vi "SSL Detection Frame Simple Estimator Cameras VelCmd.vi"(0 "NewCameras":T1[](array[typedef]) {"robots_blue"."height" format="%+4.3f"; "robots_blue"."pixel_y" format="%+4.3f"; "robots_blue"."pixel_x" format="%+4.3f"; "robots_blue"."orientation" format="%+4.3f"; "robots_blue"."y" format="%+4.3f"; "robots_blue"."confidence" format="%4.3f"; "robots_blue"."x" format="%+4.3f"; "robots_yellow"."height" format="%+4.3f"; "robots_yellow"."pixel_y" format="%+4.3f"; "robots_yellow"."pixel_x" format="%+4.3f"; "robots_yellow"."orientation" format="%+4.3f"; "robots_yellow"."y" format="%+4.3f"; "robots_yellow"."confidence" format="%4.3f"; "robots_yellow"."x" format="%+4.3f"}, 1 "Life Time":dbl=4.0, 2 "timeToValidateBall":dbl=0.5, 3 "Estimador":T5=enum."Nenhum", 5 "Field Size":T6, 9 "grSim?":bool, 10 "cameras array":dbl[](array[numeric]), 12 "Team":enum16{"Azul", "Amarelo"}(ring) caption="Enum", 14 "max ball vel":dbl, 15 "Side":enum16{"Esquerdo", "Direito"}(ring)=enum."Direito" caption="Enum") -> (4 "Detection Frame Out":T1 {"robots_blue"."height" format="%+4.3f"; "robots_blue"."pixel_y" format="%+4.3f"; "robots_blue"."pixel_x" format="%+4.3f"; "robots_blue"."orientation" format="%+4.3f"; "robots_blue"."y" format="%+4.3f"; "robots_blue"."confidence" format="%4.3f"; "robots_blue"."x" format="%+4.3f"; "robots_yellow"."height" format="%+4.3f"; "robots_yellow"."pixel_y" format="%+4.3f"; "robots_yellow"."pixel_x" format="%+4.3f"; "robots_yellow"."orientation" format="%+4.3f"; "robots_yellow"."y" format="%+4.3f"; "robots_yellow"."confidence" format="%4.3f"; "robots_yellow"."x" format="%+4.3f"}, 6 "Field Size Out":T6)   [LabVIEW 2022 SP3]
uses:
  Controls/SSL Detection Frame.ctl
  Controls/SSL Detection Robot.ctl
  <vilib>/Analysis/Matrix/Datatypes/RealMatrix.ctl
  Controls/SSL Detection Ball.ctl
  Controls/Estimadores.ctl
  <vilib>/Analysis/Matrix/Numeric/Conversions/Array To Matrix - RA.vi
  <vilib>/Analysis/Matrix/NI_Matrix.lvlib
  <vilib>/ptbypt/NI_PtbyPt.lvlib
  Utilities_class/Utilities.lvclass
  <vilib>/Analysis/NI_AALBase.lvlib
  Vision.lvclass
panel:
  in  "Enable":bool=TRUE
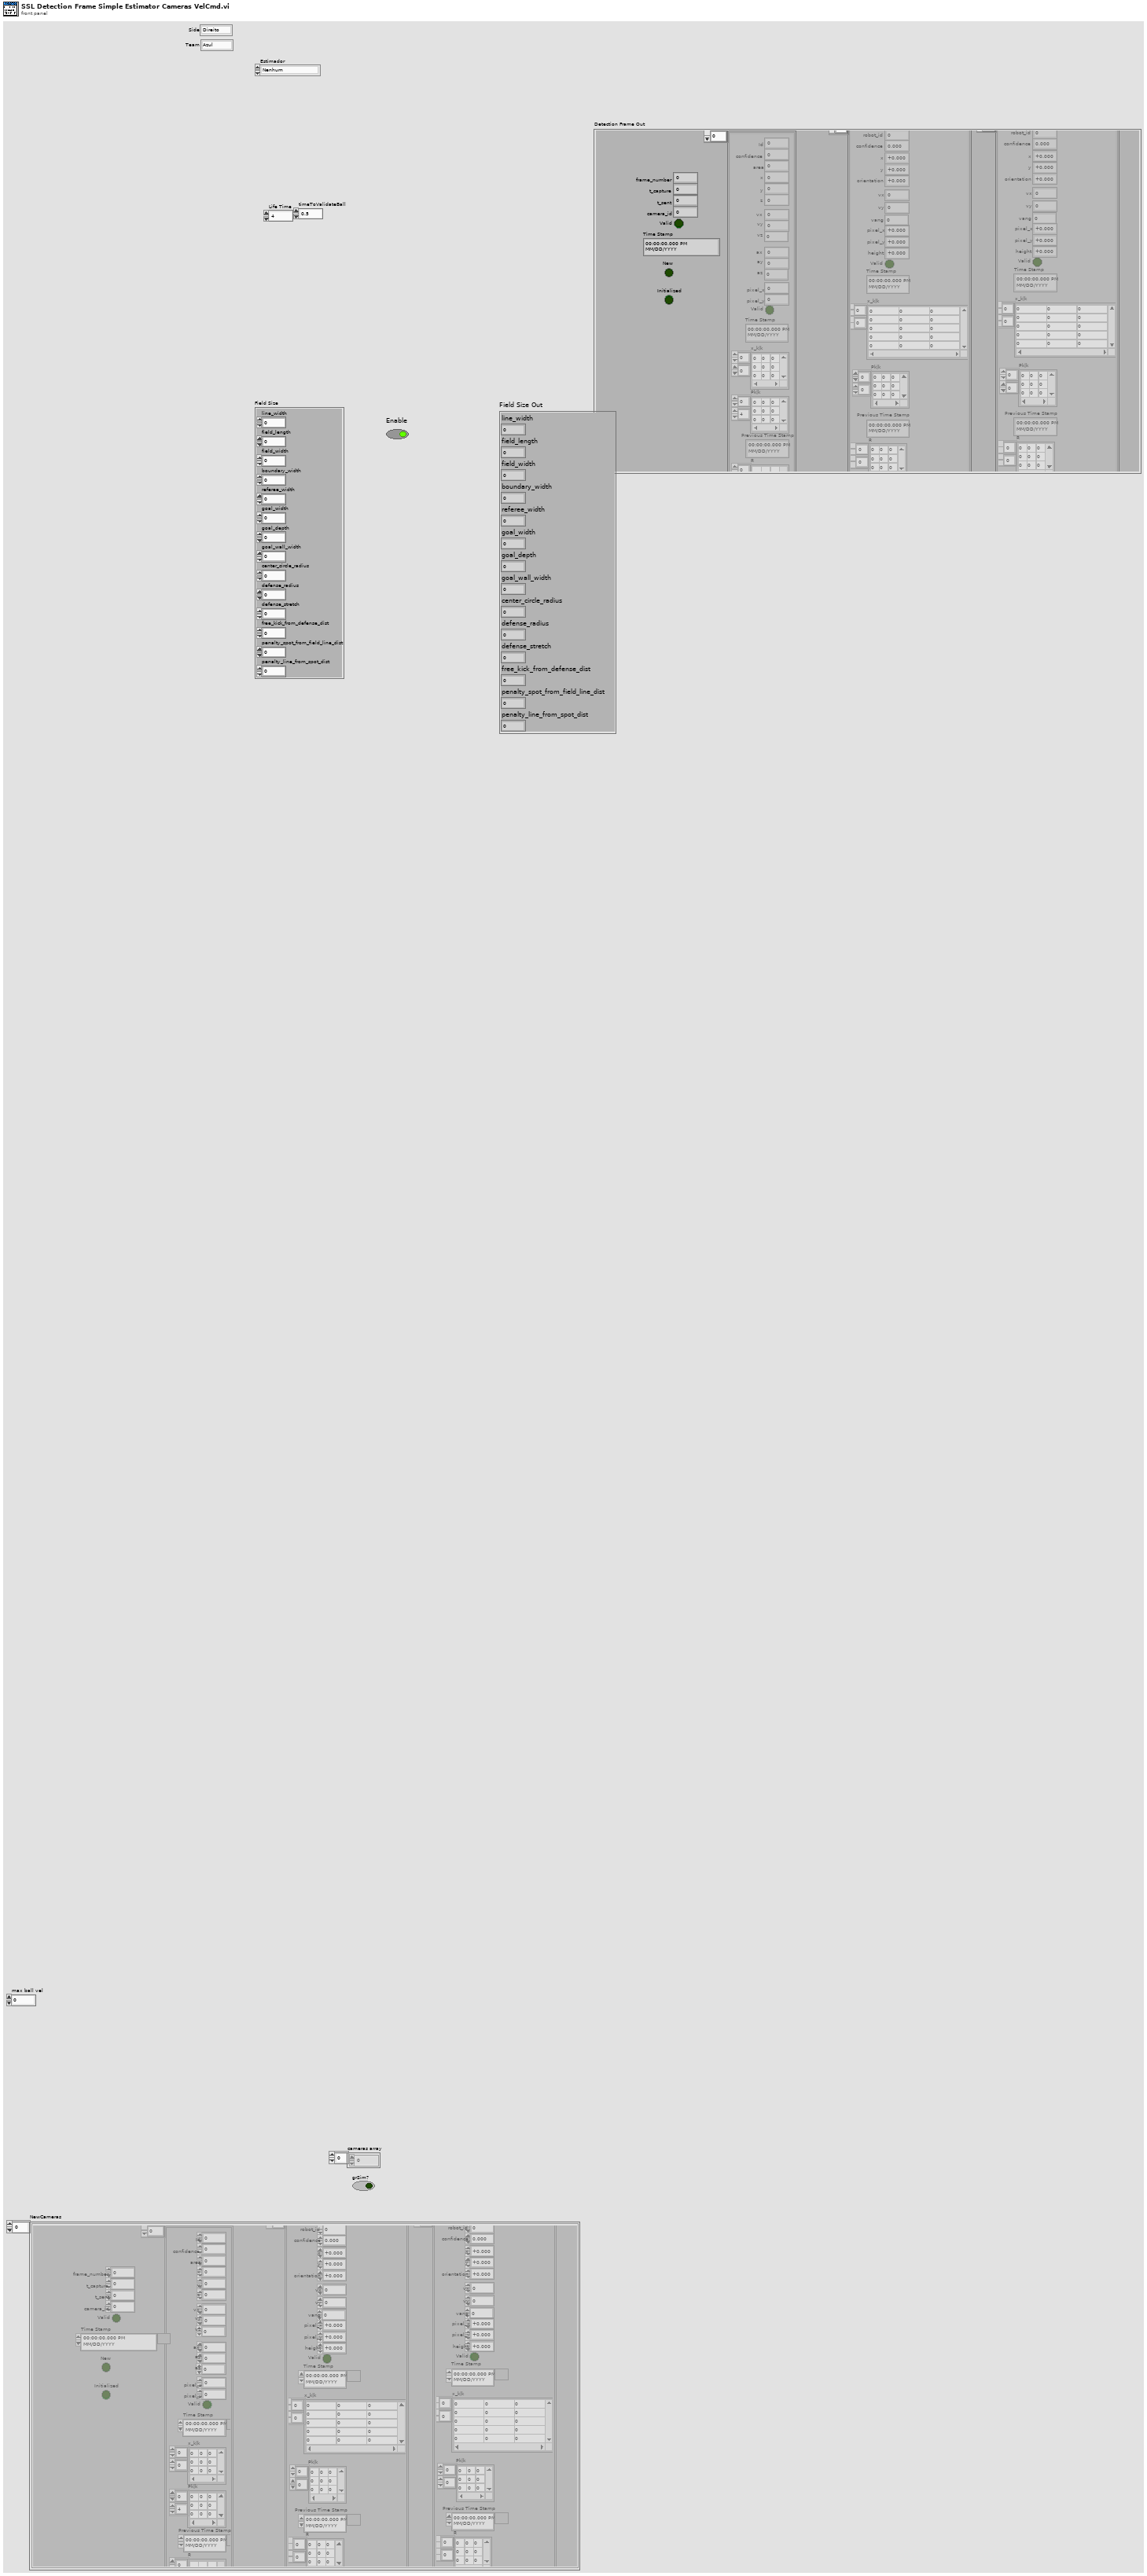
[diagram p1: front panel]
types:
  T1 = typedef "SSL Detection Frame.ctl" = cluster{"frame_number":u32, "t_capture":dbl, "t_sent":dbl, "camera_id":u32, "robots_yellow":T2[], "robots_blue":T2[], "balls":T4[], "Valid":bool, "Time Stamp":timestamp, "New":bool, "Initialized":bool}
  T2 = typedef "SSL Detection Robot.ctl" = cluster{"x":sgl, "robot_id":u32, "confidence":sgl, "y":sgl, "orientation":sgl, "pixel_x":sgl, "pixel_y":sgl, "height":sgl, "Valid":bool, "Time Stamp":timestamp, "x_k|k":T3, "Pk|k":T3, "Previous Time Stamp":timestamp, "R":T3, "vx":dbl, "vy":dbl, "vang":dbl}
  T3 = typedef "NI_Matrix.lvlib/RealMatrix.ctl" = dbl[][]
  T4 = typedef "SSL Detection Ball.ctl" = cluster{"x":sgl, "area":u32, "confidence":sgl, "y":sgl, "z":sgl, "pixel_x":sgl, "pixel_y":sgl, "Valid":bool, "Time Stamp":timestamp, "x_k|k":T3, "Pk|k":T3, "Id":u32, "Previous Time Stamp":timestamp, "R":T3, " vx":sgl, "vy":dbl, "vz":dbl, " ax":sgl, "ay":dbl, "az":dbl}
  T5 = typedef "Estimadores.ctl" = enum16{"Variable2ndDerivate", "4thDerivate", "2ndDerivate", "Nenhum", "Simples", "Kalman"}
  T6 = cluster{"line_width":u32, "field_length":u32, "field_width":u32, "boundary_width":u32, "referee_width":u32, "goal_width":u32, "goal_depth":u32, "goal_wall_width":u32, "center_circle_radius":u32, "defense_radius":u32, "defense_stretch":u32, "free_kick_from_defense_dist":u32, "penalty_spot_from_field_line_dist":u32, "penalty_line_from_spot_dist":u32}
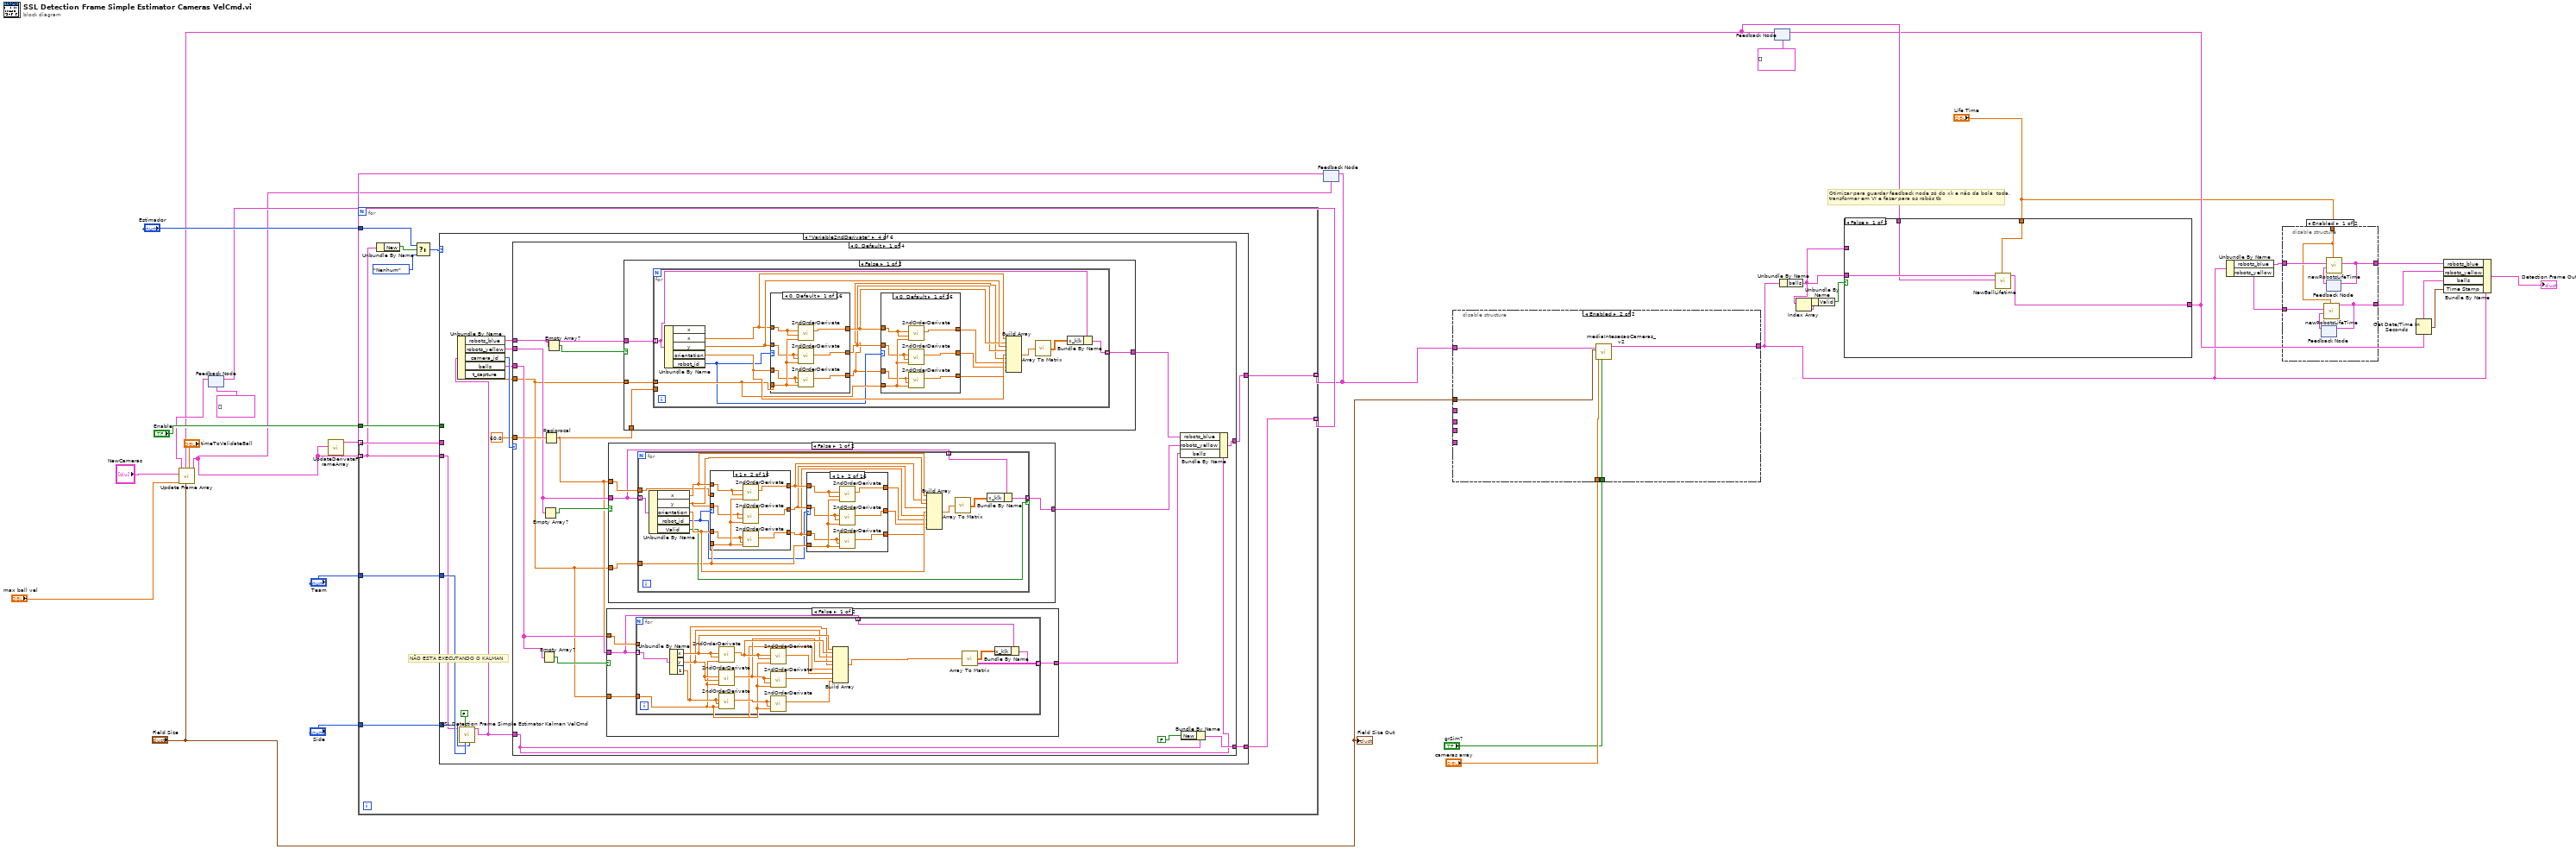
[diagram p0: block diagram]
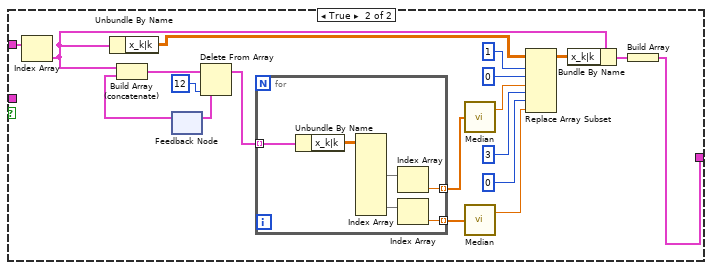
[diagram p3: hidden frame]
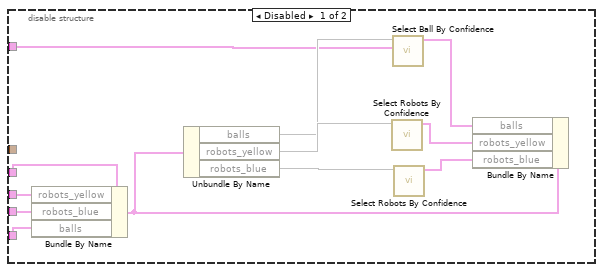
[diagram p4: hidden frame]
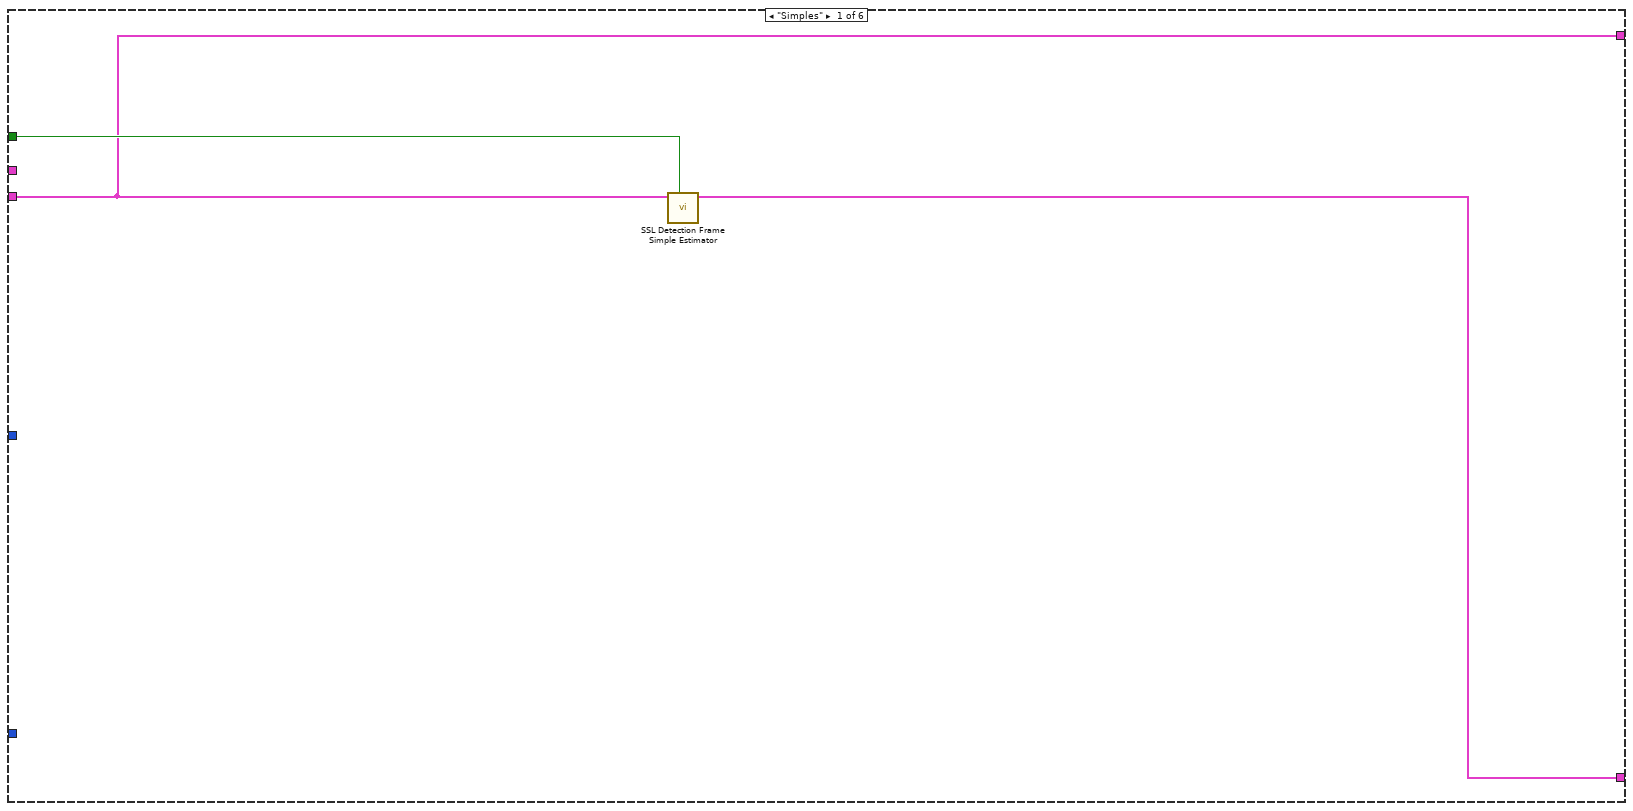
[diagram p5: hidden frame]
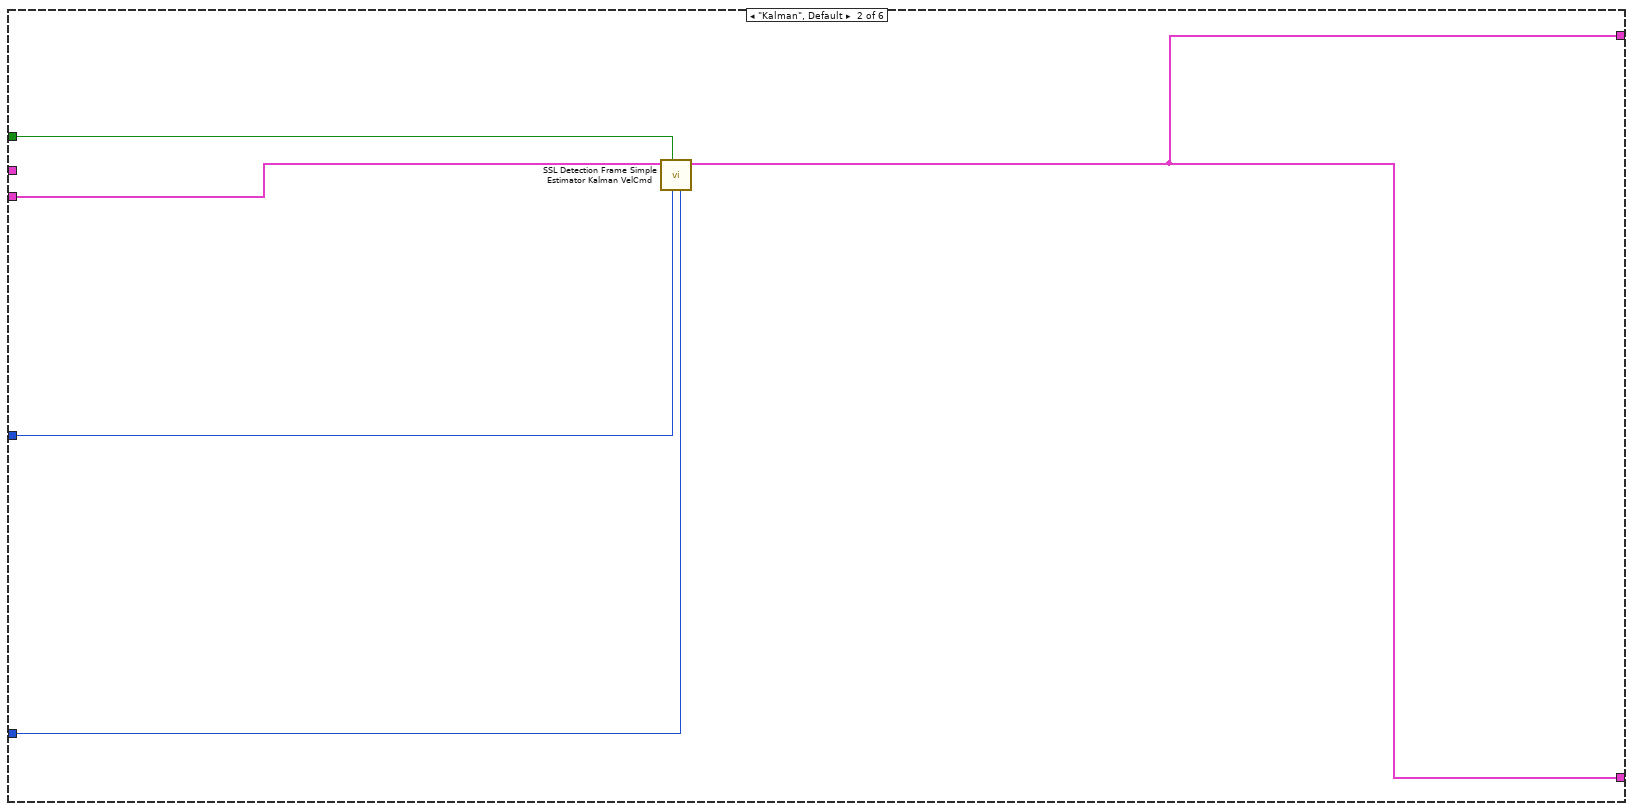
[diagram p6: hidden frame]
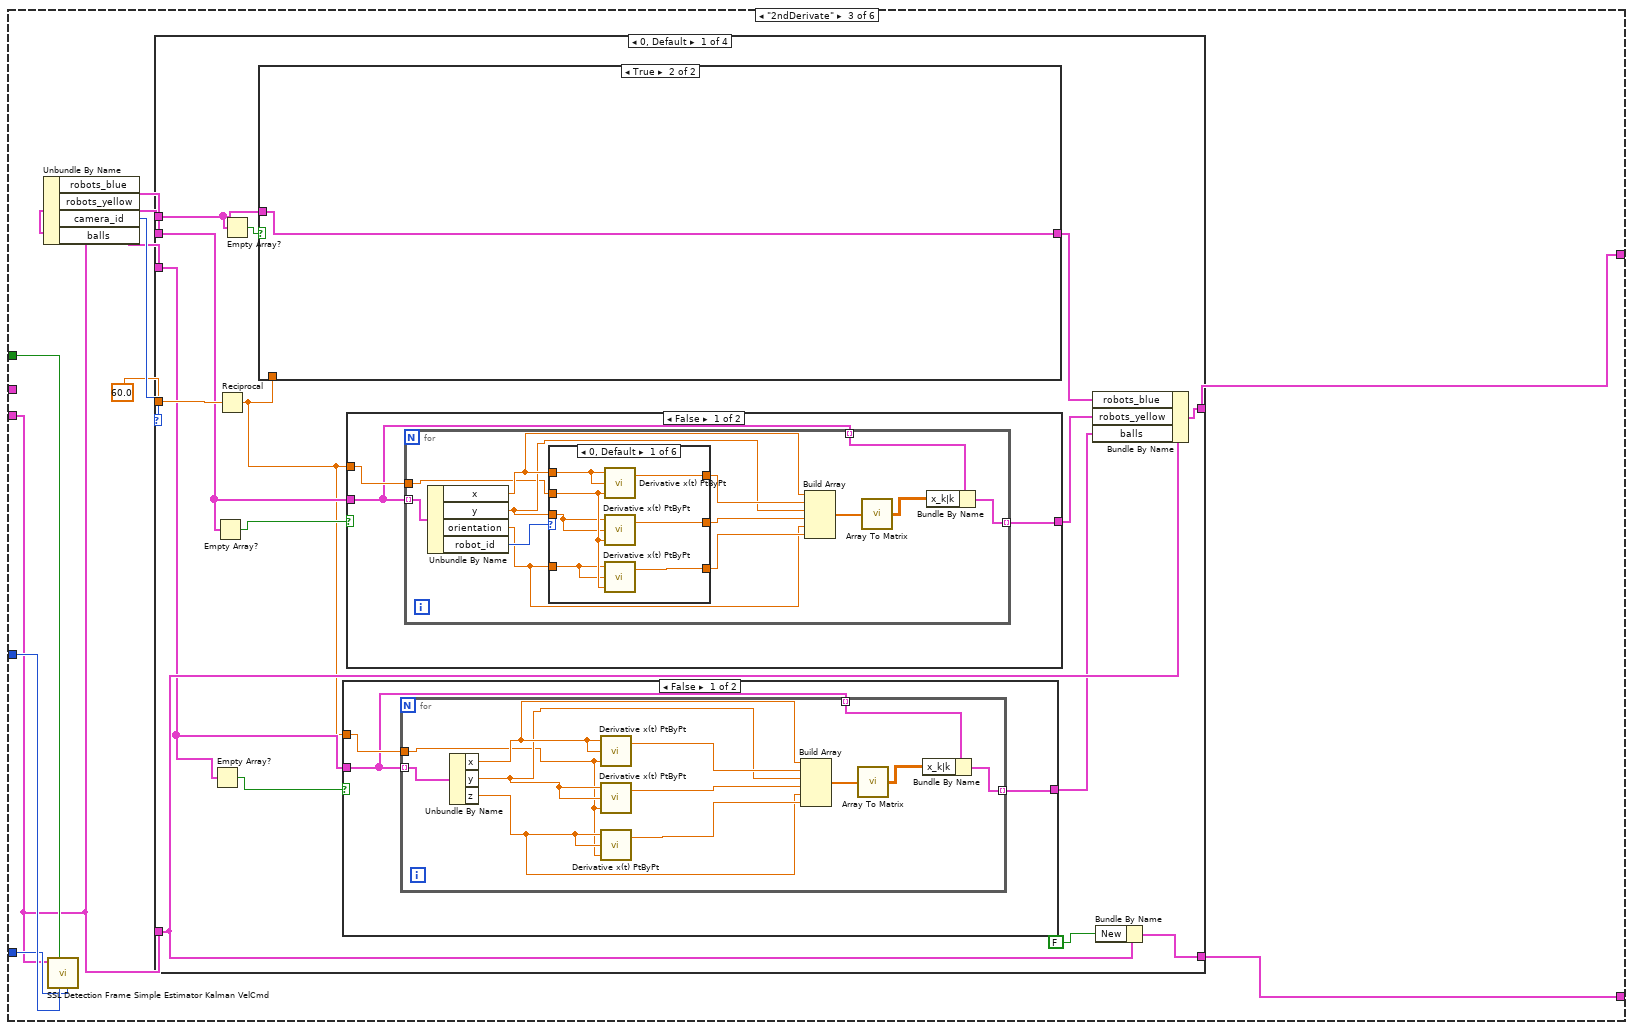
[diagram p7: hidden frame]
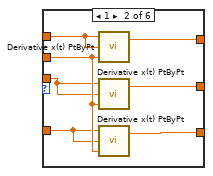
[diagram p9: hidden frame]
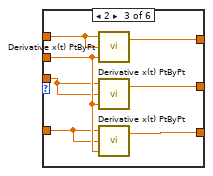
[diagram p10: hidden frame]
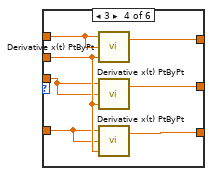
[diagram p11: hidden frame]
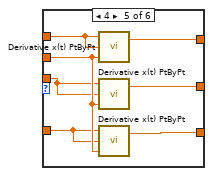
[diagram p12: hidden frame]
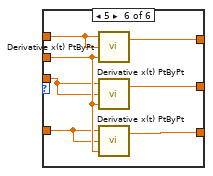
[diagram p13: hidden frame]
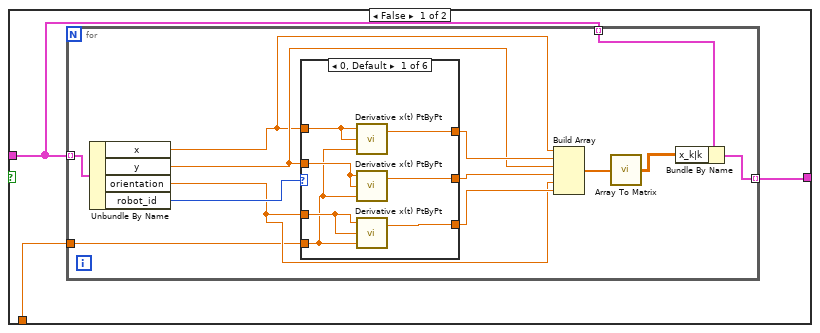
[diagram p15: hidden frame]
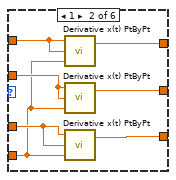
[diagram p16: hidden frame]
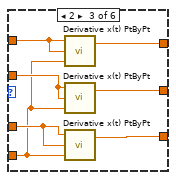
[diagram p17: hidden frame]
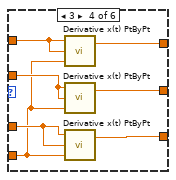
[diagram p18: hidden frame]
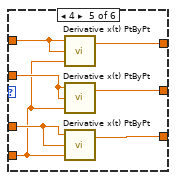
[diagram p19: hidden frame]
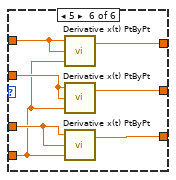
[diagram p20: hidden frame]
diagram:
  # "Otimizar para guardar feedback node só do xk e não da bola  toda.\ntransformar em VI e fazer para os robôs tb"
  n1 = feedback #1(T1[] []) -> (w28:T1[])
  n2 = feedback #2(T4[] [] ("balls")) -> (w13:T4[])
  n3 = call "Update Frame Array.vi"("timeToValidateBall"="timeToValidateBall", "Field Size"="Field Size", "balls"=w13, "max ball vel"="max ball vel", "Detection Frame In"="NewCameras", "Array Detection Frame In"=w28) -> ("Detection Frame out"=w18:T1[])  [unwired: 4 in, 1 out]
  n4 = feedback #3(w18) -> (w19:T1[])
  n5 = call "UpdateDerivateFrameArray.vi"("Current Detection Frame In"=w18, "Last Array Detection Frame In"=w19) -> ("Sorted Cameras Array"=w17:T1[])  [unwired: 9 in]
  n6 = for {
    tunnel: [w41] -> w26 mode=indexing
    tunnel: "Estimador" -> [w38]
    tunnel: "Enable" -> [w42]
    tunnel: w18 -> [w33] mode=indexing
    tunnel: "Team" -> [w40]
    tunnel: "Side" -> [w39]
    tunnel: [w36] -> w16 mode=indexing
    tunnel: w17 -> [w35] mode=indexing
    # "NÃO ESTA EXECUTANDO O KALMAN"
    n7 = Unbundle By Name(w33) -> ("New"=w34:bool)
    n8 = Select(t=w38, s=w34, f=Estimadores."Nenhum" ("Estimador")) -> (s? t:f=w37:T5)
    n9 = case shown="\"Variable2ndDerivate\"" w37 {
      tunnel: [w44 w46 w55 w665 w2786 w4880] -> w41
      tunnel: w33 -> [w43 w47 w51 w660 w2781 w4880]
      tunnel: w42 -> [w45 w50 w61 _ _ _]
      tunnel: w40 -> [_ w49 w60 w670 w2791 _]
      tunnel: w39 -> [_ w48 w59 w669 w2790 _]
      tunnel: [w43 w46 w56 w666 w2787 w4879] -> w36
      tunnel: w35 -> [_ _ _ _ _ w4879]
      frame "Simples" {
        n10 = call "SSL Detection Frame Simple Estimator.vi"("Enable"=w45, "Detection Frame In"=w43) -> ("Detection Frame Out"=w44:T1)  [unwired: 8 in, 1 out]
      }
      frame "Kalman", Default {
        n11 = call "SSL Detection Frame Simple Estimator Kalman VelCmd.vi"("Lado"=w48, "Time"=w49, "Enable"=w50, "Detection Frame In"=w47) -> ("Detection Frame Out"=w46:T1)  [unwired: 6 in, 1 out]
      }
      frame "2ndDerivate" {
        n12 = Unbundle By Name(w51) -> ("robots_blue"=w58:T2[], "robots_yellow"=w57:T2[], "camera_id"=w54:u32, "balls"=w53:T4[])
        n13 = call "SSL Detection Frame Simple Estimator Kalman VelCmd.vi"("Lado"=w59, "Time"=w60, "Enable"=w61, "Detection Frame In"=w51) -> ()  [unwired: 6 in, 2 out]
        n14 = case shown="0, Default" w54 {
          tunnel: w58 -> [w75 w224 w373 w522]
          tunnel: 60.0 -> [w74 w223 w372 w521]
          tunnel: w57 -> [w72 w221 w370 w519]
          tunnel: [w69 w218 w367 w516] -> w56
          tunnel: [w67 w216 w365 w514] -> w55
          tunnel: w51 -> [w66 w215 w364 w513]
          tunnel: w53 -> [w64 w213 w362 w511]
          frame 0, Default {
            n15 = Empty Array?(array=w64) -> (empty?=w65:bool)
            n16 = Empty Array?(array=w72) -> (empty?=w73:bool)
            n17 = Reciprocal(x=w74) -> (1/x=w63:dbl)
            n18 = Empty Array?(array=w75) -> (empty?=w76:bool)
            n19 = case shown="True" w76 {
              tunnel: w75 -> [w153 w210]
              tunnel: w63 -> [w154 _]
              tunnel: [w152 w210] -> w71
              frame False {
                n20 = for {
                  tunnel: w153 -> [w167] mode=indexing
                  tunnel: w154 -> [w157]
                  tunnel: w153 -> [w165] mode=indexing
                  tunnel: [w156] -> w152 mode=indexing
                  n21 = Unbundle By Name(w167) -> ("x"=w155:sgl, "y"=w159:sgl, "orientation"=w158:sgl, "robot_id"=w166:u32)
                  n22 = case shown="0, Default" w166 {
                    tunnel: w155 -> [w168 w178 w185 w192 w199 w206]
                    tunnel: [w174 w181 w188 w195 w202 w209] -> w164
                    tunnel: [w173 w180 w187 w194 w201 w208] -> w163
                    tunnel: [w172 w179 w186 w193 w200 w207] -> w162
                    tunnel: w159 -> [w171 w177 w184 w191 w198 w205]
                    tunnel: w158 -> [w170 w176 w183 w190 w197 w204]
                    tunnel: w157 -> [w169 w175 w182 w189 w196 w203]
                    frame 0, Default {
                      n23 = call <vilib>:"Derivative x(t) PtByPt.vi"("dt"=w169, "initial condition"=w168, "x"=w168) -> ("dx/dt"=w174:dbl)  [unwired: 1 in, 1 out]
                      n24 = call <vilib>:"Derivative x(t) PtByPt.vi"("dt"=w169, "initial condition"=w171, "x"=w171) -> ("dx/dt"=w173:dbl)  [unwired: 1 in, 1 out]
                      n25 = call <vilib>:"Derivative x(t) PtByPt.vi"("dt"=w169, "initial condition"=w170, "x"=w170) -> ("dx/dt"=w172:dbl)  [unwired: 1 in, 1 out]
                    }
                    frame 1 {
                      n26 = call <vilib>:"Derivative x(t) PtByPt.vi"("dt"=w175, "initial condition"=w178, "x"=w178) -> ("dx/dt"=w181:dbl)  [unwired: 1 in, 1 out]
                      n27 = call <vilib>:"Derivative x(t) PtByPt.vi"("dt"=w175, "initial condition"=w177, "x"=w177) -> ("dx/dt"=w180:dbl)  [unwired: 1 in, 1 out]
                      n28 = call <vilib>:"Derivative x(t) PtByPt.vi"("dt"=w175, "initial condition"=w176, "x"=w176) -> ("dx/dt"=w179:dbl)  [unwired: 1 in, 1 out]
                    }
                    frame 2 {
                      n29 = call <vilib>:"Derivative x(t) PtByPt.vi"("dt"=w182, "initial condition"=w185, "x"=w185) -> ("dx/dt"=w188:dbl)  [unwired: 1 in, 1 out]
                      n30 = call <vilib>:"Derivative x(t) PtByPt.vi"("dt"=w182, "initial condition"=w184, "x"=w184) -> ("dx/dt"=w187:dbl)  [unwired: 1 in, 1 out]
                      n31 = call <vilib>:"Derivative x(t) PtByPt.vi"("dt"=w182, "initial condition"=w183, "x"=w183) -> ("dx/dt"=w186:dbl)  [unwired: 1 in, 1 out]
                    }
                    frame 3 {
                      n32 = call <vilib>:"Derivative x(t) PtByPt.vi"("dt"=w189, "initial condition"=w192, "x"=w192) -> ("dx/dt"=w195:dbl)  [unwired: 1 in, 1 out]
                      n33 = call <vilib>:"Derivative x(t) PtByPt.vi"("dt"=w189, "initial condition"=w191, "x"=w191) -> ("dx/dt"=w194:dbl)  [unwired: 1 in, 1 out]
                      n34 = call <vilib>:"Derivative x(t) PtByPt.vi"("dt"=w189, "initial condition"=w190, "x"=w190) -> ("dx/dt"=w193:dbl)  [unwired: 1 in, 1 out]
                    }
                    frame 4 {
                      n35 = call <vilib>:"Derivative x(t) PtByPt.vi"("dt"=w196, "initial condition"=w199, "x"=w199) -> ("dx/dt"=w202:dbl)  [unwired: 1 in, 1 out]
                      n36 = call <vilib>:"Derivative x(t) PtByPt.vi"("dt"=w196, "initial condition"=w198, "x"=w198) -> ("dx/dt"=w201:dbl)  [unwired: 1 in, 1 out]
                      n37 = call <vilib>:"Derivative x(t) PtByPt.vi"("dt"=w196, "initial condition"=w197, "x"=w197) -> ("dx/dt"=w200:dbl)  [unwired: 1 in, 1 out]
                    }
                    frame 5 {
                      n38 = call <vilib>:"Derivative x(t) PtByPt.vi"("dt"=w203, "initial condition"=w206, "x"=w206) -> ("dx/dt"=w209:dbl)  [unwired: 1 in, 1 out]
                      n39 = call <vilib>:"Derivative x(t) PtByPt.vi"("dt"=w203, "initial condition"=w205, "x"=w205) -> ("dx/dt"=w208:dbl)  [unwired: 1 in, 1 out]
                      n40 = call <vilib>:"Derivative x(t) PtByPt.vi"("dt"=w203, "initial condition"=w204, "x"=w204) -> ("dx/dt"=w207:dbl)  [unwired: 1 in, 1 out]
                    }
                  }
                  n41 = Build Array(w155, w164, w159, w163, w158, w162) -> (w161:dbl[])
                  n42 = call-poly <vilib>:"Array To Matrix.vi"("Real 1D Array"=w161) -> ("Real Matrix (Column Vector)"=w160:T3)
                  n43 = Bundle By Name(cluster=w165, "x_k|k"=w160) -> (w156:T2)
                }
              }
              frame True {
              }
            }
            n44 = case shown="False" w65 {
              tunnel: w64 -> [w78 w92]
              tunnel: w63 -> [w79 _]
              tunnel: [w77 w92] -> w62
              frame False {
                n45 = for {
                  tunnel: w78 -> [w91] mode=indexing
                  tunnel: w79 -> [w80]
                  tunnel: w78 -> [w90] mode=indexing
                  tunnel: [w81] -> w77 mode=indexing
                  n46 = Unbundle By Name(w91) -> ("x"=w85:sgl, "y"=w84:sgl, "z"=w86:sgl)
                  n47 = call <vilib>:"Derivative x(t) PtByPt.vi"("dt"=w80, "initial condition"=w85, "x"=w85) -> ("dx/dt"=w89:dbl)  [unwired: 1 in, 1 out]
                  n48 = call <vilib>:"Derivative x(t) PtByPt.vi"("dt"=w80, "initial condition"=w84, "x"=w84) -> ("dx/dt"=w88:dbl)  [unwired: 1 in, 1 out]
                  n49 = call <vilib>:"Derivative x(t) PtByPt.vi"("dt"=w80, "initial condition"=w86, "x"=w86) -> ("dx/dt"=w87:dbl)  [unwired: 1 in, 1 out]
                  n50 = Build Array(w85, w89, w84, w88, w86, w87) -> (w83:dbl[])
                  n51 = call-poly <vilib>:"Array To Matrix.vi"("Real 1D Array"=w83) -> ("Real Matrix (Column Vector)"=w82:T3)
                  n52 = Bundle By Name(cluster=w90, "x_k|k"=w82) -> (w81:T4)
                }
              }
              frame True {
              }
            }
            n53 = case shown="False" w73 {
              tunnel: w72 -> [w94 w151]
              tunnel: w63 -> [w95 _]
              tunnel: [w93 w151] -> w70
              frame False {
                n54 = for {
                  tunnel: w94 -> [w108] mode=indexing
                  tunnel: w95 -> [w96]
                  tunnel: w94 -> [w106] mode=indexing
                  tunnel: [w97] -> w93 mode=indexing
                  n55 = Unbundle By Name(w108) -> ("x"=w101:sgl, "y"=w100:sgl, "orientation"=w102:sgl, "robot_id"=w107:u32)
                  n56 = case shown="0, Default" w107 {
                    tunnel: w101 -> [w112 w119 w126 w133 w140 w147]
                    tunnel: w100 -> [w110 w117 w124 w131 w138 w145]
                    tunnel: w102 -> [w109 w116 w123 w130 w137 w144]
                    tunnel: [w115 w122 w129 w136 w143 w150] -> w105
                    tunnel: [w114 w121 w128 w135 w142 w149] -> w104
                    tunnel: [w113 w120 w127 w134 w141 w148] -> w103
                    tunnel: w96 -> [w111 w118 w125 w132 w139 w146]
                    frame 0, Default {
                      n57 = call <vilib>:"Derivative x(t) PtByPt.vi"("dt"=w111, "initial condition"=w112, "x"=w112) -> ("dx/dt"=w115:dbl)  [unwired: 1 in, 1 out]
                      n58 = call <vilib>:"Derivative x(t) PtByPt.vi"("dt"=w111, "initial condition"=w110, "x"=w110) -> ("dx/dt"=w114:dbl)  [unwired: 1 in, 1 out]
                      n59 = call <vilib>:"Derivative x(t) PtByPt.vi"("dt"=w111, "initial condition"=w109, "x"=w109) -> ("dx/dt"=w113:dbl)  [unwired: 1 in, 1 out]
                    }
                    frame 1 {
                      n60 = call <vilib>:"Derivative x(t) PtByPt.vi"("dt"=w118, "initial condition"=w119, "x"=w119) -> ("dx/dt"=w122:dbl)  [unwired: 1 in, 1 out]
                      n61 = call <vilib>:"Derivative x(t) PtByPt.vi"("dt"=w118, "initial condition"=w117, "x"=w117) -> ("dx/dt"=w121:dbl)  [unwired: 1 in, 1 out]
                      n62 = call <vilib>:"Derivative x(t) PtByPt.vi"("dt"=w118, "initial condition"=w116, "x"=w116) -> ("dx/dt"=w120:dbl)  [unwired: 1 in, 1 out]
                    }
                    frame 2 {
                      n63 = call <vilib>:"Derivative x(t) PtByPt.vi"("dt"=w125, "initial condition"=w126, "x"=w126) -> ("dx/dt"=w129:dbl)  [unwired: 1 in, 1 out]
                      n64 = call <vilib>:"Derivative x(t) PtByPt.vi"("dt"=w125, "initial condition"=w124, "x"=w124) -> ("dx/dt"=w128:dbl)  [unwired: 1 in, 1 out]
                      n65 = call <vilib>:"Derivative x(t) PtByPt.vi"("dt"=w125, "initial condition"=w123, "x"=w123) -> ("dx/dt"=w127:dbl)  [unwired: 1 in, 1 out]
                    }
                    frame 3 {
                      n66 = call <vilib>:"Derivative x(t) PtByPt.vi"("dt"=w132, "initial condition"=w133, "x"=w133) -> ("dx/dt"=w136:dbl)  [unwired: 1 in, 1 out]
                      n67 = call <vilib>:"Derivative x(t) PtByPt.vi"("dt"=w132, "initial condition"=w131, "x"=w131) -> ("dx/dt"=w135:dbl)  [unwired: 1 in, 1 out]
                      n68 = call <vilib>:"Derivative x(t) PtByPt.vi"("dt"=w132, "initial condition"=w130, "x"=w130) -> ("dx/dt"=w134:dbl)  [unwired: 1 in, 1 out]
                    }
                    frame 4 {
                      n69 = call <vilib>:"Derivative x(t) PtByPt.vi"("dt"=w139, "initial condition"=w140, "x"=w140) -> ("dx/dt"=w143:dbl)  [unwired: 1 in, 1 out]
                      n70 = call <vilib>:"Derivative x(t) PtByPt.vi"("dt"=w139, "initial condition"=w138, "x"=w138) -> ("dx/dt"=w142:dbl)  [unwired: 1 in, 1 out]
                      n71 = call <vilib>:"Derivative x(t) PtByPt.vi"("dt"=w139, "initial condition"=w137, "x"=w137) -> ("dx/dt"=w141:dbl)  [unwired: 1 in, 1 out]
                    }
                    frame 5 {
                      n72 = call <vilib>:"Derivative x(t) PtByPt.vi"("dt"=w146, "initial condition"=w147, "x"=w147) -> ("dx/dt"=w150:dbl)  [unwired: 1 in, 1 out]
                      n73 = call <vilib>:"Derivative x(t) PtByPt.vi"("dt"=w146, "initial condition"=w145, "x"=w145) -> ("dx/dt"=w149:dbl)  [unwired: 1 in, 1 out]
                      n74 = call <vilib>:"Derivative x(t) PtByPt.vi"("dt"=w146, "initial condition"=w144, "x"=w144) -> ("dx/dt"=w148:dbl)  [unwired: 1 in, 1 out]
                    }
                  }
                  n75 = Build Array(w101, w105, w100, w104, w102, w103) -> (w99:dbl[])
                  n76 = call-poly <vilib>:"Array To Matrix.vi"("Real 1D Array"=w99) -> ("Real Matrix (Column Vector)"=w98:T3)
                  n77 = Bundle By Name(cluster=w106, "x_k|k"=w98) -> (w97:T2)
                }
              }
              frame True {
              }
            }
            n78 = Bundle By Name(cluster=w66, "robots_blue"=w71, "robots_yellow"=w70, "balls"=w62) -> (w69:T1)
            n79 = Bundle By Name(cluster=w66, "New"=FALSE) -> (w67:T1)
          }
          frame 1 {
            n80 = Empty Array?(array=w213) -> (empty?=w214:bool)
            n81 = Empty Array?(array=w221) -> (empty?=w222:bool)
            n82 = Reciprocal(x=w223) -> (1/x=w212:dbl)
            n83 = Empty Array?(array=w224) -> (empty?=w225:bool)
            n84 = case shown="False" w225 {
              tunnel: w224 -> [w302 w359]
              tunnel: w212 -> [w303 _]
              tunnel: [w301 w359] -> w220
              frame False {
                n85 = for {
                  tunnel: w302 -> [w316] mode=indexing
                  tunnel: w303 -> [w306]
                  tunnel: w302 -> [w314] mode=indexing
                  tunnel: [w305] -> w301 mode=indexing
                  n86 = Unbundle By Name(w316) -> ("x"=w304:sgl, "y"=w308:sgl, "orientation"=w307:sgl, "robot_id"=w315:u32)
                  n87 = case shown="0, Default" w315 {
                    tunnel: w304 -> [w317 w327 w334 w341 w348 w355]
                    tunnel: [w323 w330 w337 w344 w351 w358] -> w313
                    tunnel: [w322 w329 w336 w343 w350 w357] -> w312
                    tunnel: [w321 w328 w335 w342 w349 w356] -> w311
                    tunnel: w308 -> [w320 w326 w333 w340 w347 w354]
                    tunnel: w307 -> [w319 w325 w332 w339 w346 w353]
                    tunnel: w306 -> [w318 w324 w331 w338 w345 w352]
                    frame 0, Default {
                      n88 = call <vilib>:"Derivative x(t) PtByPt.vi"("dt"=w318, "initial condition"=w317, "x"=w317) -> ("dx/dt"=w323:dbl)  [unwired: 1 in, 1 out]
                      n89 = call <vilib>:"Derivative x(t) PtByPt.vi"("dt"=w318, "initial condition"=w320, "x"=w320) -> ("dx/dt"=w322:dbl)  [unwired: 1 in, 1 out]
                      n90 = call <vilib>:"Derivative x(t) PtByPt.vi"("dt"=w318, "initial condition"=w319, "x"=w319) -> ("dx/dt"=w321:dbl)  [unwired: 1 in, 1 out]
                    }
                    frame 1 {
                      n91 = call <vilib>:"Derivative x(t) PtByPt.vi"("dt"=w324, "initial condition"=w327, "x"=w327) -> ("dx/dt"=w330:dbl)  [unwired: 1 in, 1 out]
                      n92 = call <vilib>:"Derivative x(t) PtByPt.vi"("dt"=w324, "initial condition"=w326, "x"=w326) -> ("dx/dt"=w329:dbl)  [unwired: 1 in, 1 out]
                      n93 = call <vilib>:"Derivative x(t) PtByPt.vi"("dt"=w324, "initial condition"=w325, "x"=w325) -> ("dx/dt"=w328:dbl)  [unwired: 1 in, 1 out]
                    }
                    frame 2 {
                      n94 = call <vilib>:"Derivative x(t) PtByPt.vi"("dt"=w331, "initial condition"=w334, "x"=w334) -> ("dx/dt"=w337:dbl)  [unwired: 1 in, 1 out]
                      n95 = call <vilib>:"Derivative x(t) PtByPt.vi"("dt"=w331, "initial condition"=w333, "x"=w333) -> ("dx/dt"=w336:dbl)  [unwired: 1 in, 1 out]
                      n96 = call <vilib>:"Derivative x(t) PtByPt.vi"("dt"=w331, "initial condition"=w332, "x"=w332) -> ("dx/dt"=w335:dbl)  [unwired: 1 in, 1 out]
                    }
                    frame 3 {
                      n97 = call <vilib>:"Derivative x(t) PtByPt.vi"("dt"=w338, "initial condition"=w341, "x"=w341) -> ("dx/dt"=w344:dbl)  [unwired: 1 in, 1 out]
                      n98 = call <vilib>:"Derivative x(t) PtByPt.vi"("dt"=w338, "initial condition"=w340, "x"=w340) -> ("dx/dt"=w343:dbl)  [unwired: 1 in, 1 out]
                      n99 = call <vilib>:"Derivative x(t) PtByPt.vi"("dt"=w338, "initial condition"=w339, "x"=w339) -> ("dx/dt"=w342:dbl)  [unwired: 1 in, 1 out]
                    }
                    frame 4 {
                      n100 = call <vilib>:"Derivative x(t) PtByPt.vi"("dt"=w345, "initial condition"=w348, "x"=w348) -> ("dx/dt"=w351:dbl)  [unwired: 1 in, 1 out]
                      n101 = call <vilib>:"Derivative x(t) PtByPt.vi"("dt"=w345, "initial condition"=w347, "x"=w347) -> ("dx/dt"=w350:dbl)  [unwired: 1 in, 1 out]
                      n102 = call <vilib>:"Derivative x(t) PtByPt.vi"("dt"=w345, "initial condition"=w346, "x"=w346) -> ("dx/dt"=w349:dbl)  [unwired: 1 in, 1 out]
                    }
                    frame 5 {
                      n103 = call <vilib>:"Derivative x(t) PtByPt.vi"("dt"=w352, "initial condition"=w355, "x"=w355) -> ("dx/dt"=w358:dbl)  [unwired: 1 in, 1 out]
                      n104 = call <vilib>:"Derivative x(t) PtByPt.vi"("dt"=w352, "initial condition"=w354, "x"=w354) -> ("dx/dt"=w357:dbl)  [unwired: 1 in, 1 out]
                      n105 = call <vilib>:"Derivative x(t) PtByPt.vi"("dt"=w352, "initial condition"=w353, "x"=w353) -> ("dx/dt"=w356:dbl)  [unwired: 1 in, 1 out]
                    }
                  }
                  n106 = Build Array(w304, w313, w308, w312, w307, w311) -> (w310:dbl[])
                  n107 = call-poly <vilib>:"Array To Matrix.vi"("Real 1D Array"=w310) -> ("Real Matrix (Column Vector)"=w309:T3)
                  n108 = Bundle By Name(cluster=w314, "x_k|k"=w309) -> (w305:T2)
                }
              }
              frame True {
              }
            }
            n109 = case shown="False" w214 {
              tunnel: w213 -> [w227 w241]
              tunnel: w212 -> [w228 _]
              tunnel: [w226 w241] -> w211
              frame False {
                n110 = for {
                  tunnel: w227 -> [w240] mode=indexing
                  tunnel: w228 -> [w229]
                  tunnel: w227 -> [w239] mode=indexing
                  tunnel: [w230] -> w226 mode=indexing
                  n111 = Unbundle By Name(w240) -> ("x"=w234:sgl, "y"=w233:sgl, "z"=w235:sgl)
                  n112 = call <vilib>:"Derivative x(t) PtByPt.vi"("dt"=w229, "initial condition"=w234, "x"=w234) -> ("dx/dt"=w238:dbl)  [unwired: 1 in, 1 out]
                  n113 = call <vilib>:"Derivative x(t) PtByPt.vi"("dt"=w229, "initial condition"=w233, "x"=w233) -> ("dx/dt"=w237:dbl)  [unwired: 1 in, 1 out]
                  n114 = call <vilib>:"Derivative x(t) PtByPt.vi"("dt"=w229, "initial condition"=w235, "x"=w235) -> ("dx/dt"=w236:dbl)  [unwired: 1 in, 1 out]
                  n115 = Build Array(w234, w238, w233, w237, w235, w236) -> (w232:dbl[])
                  n116 = call-poly <vilib>:"Array To Matrix.vi"("Real 1D Array"=w232) -> ("Real Matrix (Column Vector)"=w231:T3)
                  n117 = Bundle By Name(cluster=w239, "x_k|k"=w231) -> (w230:T4)
                }
              }
              frame True {
              }
            }
            n118 = case shown="False" w222 {
              tunnel: w221 -> [w243 w300]
              tunnel: w212 -> [w244 _]
              tunnel: [w242 w300] -> w219
              frame False {
                n119 = for {
                  tunnel: w243 -> [w257] mode=indexing
                  tunnel: w244 -> [w245]
                  tunnel: w243 -> [w255] mode=indexing
                  tunnel: [w246] -> w242 mode=indexing
                  n120 = Unbundle By Name(w257) -> ("x"=w250:sgl, "y"=w249:sgl, "orientation"=w251:sgl, "robot_id"=w256:u32)
                  n121 = case shown="0, Default" w256 {
                    tunnel: w250 -> [w261 w268 w275 w282 w289 w296]
                    tunnel: w249 -> [w259 w266 w273 w280 w287 w294]
                    tunnel: w251 -> [w258 w265 w272 w279 w286 w293]
                    tunnel: [w264 w271 w278 w285 w292 w299] -> w254
                    tunnel: [w263 w270 w277 w284 w291 w298] -> w253
                    tunnel: [w262 w269 w276 w283 w290 w297] -> w252
                    tunnel: w245 -> [w260 w267 w274 w281 w288 w295]
                    frame 0, Default {
                      n122 = call <vilib>:"Derivative x(t) PtByPt.vi"("dt"=w260, "initial condition"=w261, "x"=w261) -> ("dx/dt"=w264:dbl)  [unwired: 1 in, 1 out]
                      n123 = call <vilib>:"Derivative x(t) PtByPt.vi"("dt"=w260, "initial condition"=w259, "x"=w259) -> ("dx/dt"=w263:dbl)  [unwired: 1 in, 1 out]
                      n124 = call <vilib>:"Derivative x(t) PtByPt.vi"("dt"=w260, "initial condition"=w258, "x"=w258) -> ("dx/dt"=w262:dbl)  [unwired: 1 in, 1 out]
                    }
                    frame 1 {
                      n125 = call <vilib>:"Derivative x(t) PtByPt.vi"("dt"=w267, "initial condition"=w268, "x"=w268) -> ("dx/dt"=w271:dbl)  [unwired: 1 in, 1 out]
                      n126 = call <vilib>:"Derivative x(t) PtByPt.vi"("dt"=w267, "initial condition"=w266, "x"=w266) -> ("dx/dt"=w270:dbl)  [unwired: 1 in, 1 out]
                      n127 = call <vilib>:"Derivative x(t) PtByPt.vi"("dt"=w267, "initial condition"=w265, "x"=w265) -> ("dx/dt"=w269:dbl)  [unwired: 1 in, 1 out]
                    }
                    frame 2 {
                      n128 = call <vilib>:"Derivative x(t) PtByPt.vi"("dt"=w274, "initial condition"=w275, "x"=w275) -> ("dx/dt"=w278:dbl)  [unwired: 1 in, 1 out]
                      n129 = call <vilib>:"Derivative x(t) PtByPt.vi"("dt"=w274, "initial condition"=w273, "x"=w273) -> ("dx/dt"=w277:dbl)  [unwired: 1 in, 1 out]
                      n130 = call <vilib>:"Derivative x(t) PtByPt.vi"("dt"=w274, "initial condition"=w272, "x"=w272) -> ("dx/dt"=w276:dbl)  [unwired: 1 in, 1 out]
                    }
                    frame 3 {
                      n131 = call <vilib>:"Derivative x(t) PtByPt.vi"("dt"=w281, "initial condition"=w282, "x"=w282) -> ("dx/dt"=w285:dbl)  [unwired: 1 in, 1 out]
                      n132 = call <vilib>:"Derivative x(t) PtByPt.vi"("dt"=w281, "initial condition"=w280, "x"=w280) -> ("dx/dt"=w284:dbl)  [unwired: 1 in, 1 out]
                      n133 = call <vilib>:"Derivative x(t) PtByPt.vi"("dt"=w281, "initial condition"=w279, "x"=w279) -> ("dx/dt"=w283:dbl)  [unwired: 1 in, 1 out]
                    }
                    frame 4 {
                      n134 = call <vilib>:"Derivative x(t) PtByPt.vi"("dt"=w288, "initial condition"=w289, "x"=w289) -> ("dx/dt"=w292:dbl)  [unwired: 1 in, 1 out]
                      n135 = call <vilib>:"Derivative x(t) PtByPt.vi"("dt"=w288, "initial condition"=w287, "x"=w287) -> ("dx/dt"=w291:dbl)  [unwired: 1 in, 1 out]
                      n136 = call <vilib>:"Derivative x(t) PtByPt.vi"("dt"=w288, "initial condition"=w286, "x"=w286) -> ("dx/dt"=w290:dbl)  [unwired: 1 in, 1 out]
                    }
                    frame 5 {
                      n137 = call <vilib>:"Derivative x(t) PtByPt.vi"("dt"=w295, "initial condition"=w296, "x"=w296) -> ("dx/dt"=w299:dbl)  [unwired: 1 in, 1 out]
                      n138 = call <vilib>:"Derivative x(t) PtByPt.vi"("dt"=w295, "initial condition"=w294, "x"=w294) -> ("dx/dt"=w298:dbl)  [unwired: 1 in, 1 out]
                      n139 = call <vilib>:"Derivative x(t) PtByPt.vi"("dt"=w295, "initial condition"=w293, "x"=w293) -> ("dx/dt"=w297:dbl)  [unwired: 1 in, 1 out]
                    }
                  }
                  n140 = Build Array(w250, w254, w249, w253, w251, w252) -> (w248:dbl[])
                  n141 = call-poly <vilib>:"Array To Matrix.vi"("Real 1D Array"=w248) -> ("Real Matrix (Column Vector)"=w247:T3)
                  n142 = Bundle By Name(cluster=w255, "x_k|k"=w247) -> (w246:T2)
                }
              }
              frame True {
              }
            }
            n143 = Bundle By Name(cluster=w215, "robots_blue"=w220, "robots_yellow"=w219, "balls"=w211) -> (w218:T1)
            n144 = Bundle By Name(cluster=w215, "New"=FALSE) -> (w216:T1)
          }
          frame 2 {
            n145 = Empty Array?(array=w362) -> (empty?=w363:bool)
            n146 = Empty Array?(array=w370) -> (empty?=w371:bool)
            n147 = Reciprocal(x=w372) -> (1/x=w361:dbl)
            n148 = Empty Array?(array=w373) -> (empty?=w374:bool)
            n149 = case shown="False" w374 {
              tunnel: w373 -> [w451 w508]
              tunnel: w361 -> [w452 _]
              tunnel: [w450 w508] -> w369
              frame False {
                n150 = for {
                  tunnel: w451 -> [w465] mode=indexing
                  tunnel: w452 -> [w455]
                  tunnel: w451 -> [w463] mode=indexing
                  tunnel: [w454] -> w450 mode=indexing
                  n151 = Unbundle By Name(w465) -> ("x"=w453:sgl, "y"=w457:sgl, "orientation"=w456:sgl, "robot_id"=w464:u32)
                  n152 = case shown="0, Default" w464 {
                    tunnel: w453 -> [w466 w476 w483 w490 w497 w504]
                    tunnel: [w472 w479 w486 w493 w500 w507] -> w462
                    tunnel: [w471 w478 w485 w492 w499 w506] -> w461
                    tunnel: [w470 w477 w484 w491 w498 w505] -> w460
                    tunnel: w457 -> [w469 w475 w482 w489 w496 w503]
                    tunnel: w456 -> [w468 w474 w481 w488 w495 w502]
                    tunnel: w455 -> [w467 w473 w480 w487 w494 w501]
                    frame 0, Default {
                      n153 = call <vilib>:"Derivative x(t) PtByPt.vi"("dt"=w467, "initial condition"=w466, "x"=w466) -> ("dx/dt"=w472:dbl)  [unwired: 1 in, 1 out]
                      n154 = call <vilib>:"Derivative x(t) PtByPt.vi"("dt"=w467, "initial condition"=w469, "x"=w469) -> ("dx/dt"=w471:dbl)  [unwired: 1 in, 1 out]
                      n155 = call <vilib>:"Derivative x(t) PtByPt.vi"("dt"=w467, "initial condition"=w468, "x"=w468) -> ("dx/dt"=w470:dbl)  [unwired: 1 in, 1 out]
                    }
                    frame 1 {
                      n156 = call <vilib>:"Derivative x(t) PtByPt.vi"("dt"=w473, "initial condition"=w476, "x"=w476) -> ("dx/dt"=w479:dbl)  [unwired: 1 in, 1 out]
                      n157 = call <vilib>:"Derivative x(t) PtByPt.vi"("dt"=w473, "initial condition"=w475, "x"=w475) -> ("dx/dt"=w478:dbl)  [unwired: 1 in, 1 out]
                      n158 = call <vilib>:"Derivative x(t) PtByPt.vi"("dt"=w473, "initial condition"=w474, "x"=w474) -> ("dx/dt"=w477:dbl)  [unwired: 1 in, 1 out]
                    }
                    frame 2 {
                      n159 = call <vilib>:"Derivative x(t) PtByPt.vi"("dt"=w480, "initial condition"=w483, "x"=w483) -> ("dx/dt"=w486:dbl)  [unwired: 1 in, 1 out]
                      n160 = call <vilib>:"Derivative x(t) PtByPt.vi"("dt"=w480, "initial condition"=w482, "x"=w482) -> ("dx/dt"=w485:dbl)  [unwired: 1 in, 1 out]
                      n161 = call <vilib>:"Derivative x(t) PtByPt.vi"("dt"=w480, "initial condition"=w481, "x"=w481) -> ("dx/dt"=w484:dbl)  [unwired: 1 in, 1 out]
                    }
                    frame 3 {
                      n162 = call <vilib>:"Derivative x(t) PtByPt.vi"("dt"=w487, "initial condition"=w490, "x"=w490) -> ("dx/dt"=w493:dbl)  [unwired: 1 in, 1 out]
                      n163 = call <vilib>:"Derivative x(t) PtByPt.vi"("dt"=w487, "initial condition"=w489, "x"=w489) -> ("dx/dt"=w492:dbl)  [unwired: 1 in, 1 out]
                      n164 = call <vilib>:"Derivative x(t) PtByPt.vi"("dt"=w487, "initial condition"=w488, "x"=w488) -> ("dx/dt"=w491:dbl)  [unwired: 1 in, 1 out]
                    }
                    frame 4 {
                      n165 = call <vilib>:"Derivative x(t) PtByPt.vi"("dt"=w494, "initial condition"=w497, "x"=w497) -> ("dx/dt"=w500:dbl)  [unwired: 1 in, 1 out]
                      n166 = call <vilib>:"Derivative x(t) PtByPt.vi"("dt"=w494, "initial condition"=w496, "x"=w496) -> ("dx/dt"=w499:dbl)  [unwired: 1 in, 1 out]
                      n167 = call <vilib>:"Derivative x(t) PtByPt.vi"("dt"=w494, "initial condition"=w495, "x"=w495) -> ("dx/dt"=w498:dbl)  [unwired: 1 in, 1 out]
                    }
                    frame 5 {
                      n168 = call <vilib>:"Derivative x(t) PtByPt.vi"("dt"=w501, "initial condition"=w504, "x"=w504) -> ("dx/dt"=w507:dbl)  [unwired: 1 in, 1 out]
                      n169 = call <vilib>:"Derivative x(t) PtByPt.vi"("dt"=w501, "initial condition"=w503, "x"=w503) -> ("dx/dt"=w506:dbl)  [unwired: 1 in, 1 out]
                      n170 = call <vilib>:"Derivative x(t) PtByPt.vi"("dt"=w501, "initial condition"=w502, "x"=w502) -> ("dx/dt"=w505:dbl)  [unwired: 1 in, 1 out]
                    }
                  }
                  n171 = Build Array(w453, w462, w457, w461, w456, w460) -> (w459:dbl[])
                  n172 = call-poly <vilib>:"Array To Matrix.vi"("Real 1D Array"=w459) -> ("Real Matrix (Column Vector)"=w458:T3)
                  n173 = Bundle By Name(cluster=w463, "x_k|k"=w458) -> (w454:T2)
                }
              }
              frame True {
              }
            }
            n174 = case shown="False" w363 {
              tunnel: w362 -> [w376 w390]
              tunnel: w361 -> [w377 _]
              tunnel: [w375 w390] -> w360
              frame False {
                n175 = for {
                  tunnel: w376 -> [w389] mode=indexing
                  tunnel: w377 -> [w378]
                  tunnel: w376 -> [w388] mode=indexing
                  tunnel: [w379] -> w375 mode=indexing
                  n176 = Unbundle By Name(w389) -> ("x"=w383:sgl, "y"=w382:sgl, "z"=w384:sgl)
                  n177 = call <vilib>:"Derivative x(t) PtByPt.vi"("dt"=w378, "initial condition"=w383, "x"=w383) -> ("dx/dt"=w387:dbl)  [unwired: 1 in, 1 out]
                  n178 = call <vilib>:"Derivative x(t) PtByPt.vi"("dt"=w378, "initial condition"=w382, "x"=w382) -> ("dx/dt"=w386:dbl)  [unwired: 1 in, 1 out]
                  n179 = call <vilib>:"Derivative x(t) PtByPt.vi"("dt"=w378, "initial condition"=w384, "x"=w384) -> ("dx/dt"=w385:dbl)  [unwired: 1 in, 1 out]
                  n180 = Build Array(w383, w387, w382, w386, w384, w385) -> (w381:dbl[])
                  n181 = call-poly <vilib>:"Array To Matrix.vi"("Real 1D Array"=w381) -> ("Real Matrix (Column Vector)"=w380:T3)
                  n182 = Bundle By Name(cluster=w388, "x_k|k"=w380) -> (w379:T4)
                }
              }
              frame True {
              }
            }
            n183 = case shown="False" w371 {
              tunnel: w370 -> [w392 w449]
              tunnel: w361 -> [w393 _]
              tunnel: [w391 w449] -> w368
              frame False {
                n184 = for {
                  tunnel: w392 -> [w406] mode=indexing
                  tunnel: w393 -> [w394]
                  tunnel: w392 -> [w404] mode=indexing
                  tunnel: [w395] -> w391 mode=indexing
                  n185 = Unbundle By Name(w406) -> ("x"=w399:sgl, "y"=w398:sgl, "orientation"=w400:sgl, "robot_id"=w405:u32)
                  n186 = case shown="0, Default" w405 {
                    tunnel: w399 -> [w410 w417 w424 w431 w438 w445]
                    tunnel: w398 -> [w408 w415 w422 w429 w436 w443]
                    tunnel: w400 -> [w407 w414 w421 w428 w435 w442]
                    tunnel: [w413 w420 w427 w434 w441 w448] -> w403
                    tunnel: [w412 w419 w426 w433 w440 w447] -> w402
                    tunnel: [w411 w418 w425 w432 w439 w446] -> w401
                    tunnel: w394 -> [w409 w416 w423 w430 w437 w444]
                    frame 0, Default {
                      n187 = call <vilib>:"Derivative x(t) PtByPt.vi"("dt"=w409, "initial condition"=w410, "x"=w410) -> ("dx/dt"=w413:dbl)  [unwired: 1 in, 1 out]
                      n188 = call <vilib>:"Derivative x(t) PtByPt.vi"("dt"=w409, "initial condition"=w408, "x"=w408) -> ("dx/dt"=w412:dbl)  [unwired: 1 in, 1 out]
                      n189 = call <vilib>:"Derivative x(t) PtByPt.vi"("dt"=w409, "initial condition"=w407, "x"=w407) -> ("dx/dt"=w411:dbl)  [unwired: 1 in, 1 out]
                    }
                    frame 1 {
                      n190 = call <vilib>:"Derivative x(t) PtByPt.vi"("dt"=w416, "initial condition"=w417, "x"=w417) -> ("dx/dt"=w420:dbl)  [unwired: 1 in, 1 out]
                      n191 = call <vilib>:"Derivative x(t) PtByPt.vi"("dt"=w416, "initial condition"=w415, "x"=w415) -> ("dx/dt"=w419:dbl)  [unwired: 1 in, 1 out]
                      n192 = call <vilib>:"Derivative x(t) PtByPt.vi"("dt"=w416, "initial condition"=w414, "x"=w414) -> ("dx/dt"=w418:dbl)  [unwired: 1 in, 1 out]
                    }
                    frame 2 {
                      n193 = call <vilib>:"Derivative x(t) PtByPt.vi"("dt"=w423, "initial condition"=w424, "x"=w424) -> ("dx/dt"=w427:dbl)  [unwired: 1 in, 1 out]
                      n194 = call <vilib>:"Derivative x(t) PtByPt.vi"("dt"=w423, "initial condition"=w422, "x"=w422) -> ("dx/dt"=w426:dbl)  [unwired: 1 in, 1 out]
                      n195 = call <vilib>:"Derivative x(t) PtByPt.vi"("dt"=w423, "initial condition"=w421, "x"=w421) -> ("dx/dt"=w425:dbl)  [unwired: 1 in, 1 out]
                    }
                    frame 3 {
                      n196 = call <vilib>:"Derivative x(t) PtByPt.vi"("dt"=w430, "initial condition"=w431, "x"=w431) -> ("dx/dt"=w434:dbl)  [unwired: 1 in, 1 out]
                      n197 = call <vilib>:"Derivative x(t) PtByPt.vi"("dt"=w430, "initial condition"=w429, "x"=w429) -> ("dx/dt"=w433:dbl)  [unwired: 1 in, 1 out]
                      n198 = call <vilib>:"Derivative x(t) PtByPt.vi"("dt"=w430, "initial condition"=w428, "x"=w428) -> ("dx/dt"=w432:dbl)  [unwired: 1 in, 1 out]
                    }
                    frame 4 {
                      n199 = call <vilib>:"Derivative x(t) PtByPt.vi"("dt"=w437, "initial condition"=w438, "x"=w438) -> ("dx/dt"=w441:dbl)  [unwired: 1 in, 1 out]
                      n200 = call <vilib>:"Derivative x(t) PtByPt.vi"("dt"=w437, "initial condition"=w436, "x"=w436) -> ("dx/dt"=w440:dbl)  [unwired: 1 in, 1 out]
                      n201 = call <vilib>:"Derivative x(t) PtByPt.vi"("dt"=w437, "initial condition"=w435, "x"=w435) -> ("dx/dt"=w439:dbl)  [unwired: 1 in, 1 out]
                    }
                    frame 5 {
                      n202 = call <vilib>:"Derivative x(t) PtByPt.vi"("dt"=w444, "initial condition"=w445, "x"=w445) -> ("dx/dt"=w448:dbl)  [unwired: 1 in, 1 out]
                      n203 = call <vilib>:"Derivative x(t) PtByPt.vi"("dt"=w444, "initial condition"=w443, "x"=w443) -> ("dx/dt"=w447:dbl)  [unwired: 1 in, 1 out]
                      n204 = call <vilib>:"Derivative x(t) PtByPt.vi"("dt"=w444, "initial condition"=w442, "x"=w442) -> ("dx/dt"=w446:dbl)  [unwired: 1 in, 1 out]
                    }
                  }
                  n205 = Build Array(w399, w403, w398, w402, w400, w401) -> (w397:dbl[])
                  n206 = call-poly <vilib>:"Array To Matrix.vi"("Real 1D Array"=w397) -> ("Real Matrix (Column Vector)"=w396:T3)
                  n207 = Bundle By Name(cluster=w404, "x_k|k"=w396) -> (w395:T2)
                }
              }
              frame True {
              }
            }
            n208 = Bundle By Name(cluster=w364, "robots_blue"=w369, "robots_yellow"=w368, "balls"=w360) -> (w367:T1)
            n209 = Bundle By Name(cluster=w364, "New"=FALSE) -> (w365:T1)
          }
          frame 3 {
            n210 = Empty Array?(array=w511) -> (empty?=w512:bool)
            n211 = Empty Array?(array=w519) -> (empty?=w520:bool)
            n212 = Reciprocal(x=w521) -> (1/x=w510:dbl)
            n213 = Empty Array?(array=w522) -> (empty?=w523:bool)
            n214 = case shown="False" w523 {
              tunnel: w522 -> [w600 w657]
              tunnel: w510 -> [w601 _]
              tunnel: [w599 w657] -> w518
              frame False {
                n215 = for {
                  tunnel: w600 -> [w614] mode=indexing
                  tunnel: w601 -> [w604]
                  tunnel: w600 -> [w612] mode=indexing
                  tunnel: [w603] -> w599 mode=indexing
                  n216 = Unbundle By Name(w614) -> ("x"=w602:sgl, "y"=w606:sgl, "orientation"=w605:sgl, "robot_id"=w613:u32)
                  n217 = case shown="3" w613 {
                    tunnel: w602 -> [w615 w625 w632 w639 w646 w653]
                    tunnel: [w621 w628 w635 w642 w649 w656] -> w611
                    tunnel: [w620 w627 w634 w641 w648 w655] -> w610
                    tunnel: [w619 w626 w633 w640 w647 w654] -> w609
                    tunnel: w606 -> [w618 w624 w631 w638 w645 w652]
                    tunnel: w605 -> [w617 w623 w630 w637 w644 w651]
                    tunnel: w604 -> [w616 w622 w629 w636 w643 w650]
                    frame 0, Default {
                      n218 = call <vilib>:"Derivative x(t) PtByPt.vi"("dt"=w616, "initial condition"=w615, "x"=w615) -> ("dx/dt"=w621:dbl)  [unwired: 1 in, 1 out]
                      n219 = call <vilib>:"Derivative x(t) PtByPt.vi"("dt"=w616, "initial condition"=w618, "x"=w618) -> ("dx/dt"=w620:dbl)  [unwired: 1 in, 1 out]
                      n220 = call <vilib>:"Derivative x(t) PtByPt.vi"("dt"=w616, "initial condition"=w617, "x"=w617) -> ("dx/dt"=w619:dbl)  [unwired: 1 in, 1 out]
                    }
                    frame 1 {
                      n221 = call <vilib>:"Derivative x(t) PtByPt.vi"("dt"=w622, "initial condition"=w625, "x"=w625) -> ("dx/dt"=w628:dbl)  [unwired: 1 in, 1 out]
                      n222 = call <vilib>:"Derivative x(t) PtByPt.vi"("dt"=w622, "initial condition"=w624, "x"=w624) -> ("dx/dt"=w627:dbl)  [unwired: 1 in, 1 out]
                      n223 = call <vilib>:"Derivative x(t) PtByPt.vi"("dt"=w622, "initial condition"=w623, "x"=w623) -> ("dx/dt"=w626:dbl)  [unwired: 1 in, 1 out]
                    }
                    frame 2 {
                      n224 = call <vilib>:"Derivative x(t) PtByPt.vi"("dt"=w629, "initial condition"=w632, "x"=w632) -> ("dx/dt"=w635:dbl)  [unwired: 1 in, 1 out]
                      n225 = call <vilib>:"Derivative x(t) PtByPt.vi"("dt"=w629, "initial condition"=w631, "x"=w631) -> ("dx/dt"=w634:dbl)  [unwired: 1 in, 1 out]
                      n226 = call <vilib>:"Derivative x(t) PtByPt.vi"("dt"=w629, "initial condition"=w630, "x"=w630) -> ("dx/dt"=w633:dbl)  [unwired: 1 in, 1 out]
                    }
                    frame 3 {
                      n227 = call <vilib>:"Derivative x(t) PtByPt.vi"("dt"=w636, "initial condition"=w639, "x"=w639) -> ("dx/dt"=w642:dbl)  [unwired: 1 in, 1 out]
                      n228 = call <vilib>:"Derivative x(t) PtByPt.vi"("dt"=w636, "initial condition"=w638, "x"=w638) -> ("dx/dt"=w641:dbl)  [unwired: 1 in, 1 out]
                      n229 = call <vilib>:"Derivative x(t) PtByPt.vi"("dt"=w636, "initial condition"=w637, "x"=w637) -> ("dx/dt"=w640:dbl)  [unwired: 1 in, 1 out]
                    }
                    frame 4 {
                      n230 = call <vilib>:"Derivative x(t) PtByPt.vi"("dt"=w643, "initial condition"=w646, "x"=w646) -> ("dx/dt"=w649:dbl)  [unwired: 1 in, 1 out]
                      n231 = call <vilib>:"Derivative x(t) PtByPt.vi"("dt"=w643, "initial condition"=w645, "x"=w645) -> ("dx/dt"=w648:dbl)  [unwired: 1 in, 1 out]
                      n232 = call <vilib>:"Derivative x(t) PtByPt.vi"("dt"=w643, "initial condition"=w644, "x"=w644) -> ("dx/dt"=w647:dbl)  [unwired: 1 in, 1 out]
                    }
                    frame 5 {
                      n233 = call <vilib>:"Derivative x(t) PtByPt.vi"("dt"=w650, "initial condition"=w653, "x"=w653) -> ("dx/dt"=w656:dbl)  [unwired: 1 in, 1 out]
                      n234 = call <vilib>:"Derivative x(t) PtByPt.vi"("dt"=w650, "initial condition"=w652, "x"=w652) -> ("dx/dt"=w655:dbl)  [unwired: 1 in, 1 out]
                      n235 = call <vilib>:"Derivative x(t) PtByPt.vi"("dt"=w650, "initial condition"=w651, "x"=w651) -> ("dx/dt"=w654:dbl)  [unwired: 1 in, 1 out]
                    }
                  }
                  n236 = Build Array(w602, w611, w606, w610, w605, w609) -> (w608:dbl[])
                  n237 = call-poly <vilib>:"Array To Matrix.vi"("Real 1D Array"=w608) -> ("Real Matrix (Column Vector)"=w607:T3)
                  n238 = Bundle By Name(cluster=w612, "x_k|k"=w607) -> (w603:T2)
                }
              }
              frame True {
              }
            }
            n239 = case shown="False" w512 {
              tunnel: w511 -> [w525 w539]
              tunnel: w510 -> [w526 _]
              tunnel: [w524 w539] -> w509
              frame False {
                n240 = for {
                  tunnel: w525 -> [w538] mode=indexing
                  tunnel: w526 -> [w527]
                  tunnel: w525 -> [w537] mode=indexing
                  tunnel: [w528] -> w524 mode=indexing
                  n241 = Unbundle By Name(w538) -> ("x"=w532:sgl, "y"=w531:sgl, "z"=w533:sgl)
                  n242 = call <vilib>:"Derivative x(t) PtByPt.vi"("dt"=w527, "initial condition"=w532, "x"=w532) -> ("dx/dt"=w536:dbl)  [unwired: 1 in, 1 out]
                  n243 = call <vilib>:"Derivative x(t) PtByPt.vi"("dt"=w527, "initial condition"=w531, "x"=w531) -> ("dx/dt"=w535:dbl)  [unwired: 1 in, 1 out]
                  n244 = call <vilib>:"Derivative x(t) PtByPt.vi"("dt"=w527, "initial condition"=w533, "x"=w533) -> ("dx/dt"=w534:dbl)  [unwired: 1 in, 1 out]
                  n245 = Build Array(w532, w536, w531, w535, w533, w534) -> (w530:dbl[])
                  n246 = call-poly <vilib>:"Array To Matrix.vi"("Real 1D Array"=w530) -> ("Real Matrix (Column Vector)"=w529:T3)
                  n247 = Bundle By Name(cluster=w537, "x_k|k"=w529) -> (w528:T4)
                }
              }
              frame True {
              }
            }
            n248 = case shown="False" w520 {
              tunnel: w519 -> [w541 w598]
              tunnel: w510 -> [w542 _]
              tunnel: [w540 w598] -> w517
              frame False {
                n249 = for {
                  tunnel: w541 -> [w555] mode=indexing
                  tunnel: w542 -> [w543]
                  tunnel: w541 -> [w553] mode=indexing
                  tunnel: [w544] -> w540 mode=indexing
                  n250 = Unbundle By Name(w555) -> ("x"=w548:sgl, "y"=w547:sgl, "orientation"=w549:sgl, "robot_id"=w554:u32)
                  n251 = case shown="0, Default" w554 {
                    tunnel: w548 -> [w559 w566 w573 w580 w587 w594]
                    tunnel: w547 -> [w557 w564 w571 w578 w585 w592]
                    tunnel: w549 -> [w556 w563 w570 w577 w584 w591]
                    tunnel: [w562 w569 w576 w583 w590 w597] -> w552
                    tunnel: [w561 w568 w575 w582 w589 w596] -> w551
                    tunnel: [w560 w567 w574 w581 w588 w595] -> w550
                    tunnel: w543 -> [w558 w565 w572 w579 w586 w593]
                    frame 0, Default {
                      n252 = call <vilib>:"Derivative x(t) PtByPt.vi"("dt"=w558, "initial condition"=w559, "x"=w559) -> ("dx/dt"=w562:dbl)  [unwired: 1 in, 1 out]
                      n253 = call <vilib>:"Derivative x(t) PtByPt.vi"("dt"=w558, "initial condition"=w557, "x"=w557) -> ("dx/dt"=w561:dbl)  [unwired: 1 in, 1 out]
                      n254 = call <vilib>:"Derivative x(t) PtByPt.vi"("dt"=w558, "initial condition"=w556, "x"=w556) -> ("dx/dt"=w560:dbl)  [unwired: 1 in, 1 out]
                    }
                    frame 1 {
                      n255 = call <vilib>:"Derivative x(t) PtByPt.vi"("dt"=w565, "initial condition"=w566, "x"=w566) -> ("dx/dt"=w569:dbl)  [unwired: 1 in, 1 out]
                      n256 = call <vilib>:"Derivative x(t) PtByPt.vi"("dt"=w565, "initial condition"=w564, "x"=w564) -> ("dx/dt"=w568:dbl)  [unwired: 1 in, 1 out]
                      n257 = call <vilib>:"Derivative x(t) PtByPt.vi"("dt"=w565, "initial condition"=w563, "x"=w563) -> ("dx/dt"=w567:dbl)  [unwired: 1 in, 1 out]
                    }
                    frame 2 {
                      n258 = call <vilib>:"Derivative x(t) PtByPt.vi"("dt"=w572, "initial condition"=w573, "x"=w573) -> ("dx/dt"=w576:dbl)  [unwired: 1 in, 1 out]
                      n259 = call <vilib>:"Derivative x(t) PtByPt.vi"("dt"=w572, "initial condition"=w571, "x"=w571) -> ("dx/dt"=w575:dbl)  [unwired: 1 in, 1 out]
                      n260 = call <vilib>:"Derivative x(t) PtByPt.vi"("dt"=w572, "initial condition"=w570, "x"=w570) -> ("dx/dt"=w574:dbl)  [unwired: 1 in, 1 out]
                    }
                    frame 3 {
                      n261 = call <vilib>:"Derivative x(t) PtByPt.vi"("dt"=w579, "initial condition"=w580, "x"=w580) -> ("dx/dt"=w583:dbl)  [unwired: 1 in, 1 out]
                      n262 = call <vilib>:"Derivative x(t) PtByPt.vi"("dt"=w579, "initial condition"=w578, "x"=w578) -> ("dx/dt"=w582:dbl)  [unwired: 1 in, 1 out]
                      n263 = call <vilib>:"Derivative x(t) PtByPt.vi"("dt"=w579, "initial condition"=w577, "x"=w577) -> ("dx/dt"=w581:dbl)  [unwired: 1 in, 1 out]
                    }
                    frame 4 {
                      n264 = call <vilib>:"Derivative x(t) PtByPt.vi"("dt"=w586, "initial condition"=w587, "x"=w587) -> ("dx/dt"=w590:dbl)  [unwired: 1 in, 1 out]
                      n265 = call <vilib>:"Derivative x(t) PtByPt.vi"("dt"=w586, "initial condition"=w585, "x"=w585) -> ("dx/dt"=w589:dbl)  [unwired: 1 in, 1 out]
                      n266 = call <vilib>:"Derivative x(t) PtByPt.vi"("dt"=w586, "initial condition"=w584, "x"=w584) -> ("dx/dt"=w588:dbl)  [unwired: 1 in, 1 out]
                    }
                    frame 5 {
                      n267 = call <vilib>:"Derivative x(t) PtByPt.vi"("dt"=w593, "initial condition"=w594, "x"=w594) -> ("dx/dt"=w597:dbl)  [unwired: 1 in, 1 out]
                      n268 = call <vilib>:"Derivative x(t) PtByPt.vi"("dt"=w593, "initial condition"=w592, "x"=w592) -> ("dx/dt"=w596:dbl)  [unwired: 1 in, 1 out]
                      n269 = call <vilib>:"Derivative x(t) PtByPt.vi"("dt"=w593, "initial condition"=w591, "x"=w591) -> ("dx/dt"=w595:dbl)  [unwired: 1 in, 1 out]
                    }
                  }
                  n270 = Build Array(w548, w552, w547, w551, w549, w550) -> (w546:dbl[])
                  n271 = call-poly <vilib>:"Array To Matrix.vi"("Real 1D Array"=w546) -> ("Real Matrix (Column Vector)"=w545:T3)
                  n272 = Bundle By Name(cluster=w553, "x_k|k"=w545) -> (w544:T2)
                }
              }
              frame True {
              }
            }
            n273 = Bundle By Name(cluster=w513, "robots_blue"=w518, "robots_yellow"=w517, "balls"=w509) -> (w516:T1)
            n274 = Bundle By Name(cluster=w513, "New"=FALSE) -> (w514:T1)
          }
        }
      }
      frame "Variable2ndDerivate" {
        n275 = call "SSL Detection Frame Simple Estimator Kalman VelCmd.vi"("Lado"=w669, "Time"=w670, "Enable"=FALSE, "Detection Frame In"=w660) -> ("Detection Frame Out"=w659:T1)  [unwired: 6 in, 1 out]
        n276 = Unbundle By Name(w659) -> ("robots_blue"=w668:T2[], "robots_yellow"=w667:T2[], "camera_id"=w664:u32, "balls"=w663:T4[], "t_capture"=w661:dbl)
        n277 = case shown="0, Default" w664 {
          tunnel: w668 -> [w685 w1212 w1739 w2266]
          tunnel: 60.0 -> [w684 w1211 w1738 w2265]
          tunnel: w667 -> [w682 w1209 w1736 w2263]
          tunnel: [w679 w1206 w1733 w2260] -> w666
          tunnel: [w677 w1204 w1731 w2258] -> w665
          tunnel: w659 -> [w676 w1203 w1730 w2257]
          tunnel: w663 -> [w674 w1201 w1728 w2255]
          tunnel: w661 -> [w671 w1198 w1725 w2252]
          frame 0, Default {
            n278 = Empty Array?(array=w674) -> (empty?=w675:bool)
            n279 = Empty Array?(array=w682) -> (empty?=w683:bool)
            n280 = Reciprocal(x=w684) -> (1/x=w673:dbl)
            n281 = Empty Array?(array=w685) -> (empty?=w686:bool)
            n282 = case shown="False" w675 {
              tunnel: w674 -> [w689 w706]
              tunnel: w673 -> [w690 _]
              tunnel: [w688 w706] -> w672
              tunnel: w671 -> [w687 _]
              frame False {
                n283 = for {
                  tunnel: w689 -> [w694] mode=indexing
                  tunnel: w690 -> [_]
                  tunnel: w689 -> [w705] mode=indexing
                  tunnel: [w703] -> w688 mode=indexing
                  tunnel: w687 -> [w693]
                  n284 = Unbundle By Name(w694) -> ("x"=w701:sgl, "y"=w699:sgl, "z"=w697:sgl)
                  n285 = call "2ndOrderDerivate.vi"("t_capture"=w693, "initial condition"=w701, "x"=w701) -> ("dx/dt"=w700:dbl)  [unwired: 5 in, 3 out]
                  n286 = call "2ndOrderDerivate.vi"("t_capture"=w693, "initial condition"=w699, "x"=w699) -> ("dx/dt"=w698:dbl)  [unwired: 5 in, 3 out]
                  n287 = call "2ndOrderDerivate.vi"("t_capture"=w693, "initial condition"=w697, "x"=w697) -> ("dx/dt"=w702:dbl)  [unwired: 5 in, 3 out]
                  n288 = call "2ndOrderDerivate.vi"("t_capture"=w693, "initial condition"=w700, "x"=w700) -> ("dx/dt"=w696:dbl)  [unwired: 5 in, 3 out]
                  n289 = call "2ndOrderDerivate.vi"("t_capture"=w693, "initial condition"=w698, "x"=w698) -> ("dx/dt"=w691:dbl)  [unwired: 5 in, 3 out]
                  n290 = call "2ndOrderDerivate.vi"("t_capture"=w693, "initial condition"=w702, "x"=w702) -> ("dx/dt"=w695:dbl)  [unwired: 5 in, 3 out]
                  n291 = Build Array(w701, w700, w699, w698, w697, w693, w696, w691, w695) -> (w692:dbl[])
                  n292 = call-poly <vilib>:"Array To Matrix.vi"("Real 1D Array"=w692) -> ("Real Matrix (Column Vector)"=w704:T3)
                  n293 = Bundle By Name(cluster=w705, "x_k|k"=w704) -> (w703:T4)
                }
              }
              frame True {
              }
            }
            n294 = case shown="False" w683 {
              tunnel: w682 -> [w709 w953]
              tunnel: w673 -> [w710 _]
              tunnel: [w708 w953] -> w680
              tunnel: w671 -> [w707 _]
              frame False {
                n295 = for {
                  tunnel: w709 -> [w728] mode=indexing
                  tunnel: w710 -> [w720]
                  tunnel: w709 -> [w727] mode=indexing
                  tunnel: [w721] -> w708 mode=indexing if=w719
                  tunnel: w707 -> [w718]
                  n296 = Unbundle By Name(w728) -> ("x"=w725:sgl, "y"=w724:sgl, "orientation"=w726:sgl, "robot_id"=w711:u32, "Valid"=w719:bool)
                  n297 = case shown="1" w711 {
                    tunnel: w725 -> [w847 w854 w861 w868 w875 w882 w889 w896 w903 w910 w917 w924 w931 w938 w945 w952]
                    tunnel: w724 -> [w845 w852 w859 w866 w873 w880 w887 w894 w901 w908 w915 w922 w929 w936 w943 w950]
                    tunnel: w726 -> [w844 w851 w858 w865 w872 w879 w886 w893 w900 w907 w914 w921 w928 w935 w942 w949]
                    tunnel: [w843 w850 w857 w864 w871 w878 w885 w892 w899 w906 w913 w920 w927 w934 w941 w948] -> w717
                    tunnel: [w842 w849 w856 w863 w870 w877 w884 w891 w898 w905 w912 w919 w926 w933 w940 w947] -> w716
                    tunnel: [w841 w848 w855 w862 w869 w876 w883 w890 w897 w904 w911 w918 w925 w932 w939 w946] -> w715
                    tunnel: w720 -> [_ _ _ _ _ _ _ _ _ _ _ _ _ _ _ _]
                    tunnel: w718 -> [w846 w853 w860 w867 w874 w881 w888 w895 w902 w909 w916 w923 w930 w937 w944 w951]
                    frame 0, Default {
                      n298 = call "2ndOrderDerivate.vi"("t_capture"=w846, "initial condition"=w847, "x"=w847) -> ("dx/dt"=w843:dbl)  [unwired: 5 in, 3 out]
                      n299 = call "2ndOrderDerivate.vi"("t_capture"=w846, "initial condition"=w845, "x"=w845) -> ("dx/dt"=w842:dbl)  [unwired: 5 in, 3 out]
                      n300 = call "2ndOrderDerivate.vi"("t_capture"=w846, "initial condition"=w844, "x"=w844) -> ("dx/dt"=w841:dbl)  [unwired: 5 in, 3 out]
                    }
                    frame 1 {
                      n301 = call "2ndOrderDerivate.vi"("t_capture"=w853, "initial condition"=w854, "x"=w854) -> ("dx/dt"=w850:dbl)  [unwired: 5 in, 3 out]
                      n302 = call "2ndOrderDerivate.vi"("t_capture"=w853, "initial condition"=w852, "x"=w852) -> ("dx/dt"=w849:dbl)  [unwired: 5 in, 3 out]
                      n303 = call "2ndOrderDerivate.vi"("t_capture"=w853, "initial condition"=w851, "x"=w851) -> ("dx/dt"=w848:dbl)  [unwired: 5 in, 3 out]
                    }
                    frame 2 {
                      n304 = call "2ndOrderDerivate.vi"("t_capture"=w860, "initial condition"=w861, "x"=w861) -> ("dx/dt"=w857:dbl)  [unwired: 5 in, 3 out]
                      n305 = call "2ndOrderDerivate.vi"("t_capture"=w860, "initial condition"=w859, "x"=w859) -> ("dx/dt"=w856:dbl)  [unwired: 5 in, 3 out]
                      n306 = call "2ndOrderDerivate.vi"("t_capture"=w860, "initial condition"=w858, "x"=w858) -> ("dx/dt"=w855:dbl)  [unwired: 5 in, 3 out]
                    }
                    frame 3 {
                      n307 = call "2ndOrderDerivate.vi"("t_capture"=w867, "initial condition"=w868, "x"=w868) -> ("dx/dt"=w864:dbl)  [unwired: 5 in, 3 out]
                      n308 = call "2ndOrderDerivate.vi"("t_capture"=w867, "initial condition"=w866, "x"=w866) -> ("dx/dt"=w863:dbl)  [unwired: 5 in, 3 out]
                      n309 = call "2ndOrderDerivate.vi"("t_capture"=w867, "initial condition"=w865, "x"=w865) -> ("dx/dt"=w862:dbl)  [unwired: 5 in, 3 out]
                    }
                    frame 4 {
                      n310 = call "2ndOrderDerivate.vi"("t_capture"=w874, "initial condition"=w875, "x"=w875) -> ("dx/dt"=w871:dbl)  [unwired: 5 in, 3 out]
                      n311 = call "2ndOrderDerivate.vi"("t_capture"=w874, "initial condition"=w873, "x"=w873) -> ("dx/dt"=w870:dbl)  [unwired: 5 in, 3 out]
                      n312 = call "2ndOrderDerivate.vi"("t_capture"=w874, "initial condition"=w872, "x"=w872) -> ("dx/dt"=w869:dbl)  [unwired: 5 in, 3 out]
                    }
                    frame 5 {
                      n313 = call "2ndOrderDerivate.vi"("t_capture"=w881, "initial condition"=w882, "x"=w882) -> ("dx/dt"=w878:dbl)  [unwired: 5 in, 3 out]
                      n314 = call "2ndOrderDerivate.vi"("t_capture"=w881, "initial condition"=w880, "x"=w880) -> ("dx/dt"=w877:dbl)  [unwired: 5 in, 3 out]
                      n315 = call "2ndOrderDerivate.vi"("t_capture"=w881, "initial condition"=w879, "x"=w879) -> ("dx/dt"=w876:dbl)  [unwired: 5 in, 3 out]
                    }
                    frame 6 {
                      n316 = call "2ndOrderDerivate.vi"("t_capture"=w888, "initial condition"=w889, "x"=w889) -> ("dx/dt"=w885:dbl)  [unwired: 5 in, 3 out]
                      n317 = call "2ndOrderDerivate.vi"("t_capture"=w888, "initial condition"=w887, "x"=w887) -> ("dx/dt"=w884:dbl)  [unwired: 5 in, 3 out]
                      n318 = call "2ndOrderDerivate.vi"("t_capture"=w888, "initial condition"=w886, "x"=w886) -> ("dx/dt"=w883:dbl)  [unwired: 5 in, 3 out]
                    }
                    frame 7 {
                      n319 = call "2ndOrderDerivate.vi"("t_capture"=w895, "initial condition"=w896, "x"=w896) -> ("dx/dt"=w892:dbl)  [unwired: 5 in, 3 out]
                      n320 = call "2ndOrderDerivate.vi"("t_capture"=w895, "initial condition"=w894, "x"=w894) -> ("dx/dt"=w891:dbl)  [unwired: 5 in, 3 out]
                      n321 = call "2ndOrderDerivate.vi"("t_capture"=w895, "initial condition"=w893, "x"=w893) -> ("dx/dt"=w890:dbl)  [unwired: 5 in, 3 out]
                    }
                    frame 8 {
                      n322 = call "2ndOrderDerivate.vi"("t_capture"=w902, "initial condition"=w903, "x"=w903) -> ("dx/dt"=w899:dbl)  [unwired: 5 in, 3 out]
                      n323 = call "2ndOrderDerivate.vi"("t_capture"=w902, "initial condition"=w901, "x"=w901) -> ("dx/dt"=w898:dbl)  [unwired: 5 in, 3 out]
                      n324 = call "2ndOrderDerivate.vi"("t_capture"=w902, "initial condition"=w900, "x"=w900) -> ("dx/dt"=w897:dbl)  [unwired: 5 in, 3 out]
                    }
                    frame 9 {
                      n325 = call "2ndOrderDerivate.vi"("t_capture"=w909, "initial condition"=w910, "x"=w910) -> ("dx/dt"=w906:dbl)  [unwired: 5 in, 3 out]
                      n326 = call "2ndOrderDerivate.vi"("t_capture"=w909, "initial condition"=w908, "x"=w908) -> ("dx/dt"=w905:dbl)  [unwired: 5 in, 3 out]
                      n327 = call "2ndOrderDerivate.vi"("t_capture"=w909, "initial condition"=w907, "x"=w907) -> ("dx/dt"=w904:dbl)  [unwired: 5 in, 3 out]
                    }
                    frame 10 {
                      n328 = call "2ndOrderDerivate.vi"("t_capture"=w916, "initial condition"=w917, "x"=w917) -> ("dx/dt"=w913:dbl)  [unwired: 5 in, 3 out]
                      n329 = call "2ndOrderDerivate.vi"("t_capture"=w916, "initial condition"=w915, "x"=w915) -> ("dx/dt"=w912:dbl)  [unwired: 5 in, 3 out]
                      n330 = call "2ndOrderDerivate.vi"("t_capture"=w916, "initial condition"=w914, "x"=w914) -> ("dx/dt"=w911:dbl)  [unwired: 5 in, 3 out]
                    }
                    frame 11 {
                      n331 = call "2ndOrderDerivate.vi"("t_capture"=w923, "initial condition"=w924, "x"=w924) -> ("dx/dt"=w920:dbl)  [unwired: 5 in, 3 out]
                      n332 = call "2ndOrderDerivate.vi"("t_capture"=w923, "initial condition"=w922, "x"=w922) -> ("dx/dt"=w919:dbl)  [unwired: 5 in, 3 out]
                      n333 = call "2ndOrderDerivate.vi"("t_capture"=w923, "initial condition"=w921, "x"=w921) -> ("dx/dt"=w918:dbl)  [unwired: 5 in, 3 out]
                    }
                    frame 12 {
                      n334 = call "2ndOrderDerivate.vi"("t_capture"=w930, "initial condition"=w931, "x"=w931) -> ("dx/dt"=w927:dbl)  [unwired: 5 in, 3 out]
                      n335 = call "2ndOrderDerivate.vi"("t_capture"=w930, "initial condition"=w929, "x"=w929) -> ("dx/dt"=w926:dbl)  [unwired: 5 in, 3 out]
                      n336 = call "2ndOrderDerivate.vi"("t_capture"=w930, "initial condition"=w928, "x"=w928) -> ("dx/dt"=w925:dbl)  [unwired: 5 in, 3 out]
                    }
                    frame 13 {
                      n337 = call "2ndOrderDerivate.vi"("t_capture"=w937, "initial condition"=w938, "x"=w938) -> ("dx/dt"=w934:dbl)  [unwired: 5 in, 3 out]
                      n338 = call "2ndOrderDerivate.vi"("t_capture"=w937, "initial condition"=w936, "x"=w936) -> ("dx/dt"=w933:dbl)  [unwired: 5 in, 3 out]
                      n339 = call "2ndOrderDerivate.vi"("t_capture"=w937, "initial condition"=w935, "x"=w935) -> ("dx/dt"=w932:dbl)  [unwired: 5 in, 3 out]
                    }
                    frame 14 {
                      n340 = call "2ndOrderDerivate.vi"("t_capture"=w944, "initial condition"=w945, "x"=w945) -> ("dx/dt"=w941:dbl)  [unwired: 5 in, 3 out]
                      n341 = call "2ndOrderDerivate.vi"("t_capture"=w944, "initial condition"=w943, "x"=w943) -> ("dx/dt"=w940:dbl)  [unwired: 5 in, 3 out]
                      n342 = call "2ndOrderDerivate.vi"("t_capture"=w944, "initial condition"=w942, "x"=w942) -> ("dx/dt"=w939:dbl)  [unwired: 5 in, 3 out]
                    }
                    frame 15 {
                      n343 = call "2ndOrderDerivate.vi"("t_capture"=w951, "initial condition"=w952, "x"=w952) -> ("dx/dt"=w948:dbl)  [unwired: 5 in, 3 out]
                      n344 = call "2ndOrderDerivate.vi"("t_capture"=w951, "initial condition"=w950, "x"=w950) -> ("dx/dt"=w947:dbl)  [unwired: 5 in, 3 out]
                      n345 = call "2ndOrderDerivate.vi"("t_capture"=w951, "initial condition"=w949, "x"=w949) -> ("dx/dt"=w946:dbl)  [unwired: 5 in, 3 out]
                    }
                  }
                  n346 = case shown="1" w711 {
                    tunnel: w717 -> [w735 w742 w749 w756 w763 w770 w777 w784 w791 w798 w805 w812 w819 w826 w833 w840]
                    tunnel: w716 -> [w733 w740 w747 w754 w761 w768 w775 w782 w789 w796 w803 w810 w817 w824 w831 w838]
                    tunnel: w715 -> [w732 w739 w746 w753 w760 w767 w774 w781 w788 w795 w802 w809 w816 w823 w830 w837]
                    tunnel: [w731 w738 w745 w752 w759 w766 w773 w780 w787 w794 w801 w808 w815 w822 w829 w836] -> w714
                    tunnel: [w730 w737 w744 w751 w758 w765 w772 w779 w786 w793 w800 w807 w814 w821 w828 w835] -> w713
                    tunnel: [w729 w736 w743 w750 w757 w764 w771 w778 w785 w792 w799 w806 w813 w820 w827 w834] -> w712
                    tunnel: w718 -> [w734 w741 w748 w755 w762 w769 w776 w783 w790 w797 w804 w811 w818 w825 w832 w839]
                    frame 0, Default {
                      n347 = call "2ndOrderDerivate.vi"("t_capture"=w734, "initial condition"=w735, "x"=w735) -> ("dx/dt"=w731:dbl)  [unwired: 5 in, 3 out]
                      n348 = call "2ndOrderDerivate.vi"("t_capture"=w734, "initial condition"=w733, "x"=w733) -> ("dx/dt"=w730:dbl)  [unwired: 5 in, 3 out]
                      n349 = call "2ndOrderDerivate.vi"("t_capture"=w734, "initial condition"=w732, "x"=w732) -> ("dx/dt"=w729:dbl)  [unwired: 5 in, 3 out]
                    }
                    frame 1 {
                      n350 = call "2ndOrderDerivate.vi"("t_capture"=w741, "initial condition"=w742, "x"=w742) -> ("dx/dt"=w738:dbl)  [unwired: 5 in, 3 out]
                      n351 = call "2ndOrderDerivate.vi"("t_capture"=w741, "initial condition"=w740, "x"=w740) -> ("dx/dt"=w737:dbl)  [unwired: 5 in, 3 out]
                      n352 = call "2ndOrderDerivate.vi"("t_capture"=w741, "initial condition"=w739, "x"=w739) -> ("dx/dt"=w736:dbl)  [unwired: 5 in, 3 out]
                    }
                    frame 2 {
                      n353 = call "2ndOrderDerivate.vi"("t_capture"=w748, "initial condition"=w749, "x"=w749) -> ("dx/dt"=w745:dbl)  [unwired: 5 in, 3 out]
                      n354 = call "2ndOrderDerivate.vi"("t_capture"=w748, "initial condition"=w747, "x"=w747) -> ("dx/dt"=w744:dbl)  [unwired: 5 in, 3 out]
                      n355 = call "2ndOrderDerivate.vi"("t_capture"=w748, "initial condition"=w746, "x"=w746) -> ("dx/dt"=w743:dbl)  [unwired: 5 in, 3 out]
                    }
                    frame 3 {
                      n356 = call "2ndOrderDerivate.vi"("t_capture"=w755, "initial condition"=w756, "x"=w756) -> ("dx/dt"=w752:dbl)  [unwired: 5 in, 3 out]
                      n357 = call "2ndOrderDerivate.vi"("t_capture"=w755, "initial condition"=w754, "x"=w754) -> ("dx/dt"=w751:dbl)  [unwired: 5 in, 3 out]
                      n358 = call "2ndOrderDerivate.vi"("t_capture"=w755, "initial condition"=w753, "x"=w753) -> ("dx/dt"=w750:dbl)  [unwired: 5 in, 3 out]
                    }
                    frame 4 {
                      n359 = call "2ndOrderDerivate.vi"("t_capture"=w762, "initial condition"=w763, "x"=w763) -> ("dx/dt"=w759:dbl)  [unwired: 5 in, 3 out]
                      n360 = call "2ndOrderDerivate.vi"("t_capture"=w762, "initial condition"=w761, "x"=w761) -> ("dx/dt"=w758:dbl)  [unwired: 5 in, 3 out]
                      n361 = call "2ndOrderDerivate.vi"("t_capture"=w762, "initial condition"=w760, "x"=w760) -> ("dx/dt"=w757:dbl)  [unwired: 5 in, 3 out]
                    }
                    frame 5 {
                      n362 = call "2ndOrderDerivate.vi"("t_capture"=w769, "initial condition"=w770, "x"=w770) -> ("dx/dt"=w766:dbl)  [unwired: 5 in, 3 out]
                      n363 = call "2ndOrderDerivate.vi"("t_capture"=w769, "initial condition"=w768, "x"=w768) -> ("dx/dt"=w765:dbl)  [unwired: 5 in, 3 out]
                      n364 = call "2ndOrderDerivate.vi"("t_capture"=w769, "initial condition"=w767, "x"=w767) -> ("dx/dt"=w764:dbl)  [unwired: 5 in, 3 out]
                    }
                    frame 6 {
                      n365 = call "2ndOrderDerivate.vi"("t_capture"=w776, "initial condition"=w777, "x"=w777) -> ("dx/dt"=w773:dbl)  [unwired: 5 in, 3 out]
                      n366 = call "2ndOrderDerivate.vi"("t_capture"=w776, "initial condition"=w775, "x"=w775) -> ("dx/dt"=w772:dbl)  [unwired: 5 in, 3 out]
                      n367 = call "2ndOrderDerivate.vi"("t_capture"=w776, "initial condition"=w774, "x"=w774) -> ("dx/dt"=w771:dbl)  [unwired: 5 in, 3 out]
                    }
                    frame 7 {
                      n368 = call "2ndOrderDerivate.vi"("t_capture"=w783, "initial condition"=w784, "x"=w784) -> ("dx/dt"=w780:dbl)  [unwired: 5 in, 3 out]
                      n369 = call "2ndOrderDerivate.vi"("t_capture"=w783, "initial condition"=w782, "x"=w782) -> ("dx/dt"=w779:dbl)  [unwired: 5 in, 3 out]
                      n370 = call "2ndOrderDerivate.vi"("t_capture"=w783, "initial condition"=w781, "x"=w781) -> ("dx/dt"=w778:dbl)  [unwired: 5 in, 3 out]
                    }
                    frame 8 {
                      n371 = call "2ndOrderDerivate.vi"("t_capture"=w790, "initial condition"=w791, "x"=w791) -> ("dx/dt"=w787:dbl)  [unwired: 5 in, 3 out]
                      n372 = call "2ndOrderDerivate.vi"("t_capture"=w790, "initial condition"=w789, "x"=w789) -> ("dx/dt"=w786:dbl)  [unwired: 5 in, 3 out]
                      n373 = call "2ndOrderDerivate.vi"("t_capture"=w790, "initial condition"=w788, "x"=w788) -> ("dx/dt"=w785:dbl)  [unwired: 5 in, 3 out]
                    }
                    frame 9 {
                      n374 = call "2ndOrderDerivate.vi"("t_capture"=w797, "initial condition"=w798, "x"=w798) -> ("dx/dt"=w794:dbl)  [unwired: 5 in, 3 out]
                      n375 = call "2ndOrderDerivate.vi"("t_capture"=w797, "initial condition"=w796, "x"=w796) -> ("dx/dt"=w793:dbl)  [unwired: 5 in, 3 out]
                      n376 = call "2ndOrderDerivate.vi"("t_capture"=w797, "initial condition"=w795, "x"=w795) -> ("dx/dt"=w792:dbl)  [unwired: 5 in, 3 out]
                    }
                    frame 10 {
                      n377 = call "2ndOrderDerivate.vi"("t_capture"=w804, "initial condition"=w805, "x"=w805) -> ("dx/dt"=w801:dbl)  [unwired: 5 in, 3 out]
                      n378 = call "2ndOrderDerivate.vi"("t_capture"=w804, "initial condition"=w803, "x"=w803) -> ("dx/dt"=w800:dbl)  [unwired: 5 in, 3 out]
                      n379 = call "2ndOrderDerivate.vi"("t_capture"=w804, "initial condition"=w802, "x"=w802) -> ("dx/dt"=w799:dbl)  [unwired: 5 in, 3 out]
                    }
                    frame 11 {
                      n380 = call "2ndOrderDerivate.vi"("t_capture"=w811, "initial condition"=w812, "x"=w812) -> ("dx/dt"=w808:dbl)  [unwired: 5 in, 3 out]
                      n381 = call "2ndOrderDerivate.vi"("t_capture"=w811, "initial condition"=w810, "x"=w810) -> ("dx/dt"=w807:dbl)  [unwired: 5 in, 3 out]
                      n382 = call "2ndOrderDerivate.vi"("t_capture"=w811, "initial condition"=w809, "x"=w809) -> ("dx/dt"=w806:dbl)  [unwired: 5 in, 3 out]
                    }
                    frame 12 {
                      n383 = call "2ndOrderDerivate.vi"("t_capture"=w818, "initial condition"=w819, "x"=w819) -> ("dx/dt"=w815:dbl)  [unwired: 5 in, 3 out]
                      n384 = call "2ndOrderDerivate.vi"("t_capture"=w818, "initial condition"=w817, "x"=w817) -> ("dx/dt"=w814:dbl)  [unwired: 5 in, 3 out]
                      n385 = call "2ndOrderDerivate.vi"("t_capture"=w818, "initial condition"=w816, "x"=w816) -> ("dx/dt"=w813:dbl)  [unwired: 5 in, 3 out]
                    }
                    frame 13 {
                      n386 = call "2ndOrderDerivate.vi"("t_capture"=w825, "initial condition"=w826, "x"=w826) -> ("dx/dt"=w822:dbl)  [unwired: 5 in, 3 out]
                      n387 = call "2ndOrderDerivate.vi"("t_capture"=w825, "initial condition"=w824, "x"=w824) -> ("dx/dt"=w821:dbl)  [unwired: 5 in, 3 out]
                      n388 = call "2ndOrderDerivate.vi"("t_capture"=w825, "initial condition"=w823, "x"=w823) -> ("dx/dt"=w820:dbl)  [unwired: 5 in, 3 out]
                    }
                    frame 14 {
                      n389 = call "2ndOrderDerivate.vi"("t_capture"=w832, "initial condition"=w833, "x"=w833) -> ("dx/dt"=w829:dbl)  [unwired: 5 in, 3 out]
                      n390 = call "2ndOrderDerivate.vi"("t_capture"=w832, "initial condition"=w831, "x"=w831) -> ("dx/dt"=w828:dbl)  [unwired: 5 in, 3 out]
                      n391 = call "2ndOrderDerivate.vi"("t_capture"=w832, "initial condition"=w830, "x"=w830) -> ("dx/dt"=w827:dbl)  [unwired: 5 in, 3 out]
                    }
                    frame 15 {
                      n392 = call "2ndOrderDerivate.vi"("t_capture"=w839, "initial condition"=w840, "x"=w840) -> ("dx/dt"=w836:dbl)  [unwired: 5 in, 3 out]
                      n393 = call "2ndOrderDerivate.vi"("t_capture"=w839, "initial condition"=w838, "x"=w838) -> ("dx/dt"=w835:dbl)  [unwired: 5 in, 3 out]
                      n394 = call "2ndOrderDerivate.vi"("t_capture"=w839, "initial condition"=w837, "x"=w837) -> ("dx/dt"=w834:dbl)  [unwired: 5 in, 3 out]
                    }
                  }
                  n395 = Build Array(w725, w717, w724, w716, w726, w715, w714, w713, w712) -> (w723:dbl[])
                  n396 = call-poly <vilib>:"Array To Matrix.vi"("Real 1D Array"=w723) -> ("Real Matrix (Column Vector)"=w722:T3)
                  n397 = Bundle By Name(cluster=w727, "x_k|k"=w722) -> (w721:T2)
                }
              }
              frame True {
              }
            }
            n398 = case shown="False" w686 {
              tunnel: w685 -> [w956 w1197]
              tunnel: w673 -> [w957 _]
              tunnel: [w955 w1197] -> w681
              tunnel: w671 -> [w954 _]
              frame False {
                n399 = for {
                  tunnel: w956 -> [w966] mode=indexing
                  tunnel: w957 -> [_]
                  tunnel: [w968] -> w955 mode=indexing
                  tunnel: w954 -> [w965]
                  n400 = Unbundle By Name(w966) -> ("x"=w967:sgl, "y"=w970:sgl, "orientation"=w969:sgl, "robot_id"=w964:u32)  [unwired: 1 out]
                  n401 = case shown="0, Default" w964 {
                    tunnel: w967 -> [w1087 w1094 w1101 w1108 w1115 w1122 w1129 w1136 w1143 w1150 w1157 w1164 w1171 w1178 w1185 w1192]
                    tunnel: [w1089 w1096 w1103 w1110 w1117 w1124 w1131 w1138 w1145 w1152 w1159 w1166 w1173 w1180 w1187 w1194] -> w963
                    tunnel: [w1091 w1098 w1105 w1112 w1119 w1126 w1133 w1140 w1147 w1154 w1161 w1168 w1175 w1182 w1189 w1196] -> w962
                    tunnel: [w1090 w1097 w1104 w1111 w1118 w1125 w1132 w1139 w1146 w1153 w1160 w1167 w1174 w1181 w1188 w1195] -> w961
                    tunnel: w970 -> [w1086 w1093 w1100 w1107 w1114 w1121 w1128 w1135 w1142 w1149 w1156 w1163 w1170 w1177 w1184 w1191]
                    tunnel: w969 -> [w1085 w1092 w1099 w1106 w1113 w1120 w1127 w1134 w1141 w1148 w1155 w1162 w1169 w1176 w1183 w1190]
                    tunnel: w965 -> [w1088 w1095 w1102 w1109 w1116 w1123 w1130 w1137 w1144 w1151 w1158 w1165 w1172 w1179 w1186 w1193]
                    frame 0, Default {
                      n402 = call "2ndOrderDerivate.vi"("t_capture"=w1088, "initial condition"=w1087, "x"=w1087) -> ("dx/dt"=w1089:dbl)  [unwired: 5 in, 3 out]
                      n403 = call "2ndOrderDerivate.vi"("t_capture"=w1088, "initial condition"=w1086, "x"=w1086) -> ("dx/dt"=w1091:dbl)  [unwired: 5 in, 3 out]
                      n404 = call "2ndOrderDerivate.vi"("t_capture"=w1088, "initial condition"=w1085, "x"=w1085) -> ("dx/dt"=w1090:dbl)  [unwired: 5 in, 3 out]
                    }
                    frame 1 {
                      n405 = call "2ndOrderDerivate.vi"("t_capture"=w1095, "initial condition"=w1094, "x"=w1094) -> ("dx/dt"=w1096:dbl)  [unwired: 5 in, 3 out]
                      n406 = call "2ndOrderDerivate.vi"("t_capture"=w1095, "initial condition"=w1093, "x"=w1093) -> ("dx/dt"=w1098:dbl)  [unwired: 5 in, 3 out]
                      n407 = call "2ndOrderDerivate.vi"("t_capture"=w1095, "initial condition"=w1092, "x"=w1092) -> ("dx/dt"=w1097:dbl)  [unwired: 5 in, 3 out]
                    }
                    frame 2 {
                      n408 = call "2ndOrderDerivate.vi"("t_capture"=w1102, "initial condition"=w1101, "x"=w1101) -> ("dx/dt"=w1103:dbl)  [unwired: 5 in, 3 out]
                      n409 = call "2ndOrderDerivate.vi"("t_capture"=w1102, "initial condition"=w1100, "x"=w1100) -> ("dx/dt"=w1105:dbl)  [unwired: 5 in, 3 out]
                      n410 = call "2ndOrderDerivate.vi"("t_capture"=w1102, "initial condition"=w1099, "x"=w1099) -> ("dx/dt"=w1104:dbl)  [unwired: 5 in, 3 out]
                    }
                    frame 3 {
                      n411 = call "2ndOrderDerivate.vi"("t_capture"=w1109, "initial condition"=w1108, "x"=w1108) -> ("dx/dt"=w1110:dbl)  [unwired: 5 in, 3 out]
                      n412 = call "2ndOrderDerivate.vi"("t_capture"=w1109, "initial condition"=w1107, "x"=w1107) -> ("dx/dt"=w1112:dbl)  [unwired: 5 in, 3 out]
                      n413 = call "2ndOrderDerivate.vi"("t_capture"=w1109, "initial condition"=w1106, "x"=w1106) -> ("dx/dt"=w1111:dbl)  [unwired: 5 in, 3 out]
                    }
                    frame 4 {
                      n414 = call "2ndOrderDerivate.vi"("t_capture"=w1116, "initial condition"=w1115, "x"=w1115) -> ("dx/dt"=w1117:dbl)  [unwired: 5 in, 3 out]
                      n415 = call "2ndOrderDerivate.vi"("t_capture"=w1116, "initial condition"=w1114, "x"=w1114) -> ("dx/dt"=w1119:dbl)  [unwired: 5 in, 3 out]
                      n416 = call "2ndOrderDerivate.vi"("t_capture"=w1116, "initial condition"=w1113, "x"=w1113) -> ("dx/dt"=w1118:dbl)  [unwired: 5 in, 3 out]
                    }
                    frame 5 {
                      n417 = call "2ndOrderDerivate.vi"("t_capture"=w1123, "initial condition"=w1122, "x"=w1122) -> ("dx/dt"=w1124:dbl)  [unwired: 5 in, 3 out]
                      n418 = call "2ndOrderDerivate.vi"("t_capture"=w1123, "initial condition"=w1121, "x"=w1121) -> ("dx/dt"=w1126:dbl)  [unwired: 5 in, 3 out]
                      n419 = call "2ndOrderDerivate.vi"("t_capture"=w1123, "initial condition"=w1120, "x"=w1120) -> ("dx/dt"=w1125:dbl)  [unwired: 5 in, 3 out]
                    }
                    frame 6 {
                      n420 = call "2ndOrderDerivate.vi"("t_capture"=w1130, "initial condition"=w1129, "x"=w1129) -> ("dx/dt"=w1131:dbl)  [unwired: 5 in, 3 out]
                      n421 = call "2ndOrderDerivate.vi"("t_capture"=w1130, "initial condition"=w1128, "x"=w1128) -> ("dx/dt"=w1133:dbl)  [unwired: 5 in, 3 out]
                      n422 = call "2ndOrderDerivate.vi"("t_capture"=w1130, "initial condition"=w1127, "x"=w1127) -> ("dx/dt"=w1132:dbl)  [unwired: 5 in, 3 out]
                    }
                    frame 7 {
                      n423 = call "2ndOrderDerivate.vi"("t_capture"=w1137, "initial condition"=w1136, "x"=w1136) -> ("dx/dt"=w1138:dbl)  [unwired: 5 in, 3 out]
                      n424 = call "2ndOrderDerivate.vi"("t_capture"=w1137, "initial condition"=w1135, "x"=w1135) -> ("dx/dt"=w1140:dbl)  [unwired: 5 in, 3 out]
                      n425 = call "2ndOrderDerivate.vi"("t_capture"=w1137, "initial condition"=w1134, "x"=w1134) -> ("dx/dt"=w1139:dbl)  [unwired: 5 in, 3 out]
                    }
                    frame 8 {
                      n426 = call "2ndOrderDerivate.vi"("t_capture"=w1144, "initial condition"=w1143, "x"=w1143) -> ("dx/dt"=w1145:dbl)  [unwired: 5 in, 3 out]
                      n427 = call "2ndOrderDerivate.vi"("t_capture"=w1144, "initial condition"=w1142, "x"=w1142) -> ("dx/dt"=w1147:dbl)  [unwired: 5 in, 3 out]
                      n428 = call "2ndOrderDerivate.vi"("t_capture"=w1144, "initial condition"=w1141, "x"=w1141) -> ("dx/dt"=w1146:dbl)  [unwired: 5 in, 3 out]
                    }
                    frame 9 {
                      n429 = call "2ndOrderDerivate.vi"("t_capture"=w1151, "initial condition"=w1150, "x"=w1150) -> ("dx/dt"=w1152:dbl)  [unwired: 5 in, 3 out]
                      n430 = call "2ndOrderDerivate.vi"("t_capture"=w1151, "initial condition"=w1149, "x"=w1149) -> ("dx/dt"=w1154:dbl)  [unwired: 5 in, 3 out]
                      n431 = call "2ndOrderDerivate.vi"("t_capture"=w1151, "initial condition"=w1148, "x"=w1148) -> ("dx/dt"=w1153:dbl)  [unwired: 5 in, 3 out]
                    }
                    frame 10 {
                      n432 = call "2ndOrderDerivate.vi"("t_capture"=w1158, "initial condition"=w1157, "x"=w1157) -> ("dx/dt"=w1159:dbl)  [unwired: 5 in, 3 out]
                      n433 = call "2ndOrderDerivate.vi"("t_capture"=w1158, "initial condition"=w1156, "x"=w1156) -> ("dx/dt"=w1161:dbl)  [unwired: 5 in, 3 out]
                      n434 = call "2ndOrderDerivate.vi"("t_capture"=w1158, "initial condition"=w1155, "x"=w1155) -> ("dx/dt"=w1160:dbl)  [unwired: 5 in, 3 out]
                    }
                    frame 11 {
                      n435 = call "2ndOrderDerivate.vi"("t_capture"=w1165, "initial condition"=w1164, "x"=w1164) -> ("dx/dt"=w1166:dbl)  [unwired: 5 in, 3 out]
                      n436 = call "2ndOrderDerivate.vi"("t_capture"=w1165, "initial condition"=w1163, "x"=w1163) -> ("dx/dt"=w1168:dbl)  [unwired: 5 in, 3 out]
                      n437 = call "2ndOrderDerivate.vi"("t_capture"=w1165, "initial condition"=w1162, "x"=w1162) -> ("dx/dt"=w1167:dbl)  [unwired: 5 in, 3 out]
                    }
                    frame 12 {
                      n438 = call "2ndOrderDerivate.vi"("t_capture"=w1172, "initial condition"=w1171, "x"=w1171) -> ("dx/dt"=w1173:dbl)  [unwired: 5 in, 3 out]
                      n439 = call "2ndOrderDerivate.vi"("t_capture"=w1172, "initial condition"=w1170, "x"=w1170) -> ("dx/dt"=w1175:dbl)  [unwired: 5 in, 3 out]
                      n440 = call "2ndOrderDerivate.vi"("t_capture"=w1172, "initial condition"=w1169, "x"=w1169) -> ("dx/dt"=w1174:dbl)  [unwired: 5 in, 3 out]
                    }
                    frame 13 {
                      n441 = call "2ndOrderDerivate.vi"("t_capture"=w1179, "initial condition"=w1178, "x"=w1178) -> ("dx/dt"=w1180:dbl)  [unwired: 5 in, 3 out]
                      n442 = call "2ndOrderDerivate.vi"("t_capture"=w1179, "initial condition"=w1177, "x"=w1177) -> ("dx/dt"=w1182:dbl)  [unwired: 5 in, 3 out]
                      n443 = call "2ndOrderDerivate.vi"("t_capture"=w1179, "initial condition"=w1176, "x"=w1176) -> ("dx/dt"=w1181:dbl)  [unwired: 5 in, 3 out]
                    }
                    frame 14 {
                      n444 = call "2ndOrderDerivate.vi"("t_capture"=w1186, "initial condition"=w1185, "x"=w1185) -> ("dx/dt"=w1187:dbl)  [unwired: 5 in, 3 out]
                      n445 = call "2ndOrderDerivate.vi"("t_capture"=w1186, "initial condition"=w1184, "x"=w1184) -> ("dx/dt"=w1189:dbl)  [unwired: 5 in, 3 out]
                      n446 = call "2ndOrderDerivate.vi"("t_capture"=w1186, "initial condition"=w1183, "x"=w1183) -> ("dx/dt"=w1188:dbl)  [unwired: 5 in, 3 out]
                    }
                    frame 15 {
                      n447 = call "2ndOrderDerivate.vi"("t_capture"=w1193, "initial condition"=w1192, "x"=w1192) -> ("dx/dt"=w1194:dbl)  [unwired: 5 in, 3 out]
                      n448 = call "2ndOrderDerivate.vi"("t_capture"=w1193, "initial condition"=w1191, "x"=w1191) -> ("dx/dt"=w1196:dbl)  [unwired: 5 in, 3 out]
                      n449 = call "2ndOrderDerivate.vi"("t_capture"=w1193, "initial condition"=w1190, "x"=w1190) -> ("dx/dt"=w1195:dbl)  [unwired: 5 in, 3 out]
                    }
                  }
                  n450 = case shown="0, Default" w964 {
                    tunnel: w963 -> [w975 w982 w989 w996 w1003 w1010 w1017 w1024 w1031 w1038 w1045 w1052 w1059 w1066 w1073 w1080]
                    tunnel: [w977 w984 w991 w998 w1005 w1012 w1019 w1026 w1033 w1040 w1047 w1054 w1061 w1068 w1075 w1082] -> w960
                    tunnel: [w979 w986 w993 w1000 w1007 w1014 w1021 w1028 w1035 w1042 w1049 w1056 w1063 w1070 w1077 w1084] -> w959
                    tunnel: [w978 w985 w992 w999 w1006 w1013 w1020 w1027 w1034 w1041 w1048 w1055 w1062 w1069 w1076 w1083] -> w958
                    tunnel: w962 -> [w974 w981 w988 w995 w1002 w1009 w1016 w1023 w1030 w1037 w1044 w1051 w1058 w1065 w1072 w1079]
                    tunnel: w961 -> [w973 w980 w987 w994 w1001 w1008 w1015 w1022 w1029 w1036 w1043 w1050 w1057 w1064 w1071 w1078]
                    tunnel: w965 -> [w976 w983 w990 w997 w1004 w1011 w1018 w1025 w1032 w1039 w1046 w1053 w1060 w1067 w1074 w1081]
                    frame 0, Default {
                      n451 = call "2ndOrderDerivate.vi"("t_capture"=w976, "initial condition"=w975, "x"=w975) -> ("dx/dt"=w977:dbl)  [unwired: 5 in, 3 out]
                      n452 = call "2ndOrderDerivate.vi"("t_capture"=w976, "initial condition"=w974, "x"=w974) -> ("dx/dt"=w979:dbl)  [unwired: 5 in, 3 out]
                      n453 = call "2ndOrderDerivate.vi"("t_capture"=w976, "initial condition"=w973, "x"=w973) -> ("dx/dt"=w978:dbl)  [unwired: 5 in, 3 out]
                    }
                    frame 1 {
                      n454 = call "2ndOrderDerivate.vi"("t_capture"=w983, "initial condition"=w982, "x"=w982) -> ("dx/dt"=w984:dbl)  [unwired: 5 in, 3 out]
                      n455 = call "2ndOrderDerivate.vi"("t_capture"=w983, "initial condition"=w981, "x"=w981) -> ("dx/dt"=w986:dbl)  [unwired: 5 in, 3 out]
                      n456 = call "2ndOrderDerivate.vi"("t_capture"=w983, "initial condition"=w980, "x"=w980) -> ("dx/dt"=w985:dbl)  [unwired: 5 in, 3 out]
                    }
                    frame 2 {
                      n457 = call "2ndOrderDerivate.vi"("t_capture"=w990, "initial condition"=w989, "x"=w989) -> ("dx/dt"=w991:dbl)  [unwired: 5 in, 3 out]
                      n458 = call "2ndOrderDerivate.vi"("t_capture"=w990, "initial condition"=w988, "x"=w988) -> ("dx/dt"=w993:dbl)  [unwired: 5 in, 3 out]
                      n459 = call "2ndOrderDerivate.vi"("t_capture"=w990, "initial condition"=w987, "x"=w987) -> ("dx/dt"=w992:dbl)  [unwired: 5 in, 3 out]
                    }
                    frame 3 {
                      n460 = call "2ndOrderDerivate.vi"("t_capture"=w997, "initial condition"=w996, "x"=w996) -> ("dx/dt"=w998:dbl)  [unwired: 5 in, 3 out]
                      n461 = call "2ndOrderDerivate.vi"("t_capture"=w997, "initial condition"=w995, "x"=w995) -> ("dx/dt"=w1000:dbl)  [unwired: 5 in, 3 out]
                      n462 = call "2ndOrderDerivate.vi"("t_capture"=w997, "initial condition"=w994, "x"=w994) -> ("dx/dt"=w999:dbl)  [unwired: 5 in, 3 out]
                    }
                    frame 4 {
                      n463 = call "2ndOrderDerivate.vi"("t_capture"=w1004, "initial condition"=w1003, "x"=w1003) -> ("dx/dt"=w1005:dbl)  [unwired: 5 in, 3 out]
                      n464 = call "2ndOrderDerivate.vi"("t_capture"=w1004, "initial condition"=w1002, "x"=w1002) -> ("dx/dt"=w1007:dbl)  [unwired: 5 in, 3 out]
                      n465 = call "2ndOrderDerivate.vi"("t_capture"=w1004, "initial condition"=w1001, "x"=w1001) -> ("dx/dt"=w1006:dbl)  [unwired: 5 in, 3 out]
                    }
                    frame 5 {
                      n466 = call "2ndOrderDerivate.vi"("t_capture"=w1011, "initial condition"=w1010, "x"=w1010) -> ("dx/dt"=w1012:dbl)  [unwired: 5 in, 3 out]
                      n467 = call "2ndOrderDerivate.vi"("t_capture"=w1011, "initial condition"=w1009, "x"=w1009) -> ("dx/dt"=w1014:dbl)  [unwired: 5 in, 3 out]
                      n468 = call "2ndOrderDerivate.vi"("t_capture"=w1011, "initial condition"=w1008, "x"=w1008) -> ("dx/dt"=w1013:dbl)  [unwired: 5 in, 3 out]
                    }
                    frame 6 {
                      n469 = call "2ndOrderDerivate.vi"("t_capture"=w1018, "initial condition"=w1017, "x"=w1017) -> ("dx/dt"=w1019:dbl)  [unwired: 5 in, 3 out]
                      n470 = call "2ndOrderDerivate.vi"("t_capture"=w1018, "initial condition"=w1016, "x"=w1016) -> ("dx/dt"=w1021:dbl)  [unwired: 5 in, 3 out]
                      n471 = call "2ndOrderDerivate.vi"("t_capture"=w1018, "initial condition"=w1015, "x"=w1015) -> ("dx/dt"=w1020:dbl)  [unwired: 5 in, 3 out]
                    }
                    frame 7 {
                      n472 = call "2ndOrderDerivate.vi"("t_capture"=w1025, "initial condition"=w1024, "x"=w1024) -> ("dx/dt"=w1026:dbl)  [unwired: 5 in, 3 out]
                      n473 = call "2ndOrderDerivate.vi"("t_capture"=w1025, "initial condition"=w1023, "x"=w1023) -> ("dx/dt"=w1028:dbl)  [unwired: 5 in, 3 out]
                      n474 = call "2ndOrderDerivate.vi"("t_capture"=w1025, "initial condition"=w1022, "x"=w1022) -> ("dx/dt"=w1027:dbl)  [unwired: 5 in, 3 out]
                    }
                    frame 8 {
                      n475 = call "2ndOrderDerivate.vi"("t_capture"=w1032, "initial condition"=w1031, "x"=w1031) -> ("dx/dt"=w1033:dbl)  [unwired: 5 in, 3 out]
                      n476 = call "2ndOrderDerivate.vi"("t_capture"=w1032, "initial condition"=w1030, "x"=w1030) -> ("dx/dt"=w1035:dbl)  [unwired: 5 in, 3 out]
                      n477 = call "2ndOrderDerivate.vi"("t_capture"=w1032, "initial condition"=w1029, "x"=w1029) -> ("dx/dt"=w1034:dbl)  [unwired: 5 in, 3 out]
                    }
                    frame 9 {
                      n478 = call "2ndOrderDerivate.vi"("t_capture"=w1039, "initial condition"=w1038, "x"=w1038) -> ("dx/dt"=w1040:dbl)  [unwired: 5 in, 3 out]
                      n479 = call "2ndOrderDerivate.vi"("t_capture"=w1039, "initial condition"=w1037, "x"=w1037) -> ("dx/dt"=w1042:dbl)  [unwired: 5 in, 3 out]
                      n480 = call "2ndOrderDerivate.vi"("t_capture"=w1039, "initial condition"=w1036, "x"=w1036) -> ("dx/dt"=w1041:dbl)  [unwired: 5 in, 3 out]
                    }
                    frame 10 {
                      n481 = call "2ndOrderDerivate.vi"("t_capture"=w1046, "initial condition"=w1045, "x"=w1045) -> ("dx/dt"=w1047:dbl)  [unwired: 5 in, 3 out]
                      n482 = call "2ndOrderDerivate.vi"("t_capture"=w1046, "initial condition"=w1044, "x"=w1044) -> ("dx/dt"=w1049:dbl)  [unwired: 5 in, 3 out]
                      n483 = call "2ndOrderDerivate.vi"("t_capture"=w1046, "initial condition"=w1043, "x"=w1043) -> ("dx/dt"=w1048:dbl)  [unwired: 5 in, 3 out]
                    }
                    frame 11 {
                      n484 = call "2ndOrderDerivate.vi"("t_capture"=w1053, "initial condition"=w1052, "x"=w1052) -> ("dx/dt"=w1054:dbl)  [unwired: 5 in, 3 out]
                      n485 = call "2ndOrderDerivate.vi"("t_capture"=w1053, "initial condition"=w1051, "x"=w1051) -> ("dx/dt"=w1056:dbl)  [unwired: 5 in, 3 out]
                      n486 = call "2ndOrderDerivate.vi"("t_capture"=w1053, "initial condition"=w1050, "x"=w1050) -> ("dx/dt"=w1055:dbl)  [unwired: 5 in, 3 out]
                    }
                    frame 12 {
                      n487 = call "2ndOrderDerivate.vi"("t_capture"=w1060, "initial condition"=w1059, "x"=w1059) -> ("dx/dt"=w1061:dbl)  [unwired: 5 in, 3 out]
                      n488 = call "2ndOrderDerivate.vi"("t_capture"=w1060, "initial condition"=w1058, "x"=w1058) -> ("dx/dt"=w1063:dbl)  [unwired: 5 in, 3 out]
                      n489 = call "2ndOrderDerivate.vi"("t_capture"=w1060, "initial condition"=w1057, "x"=w1057) -> ("dx/dt"=w1062:dbl)  [unwired: 5 in, 3 out]
                    }
                    frame 13 {
                      n490 = call "2ndOrderDerivate.vi"("t_capture"=w1067, "initial condition"=w1066, "x"=w1066) -> ("dx/dt"=w1068:dbl)  [unwired: 5 in, 3 out]
                      n491 = call "2ndOrderDerivate.vi"("t_capture"=w1067, "initial condition"=w1065, "x"=w1065) -> ("dx/dt"=w1070:dbl)  [unwired: 5 in, 3 out]
                      n492 = call "2ndOrderDerivate.vi"("t_capture"=w1067, "initial condition"=w1064, "x"=w1064) -> ("dx/dt"=w1069:dbl)  [unwired: 5 in, 3 out]
                    }
                    frame 14 {
                      n493 = call "2ndOrderDerivate.vi"("t_capture"=w1074, "initial condition"=w1073, "x"=w1073) -> ("dx/dt"=w1075:dbl)  [unwired: 5 in, 3 out]
                      n494 = call "2ndOrderDerivate.vi"("t_capture"=w1074, "initial condition"=w1072, "x"=w1072) -> ("dx/dt"=w1077:dbl)  [unwired: 5 in, 3 out]
                      n495 = call "2ndOrderDerivate.vi"("t_capture"=w1074, "initial condition"=w1071, "x"=w1071) -> ("dx/dt"=w1076:dbl)  [unwired: 5 in, 3 out]
                    }
                    frame 15 {
                      n496 = call "2ndOrderDerivate.vi"("t_capture"=w1081, "initial condition"=w1080, "x"=w1080) -> ("dx/dt"=w1082:dbl)  [unwired: 5 in, 3 out]
                      n497 = call "2ndOrderDerivate.vi"("t_capture"=w1081, "initial condition"=w1079, "x"=w1079) -> ("dx/dt"=w1084:dbl)  [unwired: 5 in, 3 out]
                      n498 = call "2ndOrderDerivate.vi"("t_capture"=w1081, "initial condition"=w1078, "x"=w1078) -> ("dx/dt"=w1083:dbl)  [unwired: 5 in, 3 out]
                    }
                  }
                  n499 = Build Array(w967, w963, w970, w962, w969, w961, w960, w959, w958) -> (w972:dbl[])
                  n500 = call-poly <vilib>:"Array To Matrix.vi"("Real 1D Array"=w972) -> ("Real Matrix (Column Vector)"=w971:T3)
                  n501 = Bundle By Name(cluster=w966, "x_k|k"=w971) -> (w968:T2)
                }
              }
              frame True {
              }
            }
            n502 = Bundle By Name(cluster=w676, "robots_blue"=w681, "robots_yellow"=w680, "balls"=w672) -> (w679:T1)
            n503 = Bundle By Name(cluster=w676, "New"=FALSE) -> (w677:T1)
          }
          frame 1 {
            n504 = Empty Array?(array=w1201) -> (empty?=w1202:bool)
            n505 = Empty Array?(array=w1209) -> (empty?=w1210:bool)
            n506 = Reciprocal(x=w1211) -> (1/x=w1200:dbl)
            n507 = Empty Array?(array=w1212) -> (empty?=w1213:bool)
            n508 = case shown="False" w1202 {
              tunnel: w1201 -> [w1216 w1233]
              tunnel: w1200 -> [w1217 _]
              tunnel: [w1215 w1233] -> w1199
              tunnel: w1198 -> [w1214 _]
              frame False {
                n509 = for {
                  tunnel: w1216 -> [w1220] mode=indexing
                  tunnel: w1217 -> [_]
                  tunnel: w1216 -> [w1232] mode=indexing
                  tunnel: [w1230] -> w1215 mode=indexing
                  tunnel: w1214 -> [w1219]
                  n510 = Unbundle By Name(w1220) -> ("x"=w1228:sgl, "y"=w1226:sgl, "z"=w1224:sgl)
                  n511 = call "2ndOrderDerivate.vi"("t_capture"=w1219, "initial condition"=w1228, "x"=w1228) -> ("dx/dt"=w1227:dbl)  [unwired: 5 in, 3 out]
                  n512 = call "2ndOrderDerivate.vi"("t_capture"=w1219, "initial condition"=w1226, "x"=w1226) -> ("dx/dt"=w1225:dbl)  [unwired: 5 in, 3 out]
                  n513 = call "2ndOrderDerivate.vi"("t_capture"=w1219, "initial condition"=w1224, "x"=w1224) -> ("dx/dt"=w1229:dbl)  [unwired: 5 in, 3 out]
                  n514 = call "2ndOrderDerivate.vi"("t_capture"=w1219, "initial condition"=w1227, "x"=w1227) -> ("dx/dt"=w1223:dbl)  [unwired: 5 in, 3 out]
                  n515 = call "2ndOrderDerivate.vi"("t_capture"=w1219, "initial condition"=w1225, "x"=w1225) -> ()  [unwired: 5 in, 4 out]
                  n516 = call "2ndOrderDerivate.vi"("t_capture"=w1219, "initial condition"=w1229, "x"=w1229) -> ("dx/dt"=w1222:dbl)  [unwired: 5 in, 3 out]
                  n517 = Build Array(w1228, w1227, w1226, w1225, w1224, w1219, w1223, 2.0 ("element"), w1222) -> (w1218:dbl[])
                  n518 = call-poly <vilib>:"Array To Matrix.vi"("Real 1D Array"=w1218) -> ("Real Matrix (Column Vector)"=w1231:T3)
                  n519 = Bundle By Name(cluster=w1232, "x_k|k"=w1231) -> (w1230:T4)
                }
              }
              frame True {
              }
            }
            n520 = case shown="False" w1210 {
              tunnel: w1209 -> [w1236 w1480]
              tunnel: w1200 -> [w1237 _]
              tunnel: [w1235 w1480] -> w1207
              tunnel: w1198 -> [w1234 _]
              frame False {
                n521 = for {
                  tunnel: w1236 -> [w1255] mode=indexing
                  tunnel: w1237 -> [w1247]
                  tunnel: w1236 -> [w1254] mode=indexing
                  tunnel: [w1248] -> w1235 mode=indexing if=w1246
                  tunnel: w1234 -> [w1245]
                  n522 = Unbundle By Name(w1255) -> ("x"=w1252:sgl, "y"=w1251:sgl, "orientation"=w1253:sgl, "robot_id"=w1238:u32, "Valid"=w1246:bool)
                  n523 = case shown="1" w1238 {
                    tunnel: w1252 -> [w1374 w1381 w1388 w1395 w1402 w1409 w1416 w1423 w1430 w1437 w1444 w1451 w1458 w1465 w1472 w1479]
                    tunnel: w1251 -> [w1372 w1379 w1386 w1393 w1400 w1407 w1414 w1421 w1428 w1435 w1442 w1449 w1456 w1463 w1470 w1477]
                    tunnel: w1253 -> [w1371 w1378 w1385 w1392 w1399 w1406 w1413 w1420 w1427 w1434 w1441 w1448 w1455 w1462 w1469 w1476]
                    tunnel: [w1370 w1377 w1384 w1391 w1398 w1405 w1412 w1419 w1426 w1433 w1440 w1447 w1454 w1461 w1468 w1475] -> w1244
                    tunnel: [w1369 w1376 w1383 w1390 w1397 w1404 w1411 w1418 w1425 w1432 w1439 w1446 w1453 w1460 w1467 w1474] -> w1243
                    tunnel: [w1368 w1375 w1382 w1389 w1396 w1403 w1410 w1417 w1424 w1431 w1438 w1445 w1452 w1459 w1466 w1473] -> w1242
                    tunnel: w1247 -> [_ _ _ _ _ _ _ _ _ _ _ _ _ _ _ _]
                    tunnel: w1245 -> [w1373 w1380 w1387 w1394 w1401 w1408 w1415 w1422 w1429 w1436 w1443 w1450 w1457 w1464 w1471 w1478]
                    frame 0, Default {
                      n524 = call "2ndOrderDerivate.vi"("t_capture"=w1373, "initial condition"=w1374, "x"=w1374) -> ("dx/dt"=w1370:dbl)  [unwired: 5 in, 3 out]
                      n525 = call "2ndOrderDerivate.vi"("t_capture"=w1373, "initial condition"=w1372, "x"=w1372) -> ("dx/dt"=w1369:dbl)  [unwired: 5 in, 3 out]
                      n526 = call "2ndOrderDerivate.vi"("t_capture"=w1373, "initial condition"=w1371, "x"=w1371) -> ("dx/dt"=w1368:dbl)  [unwired: 5 in, 3 out]
                    }
                    frame 1 {
                      n527 = call "2ndOrderDerivate.vi"("t_capture"=w1380, "initial condition"=w1381, "x"=w1381) -> ("dx/dt"=w1377:dbl)  [unwired: 5 in, 3 out]
                      n528 = call "2ndOrderDerivate.vi"("t_capture"=w1380, "initial condition"=w1379, "x"=w1379) -> ("dx/dt"=w1376:dbl)  [unwired: 5 in, 3 out]
                      n529 = call "2ndOrderDerivate.vi"("t_capture"=w1380, "initial condition"=w1378, "x"=w1378) -> ("dx/dt"=w1375:dbl)  [unwired: 5 in, 3 out]
                    }
                    frame 2 {
                      n530 = call "2ndOrderDerivate.vi"("t_capture"=w1387, "initial condition"=w1388, "x"=w1388) -> ("dx/dt"=w1384:dbl)  [unwired: 5 in, 3 out]
                      n531 = call "2ndOrderDerivate.vi"("t_capture"=w1387, "initial condition"=w1386, "x"=w1386) -> ("dx/dt"=w1383:dbl)  [unwired: 5 in, 3 out]
                      n532 = call "2ndOrderDerivate.vi"("t_capture"=w1387, "initial condition"=w1385, "x"=w1385) -> ("dx/dt"=w1382:dbl)  [unwired: 5 in, 3 out]
                    }
                    frame 3 {
                      n533 = call "2ndOrderDerivate.vi"("t_capture"=w1394, "initial condition"=w1395, "x"=w1395) -> ("dx/dt"=w1391:dbl)  [unwired: 5 in, 3 out]
                      n534 = call "2ndOrderDerivate.vi"("t_capture"=w1394, "initial condition"=w1393, "x"=w1393) -> ("dx/dt"=w1390:dbl)  [unwired: 5 in, 3 out]
                      n535 = call "2ndOrderDerivate.vi"("t_capture"=w1394, "initial condition"=w1392, "x"=w1392) -> ("dx/dt"=w1389:dbl)  [unwired: 5 in, 3 out]
                    }
                    frame 4 {
                      n536 = call "2ndOrderDerivate.vi"("t_capture"=w1401, "initial condition"=w1402, "x"=w1402) -> ("dx/dt"=w1398:dbl)  [unwired: 5 in, 3 out]
                      n537 = call "2ndOrderDerivate.vi"("t_capture"=w1401, "initial condition"=w1400, "x"=w1400) -> ("dx/dt"=w1397:dbl)  [unwired: 5 in, 3 out]
                      n538 = call "2ndOrderDerivate.vi"("t_capture"=w1401, "initial condition"=w1399, "x"=w1399) -> ("dx/dt"=w1396:dbl)  [unwired: 5 in, 3 out]
                    }
                    frame 5 {
                      n539 = call "2ndOrderDerivate.vi"("t_capture"=w1408, "initial condition"=w1409, "x"=w1409) -> ("dx/dt"=w1405:dbl)  [unwired: 5 in, 3 out]
                      n540 = call "2ndOrderDerivate.vi"("t_capture"=w1408, "initial condition"=w1407, "x"=w1407) -> ("dx/dt"=w1404:dbl)  [unwired: 5 in, 3 out]
                      n541 = call "2ndOrderDerivate.vi"("t_capture"=w1408, "initial condition"=w1406, "x"=w1406) -> ("dx/dt"=w1403:dbl)  [unwired: 5 in, 3 out]
                    }
                    frame 6 {
                      n542 = call "2ndOrderDerivate.vi"("t_capture"=w1415, "initial condition"=w1416, "x"=w1416) -> ("dx/dt"=w1412:dbl)  [unwired: 5 in, 3 out]
                      n543 = call "2ndOrderDerivate.vi"("t_capture"=w1415, "initial condition"=w1414, "x"=w1414) -> ("dx/dt"=w1411:dbl)  [unwired: 5 in, 3 out]
                      n544 = call "2ndOrderDerivate.vi"("t_capture"=w1415, "initial condition"=w1413, "x"=w1413) -> ("dx/dt"=w1410:dbl)  [unwired: 5 in, 3 out]
                    }
                    frame 7 {
                      n545 = call "2ndOrderDerivate.vi"("t_capture"=w1422, "initial condition"=w1423, "x"=w1423) -> ("dx/dt"=w1419:dbl)  [unwired: 5 in, 3 out]
                      n546 = call "2ndOrderDerivate.vi"("t_capture"=w1422, "initial condition"=w1421, "x"=w1421) -> ("dx/dt"=w1418:dbl)  [unwired: 5 in, 3 out]
                      n547 = call "2ndOrderDerivate.vi"("t_capture"=w1422, "initial condition"=w1420, "x"=w1420) -> ("dx/dt"=w1417:dbl)  [unwired: 5 in, 3 out]
                    }
                    frame 8 {
                      n548 = call "2ndOrderDerivate.vi"("t_capture"=w1429, "initial condition"=w1430, "x"=w1430) -> ("dx/dt"=w1426:dbl)  [unwired: 5 in, 3 out]
                      n549 = call "2ndOrderDerivate.vi"("t_capture"=w1429, "initial condition"=w1428, "x"=w1428) -> ("dx/dt"=w1425:dbl)  [unwired: 5 in, 3 out]
                      n550 = call "2ndOrderDerivate.vi"("t_capture"=w1429, "initial condition"=w1427, "x"=w1427) -> ("dx/dt"=w1424:dbl)  [unwired: 5 in, 3 out]
                    }
                    frame 9 {
                      n551 = call "2ndOrderDerivate.vi"("t_capture"=w1436, "initial condition"=w1437, "x"=w1437) -> ("dx/dt"=w1433:dbl)  [unwired: 5 in, 3 out]
                      n552 = call "2ndOrderDerivate.vi"("t_capture"=w1436, "initial condition"=w1435, "x"=w1435) -> ("dx/dt"=w1432:dbl)  [unwired: 5 in, 3 out]
                      n553 = call "2ndOrderDerivate.vi"("t_capture"=w1436, "initial condition"=w1434, "x"=w1434) -> ("dx/dt"=w1431:dbl)  [unwired: 5 in, 3 out]
                    }
                    frame 10 {
                      n554 = call "2ndOrderDerivate.vi"("t_capture"=w1443, "initial condition"=w1444, "x"=w1444) -> ("dx/dt"=w1440:dbl)  [unwired: 5 in, 3 out]
                      n555 = call "2ndOrderDerivate.vi"("t_capture"=w1443, "initial condition"=w1442, "x"=w1442) -> ("dx/dt"=w1439:dbl)  [unwired: 5 in, 3 out]
                      n556 = call "2ndOrderDerivate.vi"("t_capture"=w1443, "initial condition"=w1441, "x"=w1441) -> ("dx/dt"=w1438:dbl)  [unwired: 5 in, 3 out]
                    }
                    frame 11 {
                      n557 = call "2ndOrderDerivate.vi"("t_capture"=w1450, "initial condition"=w1451, "x"=w1451) -> ("dx/dt"=w1447:dbl)  [unwired: 5 in, 3 out]
                      n558 = call "2ndOrderDerivate.vi"("t_capture"=w1450, "initial condition"=w1449, "x"=w1449) -> ("dx/dt"=w1446:dbl)  [unwired: 5 in, 3 out]
                      n559 = call "2ndOrderDerivate.vi"("t_capture"=w1450, "initial condition"=w1448, "x"=w1448) -> ("dx/dt"=w1445:dbl)  [unwired: 5 in, 3 out]
                    }
                    frame 12 {
                      n560 = call "2ndOrderDerivate.vi"("t_capture"=w1457, "initial condition"=w1458, "x"=w1458) -> ("dx/dt"=w1454:dbl)  [unwired: 5 in, 3 out]
                      n561 = call "2ndOrderDerivate.vi"("t_capture"=w1457, "initial condition"=w1456, "x"=w1456) -> ("dx/dt"=w1453:dbl)  [unwired: 5 in, 3 out]
                      n562 = call "2ndOrderDerivate.vi"("t_capture"=w1457, "initial condition"=w1455, "x"=w1455) -> ("dx/dt"=w1452:dbl)  [unwired: 5 in, 3 out]
                    }
                    frame 13 {
                      n563 = call "2ndOrderDerivate.vi"("t_capture"=w1464, "initial condition"=w1465, "x"=w1465) -> ("dx/dt"=w1461:dbl)  [unwired: 5 in, 3 out]
                      n564 = call "2ndOrderDerivate.vi"("t_capture"=w1464, "initial condition"=w1463, "x"=w1463) -> ("dx/dt"=w1460:dbl)  [unwired: 5 in, 3 out]
                      n565 = call "2ndOrderDerivate.vi"("t_capture"=w1464, "initial condition"=w1462, "x"=w1462) -> ("dx/dt"=w1459:dbl)  [unwired: 5 in, 3 out]
                    }
                    frame 14 {
                      n566 = call "2ndOrderDerivate.vi"("t_capture"=w1471, "initial condition"=w1472, "x"=w1472) -> ("dx/dt"=w1468:dbl)  [unwired: 5 in, 3 out]
                      n567 = call "2ndOrderDerivate.vi"("t_capture"=w1471, "initial condition"=w1470, "x"=w1470) -> ("dx/dt"=w1467:dbl)  [unwired: 5 in, 3 out]
                      n568 = call "2ndOrderDerivate.vi"("t_capture"=w1471, "initial condition"=w1469, "x"=w1469) -> ("dx/dt"=w1466:dbl)  [unwired: 5 in, 3 out]
                    }
                    frame 15 {
                      n569 = call "2ndOrderDerivate.vi"("t_capture"=w1478, "initial condition"=w1479, "x"=w1479) -> ("dx/dt"=w1475:dbl)  [unwired: 5 in, 3 out]
                      n570 = call "2ndOrderDerivate.vi"("t_capture"=w1478, "initial condition"=w1477, "x"=w1477) -> ("dx/dt"=w1474:dbl)  [unwired: 5 in, 3 out]
                      n571 = call "2ndOrderDerivate.vi"("t_capture"=w1478, "initial condition"=w1476, "x"=w1476) -> ("dx/dt"=w1473:dbl)  [unwired: 5 in, 3 out]
                    }
                  }
                  n572 = case shown="1" w1238 {
                    tunnel: w1244 -> [w1262 w1269 w1276 w1283 w1290 w1297 w1304 w1311 w1318 w1325 w1332 w1339 w1346 w1353 w1360 w1367]
                    tunnel: w1243 -> [w1260 w1267 w1274 w1281 w1288 w1295 w1302 w1309 w1316 w1323 w1330 w1337 w1344 w1351 w1358 w1365]
                    tunnel: w1242 -> [w1259 w1266 w1273 w1280 w1287 w1294 w1301 w1308 w1315 w1322 w1329 w1336 w1343 w1350 w1357 w1364]
                    tunnel: [w1258 w1265 w1272 w1279 w1286 w1293 w1300 w1307 w1314 w1321 w1328 w1335 w1342 w1349 w1356 w1363] -> w1241
                    tunnel: [w1257 w1264 w1271 w1278 w1285 w1292 w1299 w1306 w1313 w1320 w1327 w1334 w1341 w1348 w1355 w1362] -> w1240
                    tunnel: [w1256 w1263 w1270 w1277 w1284 w1291 w1298 w1305 w1312 w1319 w1326 w1333 w1340 w1347 w1354 w1361] -> w1239
                    tunnel: w1245 -> [w1261 w1268 w1275 w1282 w1289 w1296 w1303 w1310 w1317 w1324 w1331 w1338 w1345 w1352 w1359 w1366]
                    frame 0, Default {
                      n573 = call "2ndOrderDerivate.vi"("t_capture"=w1261, "initial condition"=w1262, "x"=w1262) -> ("dx/dt"=w1258:dbl)  [unwired: 5 in, 3 out]
                      n574 = call "2ndOrderDerivate.vi"("t_capture"=w1261, "initial condition"=w1260, "x"=w1260) -> ("dx/dt"=w1257:dbl)  [unwired: 5 in, 3 out]
                      n575 = call "2ndOrderDerivate.vi"("t_capture"=w1261, "initial condition"=w1259, "x"=w1259) -> ("dx/dt"=w1256:dbl)  [unwired: 5 in, 3 out]
                    }
                    frame 1 {
                      n576 = call "2ndOrderDerivate.vi"("t_capture"=w1268, "initial condition"=w1269, "x"=w1269) -> ("dx/dt"=w1265:dbl)  [unwired: 5 in, 3 out]
                      n577 = call "2ndOrderDerivate.vi"("t_capture"=w1268, "initial condition"=w1267, "x"=w1267) -> ("dx/dt"=w1264:dbl)  [unwired: 5 in, 3 out]
                      n578 = call "2ndOrderDerivate.vi"("t_capture"=w1268, "initial condition"=w1266, "x"=w1266) -> ("dx/dt"=w1263:dbl)  [unwired: 5 in, 3 out]
                    }
                    frame 2 {
                      n579 = call "2ndOrderDerivate.vi"("t_capture"=w1275, "initial condition"=w1276, "x"=w1276) -> ("dx/dt"=w1272:dbl)  [unwired: 5 in, 3 out]
                      n580 = call "2ndOrderDerivate.vi"("t_capture"=w1275, "initial condition"=w1274, "x"=w1274) -> ("dx/dt"=w1271:dbl)  [unwired: 5 in, 3 out]
                      n581 = call "2ndOrderDerivate.vi"("t_capture"=w1275, "initial condition"=w1273, "x"=w1273) -> ("dx/dt"=w1270:dbl)  [unwired: 5 in, 3 out]
                    }
                    frame 3 {
                      n582 = call "2ndOrderDerivate.vi"("t_capture"=w1282, "initial condition"=w1283, "x"=w1283) -> ("dx/dt"=w1279:dbl)  [unwired: 5 in, 3 out]
                      n583 = call "2ndOrderDerivate.vi"("t_capture"=w1282, "initial condition"=w1281, "x"=w1281) -> ("dx/dt"=w1278:dbl)  [unwired: 5 in, 3 out]
                      n584 = call "2ndOrderDerivate.vi"("t_capture"=w1282, "initial condition"=w1280, "x"=w1280) -> ("dx/dt"=w1277:dbl)  [unwired: 5 in, 3 out]
                    }
                    frame 4 {
                      n585 = call "2ndOrderDerivate.vi"("t_capture"=w1289, "initial condition"=w1290, "x"=w1290) -> ("dx/dt"=w1286:dbl)  [unwired: 5 in, 3 out]
                      n586 = call "2ndOrderDerivate.vi"("t_capture"=w1289, "initial condition"=w1288, "x"=w1288) -> ("dx/dt"=w1285:dbl)  [unwired: 5 in, 3 out]
                      n587 = call "2ndOrderDerivate.vi"("t_capture"=w1289, "initial condition"=w1287, "x"=w1287) -> ("dx/dt"=w1284:dbl)  [unwired: 5 in, 3 out]
                    }
                    frame 5 {
                      n588 = call "2ndOrderDerivate.vi"("t_capture"=w1296, "initial condition"=w1297, "x"=w1297) -> ("dx/dt"=w1293:dbl)  [unwired: 5 in, 3 out]
                      n589 = call "2ndOrderDerivate.vi"("t_capture"=w1296, "initial condition"=w1295, "x"=w1295) -> ("dx/dt"=w1292:dbl)  [unwired: 5 in, 3 out]
                      n590 = call "2ndOrderDerivate.vi"("t_capture"=w1296, "initial condition"=w1294, "x"=w1294) -> ("dx/dt"=w1291:dbl)  [unwired: 5 in, 3 out]
                    }
                    frame 6 {
                      n591 = call "2ndOrderDerivate.vi"("t_capture"=w1303, "initial condition"=w1304, "x"=w1304) -> ("dx/dt"=w1300:dbl)  [unwired: 5 in, 3 out]
                      n592 = call "2ndOrderDerivate.vi"("t_capture"=w1303, "initial condition"=w1302, "x"=w1302) -> ("dx/dt"=w1299:dbl)  [unwired: 5 in, 3 out]
                      n593 = call "2ndOrderDerivate.vi"("t_capture"=w1303, "initial condition"=w1301, "x"=w1301) -> ("dx/dt"=w1298:dbl)  [unwired: 5 in, 3 out]
                    }
                    frame 7 {
                      n594 = call "2ndOrderDerivate.vi"("t_capture"=w1310, "initial condition"=w1311, "x"=w1311) -> ("dx/dt"=w1307:dbl)  [unwired: 5 in, 3 out]
                      n595 = call "2ndOrderDerivate.vi"("t_capture"=w1310, "initial condition"=w1309, "x"=w1309) -> ("dx/dt"=w1306:dbl)  [unwired: 5 in, 3 out]
                      n596 = call "2ndOrderDerivate.vi"("t_capture"=w1310, "initial condition"=w1308, "x"=w1308) -> ("dx/dt"=w1305:dbl)  [unwired: 5 in, 3 out]
                    }
                    frame 8 {
                      n597 = call "2ndOrderDerivate.vi"("t_capture"=w1317, "initial condition"=w1318, "x"=w1318) -> ("dx/dt"=w1314:dbl)  [unwired: 5 in, 3 out]
                      n598 = call "2ndOrderDerivate.vi"("t_capture"=w1317, "initial condition"=w1316, "x"=w1316) -> ("dx/dt"=w1313:dbl)  [unwired: 5 in, 3 out]
                      n599 = call "2ndOrderDerivate.vi"("t_capture"=w1317, "initial condition"=w1315, "x"=w1315) -> ("dx/dt"=w1312:dbl)  [unwired: 5 in, 3 out]
                    }
                    frame 9 {
                      n600 = call "2ndOrderDerivate.vi"("t_capture"=w1324, "initial condition"=w1325, "x"=w1325) -> ("dx/dt"=w1321:dbl)  [unwired: 5 in, 3 out]
                      n601 = call "2ndOrderDerivate.vi"("t_capture"=w1324, "initial condition"=w1323, "x"=w1323) -> ("dx/dt"=w1320:dbl)  [unwired: 5 in, 3 out]
                      n602 = call "2ndOrderDerivate.vi"("t_capture"=w1324, "initial condition"=w1322, "x"=w1322) -> ("dx/dt"=w1319:dbl)  [unwired: 5 in, 3 out]
                    }
                    frame 10 {
                      n603 = call "2ndOrderDerivate.vi"("t_capture"=w1331, "initial condition"=w1332, "x"=w1332) -> ("dx/dt"=w1328:dbl)  [unwired: 5 in, 3 out]
                      n604 = call "2ndOrderDerivate.vi"("t_capture"=w1331, "initial condition"=w1330, "x"=w1330) -> ("dx/dt"=w1327:dbl)  [unwired: 5 in, 3 out]
                      n605 = call "2ndOrderDerivate.vi"("t_capture"=w1331, "initial condition"=w1329, "x"=w1329) -> ("dx/dt"=w1326:dbl)  [unwired: 5 in, 3 out]
                    }
                    frame 11 {
                      n606 = call "2ndOrderDerivate.vi"("t_capture"=w1338, "initial condition"=w1339, "x"=w1339) -> ("dx/dt"=w1335:dbl)  [unwired: 5 in, 3 out]
                      n607 = call "2ndOrderDerivate.vi"("t_capture"=w1338, "initial condition"=w1337, "x"=w1337) -> ("dx/dt"=w1334:dbl)  [unwired: 5 in, 3 out]
                      n608 = call "2ndOrderDerivate.vi"("t_capture"=w1338, "initial condition"=w1336, "x"=w1336) -> ("dx/dt"=w1333:dbl)  [unwired: 5 in, 3 out]
                    }
                    frame 12 {
                      n609 = call "2ndOrderDerivate.vi"("t_capture"=w1345, "initial condition"=w1346, "x"=w1346) -> ("dx/dt"=w1342:dbl)  [unwired: 5 in, 3 out]
                      n610 = call "2ndOrderDerivate.vi"("t_capture"=w1345, "initial condition"=w1344, "x"=w1344) -> ("dx/dt"=w1341:dbl)  [unwired: 5 in, 3 out]
                      n611 = call "2ndOrderDerivate.vi"("t_capture"=w1345, "initial condition"=w1343, "x"=w1343) -> ("dx/dt"=w1340:dbl)  [unwired: 5 in, 3 out]
                    }
                    frame 13 {
                      n612 = call "2ndOrderDerivate.vi"("t_capture"=w1352, "initial condition"=w1353, "x"=w1353) -> ("dx/dt"=w1349:dbl)  [unwired: 5 in, 3 out]
                      n613 = call "2ndOrderDerivate.vi"("t_capture"=w1352, "initial condition"=w1351, "x"=w1351) -> ("dx/dt"=w1348:dbl)  [unwired: 5 in, 3 out]
                      n614 = call "2ndOrderDerivate.vi"("t_capture"=w1352, "initial condition"=w1350, "x"=w1350) -> ("dx/dt"=w1347:dbl)  [unwired: 5 in, 3 out]
                    }
                    frame 14 {
                      n615 = call "2ndOrderDerivate.vi"("t_capture"=w1359, "initial condition"=w1360, "x"=w1360) -> ("dx/dt"=w1356:dbl)  [unwired: 5 in, 3 out]
                      n616 = call "2ndOrderDerivate.vi"("t_capture"=w1359, "initial condition"=w1358, "x"=w1358) -> ("dx/dt"=w1355:dbl)  [unwired: 5 in, 3 out]
                      n617 = call "2ndOrderDerivate.vi"("t_capture"=w1359, "initial condition"=w1357, "x"=w1357) -> ("dx/dt"=w1354:dbl)  [unwired: 5 in, 3 out]
                    }
                    frame 15 {
                      n618 = call "2ndOrderDerivate.vi"("t_capture"=w1366, "initial condition"=w1367, "x"=w1367) -> ("dx/dt"=w1363:dbl)  [unwired: 5 in, 3 out]
                      n619 = call "2ndOrderDerivate.vi"("t_capture"=w1366, "initial condition"=w1365, "x"=w1365) -> ("dx/dt"=w1362:dbl)  [unwired: 5 in, 3 out]
                      n620 = call "2ndOrderDerivate.vi"("t_capture"=w1366, "initial condition"=w1364, "x"=w1364) -> ("dx/dt"=w1361:dbl)  [unwired: 5 in, 3 out]
                    }
                  }
                  n621 = Build Array(w1252, w1244, w1251, w1243, w1253, w1242, w1241, w1240, w1239) -> (w1250:dbl[])
                  n622 = call-poly <vilib>:"Array To Matrix.vi"("Real 1D Array"=w1250) -> ("Real Matrix (Column Vector)"=w1249:T3)
                  n623 = Bundle By Name(cluster=w1254, "x_k|k"=w1249) -> (w1248:T2)
                }
              }
              frame True {
              }
            }
            n624 = case shown="False" w1213 {
              tunnel: w1212 -> [w1483 w1724]
              tunnel: w1200 -> [w1484 _]
              tunnel: [w1482 w1724] -> w1208
              tunnel: w1198 -> [w1481 _]
              frame False {
                n625 = for {
                  tunnel: w1483 -> [w1493] mode=indexing
                  tunnel: w1484 -> [_]
                  tunnel: [w1495] -> w1482 mode=indexing
                  tunnel: w1481 -> [w1492]
                  n626 = Unbundle By Name(w1493) -> ("x"=w1494:sgl, "y"=w1497:sgl, "orientation"=w1496:sgl, "robot_id"=w1491:u32)  [unwired: 1 out]
                  n627 = case shown="0, Default" w1491 {
                    tunnel: w1494 -> [w1614 w1621 w1628 w1635 w1642 w1649 w1656 w1663 w1670 w1677 w1684 w1691 w1698 w1705 w1712 w1719]
                    tunnel: [w1616 w1623 w1630 w1637 w1644 w1651 w1658 w1665 w1672 w1679 w1686 w1693 w1700 w1707 w1714 w1721] -> w1490
                    tunnel: [w1618 w1625 w1632 w1639 w1646 w1653 w1660 w1667 w1674 w1681 w1688 w1695 w1702 w1709 w1716 w1723] -> w1489
                    tunnel: [w1617 w1624 w1631 w1638 w1645 w1652 w1659 w1666 w1673 w1680 w1687 w1694 w1701 w1708 w1715 w1722] -> w1488
                    tunnel: w1497 -> [w1613 w1620 w1627 w1634 w1641 w1648 w1655 w1662 w1669 w1676 w1683 w1690 w1697 w1704 w1711 w1718]
                    tunnel: w1496 -> [w1612 w1619 w1626 w1633 w1640 w1647 w1654 w1661 w1668 w1675 w1682 w1689 w1696 w1703 w1710 w1717]
                    tunnel: w1492 -> [w1615 w1622 w1629 w1636 w1643 w1650 w1657 w1664 w1671 w1678 w1685 w1692 w1699 w1706 w1713 w1720]
                    frame 0, Default {
                      n628 = call "2ndOrderDerivate.vi"("t_capture"=w1615, "initial condition"=w1614, "x"=w1614) -> ("dx/dt"=w1616:dbl)  [unwired: 5 in, 3 out]
                      n629 = call "2ndOrderDerivate.vi"("t_capture"=w1615, "initial condition"=w1613, "x"=w1613) -> ("dx/dt"=w1618:dbl)  [unwired: 5 in, 3 out]
                      n630 = call "2ndOrderDerivate.vi"("t_capture"=w1615, "initial condition"=w1612, "x"=w1612) -> ("dx/dt"=w1617:dbl)  [unwired: 5 in, 3 out]
                    }
                    frame 1 {
                      n631 = call "2ndOrderDerivate.vi"("t_capture"=w1622, "initial condition"=w1621, "x"=w1621) -> ("dx/dt"=w1623:dbl)  [unwired: 5 in, 3 out]
                      n632 = call "2ndOrderDerivate.vi"("t_capture"=w1622, "initial condition"=w1620, "x"=w1620) -> ("dx/dt"=w1625:dbl)  [unwired: 5 in, 3 out]
                      n633 = call "2ndOrderDerivate.vi"("t_capture"=w1622, "initial condition"=w1619, "x"=w1619) -> ("dx/dt"=w1624:dbl)  [unwired: 5 in, 3 out]
                    }
                    frame 2 {
                      n634 = call "2ndOrderDerivate.vi"("t_capture"=w1629, "initial condition"=w1628, "x"=w1628) -> ("dx/dt"=w1630:dbl)  [unwired: 5 in, 3 out]
                      n635 = call "2ndOrderDerivate.vi"("t_capture"=w1629, "initial condition"=w1627, "x"=w1627) -> ("dx/dt"=w1632:dbl)  [unwired: 5 in, 3 out]
                      n636 = call "2ndOrderDerivate.vi"("t_capture"=w1629, "initial condition"=w1626, "x"=w1626) -> ("dx/dt"=w1631:dbl)  [unwired: 5 in, 3 out]
                    }
                    frame 3 {
                      n637 = call "2ndOrderDerivate.vi"("t_capture"=w1636, "initial condition"=w1635, "x"=w1635) -> ("dx/dt"=w1637:dbl)  [unwired: 5 in, 3 out]
                      n638 = call "2ndOrderDerivate.vi"("t_capture"=w1636, "initial condition"=w1634, "x"=w1634) -> ("dx/dt"=w1639:dbl)  [unwired: 5 in, 3 out]
                      n639 = call "2ndOrderDerivate.vi"("t_capture"=w1636, "initial condition"=w1633, "x"=w1633) -> ("dx/dt"=w1638:dbl)  [unwired: 5 in, 3 out]
                    }
                    frame 4 {
                      n640 = call "2ndOrderDerivate.vi"("t_capture"=w1643, "initial condition"=w1642, "x"=w1642) -> ("dx/dt"=w1644:dbl)  [unwired: 5 in, 3 out]
                      n641 = call "2ndOrderDerivate.vi"("t_capture"=w1643, "initial condition"=w1641, "x"=w1641) -> ("dx/dt"=w1646:dbl)  [unwired: 5 in, 3 out]
                      n642 = call "2ndOrderDerivate.vi"("t_capture"=w1643, "initial condition"=w1640, "x"=w1640) -> ("dx/dt"=w1645:dbl)  [unwired: 5 in, 3 out]
                    }
                    frame 5 {
                      n643 = call "2ndOrderDerivate.vi"("t_capture"=w1650, "initial condition"=w1649, "x"=w1649) -> ("dx/dt"=w1651:dbl)  [unwired: 5 in, 3 out]
                      n644 = call "2ndOrderDerivate.vi"("t_capture"=w1650, "initial condition"=w1648, "x"=w1648) -> ("dx/dt"=w1653:dbl)  [unwired: 5 in, 3 out]
                      n645 = call "2ndOrderDerivate.vi"("t_capture"=w1650, "initial condition"=w1647, "x"=w1647) -> ("dx/dt"=w1652:dbl)  [unwired: 5 in, 3 out]
                    }
                    frame 6 {
                      n646 = call "2ndOrderDerivate.vi"("t_capture"=w1657, "initial condition"=w1656, "x"=w1656) -> ("dx/dt"=w1658:dbl)  [unwired: 5 in, 3 out]
                      n647 = call "2ndOrderDerivate.vi"("t_capture"=w1657, "initial condition"=w1655, "x"=w1655) -> ("dx/dt"=w1660:dbl)  [unwired: 5 in, 3 out]
                      n648 = call "2ndOrderDerivate.vi"("t_capture"=w1657, "initial condition"=w1654, "x"=w1654) -> ("dx/dt"=w1659:dbl)  [unwired: 5 in, 3 out]
                    }
                    frame 7 {
                      n649 = call "2ndOrderDerivate.vi"("t_capture"=w1664, "initial condition"=w1663, "x"=w1663) -> ("dx/dt"=w1665:dbl)  [unwired: 5 in, 3 out]
                      n650 = call "2ndOrderDerivate.vi"("t_capture"=w1664, "initial condition"=w1662, "x"=w1662) -> ("dx/dt"=w1667:dbl)  [unwired: 5 in, 3 out]
                      n651 = call "2ndOrderDerivate.vi"("t_capture"=w1664, "initial condition"=w1661, "x"=w1661) -> ("dx/dt"=w1666:dbl)  [unwired: 5 in, 3 out]
                    }
                    frame 8 {
                      n652 = call "2ndOrderDerivate.vi"("t_capture"=w1671, "initial condition"=w1670, "x"=w1670) -> ("dx/dt"=w1672:dbl)  [unwired: 5 in, 3 out]
                      n653 = call "2ndOrderDerivate.vi"("t_capture"=w1671, "initial condition"=w1669, "x"=w1669) -> ("dx/dt"=w1674:dbl)  [unwired: 5 in, 3 out]
                      n654 = call "2ndOrderDerivate.vi"("t_capture"=w1671, "initial condition"=w1668, "x"=w1668) -> ("dx/dt"=w1673:dbl)  [unwired: 5 in, 3 out]
                    }
                    frame 9 {
                      n655 = call "2ndOrderDerivate.vi"("t_capture"=w1678, "initial condition"=w1677, "x"=w1677) -> ("dx/dt"=w1679:dbl)  [unwired: 5 in, 3 out]
                      n656 = call "2ndOrderDerivate.vi"("t_capture"=w1678, "initial condition"=w1676, "x"=w1676) -> ("dx/dt"=w1681:dbl)  [unwired: 5 in, 3 out]
                      n657 = call "2ndOrderDerivate.vi"("t_capture"=w1678, "initial condition"=w1675, "x"=w1675) -> ("dx/dt"=w1680:dbl)  [unwired: 5 in, 3 out]
                    }
                    frame 10 {
                      n658 = call "2ndOrderDerivate.vi"("t_capture"=w1685, "initial condition"=w1684, "x"=w1684) -> ("dx/dt"=w1686:dbl)  [unwired: 5 in, 3 out]
                      n659 = call "2ndOrderDerivate.vi"("t_capture"=w1685, "initial condition"=w1683, "x"=w1683) -> ("dx/dt"=w1688:dbl)  [unwired: 5 in, 3 out]
                      n660 = call "2ndOrderDerivate.vi"("t_capture"=w1685, "initial condition"=w1682, "x"=w1682) -> ("dx/dt"=w1687:dbl)  [unwired: 5 in, 3 out]
                    }
                    frame 11 {
                      n661 = call "2ndOrderDerivate.vi"("t_capture"=w1692, "initial condition"=w1691, "x"=w1691) -> ("dx/dt"=w1693:dbl)  [unwired: 5 in, 3 out]
                      n662 = call "2ndOrderDerivate.vi"("t_capture"=w1692, "initial condition"=w1690, "x"=w1690) -> ("dx/dt"=w1695:dbl)  [unwired: 5 in, 3 out]
                      n663 = call "2ndOrderDerivate.vi"("t_capture"=w1692, "initial condition"=w1689, "x"=w1689) -> ("dx/dt"=w1694:dbl)  [unwired: 5 in, 3 out]
                    }
                    frame 12 {
                      n664 = call "2ndOrderDerivate.vi"("t_capture"=w1699, "initial condition"=w1698, "x"=w1698) -> ("dx/dt"=w1700:dbl)  [unwired: 5 in, 3 out]
                      n665 = call "2ndOrderDerivate.vi"("t_capture"=w1699, "initial condition"=w1697, "x"=w1697) -> ("dx/dt"=w1702:dbl)  [unwired: 5 in, 3 out]
                      n666 = call "2ndOrderDerivate.vi"("t_capture"=w1699, "initial condition"=w1696, "x"=w1696) -> ("dx/dt"=w1701:dbl)  [unwired: 5 in, 3 out]
                    }
                    frame 13 {
                      n667 = call "2ndOrderDerivate.vi"("t_capture"=w1706, "initial condition"=w1705, "x"=w1705) -> ("dx/dt"=w1707:dbl)  [unwired: 5 in, 3 out]
                      n668 = call "2ndOrderDerivate.vi"("t_capture"=w1706, "initial condition"=w1704, "x"=w1704) -> ("dx/dt"=w1709:dbl)  [unwired: 5 in, 3 out]
                      n669 = call "2ndOrderDerivate.vi"("t_capture"=w1706, "initial condition"=w1703, "x"=w1703) -> ("dx/dt"=w1708:dbl)  [unwired: 5 in, 3 out]
                    }
                    frame 14 {
                      n670 = call "2ndOrderDerivate.vi"("t_capture"=w1713, "initial condition"=w1712, "x"=w1712) -> ("dx/dt"=w1714:dbl)  [unwired: 5 in, 3 out]
                      n671 = call "2ndOrderDerivate.vi"("t_capture"=w1713, "initial condition"=w1711, "x"=w1711) -> ("dx/dt"=w1716:dbl)  [unwired: 5 in, 3 out]
                      n672 = call "2ndOrderDerivate.vi"("t_capture"=w1713, "initial condition"=w1710, "x"=w1710) -> ("dx/dt"=w1715:dbl)  [unwired: 5 in, 3 out]
                    }
                    frame 15 {
                      n673 = call "2ndOrderDerivate.vi"("t_capture"=w1720, "initial condition"=w1719, "x"=w1719) -> ("dx/dt"=w1721:dbl)  [unwired: 5 in, 3 out]
                      n674 = call "2ndOrderDerivate.vi"("t_capture"=w1720, "initial condition"=w1718, "x"=w1718) -> ("dx/dt"=w1723:dbl)  [unwired: 5 in, 3 out]
                      n675 = call "2ndOrderDerivate.vi"("t_capture"=w1720, "initial condition"=w1717, "x"=w1717) -> ("dx/dt"=w1722:dbl)  [unwired: 5 in, 3 out]
                    }
                  }
                  n676 = case shown="0, Default" w1491 {
                    tunnel: w1490 -> [w1502 w1509 w1516 w1523 w1530 w1537 w1544 w1551 w1558 w1565 w1572 w1579 w1586 w1593 w1600 w1607]
                    tunnel: [w1504 w1511 w1518 w1525 w1532 w1539 w1546 w1553 w1560 w1567 w1574 w1581 w1588 w1595 w1602 w1609] -> w1487
                    tunnel: [w1506 w1513 w1520 w1527 w1534 w1541 w1548 w1555 w1562 w1569 w1576 w1583 w1590 w1597 w1604 w1611] -> w1486
                    tunnel: [w1505 w1512 w1519 w1526 w1533 w1540 w1547 w1554 w1561 w1568 w1575 w1582 w1589 w1596 w1603 w1610] -> w1485
                    tunnel: w1489 -> [w1501 w1508 w1515 w1522 w1529 w1536 w1543 w1550 w1557 w1564 w1571 w1578 w1585 w1592 w1599 w1606]
                    tunnel: w1488 -> [w1500 w1507 w1514 w1521 w1528 w1535 w1542 w1549 w1556 w1563 w1570 w1577 w1584 w1591 w1598 w1605]
                    tunnel: w1492 -> [w1503 w1510 w1517 w1524 w1531 w1538 w1545 w1552 w1559 w1566 w1573 w1580 w1587 w1594 w1601 w1608]
                    frame 0, Default {
                      n677 = call "2ndOrderDerivate.vi"("t_capture"=w1503, "initial condition"=w1502, "x"=w1502) -> ("dx/dt"=w1504:dbl)  [unwired: 5 in, 3 out]
                      n678 = call "2ndOrderDerivate.vi"("t_capture"=w1503, "initial condition"=w1501, "x"=w1501) -> ("dx/dt"=w1506:dbl)  [unwired: 5 in, 3 out]
                      n679 = call "2ndOrderDerivate.vi"("t_capture"=w1503, "initial condition"=w1500, "x"=w1500) -> ("dx/dt"=w1505:dbl)  [unwired: 5 in, 3 out]
                    }
                    frame 1 {
                      n680 = call "2ndOrderDerivate.vi"("t_capture"=w1510, "initial condition"=w1509, "x"=w1509) -> ("dx/dt"=w1511:dbl)  [unwired: 5 in, 3 out]
                      n681 = call "2ndOrderDerivate.vi"("t_capture"=w1510, "initial condition"=w1508, "x"=w1508) -> ("dx/dt"=w1513:dbl)  [unwired: 5 in, 3 out]
                      n682 = call "2ndOrderDerivate.vi"("t_capture"=w1510, "initial condition"=w1507, "x"=w1507) -> ("dx/dt"=w1512:dbl)  [unwired: 5 in, 3 out]
                    }
                    frame 2 {
                      n683 = call "2ndOrderDerivate.vi"("t_capture"=w1517, "initial condition"=w1516, "x"=w1516) -> ("dx/dt"=w1518:dbl)  [unwired: 5 in, 3 out]
                      n684 = call "2ndOrderDerivate.vi"("t_capture"=w1517, "initial condition"=w1515, "x"=w1515) -> ("dx/dt"=w1520:dbl)  [unwired: 5 in, 3 out]
                      n685 = call "2ndOrderDerivate.vi"("t_capture"=w1517, "initial condition"=w1514, "x"=w1514) -> ("dx/dt"=w1519:dbl)  [unwired: 5 in, 3 out]
                    }
                    frame 3 {
                      n686 = call "2ndOrderDerivate.vi"("t_capture"=w1524, "initial condition"=w1523, "x"=w1523) -> ("dx/dt"=w1525:dbl)  [unwired: 5 in, 3 out]
                      n687 = call "2ndOrderDerivate.vi"("t_capture"=w1524, "initial condition"=w1522, "x"=w1522) -> ("dx/dt"=w1527:dbl)  [unwired: 5 in, 3 out]
                      n688 = call "2ndOrderDerivate.vi"("t_capture"=w1524, "initial condition"=w1521, "x"=w1521) -> ("dx/dt"=w1526:dbl)  [unwired: 5 in, 3 out]
                    }
                    frame 4 {
                      n689 = call "2ndOrderDerivate.vi"("t_capture"=w1531, "initial condition"=w1530, "x"=w1530) -> ("dx/dt"=w1532:dbl)  [unwired: 5 in, 3 out]
                      n690 = call "2ndOrderDerivate.vi"("t_capture"=w1531, "initial condition"=w1529, "x"=w1529) -> ("dx/dt"=w1534:dbl)  [unwired: 5 in, 3 out]
                      n691 = call "2ndOrderDerivate.vi"("t_capture"=w1531, "initial condition"=w1528, "x"=w1528) -> ("dx/dt"=w1533:dbl)  [unwired: 5 in, 3 out]
                    }
                    frame 5 {
                      n692 = call "2ndOrderDerivate.vi"("t_capture"=w1538, "initial condition"=w1537, "x"=w1537) -> ("dx/dt"=w1539:dbl)  [unwired: 5 in, 3 out]
                      n693 = call "2ndOrderDerivate.vi"("t_capture"=w1538, "initial condition"=w1536, "x"=w1536) -> ("dx/dt"=w1541:dbl)  [unwired: 5 in, 3 out]
                      n694 = call "2ndOrderDerivate.vi"("t_capture"=w1538, "initial condition"=w1535, "x"=w1535) -> ("dx/dt"=w1540:dbl)  [unwired: 5 in, 3 out]
                    }
                    frame 6 {
                      n695 = call "2ndOrderDerivate.vi"("t_capture"=w1545, "initial condition"=w1544, "x"=w1544) -> ("dx/dt"=w1546:dbl)  [unwired: 5 in, 3 out]
                      n696 = call "2ndOrderDerivate.vi"("t_capture"=w1545, "initial condition"=w1543, "x"=w1543) -> ("dx/dt"=w1548:dbl)  [unwired: 5 in, 3 out]
                      n697 = call "2ndOrderDerivate.vi"("t_capture"=w1545, "initial condition"=w1542, "x"=w1542) -> ("dx/dt"=w1547:dbl)  [unwired: 5 in, 3 out]
                    }
                    frame 7 {
                      n698 = call "2ndOrderDerivate.vi"("t_capture"=w1552, "initial condition"=w1551, "x"=w1551) -> ("dx/dt"=w1553:dbl)  [unwired: 5 in, 3 out]
                      n699 = call "2ndOrderDerivate.vi"("t_capture"=w1552, "initial condition"=w1550, "x"=w1550) -> ("dx/dt"=w1555:dbl)  [unwired: 5 in, 3 out]
                      n700 = call "2ndOrderDerivate.vi"("t_capture"=w1552, "initial condition"=w1549, "x"=w1549) -> ("dx/dt"=w1554:dbl)  [unwired: 5 in, 3 out]
                    }
                    frame 8 {
                      n701 = call "2ndOrderDerivate.vi"("t_capture"=w1559, "initial condition"=w1558, "x"=w1558) -> ("dx/dt"=w1560:dbl)  [unwired: 5 in, 3 out]
                      n702 = call "2ndOrderDerivate.vi"("t_capture"=w1559, "initial condition"=w1557, "x"=w1557) -> ("dx/dt"=w1562:dbl)  [unwired: 5 in, 3 out]
                      n703 = call "2ndOrderDerivate.vi"("t_capture"=w1559, "initial condition"=w1556, "x"=w1556) -> ("dx/dt"=w1561:dbl)  [unwired: 5 in, 3 out]
                    }
                    frame 9 {
                      n704 = call "2ndOrderDerivate.vi"("t_capture"=w1566, "initial condition"=w1565, "x"=w1565) -> ("dx/dt"=w1567:dbl)  [unwired: 5 in, 3 out]
                      n705 = call "2ndOrderDerivate.vi"("t_capture"=w1566, "initial condition"=w1564, "x"=w1564) -> ("dx/dt"=w1569:dbl)  [unwired: 5 in, 3 out]
                      n706 = call "2ndOrderDerivate.vi"("t_capture"=w1566, "initial condition"=w1563, "x"=w1563) -> ("dx/dt"=w1568:dbl)  [unwired: 5 in, 3 out]
                    }
                    frame 10 {
                      n707 = call "2ndOrderDerivate.vi"("t_capture"=w1573, "initial condition"=w1572, "x"=w1572) -> ("dx/dt"=w1574:dbl)  [unwired: 5 in, 3 out]
                      n708 = call "2ndOrderDerivate.vi"("t_capture"=w1573, "initial condition"=w1571, "x"=w1571) -> ("dx/dt"=w1576:dbl)  [unwired: 5 in, 3 out]
                      n709 = call "2ndOrderDerivate.vi"("t_capture"=w1573, "initial condition"=w1570, "x"=w1570) -> ("dx/dt"=w1575:dbl)  [unwired: 5 in, 3 out]
                    }
                    frame 11 {
                      n710 = call "2ndOrderDerivate.vi"("t_capture"=w1580, "initial condition"=w1579, "x"=w1579) -> ("dx/dt"=w1581:dbl)  [unwired: 5 in, 3 out]
                      n711 = call "2ndOrderDerivate.vi"("t_capture"=w1580, "initial condition"=w1578, "x"=w1578) -> ("dx/dt"=w1583:dbl)  [unwired: 5 in, 3 out]
                      n712 = call "2ndOrderDerivate.vi"("t_capture"=w1580, "initial condition"=w1577, "x"=w1577) -> ("dx/dt"=w1582:dbl)  [unwired: 5 in, 3 out]
                    }
                    frame 12 {
                      n713 = call "2ndOrderDerivate.vi"("t_capture"=w1587, "initial condition"=w1586, "x"=w1586) -> ("dx/dt"=w1588:dbl)  [unwired: 5 in, 3 out]
                      n714 = call "2ndOrderDerivate.vi"("t_capture"=w1587, "initial condition"=w1585, "x"=w1585) -> ("dx/dt"=w1590:dbl)  [unwired: 5 in, 3 out]
                      n715 = call "2ndOrderDerivate.vi"("t_capture"=w1587, "initial condition"=w1584, "x"=w1584) -> ("dx/dt"=w1589:dbl)  [unwired: 5 in, 3 out]
                    }
                    frame 13 {
                      n716 = call "2ndOrderDerivate.vi"("t_capture"=w1594, "initial condition"=w1593, "x"=w1593) -> ("dx/dt"=w1595:dbl)  [unwired: 5 in, 3 out]
                      n717 = call "2ndOrderDerivate.vi"("t_capture"=w1594, "initial condition"=w1592, "x"=w1592) -> ("dx/dt"=w1597:dbl)  [unwired: 5 in, 3 out]
                      n718 = call "2ndOrderDerivate.vi"("t_capture"=w1594, "initial condition"=w1591, "x"=w1591) -> ("dx/dt"=w1596:dbl)  [unwired: 5 in, 3 out]
                    }
                    frame 14 {
                      n719 = call "2ndOrderDerivate.vi"("t_capture"=w1601, "initial condition"=w1600, "x"=w1600) -> ("dx/dt"=w1602:dbl)  [unwired: 5 in, 3 out]
                      n720 = call "2ndOrderDerivate.vi"("t_capture"=w1601, "initial condition"=w1599, "x"=w1599) -> ("dx/dt"=w1604:dbl)  [unwired: 5 in, 3 out]
                      n721 = call "2ndOrderDerivate.vi"("t_capture"=w1601, "initial condition"=w1598, "x"=w1598) -> ("dx/dt"=w1603:dbl)  [unwired: 5 in, 3 out]
                    }
                    frame 15 {
                      n722 = call "2ndOrderDerivate.vi"("t_capture"=w1608, "initial condition"=w1607, "x"=w1607) -> ("dx/dt"=w1609:dbl)  [unwired: 5 in, 3 out]
                      n723 = call "2ndOrderDerivate.vi"("t_capture"=w1608, "initial condition"=w1606, "x"=w1606) -> ("dx/dt"=w1611:dbl)  [unwired: 5 in, 3 out]
                      n724 = call "2ndOrderDerivate.vi"("t_capture"=w1608, "initial condition"=w1605, "x"=w1605) -> ("dx/dt"=w1610:dbl)  [unwired: 5 in, 3 out]
                    }
                  }
                  n725 = Build Array(w1494, w1490, w1497, w1489, w1496, w1488, w1487, w1486, w1485) -> (w1499:dbl[])
                  n726 = call-poly <vilib>:"Array To Matrix.vi"("Real 1D Array"=w1499) -> ("Real Matrix (Column Vector)"=w1498:T3)
                  n727 = Bundle By Name(cluster=w1493, "x_k|k"=w1498) -> (w1495:T2)
                }
              }
              frame True {
              }
            }
            n728 = Bundle By Name(cluster=w1203, "robots_blue"=w1208, "robots_yellow"=w1207, "balls"=w1199) -> (w1206:T1)
            n729 = Bundle By Name(cluster=w1203, "New"=FALSE) -> (w1204:T1)
          }
          frame 2 {
            n730 = Empty Array?(array=w1728) -> (empty?=w1729:bool)
            n731 = Empty Array?(array=w1736) -> (empty?=w1737:bool)
            n732 = Reciprocal(x=w1738) -> (1/x=w1727:dbl)
            n733 = Empty Array?(array=w1739) -> (empty?=w1740:bool)
            n734 = case shown="False" w1729 {
              tunnel: w1728 -> [w1743 w1760]
              tunnel: w1727 -> [w1744 _]
              tunnel: [w1742 w1760] -> w1726
              tunnel: w1725 -> [w1741 _]
              frame False {
                n735 = for {
                  tunnel: w1743 -> [w1748] mode=indexing
                  tunnel: w1744 -> [_]
                  tunnel: w1743 -> [w1759] mode=indexing
                  tunnel: [w1757] -> w1742 mode=indexing
                  tunnel: w1741 -> [w1747]
                  n736 = Unbundle By Name(w1748) -> ("x"=w1755:sgl, "y"=w1753:sgl, "z"=w1751:sgl)
                  n737 = call "2ndOrderDerivate.vi"("t_capture"=w1747, "initial condition"=w1755, "x"=w1755) -> ("dx/dt"=w1754:dbl)  [unwired: 5 in, 3 out]
                  n738 = call "2ndOrderDerivate.vi"("t_capture"=w1747, "initial condition"=w1753, "x"=w1753) -> ("dx/dt"=w1752:dbl)  [unwired: 5 in, 3 out]
                  n739 = call "2ndOrderDerivate.vi"("t_capture"=w1747, "initial condition"=w1751, "x"=w1751) -> ("dx/dt"=w1756:dbl)  [unwired: 5 in, 3 out]
                  n740 = call "2ndOrderDerivate.vi"("t_capture"=w1747, "initial condition"=w1754, "x"=w1754) -> ("dx/dt"=w1750:dbl)  [unwired: 5 in, 3 out]
                  n741 = call "2ndOrderDerivate.vi"("t_capture"=w1747, "initial condition"=w1752, "x"=w1752) -> ("dx/dt"=w1745:dbl)  [unwired: 5 in, 3 out]
                  n742 = call "2ndOrderDerivate.vi"("t_capture"=w1747, "initial condition"=w1756, "x"=w1756) -> ("dx/dt"=w1749:dbl)  [unwired: 5 in, 3 out]
                  n743 = Build Array(w1755, w1754, w1753, w1752, w1751, w1747, w1750, w1745, w1749) -> (w1746:dbl[])
                  n744 = call-poly <vilib>:"Array To Matrix.vi"("Real 1D Array"=w1746) -> ("Real Matrix (Column Vector)"=w1758:T3)
                  n745 = Bundle By Name(cluster=w1759, "x_k|k"=w1758) -> (w1757:T4)
                }
              }
              frame True {
              }
            }
            n746 = case shown="False" w1737 {
              tunnel: w1736 -> [w1763 w2007]
              tunnel: w1727 -> [w1764 _]
              tunnel: [w1762 w2007] -> w1734
              tunnel: w1725 -> [w1761 _]
              frame False {
                n747 = for {
                  tunnel: w1763 -> [w1782] mode=indexing
                  tunnel: w1764 -> [w1774]
                  tunnel: w1763 -> [w1781] mode=indexing
                  tunnel: [w1775] -> w1762 mode=indexing if=w1773
                  tunnel: w1761 -> [w1772]
                  n748 = Unbundle By Name(w1782) -> ("x"=w1779:sgl, "y"=w1778:sgl, "orientation"=w1780:sgl, "robot_id"=w1765:u32, "Valid"=w1773:bool)
                  n749 = case shown="1" w1765 {
                    tunnel: w1779 -> [w1901 w1908 w1915 w1922 w1929 w1936 w1943 w1950 w1957 w1964 w1971 w1978 w1985 w1992 w1999 w2006]
                    tunnel: w1778 -> [w1899 w1906 w1913 w1920 w1927 w1934 w1941 w1948 w1955 w1962 w1969 w1976 w1983 w1990 w1997 w2004]
                    tunnel: w1780 -> [w1898 w1905 w1912 w1919 w1926 w1933 w1940 w1947 w1954 w1961 w1968 w1975 w1982 w1989 w1996 w2003]
                    tunnel: [w1897 w1904 w1911 w1918 w1925 w1932 w1939 w1946 w1953 w1960 w1967 w1974 w1981 w1988 w1995 w2002] -> w1771
                    tunnel: [w1896 w1903 w1910 w1917 w1924 w1931 w1938 w1945 w1952 w1959 w1966 w1973 w1980 w1987 w1994 w2001] -> w1770
                    tunnel: [w1895 w1902 w1909 w1916 w1923 w1930 w1937 w1944 w1951 w1958 w1965 w1972 w1979 w1986 w1993 w2000] -> w1769
                    tunnel: w1774 -> [_ _ _ _ _ _ _ _ _ _ _ _ _ _ _ _]
                    tunnel: w1772 -> [w1900 w1907 w1914 w1921 w1928 w1935 w1942 w1949 w1956 w1963 w1970 w1977 w1984 w1991 w1998 w2005]
                    frame 0, Default {
                      n750 = call "2ndOrderDerivate.vi"("t_capture"=w1900, "initial condition"=w1901, "x"=w1901) -> ("dx/dt"=w1897:dbl)  [unwired: 5 in, 3 out]
                      n751 = call "2ndOrderDerivate.vi"("t_capture"=w1900, "initial condition"=w1899, "x"=w1899) -> ("dx/dt"=w1896:dbl)  [unwired: 5 in, 3 out]
                      n752 = call "2ndOrderDerivate.vi"("t_capture"=w1900, "initial condition"=w1898, "x"=w1898) -> ("dx/dt"=w1895:dbl)  [unwired: 5 in, 3 out]
                    }
                    frame 1 {
                      n753 = call "2ndOrderDerivate.vi"("t_capture"=w1907, "initial condition"=w1908, "x"=w1908) -> ("dx/dt"=w1904:dbl)  [unwired: 5 in, 3 out]
                      n754 = call "2ndOrderDerivate.vi"("t_capture"=w1907, "initial condition"=w1906, "x"=w1906) -> ("dx/dt"=w1903:dbl)  [unwired: 5 in, 3 out]
                      n755 = call "2ndOrderDerivate.vi"("t_capture"=w1907, "initial condition"=w1905, "x"=w1905) -> ("dx/dt"=w1902:dbl)  [unwired: 5 in, 3 out]
                    }
                    frame 2 {
                      n756 = call "2ndOrderDerivate.vi"("t_capture"=w1914, "initial condition"=w1915, "x"=w1915) -> ("dx/dt"=w1911:dbl)  [unwired: 5 in, 3 out]
                      n757 = call "2ndOrderDerivate.vi"("t_capture"=w1914, "initial condition"=w1913, "x"=w1913) -> ("dx/dt"=w1910:dbl)  [unwired: 5 in, 3 out]
                      n758 = call "2ndOrderDerivate.vi"("t_capture"=w1914, "initial condition"=w1912, "x"=w1912) -> ("dx/dt"=w1909:dbl)  [unwired: 5 in, 3 out]
                    }
                    frame 3 {
                      n759 = call "2ndOrderDerivate.vi"("t_capture"=w1921, "initial condition"=w1922, "x"=w1922) -> ("dx/dt"=w1918:dbl)  [unwired: 5 in, 3 out]
                      n760 = call "2ndOrderDerivate.vi"("t_capture"=w1921, "initial condition"=w1920, "x"=w1920) -> ("dx/dt"=w1917:dbl)  [unwired: 5 in, 3 out]
                      n761 = call "2ndOrderDerivate.vi"("t_capture"=w1921, "initial condition"=w1919, "x"=w1919) -> ("dx/dt"=w1916:dbl)  [unwired: 5 in, 3 out]
                    }
                    frame 4 {
                      n762 = call "2ndOrderDerivate.vi"("t_capture"=w1928, "initial condition"=w1929, "x"=w1929) -> ("dx/dt"=w1925:dbl)  [unwired: 5 in, 3 out]
                      n763 = call "2ndOrderDerivate.vi"("t_capture"=w1928, "initial condition"=w1927, "x"=w1927) -> ("dx/dt"=w1924:dbl)  [unwired: 5 in, 3 out]
                      n764 = call "2ndOrderDerivate.vi"("t_capture"=w1928, "initial condition"=w1926, "x"=w1926) -> ("dx/dt"=w1923:dbl)  [unwired: 5 in, 3 out]
                    }
                    frame 5 {
                      n765 = call "2ndOrderDerivate.vi"("t_capture"=w1935, "initial condition"=w1936, "x"=w1936) -> ("dx/dt"=w1932:dbl)  [unwired: 5 in, 3 out]
                      n766 = call "2ndOrderDerivate.vi"("t_capture"=w1935, "initial condition"=w1934, "x"=w1934) -> ("dx/dt"=w1931:dbl)  [unwired: 5 in, 3 out]
                      n767 = call "2ndOrderDerivate.vi"("t_capture"=w1935, "initial condition"=w1933, "x"=w1933) -> ("dx/dt"=w1930:dbl)  [unwired: 5 in, 3 out]
                    }
                    frame 6 {
                      n768 = call "2ndOrderDerivate.vi"("t_capture"=w1942, "initial condition"=w1943, "x"=w1943) -> ("dx/dt"=w1939:dbl)  [unwired: 5 in, 3 out]
                      n769 = call "2ndOrderDerivate.vi"("t_capture"=w1942, "initial condition"=w1941, "x"=w1941) -> ("dx/dt"=w1938:dbl)  [unwired: 5 in, 3 out]
                      n770 = call "2ndOrderDerivate.vi"("t_capture"=w1942, "initial condition"=w1940, "x"=w1940) -> ("dx/dt"=w1937:dbl)  [unwired: 5 in, 3 out]
                    }
                    frame 7 {
                      n771 = call "2ndOrderDerivate.vi"("t_capture"=w1949, "initial condition"=w1950, "x"=w1950) -> ("dx/dt"=w1946:dbl)  [unwired: 5 in, 3 out]
                      n772 = call "2ndOrderDerivate.vi"("t_capture"=w1949, "initial condition"=w1948, "x"=w1948) -> ("dx/dt"=w1945:dbl)  [unwired: 5 in, 3 out]
                      n773 = call "2ndOrderDerivate.vi"("t_capture"=w1949, "initial condition"=w1947, "x"=w1947) -> ("dx/dt"=w1944:dbl)  [unwired: 5 in, 3 out]
                    }
                    frame 8 {
                      n774 = call "2ndOrderDerivate.vi"("t_capture"=w1956, "initial condition"=w1957, "x"=w1957) -> ("dx/dt"=w1953:dbl)  [unwired: 5 in, 3 out]
                      n775 = call "2ndOrderDerivate.vi"("t_capture"=w1956, "initial condition"=w1955, "x"=w1955) -> ("dx/dt"=w1952:dbl)  [unwired: 5 in, 3 out]
                      n776 = call "2ndOrderDerivate.vi"("t_capture"=w1956, "initial condition"=w1954, "x"=w1954) -> ("dx/dt"=w1951:dbl)  [unwired: 5 in, 3 out]
                    }
                    frame 9 {
                      n777 = call "2ndOrderDerivate.vi"("t_capture"=w1963, "initial condition"=w1964, "x"=w1964) -> ("dx/dt"=w1960:dbl)  [unwired: 5 in, 3 out]
                      n778 = call "2ndOrderDerivate.vi"("t_capture"=w1963, "initial condition"=w1962, "x"=w1962) -> ("dx/dt"=w1959:dbl)  [unwired: 5 in, 3 out]
                      n779 = call "2ndOrderDerivate.vi"("t_capture"=w1963, "initial condition"=w1961, "x"=w1961) -> ("dx/dt"=w1958:dbl)  [unwired: 5 in, 3 out]
                    }
                    frame 10 {
                      n780 = call "2ndOrderDerivate.vi"("t_capture"=w1970, "initial condition"=w1971, "x"=w1971) -> ("dx/dt"=w1967:dbl)  [unwired: 5 in, 3 out]
                      n781 = call "2ndOrderDerivate.vi"("t_capture"=w1970, "initial condition"=w1969, "x"=w1969) -> ("dx/dt"=w1966:dbl)  [unwired: 5 in, 3 out]
                      n782 = call "2ndOrderDerivate.vi"("t_capture"=w1970, "initial condition"=w1968, "x"=w1968) -> ("dx/dt"=w1965:dbl)  [unwired: 5 in, 3 out]
                    }
                    frame 11 {
                      n783 = call "2ndOrderDerivate.vi"("t_capture"=w1977, "initial condition"=w1978, "x"=w1978) -> ("dx/dt"=w1974:dbl)  [unwired: 5 in, 3 out]
                      n784 = call "2ndOrderDerivate.vi"("t_capture"=w1977, "initial condition"=w1976, "x"=w1976) -> ("dx/dt"=w1973:dbl)  [unwired: 5 in, 3 out]
                      n785 = call "2ndOrderDerivate.vi"("t_capture"=w1977, "initial condition"=w1975, "x"=w1975) -> ("dx/dt"=w1972:dbl)  [unwired: 5 in, 3 out]
                    }
                    frame 12 {
                      n786 = call "2ndOrderDerivate.vi"("t_capture"=w1984, "initial condition"=w1985, "x"=w1985) -> ("dx/dt"=w1981:dbl)  [unwired: 5 in, 3 out]
                      n787 = call "2ndOrderDerivate.vi"("t_capture"=w1984, "initial condition"=w1983, "x"=w1983) -> ("dx/dt"=w1980:dbl)  [unwired: 5 in, 3 out]
                      n788 = call "2ndOrderDerivate.vi"("t_capture"=w1984, "initial condition"=w1982, "x"=w1982) -> ("dx/dt"=w1979:dbl)  [unwired: 5 in, 3 out]
                    }
                    frame 13 {
                      n789 = call "2ndOrderDerivate.vi"("t_capture"=w1991, "initial condition"=w1992, "x"=w1992) -> ("dx/dt"=w1988:dbl)  [unwired: 5 in, 3 out]
                      n790 = call "2ndOrderDerivate.vi"("t_capture"=w1991, "initial condition"=w1990, "x"=w1990) -> ("dx/dt"=w1987:dbl)  [unwired: 5 in, 3 out]
                      n791 = call "2ndOrderDerivate.vi"("t_capture"=w1991, "initial condition"=w1989, "x"=w1989) -> ("dx/dt"=w1986:dbl)  [unwired: 5 in, 3 out]
                    }
                    frame 14 {
                      n792 = call "2ndOrderDerivate.vi"("t_capture"=w1998, "initial condition"=w1999, "x"=w1999) -> ("dx/dt"=w1995:dbl)  [unwired: 5 in, 3 out]
                      n793 = call "2ndOrderDerivate.vi"("t_capture"=w1998, "initial condition"=w1997, "x"=w1997) -> ("dx/dt"=w1994:dbl)  [unwired: 5 in, 3 out]
                      n794 = call "2ndOrderDerivate.vi"("t_capture"=w1998, "initial condition"=w1996, "x"=w1996) -> ("dx/dt"=w1993:dbl)  [unwired: 5 in, 3 out]
                    }
                    frame 15 {
                      n795 = call "2ndOrderDerivate.vi"("t_capture"=w2005, "initial condition"=w2006, "x"=w2006) -> ("dx/dt"=w2002:dbl)  [unwired: 5 in, 3 out]
                      n796 = call "2ndOrderDerivate.vi"("t_capture"=w2005, "initial condition"=w2004, "x"=w2004) -> ("dx/dt"=w2001:dbl)  [unwired: 5 in, 3 out]
                      n797 = call "2ndOrderDerivate.vi"("t_capture"=w2005, "initial condition"=w2003, "x"=w2003) -> ("dx/dt"=w2000:dbl)  [unwired: 5 in, 3 out]
                    }
                  }
                  n798 = case shown="1" w1765 {
                    tunnel: w1771 -> [w1789 w1796 w1803 w1810 w1817 w1824 w1831 w1838 w1845 w1852 w1859 w1866 w1873 w1880 w1887 w1894]
                    tunnel: w1770 -> [w1787 w1794 w1801 w1808 w1815 w1822 w1829 w1836 w1843 w1850 w1857 w1864 w1871 w1878 w1885 w1892]
                    tunnel: w1769 -> [w1786 w1793 w1800 w1807 w1814 w1821 w1828 w1835 w1842 w1849 w1856 w1863 w1870 w1877 w1884 w1891]
                    tunnel: [w1785 w1792 w1799 w1806 w1813 w1820 w1827 w1834 w1841 w1848 w1855 w1862 w1869 w1876 w1883 w1890] -> w1768
                    tunnel: [w1784 w1791 w1798 w1805 w1812 w1819 w1826 w1833 w1840 w1847 w1854 w1861 w1868 w1875 w1882 w1889] -> w1767
                    tunnel: [w1783 w1790 w1797 w1804 w1811 w1818 w1825 w1832 w1839 w1846 w1853 w1860 w1867 w1874 w1881 w1888] -> w1766
                    tunnel: w1772 -> [w1788 w1795 w1802 w1809 w1816 w1823 w1830 w1837 w1844 w1851 w1858 w1865 w1872 w1879 w1886 w1893]
                    frame 0, Default {
                      n799 = call "2ndOrderDerivate.vi"("t_capture"=w1788, "initial condition"=w1789, "x"=w1789) -> ("dx/dt"=w1785:dbl)  [unwired: 5 in, 3 out]
                      n800 = call "2ndOrderDerivate.vi"("t_capture"=w1788, "initial condition"=w1787, "x"=w1787) -> ("dx/dt"=w1784:dbl)  [unwired: 5 in, 3 out]
                      n801 = call "2ndOrderDerivate.vi"("t_capture"=w1788, "initial condition"=w1786, "x"=w1786) -> ("dx/dt"=w1783:dbl)  [unwired: 5 in, 3 out]
                    }
                    frame 1 {
                      n802 = call "2ndOrderDerivate.vi"("t_capture"=w1795, "initial condition"=w1796, "x"=w1796) -> ("dx/dt"=w1792:dbl)  [unwired: 5 in, 3 out]
                      n803 = call "2ndOrderDerivate.vi"("t_capture"=w1795, "initial condition"=w1794, "x"=w1794) -> ("dx/dt"=w1791:dbl)  [unwired: 5 in, 3 out]
                      n804 = call "2ndOrderDerivate.vi"("t_capture"=w1795, "initial condition"=w1793, "x"=w1793) -> ("dx/dt"=w1790:dbl)  [unwired: 5 in, 3 out]
                    }
                    frame 2 {
                      n805 = call "2ndOrderDerivate.vi"("t_capture"=w1802, "initial condition"=w1803, "x"=w1803) -> ("dx/dt"=w1799:dbl)  [unwired: 5 in, 3 out]
                      n806 = call "2ndOrderDerivate.vi"("t_capture"=w1802, "initial condition"=w1801, "x"=w1801) -> ("dx/dt"=w1798:dbl)  [unwired: 5 in, 3 out]
                      n807 = call "2ndOrderDerivate.vi"("t_capture"=w1802, "initial condition"=w1800, "x"=w1800) -> ("dx/dt"=w1797:dbl)  [unwired: 5 in, 3 out]
                    }
                    frame 3 {
                      n808 = call "2ndOrderDerivate.vi"("t_capture"=w1809, "initial condition"=w1810, "x"=w1810) -> ("dx/dt"=w1806:dbl)  [unwired: 5 in, 3 out]
                      n809 = call "2ndOrderDerivate.vi"("t_capture"=w1809, "initial condition"=w1808, "x"=w1808) -> ("dx/dt"=w1805:dbl)  [unwired: 5 in, 3 out]
                      n810 = call "2ndOrderDerivate.vi"("t_capture"=w1809, "initial condition"=w1807, "x"=w1807) -> ("dx/dt"=w1804:dbl)  [unwired: 5 in, 3 out]
                    }
                    frame 4 {
                      n811 = call "2ndOrderDerivate.vi"("t_capture"=w1816, "initial condition"=w1817, "x"=w1817) -> ("dx/dt"=w1813:dbl)  [unwired: 5 in, 3 out]
                      n812 = call "2ndOrderDerivate.vi"("t_capture"=w1816, "initial condition"=w1815, "x"=w1815) -> ("dx/dt"=w1812:dbl)  [unwired: 5 in, 3 out]
                      n813 = call "2ndOrderDerivate.vi"("t_capture"=w1816, "initial condition"=w1814, "x"=w1814) -> ("dx/dt"=w1811:dbl)  [unwired: 5 in, 3 out]
                    }
                    frame 5 {
                      n814 = call "2ndOrderDerivate.vi"("t_capture"=w1823, "initial condition"=w1824, "x"=w1824) -> ("dx/dt"=w1820:dbl)  [unwired: 5 in, 3 out]
                      n815 = call "2ndOrderDerivate.vi"("t_capture"=w1823, "initial condition"=w1822, "x"=w1822) -> ("dx/dt"=w1819:dbl)  [unwired: 5 in, 3 out]
                      n816 = call "2ndOrderDerivate.vi"("t_capture"=w1823, "initial condition"=w1821, "x"=w1821) -> ("dx/dt"=w1818:dbl)  [unwired: 5 in, 3 out]
                    }
                    frame 6 {
                      n817 = call "2ndOrderDerivate.vi"("t_capture"=w1830, "initial condition"=w1831, "x"=w1831) -> ("dx/dt"=w1827:dbl)  [unwired: 5 in, 3 out]
                      n818 = call "2ndOrderDerivate.vi"("t_capture"=w1830, "initial condition"=w1829, "x"=w1829) -> ("dx/dt"=w1826:dbl)  [unwired: 5 in, 3 out]
                      n819 = call "2ndOrderDerivate.vi"("t_capture"=w1830, "initial condition"=w1828, "x"=w1828) -> ("dx/dt"=w1825:dbl)  [unwired: 5 in, 3 out]
                    }
                    frame 7 {
                      n820 = call "2ndOrderDerivate.vi"("t_capture"=w1837, "initial condition"=w1838, "x"=w1838) -> ("dx/dt"=w1834:dbl)  [unwired: 5 in, 3 out]
                      n821 = call "2ndOrderDerivate.vi"("t_capture"=w1837, "initial condition"=w1836, "x"=w1836) -> ("dx/dt"=w1833:dbl)  [unwired: 5 in, 3 out]
                      n822 = call "2ndOrderDerivate.vi"("t_capture"=w1837, "initial condition"=w1835, "x"=w1835) -> ("dx/dt"=w1832:dbl)  [unwired: 5 in, 3 out]
                    }
                    frame 8 {
                      n823 = call "2ndOrderDerivate.vi"("t_capture"=w1844, "initial condition"=w1845, "x"=w1845) -> ("dx/dt"=w1841:dbl)  [unwired: 5 in, 3 out]
                      n824 = call "2ndOrderDerivate.vi"("t_capture"=w1844, "initial condition"=w1843, "x"=w1843) -> ("dx/dt"=w1840:dbl)  [unwired: 5 in, 3 out]
                      n825 = call "2ndOrderDerivate.vi"("t_capture"=w1844, "initial condition"=w1842, "x"=w1842) -> ("dx/dt"=w1839:dbl)  [unwired: 5 in, 3 out]
                    }
                    frame 9 {
                      n826 = call "2ndOrderDerivate.vi"("t_capture"=w1851, "initial condition"=w1852, "x"=w1852) -> ("dx/dt"=w1848:dbl)  [unwired: 5 in, 3 out]
                      n827 = call "2ndOrderDerivate.vi"("t_capture"=w1851, "initial condition"=w1850, "x"=w1850) -> ("dx/dt"=w1847:dbl)  [unwired: 5 in, 3 out]
                      n828 = call "2ndOrderDerivate.vi"("t_capture"=w1851, "initial condition"=w1849, "x"=w1849) -> ("dx/dt"=w1846:dbl)  [unwired: 5 in, 3 out]
                    }
                    frame 10 {
                      n829 = call "2ndOrderDerivate.vi"("t_capture"=w1858, "initial condition"=w1859, "x"=w1859) -> ("dx/dt"=w1855:dbl)  [unwired: 5 in, 3 out]
                      n830 = call "2ndOrderDerivate.vi"("t_capture"=w1858, "initial condition"=w1857, "x"=w1857) -> ("dx/dt"=w1854:dbl)  [unwired: 5 in, 3 out]
                      n831 = call "2ndOrderDerivate.vi"("t_capture"=w1858, "initial condition"=w1856, "x"=w1856) -> ("dx/dt"=w1853:dbl)  [unwired: 5 in, 3 out]
                    }
                    frame 11 {
                      n832 = call "2ndOrderDerivate.vi"("t_capture"=w1865, "initial condition"=w1866, "x"=w1866) -> ("dx/dt"=w1862:dbl)  [unwired: 5 in, 3 out]
                      n833 = call "2ndOrderDerivate.vi"("t_capture"=w1865, "initial condition"=w1864, "x"=w1864) -> ("dx/dt"=w1861:dbl)  [unwired: 5 in, 3 out]
                      n834 = call "2ndOrderDerivate.vi"("t_capture"=w1865, "initial condition"=w1863, "x"=w1863) -> ("dx/dt"=w1860:dbl)  [unwired: 5 in, 3 out]
                    }
                    frame 12 {
                      n835 = call "2ndOrderDerivate.vi"("t_capture"=w1872, "initial condition"=w1873, "x"=w1873) -> ("dx/dt"=w1869:dbl)  [unwired: 5 in, 3 out]
                      n836 = call "2ndOrderDerivate.vi"("t_capture"=w1872, "initial condition"=w1871, "x"=w1871) -> ("dx/dt"=w1868:dbl)  [unwired: 5 in, 3 out]
                      n837 = call "2ndOrderDerivate.vi"("t_capture"=w1872, "initial condition"=w1870, "x"=w1870) -> ("dx/dt"=w1867:dbl)  [unwired: 5 in, 3 out]
                    }
                    frame 13 {
                      n838 = call "2ndOrderDerivate.vi"("t_capture"=w1879, "initial condition"=w1880, "x"=w1880) -> ("dx/dt"=w1876:dbl)  [unwired: 5 in, 3 out]
                      n839 = call "2ndOrderDerivate.vi"("t_capture"=w1879, "initial condition"=w1878, "x"=w1878) -> ("dx/dt"=w1875:dbl)  [unwired: 5 in, 3 out]
                      n840 = call "2ndOrderDerivate.vi"("t_capture"=w1879, "initial condition"=w1877, "x"=w1877) -> ("dx/dt"=w1874:dbl)  [unwired: 5 in, 3 out]
                    }
                    frame 14 {
                      n841 = call "2ndOrderDerivate.vi"("t_capture"=w1886, "initial condition"=w1887, "x"=w1887) -> ("dx/dt"=w1883:dbl)  [unwired: 5 in, 3 out]
                      n842 = call "2ndOrderDerivate.vi"("t_capture"=w1886, "initial condition"=w1885, "x"=w1885) -> ("dx/dt"=w1882:dbl)  [unwired: 5 in, 3 out]
                      n843 = call "2ndOrderDerivate.vi"("t_capture"=w1886, "initial condition"=w1884, "x"=w1884) -> ("dx/dt"=w1881:dbl)  [unwired: 5 in, 3 out]
                    }
                    frame 15 {
                      n844 = call "2ndOrderDerivate.vi"("t_capture"=w1893, "initial condition"=w1894, "x"=w1894) -> ("dx/dt"=w1890:dbl)  [unwired: 5 in, 3 out]
                      n845 = call "2ndOrderDerivate.vi"("t_capture"=w1893, "initial condition"=w1892, "x"=w1892) -> ("dx/dt"=w1889:dbl)  [unwired: 5 in, 3 out]
                      n846 = call "2ndOrderDerivate.vi"("t_capture"=w1893, "initial condition"=w1891, "x"=w1891) -> ("dx/dt"=w1888:dbl)  [unwired: 5 in, 3 out]
                    }
                  }
                  n847 = Build Array(w1779, w1771, w1778, w1770, w1780, w1769, w1768, w1767, w1766) -> (w1777:dbl[])
                  n848 = call-poly <vilib>:"Array To Matrix.vi"("Real 1D Array"=w1777) -> ("Real Matrix (Column Vector)"=w1776:T3)
                  n849 = Bundle By Name(cluster=w1781, "x_k|k"=w1776) -> (w1775:T2)
                }
              }
              frame True {
              }
            }
            n850 = case shown="False" w1740 {
              tunnel: w1739 -> [w2010 w2251]
              tunnel: w1727 -> [w2011 _]
              tunnel: [w2009 w2251] -> w1735
              tunnel: w1725 -> [w2008 _]
              frame False {
                n851 = for {
                  tunnel: w2010 -> [w2020] mode=indexing
                  tunnel: w2011 -> [_]
                  tunnel: [w2022] -> w2009 mode=indexing
                  tunnel: w2008 -> [w2019]
                  n852 = Unbundle By Name(w2020) -> ("x"=w2021:sgl, "y"=w2024:sgl, "orientation"=w2023:sgl, "robot_id"=w2018:u32)  [unwired: 1 out]
                  n853 = case shown="0, Default" w2018 {
                    tunnel: w2021 -> [w2141 w2148 w2155 w2162 w2169 w2176 w2183 w2190 w2197 w2204 w2211 w2218 w2225 w2232 w2239 w2246]
                    tunnel: [w2143 w2150 w2157 w2164 w2171 w2178 w2185 w2192 w2199 w2206 w2213 w2220 w2227 w2234 w2241 w2248] -> w2017
                    tunnel: [w2145 w2152 w2159 w2166 w2173 w2180 w2187 w2194 w2201 w2208 w2215 w2222 w2229 w2236 w2243 w2250] -> w2016
                    tunnel: [w2144 w2151 w2158 w2165 w2172 w2179 w2186 w2193 w2200 w2207 w2214 w2221 w2228 w2235 w2242 w2249] -> w2015
                    tunnel: w2024 -> [w2140 w2147 w2154 w2161 w2168 w2175 w2182 w2189 w2196 w2203 w2210 w2217 w2224 w2231 w2238 w2245]
                    tunnel: w2023 -> [w2139 w2146 w2153 w2160 w2167 w2174 w2181 w2188 w2195 w2202 w2209 w2216 w2223 w2230 w2237 w2244]
                    tunnel: w2019 -> [w2142 w2149 w2156 w2163 w2170 w2177 w2184 w2191 w2198 w2205 w2212 w2219 w2226 w2233 w2240 w2247]
                    frame 0, Default {
                      n854 = call "2ndOrderDerivate.vi"("t_capture"=w2142, "initial condition"=w2141, "x"=w2141) -> ("dx/dt"=w2143:dbl)  [unwired: 5 in, 3 out]
                      n855 = call "2ndOrderDerivate.vi"("t_capture"=w2142, "initial condition"=w2140, "x"=w2140) -> ("dx/dt"=w2145:dbl)  [unwired: 5 in, 3 out]
                      n856 = call "2ndOrderDerivate.vi"("t_capture"=w2142, "initial condition"=w2139, "x"=w2139) -> ("dx/dt"=w2144:dbl)  [unwired: 5 in, 3 out]
                    }
                    frame 1 {
                      n857 = call "2ndOrderDerivate.vi"("t_capture"=w2149, "initial condition"=w2148, "x"=w2148) -> ("dx/dt"=w2150:dbl)  [unwired: 5 in, 3 out]
                      n858 = call "2ndOrderDerivate.vi"("t_capture"=w2149, "initial condition"=w2147, "x"=w2147) -> ("dx/dt"=w2152:dbl)  [unwired: 5 in, 3 out]
                      n859 = call "2ndOrderDerivate.vi"("t_capture"=w2149, "initial condition"=w2146, "x"=w2146) -> ("dx/dt"=w2151:dbl)  [unwired: 5 in, 3 out]
                    }
                    frame 2 {
                      n860 = call "2ndOrderDerivate.vi"("t_capture"=w2156, "initial condition"=w2155, "x"=w2155) -> ("dx/dt"=w2157:dbl)  [unwired: 5 in, 3 out]
                      n861 = call "2ndOrderDerivate.vi"("t_capture"=w2156, "initial condition"=w2154, "x"=w2154) -> ("dx/dt"=w2159:dbl)  [unwired: 5 in, 3 out]
                      n862 = call "2ndOrderDerivate.vi"("t_capture"=w2156, "initial condition"=w2153, "x"=w2153) -> ("dx/dt"=w2158:dbl)  [unwired: 5 in, 3 out]
                    }
                    frame 3 {
                      n863 = call "2ndOrderDerivate.vi"("t_capture"=w2163, "initial condition"=w2162, "x"=w2162) -> ("dx/dt"=w2164:dbl)  [unwired: 5 in, 3 out]
                      n864 = call "2ndOrderDerivate.vi"("t_capture"=w2163, "initial condition"=w2161, "x"=w2161) -> ("dx/dt"=w2166:dbl)  [unwired: 5 in, 3 out]
                      n865 = call "2ndOrderDerivate.vi"("t_capture"=w2163, "initial condition"=w2160, "x"=w2160) -> ("dx/dt"=w2165:dbl)  [unwired: 5 in, 3 out]
                    }
                    frame 4 {
                      n866 = call "2ndOrderDerivate.vi"("t_capture"=w2170, "initial condition"=w2169, "x"=w2169) -> ("dx/dt"=w2171:dbl)  [unwired: 5 in, 3 out]
                      n867 = call "2ndOrderDerivate.vi"("t_capture"=w2170, "initial condition"=w2168, "x"=w2168) -> ("dx/dt"=w2173:dbl)  [unwired: 5 in, 3 out]
                      n868 = call "2ndOrderDerivate.vi"("t_capture"=w2170, "initial condition"=w2167, "x"=w2167) -> ("dx/dt"=w2172:dbl)  [unwired: 5 in, 3 out]
                    }
                    frame 5 {
                      n869 = call "2ndOrderDerivate.vi"("t_capture"=w2177, "initial condition"=w2176, "x"=w2176) -> ("dx/dt"=w2178:dbl)  [unwired: 5 in, 3 out]
                      n870 = call "2ndOrderDerivate.vi"("t_capture"=w2177, "initial condition"=w2175, "x"=w2175) -> ("dx/dt"=w2180:dbl)  [unwired: 5 in, 3 out]
                      n871 = call "2ndOrderDerivate.vi"("t_capture"=w2177, "initial condition"=w2174, "x"=w2174) -> ("dx/dt"=w2179:dbl)  [unwired: 5 in, 3 out]
                    }
                    frame 6 {
                      n872 = call "2ndOrderDerivate.vi"("t_capture"=w2184, "initial condition"=w2183, "x"=w2183) -> ("dx/dt"=w2185:dbl)  [unwired: 5 in, 3 out]
                      n873 = call "2ndOrderDerivate.vi"("t_capture"=w2184, "initial condition"=w2182, "x"=w2182) -> ("dx/dt"=w2187:dbl)  [unwired: 5 in, 3 out]
                      n874 = call "2ndOrderDerivate.vi"("t_capture"=w2184, "initial condition"=w2181, "x"=w2181) -> ("dx/dt"=w2186:dbl)  [unwired: 5 in, 3 out]
                    }
                    frame 7 {
                      n875 = call "2ndOrderDerivate.vi"("t_capture"=w2191, "initial condition"=w2190, "x"=w2190) -> ("dx/dt"=w2192:dbl)  [unwired: 5 in, 3 out]
                      n876 = call "2ndOrderDerivate.vi"("t_capture"=w2191, "initial condition"=w2189, "x"=w2189) -> ("dx/dt"=w2194:dbl)  [unwired: 5 in, 3 out]
                      n877 = call "2ndOrderDerivate.vi"("t_capture"=w2191, "initial condition"=w2188, "x"=w2188) -> ("dx/dt"=w2193:dbl)  [unwired: 5 in, 3 out]
                    }
                    frame 8 {
                      n878 = call "2ndOrderDerivate.vi"("t_capture"=w2198, "initial condition"=w2197, "x"=w2197) -> ("dx/dt"=w2199:dbl)  [unwired: 5 in, 3 out]
                      n879 = call "2ndOrderDerivate.vi"("t_capture"=w2198, "initial condition"=w2196, "x"=w2196) -> ("dx/dt"=w2201:dbl)  [unwired: 5 in, 3 out]
                      n880 = call "2ndOrderDerivate.vi"("t_capture"=w2198, "initial condition"=w2195, "x"=w2195) -> ("dx/dt"=w2200:dbl)  [unwired: 5 in, 3 out]
                    }
                    frame 9 {
                      n881 = call "2ndOrderDerivate.vi"("t_capture"=w2205, "initial condition"=w2204, "x"=w2204) -> ("dx/dt"=w2206:dbl)  [unwired: 5 in, 3 out]
                      n882 = call "2ndOrderDerivate.vi"("t_capture"=w2205, "initial condition"=w2203, "x"=w2203) -> ("dx/dt"=w2208:dbl)  [unwired: 5 in, 3 out]
                      n883 = call "2ndOrderDerivate.vi"("t_capture"=w2205, "initial condition"=w2202, "x"=w2202) -> ("dx/dt"=w2207:dbl)  [unwired: 5 in, 3 out]
                    }
                    frame 10 {
                      n884 = call "2ndOrderDerivate.vi"("t_capture"=w2212, "initial condition"=w2211, "x"=w2211) -> ("dx/dt"=w2213:dbl)  [unwired: 5 in, 3 out]
                      n885 = call "2ndOrderDerivate.vi"("t_capture"=w2212, "initial condition"=w2210, "x"=w2210) -> ("dx/dt"=w2215:dbl)  [unwired: 5 in, 3 out]
                      n886 = call "2ndOrderDerivate.vi"("t_capture"=w2212, "initial condition"=w2209, "x"=w2209) -> ("dx/dt"=w2214:dbl)  [unwired: 5 in, 3 out]
                    }
                    frame 11 {
                      n887 = call "2ndOrderDerivate.vi"("t_capture"=w2219, "initial condition"=w2218, "x"=w2218) -> ("dx/dt"=w2220:dbl)  [unwired: 5 in, 3 out]
                      n888 = call "2ndOrderDerivate.vi"("t_capture"=w2219, "initial condition"=w2217, "x"=w2217) -> ("dx/dt"=w2222:dbl)  [unwired: 5 in, 3 out]
                      n889 = call "2ndOrderDerivate.vi"("t_capture"=w2219, "initial condition"=w2216, "x"=w2216) -> ("dx/dt"=w2221:dbl)  [unwired: 5 in, 3 out]
                    }
                    frame 12 {
                      n890 = call "2ndOrderDerivate.vi"("t_capture"=w2226, "initial condition"=w2225, "x"=w2225) -> ("dx/dt"=w2227:dbl)  [unwired: 5 in, 3 out]
                      n891 = call "2ndOrderDerivate.vi"("t_capture"=w2226, "initial condition"=w2224, "x"=w2224) -> ("dx/dt"=w2229:dbl)  [unwired: 5 in, 3 out]
                      n892 = call "2ndOrderDerivate.vi"("t_capture"=w2226, "initial condition"=w2223, "x"=w2223) -> ("dx/dt"=w2228:dbl)  [unwired: 5 in, 3 out]
                    }
                    frame 13 {
                      n893 = call "2ndOrderDerivate.vi"("t_capture"=w2233, "initial condition"=w2232, "x"=w2232) -> ("dx/dt"=w2234:dbl)  [unwired: 5 in, 3 out]
                      n894 = call "2ndOrderDerivate.vi"("t_capture"=w2233, "initial condition"=w2231, "x"=w2231) -> ("dx/dt"=w2236:dbl)  [unwired: 5 in, 3 out]
                      n895 = call "2ndOrderDerivate.vi"("t_capture"=w2233, "initial condition"=w2230, "x"=w2230) -> ("dx/dt"=w2235:dbl)  [unwired: 5 in, 3 out]
                    }
                    frame 14 {
                      n896 = call "2ndOrderDerivate.vi"("t_capture"=w2240, "initial condition"=w2239, "x"=w2239) -> ("dx/dt"=w2241:dbl)  [unwired: 5 in, 3 out]
                      n897 = call "2ndOrderDerivate.vi"("t_capture"=w2240, "initial condition"=w2238, "x"=w2238) -> ("dx/dt"=w2243:dbl)  [unwired: 5 in, 3 out]
                      n898 = call "2ndOrderDerivate.vi"("t_capture"=w2240, "initial condition"=w2237, "x"=w2237) -> ("dx/dt"=w2242:dbl)  [unwired: 5 in, 3 out]
                    }
                    frame 15 {
                      n899 = call "2ndOrderDerivate.vi"("t_capture"=w2247, "initial condition"=w2246, "x"=w2246) -> ("dx/dt"=w2248:dbl)  [unwired: 5 in, 3 out]
                      n900 = call "2ndOrderDerivate.vi"("t_capture"=w2247, "initial condition"=w2245, "x"=w2245) -> ("dx/dt"=w2250:dbl)  [unwired: 5 in, 3 out]
                      n901 = call "2ndOrderDerivate.vi"("t_capture"=w2247, "initial condition"=w2244, "x"=w2244) -> ("dx/dt"=w2249:dbl)  [unwired: 5 in, 3 out]
                    }
                  }
                  n902 = case shown="0, Default" w2018 {
                    tunnel: w2017 -> [w2029 w2036 w2043 w2050 w2057 w2064 w2071 w2078 w2085 w2092 w2099 w2106 w2113 w2120 w2127 w2134]
                    tunnel: [w2031 w2038 w2045 w2052 w2059 w2066 w2073 w2080 w2087 w2094 w2101 w2108 w2115 w2122 w2129 w2136] -> w2014
                    tunnel: [w2033 w2040 w2047 w2054 w2061 w2068 w2075 w2082 w2089 w2096 w2103 w2110 w2117 w2124 w2131 w2138] -> w2013
                    tunnel: [w2032 w2039 w2046 w2053 w2060 w2067 w2074 w2081 w2088 w2095 w2102 w2109 w2116 w2123 w2130 w2137] -> w2012
                    tunnel: w2016 -> [w2028 w2035 w2042 w2049 w2056 w2063 w2070 w2077 w2084 w2091 w2098 w2105 w2112 w2119 w2126 w2133]
                    tunnel: w2015 -> [w2027 w2034 w2041 w2048 w2055 w2062 w2069 w2076 w2083 w2090 w2097 w2104 w2111 w2118 w2125 w2132]
                    tunnel: w2019 -> [w2030 w2037 w2044 w2051 w2058 w2065 w2072 w2079 w2086 w2093 w2100 w2107 w2114 w2121 w2128 w2135]
                    frame 0, Default {
                      n903 = call "2ndOrderDerivate.vi"("t_capture"=w2030, "initial condition"=w2029, "x"=w2029) -> ("dx/dt"=w2031:dbl)  [unwired: 5 in, 3 out]
                      n904 = call "2ndOrderDerivate.vi"("t_capture"=w2030, "initial condition"=w2028, "x"=w2028) -> ("dx/dt"=w2033:dbl)  [unwired: 5 in, 3 out]
                      n905 = call "2ndOrderDerivate.vi"("t_capture"=w2030, "initial condition"=w2027, "x"=w2027) -> ("dx/dt"=w2032:dbl)  [unwired: 5 in, 3 out]
                    }
                    frame 1 {
                      n906 = call "2ndOrderDerivate.vi"("t_capture"=w2037, "initial condition"=w2036, "x"=w2036) -> ("dx/dt"=w2038:dbl)  [unwired: 5 in, 3 out]
                      n907 = call "2ndOrderDerivate.vi"("t_capture"=w2037, "initial condition"=w2035, "x"=w2035) -> ("dx/dt"=w2040:dbl)  [unwired: 5 in, 3 out]
                      n908 = call "2ndOrderDerivate.vi"("t_capture"=w2037, "initial condition"=w2034, "x"=w2034) -> ("dx/dt"=w2039:dbl)  [unwired: 5 in, 3 out]
                    }
                    frame 2 {
                      n909 = call "2ndOrderDerivate.vi"("t_capture"=w2044, "initial condition"=w2043, "x"=w2043) -> ("dx/dt"=w2045:dbl)  [unwired: 5 in, 3 out]
                      n910 = call "2ndOrderDerivate.vi"("t_capture"=w2044, "initial condition"=w2042, "x"=w2042) -> ("dx/dt"=w2047:dbl)  [unwired: 5 in, 3 out]
                      n911 = call "2ndOrderDerivate.vi"("t_capture"=w2044, "initial condition"=w2041, "x"=w2041) -> ("dx/dt"=w2046:dbl)  [unwired: 5 in, 3 out]
                    }
                    frame 3 {
                      n912 = call "2ndOrderDerivate.vi"("t_capture"=w2051, "initial condition"=w2050, "x"=w2050) -> ("dx/dt"=w2052:dbl)  [unwired: 5 in, 3 out]
                      n913 = call "2ndOrderDerivate.vi"("t_capture"=w2051, "initial condition"=w2049, "x"=w2049) -> ("dx/dt"=w2054:dbl)  [unwired: 5 in, 3 out]
                      n914 = call "2ndOrderDerivate.vi"("t_capture"=w2051, "initial condition"=w2048, "x"=w2048) -> ("dx/dt"=w2053:dbl)  [unwired: 5 in, 3 out]
                    }
                    frame 4 {
                      n915 = call "2ndOrderDerivate.vi"("t_capture"=w2058, "initial condition"=w2057, "x"=w2057) -> ("dx/dt"=w2059:dbl)  [unwired: 5 in, 3 out]
                      n916 = call "2ndOrderDerivate.vi"("t_capture"=w2058, "initial condition"=w2056, "x"=w2056) -> ("dx/dt"=w2061:dbl)  [unwired: 5 in, 3 out]
                      n917 = call "2ndOrderDerivate.vi"("t_capture"=w2058, "initial condition"=w2055, "x"=w2055) -> ("dx/dt"=w2060:dbl)  [unwired: 5 in, 3 out]
                    }
                    frame 5 {
                      n918 = call "2ndOrderDerivate.vi"("t_capture"=w2065, "initial condition"=w2064, "x"=w2064) -> ("dx/dt"=w2066:dbl)  [unwired: 5 in, 3 out]
                      n919 = call "2ndOrderDerivate.vi"("t_capture"=w2065, "initial condition"=w2063, "x"=w2063) -> ("dx/dt"=w2068:dbl)  [unwired: 5 in, 3 out]
                      n920 = call "2ndOrderDerivate.vi"("t_capture"=w2065, "initial condition"=w2062, "x"=w2062) -> ("dx/dt"=w2067:dbl)  [unwired: 5 in, 3 out]
                    }
                    frame 6 {
                      n921 = call "2ndOrderDerivate.vi"("t_capture"=w2072, "initial condition"=w2071, "x"=w2071) -> ("dx/dt"=w2073:dbl)  [unwired: 5 in, 3 out]
                      n922 = call "2ndOrderDerivate.vi"("t_capture"=w2072, "initial condition"=w2070, "x"=w2070) -> ("dx/dt"=w2075:dbl)  [unwired: 5 in, 3 out]
                      n923 = call "2ndOrderDerivate.vi"("t_capture"=w2072, "initial condition"=w2069, "x"=w2069) -> ("dx/dt"=w2074:dbl)  [unwired: 5 in, 3 out]
                    }
                    frame 7 {
                      n924 = call "2ndOrderDerivate.vi"("t_capture"=w2079, "initial condition"=w2078, "x"=w2078) -> ("dx/dt"=w2080:dbl)  [unwired: 5 in, 3 out]
                      n925 = call "2ndOrderDerivate.vi"("t_capture"=w2079, "initial condition"=w2077, "x"=w2077) -> ("dx/dt"=w2082:dbl)  [unwired: 5 in, 3 out]
                      n926 = call "2ndOrderDerivate.vi"("t_capture"=w2079, "initial condition"=w2076, "x"=w2076) -> ("dx/dt"=w2081:dbl)  [unwired: 5 in, 3 out]
                    }
                    frame 8 {
                      n927 = call "2ndOrderDerivate.vi"("t_capture"=w2086, "initial condition"=w2085, "x"=w2085) -> ("dx/dt"=w2087:dbl)  [unwired: 5 in, 3 out]
                      n928 = call "2ndOrderDerivate.vi"("t_capture"=w2086, "initial condition"=w2084, "x"=w2084) -> ("dx/dt"=w2089:dbl)  [unwired: 5 in, 3 out]
                      n929 = call "2ndOrderDerivate.vi"("t_capture"=w2086, "initial condition"=w2083, "x"=w2083) -> ("dx/dt"=w2088:dbl)  [unwired: 5 in, 3 out]
                    }
                    frame 9 {
                      n930 = call "2ndOrderDerivate.vi"("t_capture"=w2093, "initial condition"=w2092, "x"=w2092) -> ("dx/dt"=w2094:dbl)  [unwired: 5 in, 3 out]
                      n931 = call "2ndOrderDerivate.vi"("t_capture"=w2093, "initial condition"=w2091, "x"=w2091) -> ("dx/dt"=w2096:dbl)  [unwired: 5 in, 3 out]
                      n932 = call "2ndOrderDerivate.vi"("t_capture"=w2093, "initial condition"=w2090, "x"=w2090) -> ("dx/dt"=w2095:dbl)  [unwired: 5 in, 3 out]
                    }
                    frame 10 {
                      n933 = call "2ndOrderDerivate.vi"("t_capture"=w2100, "initial condition"=w2099, "x"=w2099) -> ("dx/dt"=w2101:dbl)  [unwired: 5 in, 3 out]
                      n934 = call "2ndOrderDerivate.vi"("t_capture"=w2100, "initial condition"=w2098, "x"=w2098) -> ("dx/dt"=w2103:dbl)  [unwired: 5 in, 3 out]
                      n935 = call "2ndOrderDerivate.vi"("t_capture"=w2100, "initial condition"=w2097, "x"=w2097) -> ("dx/dt"=w2102:dbl)  [unwired: 5 in, 3 out]
                    }
                    frame 11 {
                      n936 = call "2ndOrderDerivate.vi"("t_capture"=w2107, "initial condition"=w2106, "x"=w2106) -> ("dx/dt"=w2108:dbl)  [unwired: 5 in, 3 out]
                      n937 = call "2ndOrderDerivate.vi"("t_capture"=w2107, "initial condition"=w2105, "x"=w2105) -> ("dx/dt"=w2110:dbl)  [unwired: 5 in, 3 out]
                      n938 = call "2ndOrderDerivate.vi"("t_capture"=w2107, "initial condition"=w2104, "x"=w2104) -> ("dx/dt"=w2109:dbl)  [unwired: 5 in, 3 out]
                    }
                    frame 12 {
                      n939 = call "2ndOrderDerivate.vi"("t_capture"=w2114, "initial condition"=w2113, "x"=w2113) -> ("dx/dt"=w2115:dbl)  [unwired: 5 in, 3 out]
                      n940 = call "2ndOrderDerivate.vi"("t_capture"=w2114, "initial condition"=w2112, "x"=w2112) -> ("dx/dt"=w2117:dbl)  [unwired: 5 in, 3 out]
                      n941 = call "2ndOrderDerivate.vi"("t_capture"=w2114, "initial condition"=w2111, "x"=w2111) -> ("dx/dt"=w2116:dbl)  [unwired: 5 in, 3 out]
                    }
                    frame 13 {
                      n942 = call "2ndOrderDerivate.vi"("t_capture"=w2121, "initial condition"=w2120, "x"=w2120) -> ("dx/dt"=w2122:dbl)  [unwired: 5 in, 3 out]
                      n943 = call "2ndOrderDerivate.vi"("t_capture"=w2121, "initial condition"=w2119, "x"=w2119) -> ("dx/dt"=w2124:dbl)  [unwired: 5 in, 3 out]
                      n944 = call "2ndOrderDerivate.vi"("t_capture"=w2121, "initial condition"=w2118, "x"=w2118) -> ("dx/dt"=w2123:dbl)  [unwired: 5 in, 3 out]
                    }
                    frame 14 {
                      n945 = call "2ndOrderDerivate.vi"("t_capture"=w2128, "initial condition"=w2127, "x"=w2127) -> ("dx/dt"=w2129:dbl)  [unwired: 5 in, 3 out]
                      n946 = call "2ndOrderDerivate.vi"("t_capture"=w2128, "initial condition"=w2126, "x"=w2126) -> ("dx/dt"=w2131:dbl)  [unwired: 5 in, 3 out]
                      n947 = call "2ndOrderDerivate.vi"("t_capture"=w2128, "initial condition"=w2125, "x"=w2125) -> ("dx/dt"=w2130:dbl)  [unwired: 5 in, 3 out]
                    }
                    frame 15 {
                      n948 = call "2ndOrderDerivate.vi"("t_capture"=w2135, "initial condition"=w2134, "x"=w2134) -> ("dx/dt"=w2136:dbl)  [unwired: 5 in, 3 out]
                      n949 = call "2ndOrderDerivate.vi"("t_capture"=w2135, "initial condition"=w2133, "x"=w2133) -> ("dx/dt"=w2138:dbl)  [unwired: 5 in, 3 out]
                      n950 = call "2ndOrderDerivate.vi"("t_capture"=w2135, "initial condition"=w2132, "x"=w2132) -> ("dx/dt"=w2137:dbl)  [unwired: 5 in, 3 out]
                    }
                  }
                  n951 = Build Array(w2021, w2017, w2024, w2016, w2023, w2015, w2014, w2013, w2012) -> (w2026:dbl[])
                  n952 = call-poly <vilib>:"Array To Matrix.vi"("Real 1D Array"=w2026) -> ("Real Matrix (Column Vector)"=w2025:T3)
                  n953 = Bundle By Name(cluster=w2020, "x_k|k"=w2025) -> (w2022:T2)
                }
              }
              frame True {
              }
            }
            n954 = Bundle By Name(cluster=w1730, "robots_blue"=w1735, "robots_yellow"=w1734, "balls"=w1726) -> (w1733:T1)
            n955 = Bundle By Name(cluster=w1730, "New"=FALSE) -> (w1731:T1)
          }
          frame 3 {
            n956 = Empty Array?(array=w2255) -> (empty?=w2256:bool)
            n957 = Empty Array?(array=w2263) -> (empty?=w2264:bool)
            n958 = Reciprocal(x=w2265) -> (1/x=w2254:dbl)
            n959 = Empty Array?(array=w2266) -> (empty?=w2267:bool)
            n960 = case shown="False" w2256 {
              tunnel: w2255 -> [w2270 w2287]
              tunnel: w2254 -> [w2271 _]
              tunnel: [w2269 w2287] -> w2253
              tunnel: w2252 -> [w2268 _]
              frame False {
                n961 = for {
                  tunnel: w2270 -> [w2274] mode=indexing
                  tunnel: w2271 -> [_]
                  tunnel: w2270 -> [w2286] mode=indexing
                  tunnel: [w2284] -> w2269 mode=indexing
                  tunnel: w2268 -> [w2273]
                  n962 = Unbundle By Name(w2274) -> ("x"=w2282:sgl, "y"=w2280:sgl, "z"=w2278:sgl)
                  n963 = call "2ndOrderDerivate.vi"("t_capture"=w2273, "initial condition"=w2282, "x"=w2282) -> ("dx/dt"=w2281:dbl)  [unwired: 5 in, 3 out]
                  n964 = call "2ndOrderDerivate.vi"("t_capture"=w2273, "initial condition"=w2280, "x"=w2280) -> ("dx/dt"=w2279:dbl)  [unwired: 5 in, 3 out]
                  n965 = call "2ndOrderDerivate.vi"("t_capture"=w2273, "initial condition"=w2278, "x"=w2278) -> ("dx/dt"=w2283:dbl)  [unwired: 5 in, 3 out]
                  n966 = call "2ndOrderDerivate.vi"("t_capture"=w2273, "initial condition"=w2281, "x"=w2281) -> ("dx/dt"=w2277:dbl)  [unwired: 5 in, 3 out]
                  n967 = call "2ndOrderDerivate.vi"("t_capture"=w2273, "initial condition"=w2279, "x"=w2279) -> ()  [unwired: 5 in, 4 out]
                  n968 = call "2ndOrderDerivate.vi"("t_capture"=w2273, "initial condition"=w2283, "x"=w2283) -> ("dx/dt"=w2276:dbl)  [unwired: 5 in, 3 out]
                  n969 = Build Array(w2282, w2281, w2280, w2279, w2278, w2273, w2277, 2.0 ("element"), w2276) -> (w2272:dbl[])
                  n970 = call-poly <vilib>:"Array To Matrix.vi"("Real 1D Array"=w2272) -> ("Real Matrix (Column Vector)"=w2285:T3)
                  n971 = Bundle By Name(cluster=w2286, "x_k|k"=w2285) -> (w2284:T4)
                }
              }
              frame True {
              }
            }
            n972 = case shown="False" w2264 {
              tunnel: w2263 -> [w2290 w2534]
              tunnel: w2254 -> [w2291 _]
              tunnel: [w2289 w2534] -> w2261
              tunnel: w2252 -> [w2288 _]
              frame False {
                n973 = for {
                  tunnel: w2290 -> [w2309] mode=indexing
                  tunnel: w2291 -> [w2301]
                  tunnel: w2290 -> [w2308] mode=indexing
                  tunnel: [w2302] -> w2289 mode=indexing if=w2300
                  tunnel: w2288 -> [w2299]
                  n974 = Unbundle By Name(w2309) -> ("x"=w2306:sgl, "y"=w2305:sgl, "orientation"=w2307:sgl, "robot_id"=w2292:u32, "Valid"=w2300:bool)
                  n975 = case shown="1" w2292 {
                    tunnel: w2306 -> [w2428 w2435 w2442 w2449 w2456 w2463 w2470 w2477 w2484 w2491 w2498 w2505 w2512 w2519 w2526 w2533]
                    tunnel: w2305 -> [w2426 w2433 w2440 w2447 w2454 w2461 w2468 w2475 w2482 w2489 w2496 w2503 w2510 w2517 w2524 w2531]
                    tunnel: w2307 -> [w2425 w2432 w2439 w2446 w2453 w2460 w2467 w2474 w2481 w2488 w2495 w2502 w2509 w2516 w2523 w2530]
                    tunnel: [w2424 w2431 w2438 w2445 w2452 w2459 w2466 w2473 w2480 w2487 w2494 w2501 w2508 w2515 w2522 w2529] -> w2298
                    tunnel: [w2423 w2430 w2437 w2444 w2451 w2458 w2465 w2472 w2479 w2486 w2493 w2500 w2507 w2514 w2521 w2528] -> w2297
                    tunnel: [w2422 w2429 w2436 w2443 w2450 w2457 w2464 w2471 w2478 w2485 w2492 w2499 w2506 w2513 w2520 w2527] -> w2296
                    tunnel: w2301 -> [_ _ _ _ _ _ _ _ _ _ _ _ _ _ _ _]
                    tunnel: w2299 -> [w2427 w2434 w2441 w2448 w2455 w2462 w2469 w2476 w2483 w2490 w2497 w2504 w2511 w2518 w2525 w2532]
                    frame 0, Default {
                      n976 = call "2ndOrderDerivate.vi"("t_capture"=w2427, "initial condition"=w2428, "x"=w2428) -> ("dx/dt"=w2424:dbl)  [unwired: 5 in, 3 out]
                      n977 = call "2ndOrderDerivate.vi"("t_capture"=w2427, "initial condition"=w2426, "x"=w2426) -> ("dx/dt"=w2423:dbl)  [unwired: 5 in, 3 out]
                      n978 = call "2ndOrderDerivate.vi"("t_capture"=w2427, "initial condition"=w2425, "x"=w2425) -> ("dx/dt"=w2422:dbl)  [unwired: 5 in, 3 out]
                    }
                    frame 1 {
                      n979 = call "2ndOrderDerivate.vi"("t_capture"=w2434, "initial condition"=w2435, "x"=w2435) -> ("dx/dt"=w2431:dbl)  [unwired: 5 in, 3 out]
                      n980 = call "2ndOrderDerivate.vi"("t_capture"=w2434, "initial condition"=w2433, "x"=w2433) -> ("dx/dt"=w2430:dbl)  [unwired: 5 in, 3 out]
                      n981 = call "2ndOrderDerivate.vi"("t_capture"=w2434, "initial condition"=w2432, "x"=w2432) -> ("dx/dt"=w2429:dbl)  [unwired: 5 in, 3 out]
                    }
                    frame 2 {
                      n982 = call "2ndOrderDerivate.vi"("t_capture"=w2441, "initial condition"=w2442, "x"=w2442) -> ("dx/dt"=w2438:dbl)  [unwired: 5 in, 3 out]
                      n983 = call "2ndOrderDerivate.vi"("t_capture"=w2441, "initial condition"=w2440, "x"=w2440) -> ("dx/dt"=w2437:dbl)  [unwired: 5 in, 3 out]
                      n984 = call "2ndOrderDerivate.vi"("t_capture"=w2441, "initial condition"=w2439, "x"=w2439) -> ("dx/dt"=w2436:dbl)  [unwired: 5 in, 3 out]
                    }
                    frame 3 {
                      n985 = call "2ndOrderDerivate.vi"("t_capture"=w2448, "initial condition"=w2449, "x"=w2449) -> ("dx/dt"=w2445:dbl)  [unwired: 5 in, 3 out]
                      n986 = call "2ndOrderDerivate.vi"("t_capture"=w2448, "initial condition"=w2447, "x"=w2447) -> ("dx/dt"=w2444:dbl)  [unwired: 5 in, 3 out]
                      n987 = call "2ndOrderDerivate.vi"("t_capture"=w2448, "initial condition"=w2446, "x"=w2446) -> ("dx/dt"=w2443:dbl)  [unwired: 5 in, 3 out]
                    }
                    frame 4 {
                      n988 = call "2ndOrderDerivate.vi"("t_capture"=w2455, "initial condition"=w2456, "x"=w2456) -> ("dx/dt"=w2452:dbl)  [unwired: 5 in, 3 out]
                      n989 = call "2ndOrderDerivate.vi"("t_capture"=w2455, "initial condition"=w2454, "x"=w2454) -> ("dx/dt"=w2451:dbl)  [unwired: 5 in, 3 out]
                      n990 = call "2ndOrderDerivate.vi"("t_capture"=w2455, "initial condition"=w2453, "x"=w2453) -> ("dx/dt"=w2450:dbl)  [unwired: 5 in, 3 out]
                    }
                    frame 5 {
                      n991 = call "2ndOrderDerivate.vi"("t_capture"=w2462, "initial condition"=w2463, "x"=w2463) -> ("dx/dt"=w2459:dbl)  [unwired: 5 in, 3 out]
                      n992 = call "2ndOrderDerivate.vi"("t_capture"=w2462, "initial condition"=w2461, "x"=w2461) -> ("dx/dt"=w2458:dbl)  [unwired: 5 in, 3 out]
                      n993 = call "2ndOrderDerivate.vi"("t_capture"=w2462, "initial condition"=w2460, "x"=w2460) -> ("dx/dt"=w2457:dbl)  [unwired: 5 in, 3 out]
                    }
                    frame 6 {
                      n994 = call "2ndOrderDerivate.vi"("t_capture"=w2469, "initial condition"=w2470, "x"=w2470) -> ("dx/dt"=w2466:dbl)  [unwired: 5 in, 3 out]
                      n995 = call "2ndOrderDerivate.vi"("t_capture"=w2469, "initial condition"=w2468, "x"=w2468) -> ("dx/dt"=w2465:dbl)  [unwired: 5 in, 3 out]
                      n996 = call "2ndOrderDerivate.vi"("t_capture"=w2469, "initial condition"=w2467, "x"=w2467) -> ("dx/dt"=w2464:dbl)  [unwired: 5 in, 3 out]
                    }
                    frame 7 {
                      n997 = call "2ndOrderDerivate.vi"("t_capture"=w2476, "initial condition"=w2477, "x"=w2477) -> ("dx/dt"=w2473:dbl)  [unwired: 5 in, 3 out]
                      n998 = call "2ndOrderDerivate.vi"("t_capture"=w2476, "initial condition"=w2475, "x"=w2475) -> ("dx/dt"=w2472:dbl)  [unwired: 5 in, 3 out]
                      n999 = call "2ndOrderDerivate.vi"("t_capture"=w2476, "initial condition"=w2474, "x"=w2474) -> ("dx/dt"=w2471:dbl)  [unwired: 5 in, 3 out]
                    }
                    frame 8 {
                      n1000 = call "2ndOrderDerivate.vi"("t_capture"=w2483, "initial condition"=w2484, "x"=w2484) -> ("dx/dt"=w2480:dbl)  [unwired: 5 in, 3 out]
                      n1001 = call "2ndOrderDerivate.vi"("t_capture"=w2483, "initial condition"=w2482, "x"=w2482) -> ("dx/dt"=w2479:dbl)  [unwired: 5 in, 3 out]
                      n1002 = call "2ndOrderDerivate.vi"("t_capture"=w2483, "initial condition"=w2481, "x"=w2481) -> ("dx/dt"=w2478:dbl)  [unwired: 5 in, 3 out]
                    }
                    frame 9 {
                      n1003 = call "2ndOrderDerivate.vi"("t_capture"=w2490, "initial condition"=w2491, "x"=w2491) -> ("dx/dt"=w2487:dbl)  [unwired: 5 in, 3 out]
                      n1004 = call "2ndOrderDerivate.vi"("t_capture"=w2490, "initial condition"=w2489, "x"=w2489) -> ("dx/dt"=w2486:dbl)  [unwired: 5 in, 3 out]
                      n1005 = call "2ndOrderDerivate.vi"("t_capture"=w2490, "initial condition"=w2488, "x"=w2488) -> ("dx/dt"=w2485:dbl)  [unwired: 5 in, 3 out]
                    }
                    frame 10 {
                      n1006 = call "2ndOrderDerivate.vi"("t_capture"=w2497, "initial condition"=w2498, "x"=w2498) -> ("dx/dt"=w2494:dbl)  [unwired: 5 in, 3 out]
                      n1007 = call "2ndOrderDerivate.vi"("t_capture"=w2497, "initial condition"=w2496, "x"=w2496) -> ("dx/dt"=w2493:dbl)  [unwired: 5 in, 3 out]
                      n1008 = call "2ndOrderDerivate.vi"("t_capture"=w2497, "initial condition"=w2495, "x"=w2495) -> ("dx/dt"=w2492:dbl)  [unwired: 5 in, 3 out]
                    }
                    frame 11 {
                      n1009 = call "2ndOrderDerivate.vi"("t_capture"=w2504, "initial condition"=w2505, "x"=w2505) -> ("dx/dt"=w2501:dbl)  [unwired: 5 in, 3 out]
                      n1010 = call "2ndOrderDerivate.vi"("t_capture"=w2504, "initial condition"=w2503, "x"=w2503) -> ("dx/dt"=w2500:dbl)  [unwired: 5 in, 3 out]
                      n1011 = call "2ndOrderDerivate.vi"("t_capture"=w2504, "initial condition"=w2502, "x"=w2502) -> ("dx/dt"=w2499:dbl)  [unwired: 5 in, 3 out]
                    }
                    frame 12 {
                      n1012 = call "2ndOrderDerivate.vi"("t_capture"=w2511, "initial condition"=w2512, "x"=w2512) -> ("dx/dt"=w2508:dbl)  [unwired: 5 in, 3 out]
                      n1013 = call "2ndOrderDerivate.vi"("t_capture"=w2511, "initial condition"=w2510, "x"=w2510) -> ("dx/dt"=w2507:dbl)  [unwired: 5 in, 3 out]
                      n1014 = call "2ndOrderDerivate.vi"("t_capture"=w2511, "initial condition"=w2509, "x"=w2509) -> ("dx/dt"=w2506:dbl)  [unwired: 5 in, 3 out]
                    }
                    frame 13 {
                      n1015 = call "2ndOrderDerivate.vi"("t_capture"=w2518, "initial condition"=w2519, "x"=w2519) -> ("dx/dt"=w2515:dbl)  [unwired: 5 in, 3 out]
                      n1016 = call "2ndOrderDerivate.vi"("t_capture"=w2518, "initial condition"=w2517, "x"=w2517) -> ("dx/dt"=w2514:dbl)  [unwired: 5 in, 3 out]
                      n1017 = call "2ndOrderDerivate.vi"("t_capture"=w2518, "initial condition"=w2516, "x"=w2516) -> ("dx/dt"=w2513:dbl)  [unwired: 5 in, 3 out]
                    }
                    frame 14 {
                      n1018 = call "2ndOrderDerivate.vi"("t_capture"=w2525, "initial condition"=w2526, "x"=w2526) -> ("dx/dt"=w2522:dbl)  [unwired: 5 in, 3 out]
                      n1019 = call "2ndOrderDerivate.vi"("t_capture"=w2525, "initial condition"=w2524, "x"=w2524) -> ("dx/dt"=w2521:dbl)  [unwired: 5 in, 3 out]
                      n1020 = call "2ndOrderDerivate.vi"("t_capture"=w2525, "initial condition"=w2523, "x"=w2523) -> ("dx/dt"=w2520:dbl)  [unwired: 5 in, 3 out]
                    }
                    frame 15 {
                      n1021 = call "2ndOrderDerivate.vi"("t_capture"=w2532, "initial condition"=w2533, "x"=w2533) -> ("dx/dt"=w2529:dbl)  [unwired: 5 in, 3 out]
                      n1022 = call "2ndOrderDerivate.vi"("t_capture"=w2532, "initial condition"=w2531, "x"=w2531) -> ("dx/dt"=w2528:dbl)  [unwired: 5 in, 3 out]
                      n1023 = call "2ndOrderDerivate.vi"("t_capture"=w2532, "initial condition"=w2530, "x"=w2530) -> ("dx/dt"=w2527:dbl)  [unwired: 5 in, 3 out]
                    }
                  }
                  n1024 = case shown="1" w2292 {
                    tunnel: w2298 -> [w2316 w2323 w2330 w2337 w2344 w2351 w2358 w2365 w2372 w2379 w2386 w2393 w2400 w2407 w2414 w2421]
                    tunnel: w2297 -> [w2314 w2321 w2328 w2335 w2342 w2349 w2356 w2363 w2370 w2377 w2384 w2391 w2398 w2405 w2412 w2419]
                    tunnel: w2296 -> [w2313 w2320 w2327 w2334 w2341 w2348 w2355 w2362 w2369 w2376 w2383 w2390 w2397 w2404 w2411 w2418]
                    tunnel: [w2312 w2319 w2326 w2333 w2340 w2347 w2354 w2361 w2368 w2375 w2382 w2389 w2396 w2403 w2410 w2417] -> w2295
                    tunnel: [w2311 w2318 w2325 w2332 w2339 w2346 w2353 w2360 w2367 w2374 w2381 w2388 w2395 w2402 w2409 w2416] -> w2294
                    tunnel: [w2310 w2317 w2324 w2331 w2338 w2345 w2352 w2359 w2366 w2373 w2380 w2387 w2394 w2401 w2408 w2415] -> w2293
                    tunnel: w2299 -> [w2315 w2322 w2329 w2336 w2343 w2350 w2357 w2364 w2371 w2378 w2385 w2392 w2399 w2406 w2413 w2420]
                    frame 0, Default {
                      n1025 = call "2ndOrderDerivate.vi"("t_capture"=w2315, "initial condition"=w2316, "x"=w2316) -> ("dx/dt"=w2312:dbl)  [unwired: 5 in, 3 out]
                      n1026 = call "2ndOrderDerivate.vi"("t_capture"=w2315, "initial condition"=w2314, "x"=w2314) -> ("dx/dt"=w2311:dbl)  [unwired: 5 in, 3 out]
                      n1027 = call "2ndOrderDerivate.vi"("t_capture"=w2315, "initial condition"=w2313, "x"=w2313) -> ("dx/dt"=w2310:dbl)  [unwired: 5 in, 3 out]
                    }
                    frame 1 {
                      n1028 = call "2ndOrderDerivate.vi"("t_capture"=w2322, "initial condition"=w2323, "x"=w2323) -> ("dx/dt"=w2319:dbl)  [unwired: 5 in, 3 out]
                      n1029 = call "2ndOrderDerivate.vi"("t_capture"=w2322, "initial condition"=w2321, "x"=w2321) -> ("dx/dt"=w2318:dbl)  [unwired: 5 in, 3 out]
                      n1030 = call "2ndOrderDerivate.vi"("t_capture"=w2322, "initial condition"=w2320, "x"=w2320) -> ("dx/dt"=w2317:dbl)  [unwired: 5 in, 3 out]
                    }
                    frame 2 {
                      n1031 = call "2ndOrderDerivate.vi"("t_capture"=w2329, "initial condition"=w2330, "x"=w2330) -> ("dx/dt"=w2326:dbl)  [unwired: 5 in, 3 out]
                      n1032 = call "2ndOrderDerivate.vi"("t_capture"=w2329, "initial condition"=w2328, "x"=w2328) -> ("dx/dt"=w2325:dbl)  [unwired: 5 in, 3 out]
                      n1033 = call "2ndOrderDerivate.vi"("t_capture"=w2329, "initial condition"=w2327, "x"=w2327) -> ("dx/dt"=w2324:dbl)  [unwired: 5 in, 3 out]
                    }
                    frame 3 {
                      n1034 = call "2ndOrderDerivate.vi"("t_capture"=w2336, "initial condition"=w2337, "x"=w2337) -> ("dx/dt"=w2333:dbl)  [unwired: 5 in, 3 out]
                      n1035 = call "2ndOrderDerivate.vi"("t_capture"=w2336, "initial condition"=w2335, "x"=w2335) -> ("dx/dt"=w2332:dbl)  [unwired: 5 in, 3 out]
                      n1036 = call "2ndOrderDerivate.vi"("t_capture"=w2336, "initial condition"=w2334, "x"=w2334) -> ("dx/dt"=w2331:dbl)  [unwired: 5 in, 3 out]
                    }
                    frame 4 {
                      n1037 = call "2ndOrderDerivate.vi"("t_capture"=w2343, "initial condition"=w2344, "x"=w2344) -> ("dx/dt"=w2340:dbl)  [unwired: 5 in, 3 out]
                      n1038 = call "2ndOrderDerivate.vi"("t_capture"=w2343, "initial condition"=w2342, "x"=w2342) -> ("dx/dt"=w2339:dbl)  [unwired: 5 in, 3 out]
                      n1039 = call "2ndOrderDerivate.vi"("t_capture"=w2343, "initial condition"=w2341, "x"=w2341) -> ("dx/dt"=w2338:dbl)  [unwired: 5 in, 3 out]
                    }
                    frame 5 {
                      n1040 = call "2ndOrderDerivate.vi"("t_capture"=w2350, "initial condition"=w2351, "x"=w2351) -> ("dx/dt"=w2347:dbl)  [unwired: 5 in, 3 out]
                      n1041 = call "2ndOrderDerivate.vi"("t_capture"=w2350, "initial condition"=w2349, "x"=w2349) -> ("dx/dt"=w2346:dbl)  [unwired: 5 in, 3 out]
                      n1042 = call "2ndOrderDerivate.vi"("t_capture"=w2350, "initial condition"=w2348, "x"=w2348) -> ("dx/dt"=w2345:dbl)  [unwired: 5 in, 3 out]
                    }
                    frame 6 {
                      n1043 = call "2ndOrderDerivate.vi"("t_capture"=w2357, "initial condition"=w2358, "x"=w2358) -> ("dx/dt"=w2354:dbl)  [unwired: 5 in, 3 out]
                      n1044 = call "2ndOrderDerivate.vi"("t_capture"=w2357, "initial condition"=w2356, "x"=w2356) -> ("dx/dt"=w2353:dbl)  [unwired: 5 in, 3 out]
                      n1045 = call "2ndOrderDerivate.vi"("t_capture"=w2357, "initial condition"=w2355, "x"=w2355) -> ("dx/dt"=w2352:dbl)  [unwired: 5 in, 3 out]
                    }
                    frame 7 {
                      n1046 = call "2ndOrderDerivate.vi"("t_capture"=w2364, "initial condition"=w2365, "x"=w2365) -> ("dx/dt"=w2361:dbl)  [unwired: 5 in, 3 out]
                      n1047 = call "2ndOrderDerivate.vi"("t_capture"=w2364, "initial condition"=w2363, "x"=w2363) -> ("dx/dt"=w2360:dbl)  [unwired: 5 in, 3 out]
                      n1048 = call "2ndOrderDerivate.vi"("t_capture"=w2364, "initial condition"=w2362, "x"=w2362) -> ("dx/dt"=w2359:dbl)  [unwired: 5 in, 3 out]
                    }
                    frame 8 {
                      n1049 = call "2ndOrderDerivate.vi"("t_capture"=w2371, "initial condition"=w2372, "x"=w2372) -> ("dx/dt"=w2368:dbl)  [unwired: 5 in, 3 out]
                      n1050 = call "2ndOrderDerivate.vi"("t_capture"=w2371, "initial condition"=w2370, "x"=w2370) -> ("dx/dt"=w2367:dbl)  [unwired: 5 in, 3 out]
                      n1051 = call "2ndOrderDerivate.vi"("t_capture"=w2371, "initial condition"=w2369, "x"=w2369) -> ("dx/dt"=w2366:dbl)  [unwired: 5 in, 3 out]
                    }
                    frame 9 {
                      n1052 = call "2ndOrderDerivate.vi"("t_capture"=w2378, "initial condition"=w2379, "x"=w2379) -> ("dx/dt"=w2375:dbl)  [unwired: 5 in, 3 out]
                      n1053 = call "2ndOrderDerivate.vi"("t_capture"=w2378, "initial condition"=w2377, "x"=w2377) -> ("dx/dt"=w2374:dbl)  [unwired: 5 in, 3 out]
                      n1054 = call "2ndOrderDerivate.vi"("t_capture"=w2378, "initial condition"=w2376, "x"=w2376) -> ("dx/dt"=w2373:dbl)  [unwired: 5 in, 3 out]
                    }
                    frame 10 {
                      n1055 = call "2ndOrderDerivate.vi"("t_capture"=w2385, "initial condition"=w2386, "x"=w2386) -> ("dx/dt"=w2382:dbl)  [unwired: 5 in, 3 out]
                      n1056 = call "2ndOrderDerivate.vi"("t_capture"=w2385, "initial condition"=w2384, "x"=w2384) -> ("dx/dt"=w2381:dbl)  [unwired: 5 in, 3 out]
                      n1057 = call "2ndOrderDerivate.vi"("t_capture"=w2385, "initial condition"=w2383, "x"=w2383) -> ("dx/dt"=w2380:dbl)  [unwired: 5 in, 3 out]
                    }
                    frame 11 {
                      n1058 = call "2ndOrderDerivate.vi"("t_capture"=w2392, "initial condition"=w2393, "x"=w2393) -> ("dx/dt"=w2389:dbl)  [unwired: 5 in, 3 out]
                      n1059 = call "2ndOrderDerivate.vi"("t_capture"=w2392, "initial condition"=w2391, "x"=w2391) -> ("dx/dt"=w2388:dbl)  [unwired: 5 in, 3 out]
                      n1060 = call "2ndOrderDerivate.vi"("t_capture"=w2392, "initial condition"=w2390, "x"=w2390) -> ("dx/dt"=w2387:dbl)  [unwired: 5 in, 3 out]
                    }
                    frame 12 {
                      n1061 = call "2ndOrderDerivate.vi"("t_capture"=w2399, "initial condition"=w2400, "x"=w2400) -> ("dx/dt"=w2396:dbl)  [unwired: 5 in, 3 out]
                      n1062 = call "2ndOrderDerivate.vi"("t_capture"=w2399, "initial condition"=w2398, "x"=w2398) -> ("dx/dt"=w2395:dbl)  [unwired: 5 in, 3 out]
                      n1063 = call "2ndOrderDerivate.vi"("t_capture"=w2399, "initial condition"=w2397, "x"=w2397) -> ("dx/dt"=w2394:dbl)  [unwired: 5 in, 3 out]
                    }
                    frame 13 {
                      n1064 = call "2ndOrderDerivate.vi"("t_capture"=w2406, "initial condition"=w2407, "x"=w2407) -> ("dx/dt"=w2403:dbl)  [unwired: 5 in, 3 out]
                      n1065 = call "2ndOrderDerivate.vi"("t_capture"=w2406, "initial condition"=w2405, "x"=w2405) -> ("dx/dt"=w2402:dbl)  [unwired: 5 in, 3 out]
                      n1066 = call "2ndOrderDerivate.vi"("t_capture"=w2406, "initial condition"=w2404, "x"=w2404) -> ("dx/dt"=w2401:dbl)  [unwired: 5 in, 3 out]
                    }
                    frame 14 {
                      n1067 = call "2ndOrderDerivate.vi"("t_capture"=w2413, "initial condition"=w2414, "x"=w2414) -> ("dx/dt"=w2410:dbl)  [unwired: 5 in, 3 out]
                      n1068 = call "2ndOrderDerivate.vi"("t_capture"=w2413, "initial condition"=w2412, "x"=w2412) -> ("dx/dt"=w2409:dbl)  [unwired: 5 in, 3 out]
                      n1069 = call "2ndOrderDerivate.vi"("t_capture"=w2413, "initial condition"=w2411, "x"=w2411) -> ("dx/dt"=w2408:dbl)  [unwired: 5 in, 3 out]
                    }
                    frame 15 {
                      n1070 = call "2ndOrderDerivate.vi"("t_capture"=w2420, "initial condition"=w2421, "x"=w2421) -> ("dx/dt"=w2417:dbl)  [unwired: 5 in, 3 out]
                      n1071 = call "2ndOrderDerivate.vi"("t_capture"=w2420, "initial condition"=w2419, "x"=w2419) -> ("dx/dt"=w2416:dbl)  [unwired: 5 in, 3 out]
                      n1072 = call "2ndOrderDerivate.vi"("t_capture"=w2420, "initial condition"=w2418, "x"=w2418) -> ("dx/dt"=w2415:dbl)  [unwired: 5 in, 3 out]
                    }
                  }
                  n1073 = Build Array(w2306, w2298, w2305, w2297, w2307, w2296, w2295, w2294, w2293) -> (w2304:dbl[])
                  n1074 = call-poly <vilib>:"Array To Matrix.vi"("Real 1D Array"=w2304) -> ("Real Matrix (Column Vector)"=w2303:T3)
                  n1075 = Bundle By Name(cluster=w2308, "x_k|k"=w2303) -> (w2302:T2)
                }
              }
              frame True {
              }
            }
            n1076 = case shown="False" w2267 {
              tunnel: w2266 -> [w2537 w2778]
              tunnel: w2254 -> [w2538 _]
              tunnel: [w2536 w2778] -> w2262
              tunnel: w2252 -> [w2535 _]
              frame False {
                n1077 = for {
                  tunnel: w2537 -> [w2547] mode=indexing
                  tunnel: w2538 -> [_]
                  tunnel: [w2549] -> w2536 mode=indexing
                  tunnel: w2535 -> [w2546]
                  n1078 = Unbundle By Name(w2547) -> ("x"=w2548:sgl, "y"=w2551:sgl, "orientation"=w2550:sgl, "robot_id"=w2545:u32)  [unwired: 1 out]
                  n1079 = case shown="0, Default" w2545 {
                    tunnel: w2548 -> [w2668 w2675 w2682 w2689 w2696 w2703 w2710 w2717 w2724 w2731 w2738 w2745 w2752 w2759 w2766 w2773]
                    tunnel: [w2670 w2677 w2684 w2691 w2698 w2705 w2712 w2719 w2726 w2733 w2740 w2747 w2754 w2761 w2768 w2775] -> w2544
                    tunnel: [w2672 w2679 w2686 w2693 w2700 w2707 w2714 w2721 w2728 w2735 w2742 w2749 w2756 w2763 w2770 w2777] -> w2543
                    tunnel: [w2671 w2678 w2685 w2692 w2699 w2706 w2713 w2720 w2727 w2734 w2741 w2748 w2755 w2762 w2769 w2776] -> w2542
                    tunnel: w2551 -> [w2667 w2674 w2681 w2688 w2695 w2702 w2709 w2716 w2723 w2730 w2737 w2744 w2751 w2758 w2765 w2772]
                    tunnel: w2550 -> [w2666 w2673 w2680 w2687 w2694 w2701 w2708 w2715 w2722 w2729 w2736 w2743 w2750 w2757 w2764 w2771]
                    tunnel: w2546 -> [w2669 w2676 w2683 w2690 w2697 w2704 w2711 w2718 w2725 w2732 w2739 w2746 w2753 w2760 w2767 w2774]
                    frame 0, Default {
                      n1080 = call "2ndOrderDerivate.vi"("t_capture"=w2669, "initial condition"=w2668, "x"=w2668) -> ("dx/dt"=w2670:dbl)  [unwired: 5 in, 3 out]
                      n1081 = call "2ndOrderDerivate.vi"("t_capture"=w2669, "initial condition"=w2667, "x"=w2667) -> ("dx/dt"=w2672:dbl)  [unwired: 5 in, 3 out]
                      n1082 = call "2ndOrderDerivate.vi"("t_capture"=w2669, "initial condition"=w2666, "x"=w2666) -> ("dx/dt"=w2671:dbl)  [unwired: 5 in, 3 out]
                    }
                    frame 1 {
                      n1083 = call "2ndOrderDerivate.vi"("t_capture"=w2676, "initial condition"=w2675, "x"=w2675) -> ("dx/dt"=w2677:dbl)  [unwired: 5 in, 3 out]
                      n1084 = call "2ndOrderDerivate.vi"("t_capture"=w2676, "initial condition"=w2674, "x"=w2674) -> ("dx/dt"=w2679:dbl)  [unwired: 5 in, 3 out]
                      n1085 = call "2ndOrderDerivate.vi"("t_capture"=w2676, "initial condition"=w2673, "x"=w2673) -> ("dx/dt"=w2678:dbl)  [unwired: 5 in, 3 out]
                    }
                    frame 2 {
                      n1086 = call "2ndOrderDerivate.vi"("t_capture"=w2683, "initial condition"=w2682, "x"=w2682) -> ("dx/dt"=w2684:dbl)  [unwired: 5 in, 3 out]
                      n1087 = call "2ndOrderDerivate.vi"("t_capture"=w2683, "initial condition"=w2681, "x"=w2681) -> ("dx/dt"=w2686:dbl)  [unwired: 5 in, 3 out]
                      n1088 = call "2ndOrderDerivate.vi"("t_capture"=w2683, "initial condition"=w2680, "x"=w2680) -> ("dx/dt"=w2685:dbl)  [unwired: 5 in, 3 out]
                    }
                    frame 3 {
                      n1089 = call "2ndOrderDerivate.vi"("t_capture"=w2690, "initial condition"=w2689, "x"=w2689) -> ("dx/dt"=w2691:dbl)  [unwired: 5 in, 3 out]
                      n1090 = call "2ndOrderDerivate.vi"("t_capture"=w2690, "initial condition"=w2688, "x"=w2688) -> ("dx/dt"=w2693:dbl)  [unwired: 5 in, 3 out]
                      n1091 = call "2ndOrderDerivate.vi"("t_capture"=w2690, "initial condition"=w2687, "x"=w2687) -> ("dx/dt"=w2692:dbl)  [unwired: 5 in, 3 out]
                    }
                    frame 4 {
                      n1092 = call "2ndOrderDerivate.vi"("t_capture"=w2697, "initial condition"=w2696, "x"=w2696) -> ("dx/dt"=w2698:dbl)  [unwired: 5 in, 3 out]
                      n1093 = call "2ndOrderDerivate.vi"("t_capture"=w2697, "initial condition"=w2695, "x"=w2695) -> ("dx/dt"=w2700:dbl)  [unwired: 5 in, 3 out]
                      n1094 = call "2ndOrderDerivate.vi"("t_capture"=w2697, "initial condition"=w2694, "x"=w2694) -> ("dx/dt"=w2699:dbl)  [unwired: 5 in, 3 out]
                    }
                    frame 5 {
                      n1095 = call "2ndOrderDerivate.vi"("t_capture"=w2704, "initial condition"=w2703, "x"=w2703) -> ("dx/dt"=w2705:dbl)  [unwired: 5 in, 3 out]
                      n1096 = call "2ndOrderDerivate.vi"("t_capture"=w2704, "initial condition"=w2702, "x"=w2702) -> ("dx/dt"=w2707:dbl)  [unwired: 5 in, 3 out]
                      n1097 = call "2ndOrderDerivate.vi"("t_capture"=w2704, "initial condition"=w2701, "x"=w2701) -> ("dx/dt"=w2706:dbl)  [unwired: 5 in, 3 out]
                    }
                    frame 6 {
                      n1098 = call "2ndOrderDerivate.vi"("t_capture"=w2711, "initial condition"=w2710, "x"=w2710) -> ("dx/dt"=w2712:dbl)  [unwired: 5 in, 3 out]
                      n1099 = call "2ndOrderDerivate.vi"("t_capture"=w2711, "initial condition"=w2709, "x"=w2709) -> ("dx/dt"=w2714:dbl)  [unwired: 5 in, 3 out]
                      n1100 = call "2ndOrderDerivate.vi"("t_capture"=w2711, "initial condition"=w2708, "x"=w2708) -> ("dx/dt"=w2713:dbl)  [unwired: 5 in, 3 out]
                    }
                    frame 7 {
                      n1101 = call "2ndOrderDerivate.vi"("t_capture"=w2718, "initial condition"=w2717, "x"=w2717) -> ("dx/dt"=w2719:dbl)  [unwired: 5 in, 3 out]
                      n1102 = call "2ndOrderDerivate.vi"("t_capture"=w2718, "initial condition"=w2716, "x"=w2716) -> ("dx/dt"=w2721:dbl)  [unwired: 5 in, 3 out]
                      n1103 = call "2ndOrderDerivate.vi"("t_capture"=w2718, "initial condition"=w2715, "x"=w2715) -> ("dx/dt"=w2720:dbl)  [unwired: 5 in, 3 out]
                    }
                    frame 8 {
                      n1104 = call "2ndOrderDerivate.vi"("t_capture"=w2725, "initial condition"=w2724, "x"=w2724) -> ("dx/dt"=w2726:dbl)  [unwired: 5 in, 3 out]
                      n1105 = call "2ndOrderDerivate.vi"("t_capture"=w2725, "initial condition"=w2723, "x"=w2723) -> ("dx/dt"=w2728:dbl)  [unwired: 5 in, 3 out]
                      n1106 = call "2ndOrderDerivate.vi"("t_capture"=w2725, "initial condition"=w2722, "x"=w2722) -> ("dx/dt"=w2727:dbl)  [unwired: 5 in, 3 out]
                    }
                    frame 9 {
                      n1107 = call "2ndOrderDerivate.vi"("t_capture"=w2732, "initial condition"=w2731, "x"=w2731) -> ("dx/dt"=w2733:dbl)  [unwired: 5 in, 3 out]
                      n1108 = call "2ndOrderDerivate.vi"("t_capture"=w2732, "initial condition"=w2730, "x"=w2730) -> ("dx/dt"=w2735:dbl)  [unwired: 5 in, 3 out]
                      n1109 = call "2ndOrderDerivate.vi"("t_capture"=w2732, "initial condition"=w2729, "x"=w2729) -> ("dx/dt"=w2734:dbl)  [unwired: 5 in, 3 out]
                    }
                    frame 10 {
                      n1110 = call "2ndOrderDerivate.vi"("t_capture"=w2739, "initial condition"=w2738, "x"=w2738) -> ("dx/dt"=w2740:dbl)  [unwired: 5 in, 3 out]
                      n1111 = call "2ndOrderDerivate.vi"("t_capture"=w2739, "initial condition"=w2737, "x"=w2737) -> ("dx/dt"=w2742:dbl)  [unwired: 5 in, 3 out]
                      n1112 = call "2ndOrderDerivate.vi"("t_capture"=w2739, "initial condition"=w2736, "x"=w2736) -> ("dx/dt"=w2741:dbl)  [unwired: 5 in, 3 out]
                    }
                    frame 11 {
                      n1113 = call "2ndOrderDerivate.vi"("t_capture"=w2746, "initial condition"=w2745, "x"=w2745) -> ("dx/dt"=w2747:dbl)  [unwired: 5 in, 3 out]
                      n1114 = call "2ndOrderDerivate.vi"("t_capture"=w2746, "initial condition"=w2744, "x"=w2744) -> ("dx/dt"=w2749:dbl)  [unwired: 5 in, 3 out]
                      n1115 = call "2ndOrderDerivate.vi"("t_capture"=w2746, "initial condition"=w2743, "x"=w2743) -> ("dx/dt"=w2748:dbl)  [unwired: 5 in, 3 out]
                    }
                    frame 12 {
                      n1116 = call "2ndOrderDerivate.vi"("t_capture"=w2753, "initial condition"=w2752, "x"=w2752) -> ("dx/dt"=w2754:dbl)  [unwired: 5 in, 3 out]
                      n1117 = call "2ndOrderDerivate.vi"("t_capture"=w2753, "initial condition"=w2751, "x"=w2751) -> ("dx/dt"=w2756:dbl)  [unwired: 5 in, 3 out]
                      n1118 = call "2ndOrderDerivate.vi"("t_capture"=w2753, "initial condition"=w2750, "x"=w2750) -> ("dx/dt"=w2755:dbl)  [unwired: 5 in, 3 out]
                    }
                    frame 13 {
                      n1119 = call "2ndOrderDerivate.vi"("t_capture"=w2760, "initial condition"=w2759, "x"=w2759) -> ("dx/dt"=w2761:dbl)  [unwired: 5 in, 3 out]
                      n1120 = call "2ndOrderDerivate.vi"("t_capture"=w2760, "initial condition"=w2758, "x"=w2758) -> ("dx/dt"=w2763:dbl)  [unwired: 5 in, 3 out]
                      n1121 = call "2ndOrderDerivate.vi"("t_capture"=w2760, "initial condition"=w2757, "x"=w2757) -> ("dx/dt"=w2762:dbl)  [unwired: 5 in, 3 out]
                    }
                    frame 14 {
                      n1122 = call "2ndOrderDerivate.vi"("t_capture"=w2767, "initial condition"=w2766, "x"=w2766) -> ("dx/dt"=w2768:dbl)  [unwired: 5 in, 3 out]
                      n1123 = call "2ndOrderDerivate.vi"("t_capture"=w2767, "initial condition"=w2765, "x"=w2765) -> ("dx/dt"=w2770:dbl)  [unwired: 5 in, 3 out]
                      n1124 = call "2ndOrderDerivate.vi"("t_capture"=w2767, "initial condition"=w2764, "x"=w2764) -> ("dx/dt"=w2769:dbl)  [unwired: 5 in, 3 out]
                    }
                    frame 15 {
                      n1125 = call "2ndOrderDerivate.vi"("t_capture"=w2774, "initial condition"=w2773, "x"=w2773) -> ("dx/dt"=w2775:dbl)  [unwired: 5 in, 3 out]
                      n1126 = call "2ndOrderDerivate.vi"("t_capture"=w2774, "initial condition"=w2772, "x"=w2772) -> ("dx/dt"=w2777:dbl)  [unwired: 5 in, 3 out]
                      n1127 = call "2ndOrderDerivate.vi"("t_capture"=w2774, "initial condition"=w2771, "x"=w2771) -> ("dx/dt"=w2776:dbl)  [unwired: 5 in, 3 out]
                    }
                  }
                  n1128 = case shown="0, Default" w2545 {
                    tunnel: w2544 -> [w2556 w2563 w2570 w2577 w2584 w2591 w2598 w2605 w2612 w2619 w2626 w2633 w2640 w2647 w2654 w2661]
                    tunnel: [w2558 w2565 w2572 w2579 w2586 w2593 w2600 w2607 w2614 w2621 w2628 w2635 w2642 w2649 w2656 w2663] -> w2541
                    tunnel: [w2560 w2567 w2574 w2581 w2588 w2595 w2602 w2609 w2616 w2623 w2630 w2637 w2644 w2651 w2658 w2665] -> w2540
                    tunnel: [w2559 w2566 w2573 w2580 w2587 w2594 w2601 w2608 w2615 w2622 w2629 w2636 w2643 w2650 w2657 w2664] -> w2539
                    tunnel: w2543 -> [w2555 w2562 w2569 w2576 w2583 w2590 w2597 w2604 w2611 w2618 w2625 w2632 w2639 w2646 w2653 w2660]
                    tunnel: w2542 -> [w2554 w2561 w2568 w2575 w2582 w2589 w2596 w2603 w2610 w2617 w2624 w2631 w2638 w2645 w2652 w2659]
                    tunnel: w2546 -> [w2557 w2564 w2571 w2578 w2585 w2592 w2599 w2606 w2613 w2620 w2627 w2634 w2641 w2648 w2655 w2662]
                    frame 0, Default {
                      n1129 = call "2ndOrderDerivate.vi"("t_capture"=w2557, "initial condition"=w2556, "x"=w2556) -> ("dx/dt"=w2558:dbl)  [unwired: 5 in, 3 out]
                      n1130 = call "2ndOrderDerivate.vi"("t_capture"=w2557, "initial condition"=w2555, "x"=w2555) -> ("dx/dt"=w2560:dbl)  [unwired: 5 in, 3 out]
                      n1131 = call "2ndOrderDerivate.vi"("t_capture"=w2557, "initial condition"=w2554, "x"=w2554) -> ("dx/dt"=w2559:dbl)  [unwired: 5 in, 3 out]
                    }
                    frame 1 {
                      n1132 = call "2ndOrderDerivate.vi"("t_capture"=w2564, "initial condition"=w2563, "x"=w2563) -> ("dx/dt"=w2565:dbl)  [unwired: 5 in, 3 out]
                      n1133 = call "2ndOrderDerivate.vi"("t_capture"=w2564, "initial condition"=w2562, "x"=w2562) -> ("dx/dt"=w2567:dbl)  [unwired: 5 in, 3 out]
                      n1134 = call "2ndOrderDerivate.vi"("t_capture"=w2564, "initial condition"=w2561, "x"=w2561) -> ("dx/dt"=w2566:dbl)  [unwired: 5 in, 3 out]
                    }
                    frame 2 {
                      n1135 = call "2ndOrderDerivate.vi"("t_capture"=w2571, "initial condition"=w2570, "x"=w2570) -> ("dx/dt"=w2572:dbl)  [unwired: 5 in, 3 out]
                      n1136 = call "2ndOrderDerivate.vi"("t_capture"=w2571, "initial condition"=w2569, "x"=w2569) -> ("dx/dt"=w2574:dbl)  [unwired: 5 in, 3 out]
                      n1137 = call "2ndOrderDerivate.vi"("t_capture"=w2571, "initial condition"=w2568, "x"=w2568) -> ("dx/dt"=w2573:dbl)  [unwired: 5 in, 3 out]
                    }
                    frame 3 {
                      n1138 = call "2ndOrderDerivate.vi"("t_capture"=w2578, "initial condition"=w2577, "x"=w2577) -> ("dx/dt"=w2579:dbl)  [unwired: 5 in, 3 out]
                      n1139 = call "2ndOrderDerivate.vi"("t_capture"=w2578, "initial condition"=w2576, "x"=w2576) -> ("dx/dt"=w2581:dbl)  [unwired: 5 in, 3 out]
                      n1140 = call "2ndOrderDerivate.vi"("t_capture"=w2578, "initial condition"=w2575, "x"=w2575) -> ("dx/dt"=w2580:dbl)  [unwired: 5 in, 3 out]
                    }
                    frame 4 {
                      n1141 = call "2ndOrderDerivate.vi"("t_capture"=w2585, "initial condition"=w2584, "x"=w2584) -> ("dx/dt"=w2586:dbl)  [unwired: 5 in, 3 out]
                      n1142 = call "2ndOrderDerivate.vi"("t_capture"=w2585, "initial condition"=w2583, "x"=w2583) -> ("dx/dt"=w2588:dbl)  [unwired: 5 in, 3 out]
                      n1143 = call "2ndOrderDerivate.vi"("t_capture"=w2585, "initial condition"=w2582, "x"=w2582) -> ("dx/dt"=w2587:dbl)  [unwired: 5 in, 3 out]
                    }
                    frame 5 {
                      n1144 = call "2ndOrderDerivate.vi"("t_capture"=w2592, "initial condition"=w2591, "x"=w2591) -> ("dx/dt"=w2593:dbl)  [unwired: 5 in, 3 out]
                      n1145 = call "2ndOrderDerivate.vi"("t_capture"=w2592, "initial condition"=w2590, "x"=w2590) -> ("dx/dt"=w2595:dbl)  [unwired: 5 in, 3 out]
                      n1146 = call "2ndOrderDerivate.vi"("t_capture"=w2592, "initial condition"=w2589, "x"=w2589) -> ("dx/dt"=w2594:dbl)  [unwired: 5 in, 3 out]
                    }
                    frame 6 {
                      n1147 = call "2ndOrderDerivate.vi"("t_capture"=w2599, "initial condition"=w2598, "x"=w2598) -> ("dx/dt"=w2600:dbl)  [unwired: 5 in, 3 out]
                      n1148 = call "2ndOrderDerivate.vi"("t_capture"=w2599, "initial condition"=w2597, "x"=w2597) -> ("dx/dt"=w2602:dbl)  [unwired: 5 in, 3 out]
                      n1149 = call "2ndOrderDerivate.vi"("t_capture"=w2599, "initial condition"=w2596, "x"=w2596) -> ("dx/dt"=w2601:dbl)  [unwired: 5 in, 3 out]
                    }
                    frame 7 {
                      n1150 = call "2ndOrderDerivate.vi"("t_capture"=w2606, "initial condition"=w2605, "x"=w2605) -> ("dx/dt"=w2607:dbl)  [unwired: 5 in, 3 out]
                      n1151 = call "2ndOrderDerivate.vi"("t_capture"=w2606, "initial condition"=w2604, "x"=w2604) -> ("dx/dt"=w2609:dbl)  [unwired: 5 in, 3 out]
                      n1152 = call "2ndOrderDerivate.vi"("t_capture"=w2606, "initial condition"=w2603, "x"=w2603) -> ("dx/dt"=w2608:dbl)  [unwired: 5 in, 3 out]
                    }
                    frame 8 {
                      n1153 = call "2ndOrderDerivate.vi"("t_capture"=w2613, "initial condition"=w2612, "x"=w2612) -> ("dx/dt"=w2614:dbl)  [unwired: 5 in, 3 out]
                      n1154 = call "2ndOrderDerivate.vi"("t_capture"=w2613, "initial condition"=w2611, "x"=w2611) -> ("dx/dt"=w2616:dbl)  [unwired: 5 in, 3 out]
                      n1155 = call "2ndOrderDerivate.vi"("t_capture"=w2613, "initial condition"=w2610, "x"=w2610) -> ("dx/dt"=w2615:dbl)  [unwired: 5 in, 3 out]
                    }
                    frame 9 {
                      n1156 = call "2ndOrderDerivate.vi"("t_capture"=w2620, "initial condition"=w2619, "x"=w2619) -> ("dx/dt"=w2621:dbl)  [unwired: 5 in, 3 out]
                      n1157 = call "2ndOrderDerivate.vi"("t_capture"=w2620, "initial condition"=w2618, "x"=w2618) -> ("dx/dt"=w2623:dbl)  [unwired: 5 in, 3 out]
                      n1158 = call "2ndOrderDerivate.vi"("t_capture"=w2620, "initial condition"=w2617, "x"=w2617) -> ("dx/dt"=w2622:dbl)  [unwired: 5 in, 3 out]
                    }
                    frame 10 {
                      n1159 = call "2ndOrderDerivate.vi"("t_capture"=w2627, "initial condition"=w2626, "x"=w2626) -> ("dx/dt"=w2628:dbl)  [unwired: 5 in, 3 out]
                      n1160 = call "2ndOrderDerivate.vi"("t_capture"=w2627, "initial condition"=w2625, "x"=w2625) -> ("dx/dt"=w2630:dbl)  [unwired: 5 in, 3 out]
                      n1161 = call "2ndOrderDerivate.vi"("t_capture"=w2627, "initial condition"=w2624, "x"=w2624) -> ("dx/dt"=w2629:dbl)  [unwired: 5 in, 3 out]
                    }
                    frame 11 {
                      n1162 = call "2ndOrderDerivate.vi"("t_capture"=w2634, "initial condition"=w2633, "x"=w2633) -> ("dx/dt"=w2635:dbl)  [unwired: 5 in, 3 out]
                      n1163 = call "2ndOrderDerivate.vi"("t_capture"=w2634, "initial condition"=w2632, "x"=w2632) -> ("dx/dt"=w2637:dbl)  [unwired: 5 in, 3 out]
                      n1164 = call "2ndOrderDerivate.vi"("t_capture"=w2634, "initial condition"=w2631, "x"=w2631) -> ("dx/dt"=w2636:dbl)  [unwired: 5 in, 3 out]
                    }
                    frame 12 {
                      n1165 = call "2ndOrderDerivate.vi"("t_capture"=w2641, "initial condition"=w2640, "x"=w2640) -> ("dx/dt"=w2642:dbl)  [unwired: 5 in, 3 out]
                      n1166 = call "2ndOrderDerivate.vi"("t_capture"=w2641, "initial condition"=w2639, "x"=w2639) -> ("dx/dt"=w2644:dbl)  [unwired: 5 in, 3 out]
                      n1167 = call "2ndOrderDerivate.vi"("t_capture"=w2641, "initial condition"=w2638, "x"=w2638) -> ("dx/dt"=w2643:dbl)  [unwired: 5 in, 3 out]
                    }
                    frame 13 {
                      n1168 = call "2ndOrderDerivate.vi"("t_capture"=w2648, "initial condition"=w2647, "x"=w2647) -> ("dx/dt"=w2649:dbl)  [unwired: 5 in, 3 out]
                      n1169 = call "2ndOrderDerivate.vi"("t_capture"=w2648, "initial condition"=w2646, "x"=w2646) -> ("dx/dt"=w2651:dbl)  [unwired: 5 in, 3 out]
                      n1170 = call "2ndOrderDerivate.vi"("t_capture"=w2648, "initial condition"=w2645, "x"=w2645) -> ("dx/dt"=w2650:dbl)  [unwired: 5 in, 3 out]
                    }
                    frame 14 {
                      n1171 = call "2ndOrderDerivate.vi"("t_capture"=w2655, "initial condition"=w2654, "x"=w2654) -> ("dx/dt"=w2656:dbl)  [unwired: 5 in, 3 out]
                      n1172 = call "2ndOrderDerivate.vi"("t_capture"=w2655, "initial condition"=w2653, "x"=w2653) -> ("dx/dt"=w2658:dbl)  [unwired: 5 in, 3 out]
                      n1173 = call "2ndOrderDerivate.vi"("t_capture"=w2655, "initial condition"=w2652, "x"=w2652) -> ("dx/dt"=w2657:dbl)  [unwired: 5 in, 3 out]
                    }
                    frame 15 {
                      n1174 = call "2ndOrderDerivate.vi"("t_capture"=w2662, "initial condition"=w2661, "x"=w2661) -> ("dx/dt"=w2663:dbl)  [unwired: 5 in, 3 out]
                      n1175 = call "2ndOrderDerivate.vi"("t_capture"=w2662, "initial condition"=w2660, "x"=w2660) -> ("dx/dt"=w2665:dbl)  [unwired: 5 in, 3 out]
                      n1176 = call "2ndOrderDerivate.vi"("t_capture"=w2662, "initial condition"=w2659, "x"=w2659) -> ("dx/dt"=w2664:dbl)  [unwired: 5 in, 3 out]
                    }
                  }
                  n1177 = Build Array(w2548, w2544, w2551, w2543, w2550, w2542, w2541, w2540, w2539) -> (w2553:dbl[])
                  n1178 = call-poly <vilib>:"Array To Matrix.vi"("Real 1D Array"=w2553) -> ("Real Matrix (Column Vector)"=w2552:T3)
                  n1179 = Bundle By Name(cluster=w2547, "x_k|k"=w2552) -> (w2549:T2)
                }
              }
              frame True {
              }
            }
            n1180 = Bundle By Name(cluster=w2257, "robots_blue"=w2262, "robots_yellow"=w2261, "balls"=w2253) -> (w2260:T1)
            n1181 = Bundle By Name(cluster=w2257, "New"=FALSE) -> (w2258:T1)
          }
        }
      }
      frame "4thDerivate" {
        n1182 = call "SSL Detection Frame Simple Estimator Kalman VelCmd.vi"("Lado"=w2790, "Time"=w2791, "Enable"=FALSE, "Detection Frame In"=w2781) -> ("Detection Frame Out"=w2780:T1)  [unwired: 6 in, 1 out]
        n1183 = Unbundle By Name(w2780) -> ("robots_blue"=w2789:T2[], "robots_yellow"=w2788:T2[], "camera_id"=w2785:u32, "balls"=w2784:T4[], "t_capture"=w2782:dbl)
        n1184 = case shown="1" w2785 {
          tunnel: w2789 -> [w2806 w3330 w3850 w4370]
          tunnel: 60.0 -> [w2805 w3329 w3849 w4369]
          tunnel: w2788 -> [w2803 w3327 w3847 w4367]
          tunnel: [w2800 w3324 w3844 w4364] -> w2787
          tunnel: [w2798 w3322 w3842 w4362] -> w2786
          tunnel: w2780 -> [w2797 w3321 w3841 w4361]
          tunnel: w2784 -> [w2795 w3319 w3839 w4359]
          tunnel: w2782 -> [w2792 w3316 w3836 w4356]
          frame 3 {
            n1185 = Empty Array?(array=w2795) -> (empty?=w2796:bool)
            n1186 = Empty Array?(array=w2803) -> (empty?=w2804:bool)
            n1187 = Reciprocal(x=w2805) -> (1/x=w2794:dbl)
            n1188 = Empty Array?(array=w2806) -> (empty?=w2807:bool)
            n1189 = case shown="False" w2796 {
              tunnel: w2795 -> [w2810 w2824]
              tunnel: w2794 -> [w2811 _]
              tunnel: [w2809 w2824] -> w2793
              tunnel: w2792 -> [w2808 _]
              frame False {
                n1190 = for {
                  tunnel: w2810 -> [w2823] mode=indexing
                  tunnel: w2811 -> [_]
                  tunnel: w2810 -> [w2822] mode=indexing
                  tunnel: [w2819] -> w2809 mode=indexing
                  tunnel: w2808 -> [w2817]
                  n1191 = Unbundle By Name(w2823) -> ("x"=w2818:sgl, "y"=w2816:sgl, "z"=w2812:sgl)
                  n1192 = call "2ndOrderDerivate.vi"("t_capture"=w2817, "initial condition"=w2816, "x"=w2816) -> ("dx/dt"=w2814:dbl)  [unwired: 5 in, 3 out]
                  n1193 = call "2ndOrderDerivate.vi"("t_capture"=w2817, "initial condition"=w2818, "x"=w2818) -> ("dx/dt"=w2815:dbl)  [unwired: 5 in, 3 out]
                  n1194 = call "2ndOrderDerivate.vi"("t_capture"=w2817, "initial condition"=w2812, "x"=w2812) -> ("dx/dt"=w2813:dbl)  [unwired: 5 in, 3 out]
                  n1195 = Build Array(w2818, w2815, w2816, w2814, w2812, w2813) -> (w2821:dbl[])
                  n1196 = call-poly <vilib>:"Array To Matrix.vi"("Real 1D Array"=w2821) -> ("Real Matrix (Column Vector)"=w2820:T3)
                  n1197 = Bundle By Name(cluster=w2822, "x_k|k"=w2820) -> (w2819:T4)
                }
              }
              frame True {
              }
            }
            n1198 = case shown="False" w2804 {
              tunnel: w2803 -> [w2827 w3071]
              tunnel: w2794 -> [w2828 _]
              tunnel: [w2826 w3071] -> w2801
              tunnel: w2792 -> [w2825 _]
              frame False {
                n1199 = for {
                  tunnel: w2827 -> [w2846] mode=indexing
                  tunnel: w2828 -> [w2838]
                  tunnel: w2827 -> [w2845] mode=indexing
                  tunnel: [w2839] -> w2826 mode=indexing if=w2837
                  tunnel: w2825 -> [w2836]
                  n1200 = Unbundle By Name(w2846) -> ("x"=w2843:sgl, "y"=w2842:sgl, "orientation"=w2844:sgl, "robot_id"=w2829:u32, "Valid"=w2837:bool)
                  n1201 = case shown="1" w2829 {
                    tunnel: w2843 -> [w2965 w2972 w2979 w2986 w2993 w3000 w3007 w3014 w3021 w3028 w3035 w3042 w3049 w3056 w3063 w3070]
                    tunnel: w2842 -> [w2963 w2970 w2977 w2984 w2991 w2998 w3005 w3012 w3019 w3026 w3033 w3040 w3047 w3054 w3061 w3068]
                    tunnel: w2844 -> [w2962 w2969 w2976 w2983 w2990 w2997 w3004 w3011 w3018 w3025 w3032 w3039 w3046 w3053 w3060 w3067]
                    tunnel: [w2961 w2968 w2975 w2982 w2989 w2996 w3003 w3010 w3017 w3024 w3031 w3038 w3045 w3052 w3059 w3066] -> w2835
                    tunnel: [w2960 w2967 w2974 w2981 w2988 w2995 w3002 w3009 w3016 w3023 w3030 w3037 w3044 w3051 w3058 w3065] -> w2834
                    tunnel: [w2959 w2966 w2973 w2980 w2987 w2994 w3001 w3008 w3015 w3022 w3029 w3036 w3043 w3050 w3057 w3064] -> w2833
                    tunnel: w2838 -> [_ _ _ _ _ _ _ _ _ _ _ _ _ _ _ _]
                    tunnel: w2836 -> [w2964 w2971 w2978 w2985 w2992 w2999 w3006 w3013 w3020 w3027 w3034 w3041 w3048 w3055 w3062 w3069]
                    frame 0, Default {
                      n1202 = call "2ndOrderDerivate.vi"("t_capture"=w2964, "initial condition"=w2965, "x"=w2965) -> ("dx/dt"=w2961:dbl)  [unwired: 5 in, 3 out]
                      n1203 = call "2ndOrderDerivate.vi"("t_capture"=w2964, "initial condition"=w2963, "x"=w2963) -> ("dx/dt"=w2960:dbl)  [unwired: 5 in, 3 out]
                      n1204 = call "2ndOrderDerivate.vi"("t_capture"=w2964, "initial condition"=w2962, "x"=w2962) -> ("dx/dt"=w2959:dbl)  [unwired: 5 in, 3 out]
                    }
                    frame 1 {
                      n1205 = call "2ndOrderDerivate.vi"("t_capture"=w2971, "initial condition"=w2972, "x"=w2972) -> ("dx/dt"=w2968:dbl)  [unwired: 5 in, 3 out]
                      n1206 = call "2ndOrderDerivate.vi"("t_capture"=w2971, "initial condition"=w2970, "x"=w2970) -> ("dx/dt"=w2967:dbl)  [unwired: 5 in, 3 out]
                      n1207 = call "2ndOrderDerivate.vi"("t_capture"=w2971, "initial condition"=w2969, "x"=w2969) -> ("dx/dt"=w2966:dbl)  [unwired: 5 in, 3 out]
                    }
                    frame 2 {
                      n1208 = call "2ndOrderDerivate.vi"("t_capture"=w2978, "initial condition"=w2979, "x"=w2979) -> ("dx/dt"=w2975:dbl)  [unwired: 5 in, 3 out]
                      n1209 = call "2ndOrderDerivate.vi"("t_capture"=w2978, "initial condition"=w2977, "x"=w2977) -> ("dx/dt"=w2974:dbl)  [unwired: 5 in, 3 out]
                      n1210 = call "2ndOrderDerivate.vi"("t_capture"=w2978, "initial condition"=w2976, "x"=w2976) -> ("dx/dt"=w2973:dbl)  [unwired: 5 in, 3 out]
                    }
                    frame 3 {
                      n1211 = call "2ndOrderDerivate.vi"("t_capture"=w2985, "initial condition"=w2986, "x"=w2986) -> ("dx/dt"=w2982:dbl)  [unwired: 5 in, 3 out]
                      n1212 = call "2ndOrderDerivate.vi"("t_capture"=w2985, "initial condition"=w2984, "x"=w2984) -> ("dx/dt"=w2981:dbl)  [unwired: 5 in, 3 out]
                      n1213 = call "2ndOrderDerivate.vi"("t_capture"=w2985, "initial condition"=w2983, "x"=w2983) -> ("dx/dt"=w2980:dbl)  [unwired: 5 in, 3 out]
                    }
                    frame 4 {
                      n1214 = call "2ndOrderDerivate.vi"("t_capture"=w2992, "initial condition"=w2993, "x"=w2993) -> ("dx/dt"=w2989:dbl)  [unwired: 5 in, 3 out]
                      n1215 = call "2ndOrderDerivate.vi"("t_capture"=w2992, "initial condition"=w2991, "x"=w2991) -> ("dx/dt"=w2988:dbl)  [unwired: 5 in, 3 out]
                      n1216 = call "2ndOrderDerivate.vi"("t_capture"=w2992, "initial condition"=w2990, "x"=w2990) -> ("dx/dt"=w2987:dbl)  [unwired: 5 in, 3 out]
                    }
                    frame 5 {
                      n1217 = call "2ndOrderDerivate.vi"("t_capture"=w2999, "initial condition"=w3000, "x"=w3000) -> ("dx/dt"=w2996:dbl)  [unwired: 5 in, 3 out]
                      n1218 = call "2ndOrderDerivate.vi"("t_capture"=w2999, "initial condition"=w2998, "x"=w2998) -> ("dx/dt"=w2995:dbl)  [unwired: 5 in, 3 out]
                      n1219 = call "2ndOrderDerivate.vi"("t_capture"=w2999, "initial condition"=w2997, "x"=w2997) -> ("dx/dt"=w2994:dbl)  [unwired: 5 in, 3 out]
                    }
                    frame 6 {
                      n1220 = call "2ndOrderDerivate.vi"("t_capture"=w3006, "initial condition"=w3007, "x"=w3007) -> ("dx/dt"=w3003:dbl)  [unwired: 5 in, 3 out]
                      n1221 = call "2ndOrderDerivate.vi"("t_capture"=w3006, "initial condition"=w3005, "x"=w3005) -> ("dx/dt"=w3002:dbl)  [unwired: 5 in, 3 out]
                      n1222 = call "2ndOrderDerivate.vi"("t_capture"=w3006, "initial condition"=w3004, "x"=w3004) -> ("dx/dt"=w3001:dbl)  [unwired: 5 in, 3 out]
                    }
                    frame 7 {
                      n1223 = call "2ndOrderDerivate.vi"("t_capture"=w3013, "initial condition"=w3014, "x"=w3014) -> ("dx/dt"=w3010:dbl)  [unwired: 5 in, 3 out]
                      n1224 = call "2ndOrderDerivate.vi"("t_capture"=w3013, "initial condition"=w3012, "x"=w3012) -> ("dx/dt"=w3009:dbl)  [unwired: 5 in, 3 out]
                      n1225 = call "2ndOrderDerivate.vi"("t_capture"=w3013, "initial condition"=w3011, "x"=w3011) -> ("dx/dt"=w3008:dbl)  [unwired: 5 in, 3 out]
                    }
                    frame 8 {
                      n1226 = call "2ndOrderDerivate.vi"("t_capture"=w3020, "initial condition"=w3021, "x"=w3021) -> ("dx/dt"=w3017:dbl)  [unwired: 5 in, 3 out]
                      n1227 = call "2ndOrderDerivate.vi"("t_capture"=w3020, "initial condition"=w3019, "x"=w3019) -> ("dx/dt"=w3016:dbl)  [unwired: 5 in, 3 out]
                      n1228 = call "2ndOrderDerivate.vi"("t_capture"=w3020, "initial condition"=w3018, "x"=w3018) -> ("dx/dt"=w3015:dbl)  [unwired: 5 in, 3 out]
                    }
                    frame 9 {
                      n1229 = call "2ndOrderDerivate.vi"("t_capture"=w3027, "initial condition"=w3028, "x"=w3028) -> ("dx/dt"=w3024:dbl)  [unwired: 5 in, 3 out]
                      n1230 = call "2ndOrderDerivate.vi"("t_capture"=w3027, "initial condition"=w3026, "x"=w3026) -> ("dx/dt"=w3023:dbl)  [unwired: 5 in, 3 out]
                      n1231 = call "2ndOrderDerivate.vi"("t_capture"=w3027, "initial condition"=w3025, "x"=w3025) -> ("dx/dt"=w3022:dbl)  [unwired: 5 in, 3 out]
                    }
                    frame 10 {
                      n1232 = call "2ndOrderDerivate.vi"("t_capture"=w3034, "initial condition"=w3035, "x"=w3035) -> ("dx/dt"=w3031:dbl)  [unwired: 5 in, 3 out]
                      n1233 = call "2ndOrderDerivate.vi"("t_capture"=w3034, "initial condition"=w3033, "x"=w3033) -> ("dx/dt"=w3030:dbl)  [unwired: 5 in, 3 out]
                      n1234 = call "2ndOrderDerivate.vi"("t_capture"=w3034, "initial condition"=w3032, "x"=w3032) -> ("dx/dt"=w3029:dbl)  [unwired: 5 in, 3 out]
                    }
                    frame 11 {
                      n1235 = call "2ndOrderDerivate.vi"("t_capture"=w3041, "initial condition"=w3042, "x"=w3042) -> ("dx/dt"=w3038:dbl)  [unwired: 5 in, 3 out]
                      n1236 = call "2ndOrderDerivate.vi"("t_capture"=w3041, "initial condition"=w3040, "x"=w3040) -> ("dx/dt"=w3037:dbl)  [unwired: 5 in, 3 out]
                      n1237 = call "2ndOrderDerivate.vi"("t_capture"=w3041, "initial condition"=w3039, "x"=w3039) -> ("dx/dt"=w3036:dbl)  [unwired: 5 in, 3 out]
                    }
                    frame 12 {
                      n1238 = call "2ndOrderDerivate.vi"("t_capture"=w3048, "initial condition"=w3049, "x"=w3049) -> ("dx/dt"=w3045:dbl)  [unwired: 5 in, 3 out]
                      n1239 = call "2ndOrderDerivate.vi"("t_capture"=w3048, "initial condition"=w3047, "x"=w3047) -> ("dx/dt"=w3044:dbl)  [unwired: 5 in, 3 out]
                      n1240 = call "2ndOrderDerivate.vi"("t_capture"=w3048, "initial condition"=w3046, "x"=w3046) -> ("dx/dt"=w3043:dbl)  [unwired: 5 in, 3 out]
                    }
                    frame 13 {
                      n1241 = call "2ndOrderDerivate.vi"("t_capture"=w3055, "initial condition"=w3056, "x"=w3056) -> ("dx/dt"=w3052:dbl)  [unwired: 5 in, 3 out]
                      n1242 = call "2ndOrderDerivate.vi"("t_capture"=w3055, "initial condition"=w3054, "x"=w3054) -> ("dx/dt"=w3051:dbl)  [unwired: 5 in, 3 out]
                      n1243 = call "2ndOrderDerivate.vi"("t_capture"=w3055, "initial condition"=w3053, "x"=w3053) -> ("dx/dt"=w3050:dbl)  [unwired: 5 in, 3 out]
                    }
                    frame 14 {
                      n1244 = call "2ndOrderDerivate.vi"("t_capture"=w3062, "initial condition"=w3063, "x"=w3063) -> ("dx/dt"=w3059:dbl)  [unwired: 5 in, 3 out]
                      n1245 = call "2ndOrderDerivate.vi"("t_capture"=w3062, "initial condition"=w3061, "x"=w3061) -> ("dx/dt"=w3058:dbl)  [unwired: 5 in, 3 out]
                      n1246 = call "2ndOrderDerivate.vi"("t_capture"=w3062, "initial condition"=w3060, "x"=w3060) -> ("dx/dt"=w3057:dbl)  [unwired: 5 in, 3 out]
                    }
                    frame 15 {
                      n1247 = call "2ndOrderDerivate.vi"("t_capture"=w3069, "initial condition"=w3070, "x"=w3070) -> ("dx/dt"=w3066:dbl)  [unwired: 5 in, 3 out]
                      n1248 = call "2ndOrderDerivate.vi"("t_capture"=w3069, "initial condition"=w3068, "x"=w3068) -> ("dx/dt"=w3065:dbl)  [unwired: 5 in, 3 out]
                      n1249 = call "2ndOrderDerivate.vi"("t_capture"=w3069, "initial condition"=w3067, "x"=w3067) -> ("dx/dt"=w3064:dbl)  [unwired: 5 in, 3 out]
                    }
                  }
                  n1250 = case shown="1" w2829 {
                    tunnel: w2835 -> [w2853 w2860 w2867 w2874 w2881 w2888 w2895 w2902 w2909 w2916 w2923 w2930 w2937 w2944 w2951 w2958]
                    tunnel: w2834 -> [w2851 w2858 w2865 w2872 w2879 w2886 w2893 w2900 w2907 w2914 w2921 w2928 w2935 w2942 w2949 w2956]
                    tunnel: w2833 -> [w2850 w2857 w2864 w2871 w2878 w2885 w2892 w2899 w2906 w2913 w2920 w2927 w2934 w2941 w2948 w2955]
                    tunnel: [w2849 w2856 w2863 w2870 w2877 w2884 w2891 w2898 w2905 w2912 w2919 w2926 w2933 w2940 w2947 w2954] -> w2832
                    tunnel: [w2848 w2855 w2862 w2869 w2876 w2883 w2890 w2897 w2904 w2911 w2918 w2925 w2932 w2939 w2946 w2953] -> w2831
                    tunnel: [w2847 w2854 w2861 w2868 w2875 w2882 w2889 w2896 w2903 w2910 w2917 w2924 w2931 w2938 w2945 w2952] -> w2830
                    tunnel: w2836 -> [w2852 w2859 w2866 w2873 w2880 w2887 w2894 w2901 w2908 w2915 w2922 w2929 w2936 w2943 w2950 w2957]
                    frame 0, Default {
                      n1251 = call "2ndOrderDerivate.vi"("t_capture"=w2852, "initial condition"=w2853, "x"=w2853) -> ("dx/dt"=w2849:dbl)  [unwired: 5 in, 3 out]
                      n1252 = call "2ndOrderDerivate.vi"("t_capture"=w2852, "initial condition"=w2851, "x"=w2851) -> ("dx/dt"=w2848:dbl)  [unwired: 5 in, 3 out]
                      n1253 = call "2ndOrderDerivate.vi"("t_capture"=w2852, "initial condition"=w2850, "x"=w2850) -> ("dx/dt"=w2847:dbl)  [unwired: 5 in, 3 out]
                    }
                    frame 1 {
                      n1254 = call "2ndOrderDerivate.vi"("t_capture"=w2859, "initial condition"=w2860, "x"=w2860) -> ("dx/dt"=w2856:dbl)  [unwired: 5 in, 3 out]
                      n1255 = call "2ndOrderDerivate.vi"("t_capture"=w2859, "initial condition"=w2858, "x"=w2858) -> ("dx/dt"=w2855:dbl)  [unwired: 5 in, 3 out]
                      n1256 = call "2ndOrderDerivate.vi"("t_capture"=w2859, "initial condition"=w2857, "x"=w2857) -> ("dx/dt"=w2854:dbl)  [unwired: 5 in, 3 out]
                    }
                    frame 2 {
                      n1257 = call "2ndOrderDerivate.vi"("t_capture"=w2866, "initial condition"=w2867, "x"=w2867) -> ("dx/dt"=w2863:dbl)  [unwired: 5 in, 3 out]
                      n1258 = call "2ndOrderDerivate.vi"("t_capture"=w2866, "initial condition"=w2865, "x"=w2865) -> ("dx/dt"=w2862:dbl)  [unwired: 5 in, 3 out]
                      n1259 = call "2ndOrderDerivate.vi"("t_capture"=w2866, "initial condition"=w2864, "x"=w2864) -> ("dx/dt"=w2861:dbl)  [unwired: 5 in, 3 out]
                    }
                    frame 3 {
                      n1260 = call "2ndOrderDerivate.vi"("t_capture"=w2873, "initial condition"=w2874, "x"=w2874) -> ("dx/dt"=w2870:dbl)  [unwired: 5 in, 3 out]
                      n1261 = call "2ndOrderDerivate.vi"("t_capture"=w2873, "initial condition"=w2872, "x"=w2872) -> ("dx/dt"=w2869:dbl)  [unwired: 5 in, 3 out]
                      n1262 = call "2ndOrderDerivate.vi"("t_capture"=w2873, "initial condition"=w2871, "x"=w2871) -> ("dx/dt"=w2868:dbl)  [unwired: 5 in, 3 out]
                    }
                    frame 4 {
                      n1263 = call "2ndOrderDerivate.vi"("t_capture"=w2880, "initial condition"=w2881, "x"=w2881) -> ("dx/dt"=w2877:dbl)  [unwired: 5 in, 3 out]
                      n1264 = call "2ndOrderDerivate.vi"("t_capture"=w2880, "initial condition"=w2879, "x"=w2879) -> ("dx/dt"=w2876:dbl)  [unwired: 5 in, 3 out]
                      n1265 = call "2ndOrderDerivate.vi"("t_capture"=w2880, "initial condition"=w2878, "x"=w2878) -> ("dx/dt"=w2875:dbl)  [unwired: 5 in, 3 out]
                    }
                    frame 5 {
                      n1266 = call "2ndOrderDerivate.vi"("t_capture"=w2887, "initial condition"=w2888, "x"=w2888) -> ("dx/dt"=w2884:dbl)  [unwired: 5 in, 3 out]
                      n1267 = call "2ndOrderDerivate.vi"("t_capture"=w2887, "initial condition"=w2886, "x"=w2886) -> ("dx/dt"=w2883:dbl)  [unwired: 5 in, 3 out]
                      n1268 = call "2ndOrderDerivate.vi"("t_capture"=w2887, "initial condition"=w2885, "x"=w2885) -> ("dx/dt"=w2882:dbl)  [unwired: 5 in, 3 out]
                    }
                    frame 6 {
                      n1269 = call "2ndOrderDerivate.vi"("t_capture"=w2894, "initial condition"=w2895, "x"=w2895) -> ("dx/dt"=w2891:dbl)  [unwired: 5 in, 3 out]
                      n1270 = call "2ndOrderDerivate.vi"("t_capture"=w2894, "initial condition"=w2893, "x"=w2893) -> ("dx/dt"=w2890:dbl)  [unwired: 5 in, 3 out]
                      n1271 = call "2ndOrderDerivate.vi"("t_capture"=w2894, "initial condition"=w2892, "x"=w2892) -> ("dx/dt"=w2889:dbl)  [unwired: 5 in, 3 out]
                    }
                    frame 7 {
                      n1272 = call "2ndOrderDerivate.vi"("t_capture"=w2901, "initial condition"=w2902, "x"=w2902) -> ("dx/dt"=w2898:dbl)  [unwired: 5 in, 3 out]
                      n1273 = call "2ndOrderDerivate.vi"("t_capture"=w2901, "initial condition"=w2900, "x"=w2900) -> ("dx/dt"=w2897:dbl)  [unwired: 5 in, 3 out]
                      n1274 = call "2ndOrderDerivate.vi"("t_capture"=w2901, "initial condition"=w2899, "x"=w2899) -> ("dx/dt"=w2896:dbl)  [unwired: 5 in, 3 out]
                    }
                    frame 8 {
                      n1275 = call "2ndOrderDerivate.vi"("t_capture"=w2908, "initial condition"=w2909, "x"=w2909) -> ("dx/dt"=w2905:dbl)  [unwired: 5 in, 3 out]
                      n1276 = call "2ndOrderDerivate.vi"("t_capture"=w2908, "initial condition"=w2907, "x"=w2907) -> ("dx/dt"=w2904:dbl)  [unwired: 5 in, 3 out]
                      n1277 = call "2ndOrderDerivate.vi"("t_capture"=w2908, "initial condition"=w2906, "x"=w2906) -> ("dx/dt"=w2903:dbl)  [unwired: 5 in, 3 out]
                    }
                    frame 9 {
                      n1278 = call "2ndOrderDerivate.vi"("t_capture"=w2915, "initial condition"=w2916, "x"=w2916) -> ("dx/dt"=w2912:dbl)  [unwired: 5 in, 3 out]
                      n1279 = call "2ndOrderDerivate.vi"("t_capture"=w2915, "initial condition"=w2914, "x"=w2914) -> ("dx/dt"=w2911:dbl)  [unwired: 5 in, 3 out]
                      n1280 = call "2ndOrderDerivate.vi"("t_capture"=w2915, "initial condition"=w2913, "x"=w2913) -> ("dx/dt"=w2910:dbl)  [unwired: 5 in, 3 out]
                    }
                    frame 10 {
                      n1281 = call "2ndOrderDerivate.vi"("t_capture"=w2922, "initial condition"=w2923, "x"=w2923) -> ("dx/dt"=w2919:dbl)  [unwired: 5 in, 3 out]
                      n1282 = call "2ndOrderDerivate.vi"("t_capture"=w2922, "initial condition"=w2921, "x"=w2921) -> ("dx/dt"=w2918:dbl)  [unwired: 5 in, 3 out]
                      n1283 = call "2ndOrderDerivate.vi"("t_capture"=w2922, "initial condition"=w2920, "x"=w2920) -> ("dx/dt"=w2917:dbl)  [unwired: 5 in, 3 out]
                    }
                    frame 11 {
                      n1284 = call "2ndOrderDerivate.vi"("t_capture"=w2929, "initial condition"=w2930, "x"=w2930) -> ("dx/dt"=w2926:dbl)  [unwired: 5 in, 3 out]
                      n1285 = call "2ndOrderDerivate.vi"("t_capture"=w2929, "initial condition"=w2928, "x"=w2928) -> ("dx/dt"=w2925:dbl)  [unwired: 5 in, 3 out]
                      n1286 = call "2ndOrderDerivate.vi"("t_capture"=w2929, "initial condition"=w2927, "x"=w2927) -> ("dx/dt"=w2924:dbl)  [unwired: 5 in, 3 out]
                    }
                    frame 12 {
                      n1287 = call "2ndOrderDerivate.vi"("t_capture"=w2936, "initial condition"=w2937, "x"=w2937) -> ("dx/dt"=w2933:dbl)  [unwired: 5 in, 3 out]
                      n1288 = call "2ndOrderDerivate.vi"("t_capture"=w2936, "initial condition"=w2935, "x"=w2935) -> ("dx/dt"=w2932:dbl)  [unwired: 5 in, 3 out]
                      n1289 = call "2ndOrderDerivate.vi"("t_capture"=w2936, "initial condition"=w2934, "x"=w2934) -> ("dx/dt"=w2931:dbl)  [unwired: 5 in, 3 out]
                    }
                    frame 13 {
                      n1290 = call "2ndOrderDerivate.vi"("t_capture"=w2943, "initial condition"=w2944, "x"=w2944) -> ("dx/dt"=w2940:dbl)  [unwired: 5 in, 3 out]
                      n1291 = call "2ndOrderDerivate.vi"("t_capture"=w2943, "initial condition"=w2942, "x"=w2942) -> ("dx/dt"=w2939:dbl)  [unwired: 5 in, 3 out]
                      n1292 = call "2ndOrderDerivate.vi"("t_capture"=w2943, "initial condition"=w2941, "x"=w2941) -> ("dx/dt"=w2938:dbl)  [unwired: 5 in, 3 out]
                    }
                    frame 14 {
                      n1293 = call "2ndOrderDerivate.vi"("t_capture"=w2950, "initial condition"=w2951, "x"=w2951) -> ("dx/dt"=w2947:dbl)  [unwired: 5 in, 3 out]
                      n1294 = call "2ndOrderDerivate.vi"("t_capture"=w2950, "initial condition"=w2949, "x"=w2949) -> ("dx/dt"=w2946:dbl)  [unwired: 5 in, 3 out]
                      n1295 = call "2ndOrderDerivate.vi"("t_capture"=w2950, "initial condition"=w2948, "x"=w2948) -> ("dx/dt"=w2945:dbl)  [unwired: 5 in, 3 out]
                    }
                    frame 15 {
                      n1296 = call "2ndOrderDerivate.vi"("t_capture"=w2957, "initial condition"=w2958, "x"=w2958) -> ("dx/dt"=w2954:dbl)  [unwired: 5 in, 3 out]
                      n1297 = call "2ndOrderDerivate.vi"("t_capture"=w2957, "initial condition"=w2956, "x"=w2956) -> ("dx/dt"=w2953:dbl)  [unwired: 5 in, 3 out]
                      n1298 = call "2ndOrderDerivate.vi"("t_capture"=w2957, "initial condition"=w2955, "x"=w2955) -> ("dx/dt"=w2952:dbl)  [unwired: 5 in, 3 out]
                    }
                  }
                  n1299 = Build Array(w2843, w2835, w2842, w2834, w2844, w2833, w2832, w2831, w2830) -> (w2841:dbl[])
                  n1300 = call-poly <vilib>:"Array To Matrix.vi"("Real 1D Array"=w2841) -> ("Real Matrix (Column Vector)"=w2840:T3)
                  n1301 = Bundle By Name(cluster=w2845, "x_k|k"=w2840) -> (w2839:T2)
                }
              }
              frame True {
              }
            }
            n1302 = case shown="False" w2807 {
              tunnel: w2806 -> [w3074 w3315]
              tunnel: w2794 -> [w3075 _]
              tunnel: [w3073 w3315] -> w2802
              tunnel: w2792 -> [w3072 _]
              frame False {
                n1303 = for {
                  tunnel: w3074 -> [w3084] mode=indexing
                  tunnel: w3075 -> [_]
                  tunnel: [w3086] -> w3073 mode=indexing
                  tunnel: w3072 -> [w3083]
                  n1304 = Unbundle By Name(w3084) -> ("x"=w3085:sgl, "y"=w3088:sgl, "orientation"=w3087:sgl, "robot_id"=w3082:u32)  [unwired: 1 out]
                  n1305 = case shown="0, Default" w3082 {
                    tunnel: w3085 -> [w3205 w3212 w3219 w3226 w3233 w3240 w3247 w3254 w3261 w3268 w3275 w3282 w3289 w3296 w3303 w3310]
                    tunnel: [w3207 w3214 w3221 w3228 w3235 w3242 w3249 w3256 w3263 w3270 w3277 w3284 w3291 w3298 w3305 w3312] -> w3081
                    tunnel: [w3209 w3216 w3223 w3230 w3237 w3244 w3251 w3258 w3265 w3272 w3279 w3286 w3293 w3300 w3307 w3314] -> w3080
                    tunnel: [w3208 w3215 w3222 w3229 w3236 w3243 w3250 w3257 w3264 w3271 w3278 w3285 w3292 w3299 w3306 w3313] -> w3079
                    tunnel: w3088 -> [w3204 w3211 w3218 w3225 w3232 w3239 w3246 w3253 w3260 w3267 w3274 w3281 w3288 w3295 w3302 w3309]
                    tunnel: w3087 -> [w3203 w3210 w3217 w3224 w3231 w3238 w3245 w3252 w3259 w3266 w3273 w3280 w3287 w3294 w3301 w3308]
                    tunnel: w3083 -> [w3206 w3213 w3220 w3227 w3234 w3241 w3248 w3255 w3262 w3269 w3276 w3283 w3290 w3297 w3304 w3311]
                    frame 0, Default {
                      n1306 = call "2ndOrderDerivate.vi"("t_capture"=w3206, "initial condition"=w3205, "x"=w3205) -> ("dx/dt"=w3207:dbl)  [unwired: 5 in, 3 out]
                      n1307 = call "2ndOrderDerivate.vi"("t_capture"=w3206, "initial condition"=w3204, "x"=w3204) -> ("dx/dt"=w3209:dbl)  [unwired: 5 in, 3 out]
                      n1308 = call "2ndOrderDerivate.vi"("t_capture"=w3206, "initial condition"=w3203, "x"=w3203) -> ("dx/dt"=w3208:dbl)  [unwired: 5 in, 3 out]
                    }
                    frame 1 {
                      n1309 = call "2ndOrderDerivate.vi"("t_capture"=w3213, "initial condition"=w3212, "x"=w3212) -> ("dx/dt"=w3214:dbl)  [unwired: 5 in, 3 out]
                      n1310 = call "2ndOrderDerivate.vi"("t_capture"=w3213, "initial condition"=w3211, "x"=w3211) -> ("dx/dt"=w3216:dbl)  [unwired: 5 in, 3 out]
                      n1311 = call "2ndOrderDerivate.vi"("t_capture"=w3213, "initial condition"=w3210, "x"=w3210) -> ("dx/dt"=w3215:dbl)  [unwired: 5 in, 3 out]
                    }
                    frame 2 {
                      n1312 = call "2ndOrderDerivate.vi"("t_capture"=w3220, "initial condition"=w3219, "x"=w3219) -> ("dx/dt"=w3221:dbl)  [unwired: 5 in, 3 out]
                      n1313 = call "2ndOrderDerivate.vi"("t_capture"=w3220, "initial condition"=w3218, "x"=w3218) -> ("dx/dt"=w3223:dbl)  [unwired: 5 in, 3 out]
                      n1314 = call "2ndOrderDerivate.vi"("t_capture"=w3220, "initial condition"=w3217, "x"=w3217) -> ("dx/dt"=w3222:dbl)  [unwired: 5 in, 3 out]
                    }
                    frame 3 {
                      n1315 = call "2ndOrderDerivate.vi"("t_capture"=w3227, "initial condition"=w3226, "x"=w3226) -> ("dx/dt"=w3228:dbl)  [unwired: 5 in, 3 out]
                      n1316 = call "2ndOrderDerivate.vi"("t_capture"=w3227, "initial condition"=w3225, "x"=w3225) -> ("dx/dt"=w3230:dbl)  [unwired: 5 in, 3 out]
                      n1317 = call "2ndOrderDerivate.vi"("t_capture"=w3227, "initial condition"=w3224, "x"=w3224) -> ("dx/dt"=w3229:dbl)  [unwired: 5 in, 3 out]
                    }
                    frame 4 {
                      n1318 = call "2ndOrderDerivate.vi"("t_capture"=w3234, "initial condition"=w3233, "x"=w3233) -> ("dx/dt"=w3235:dbl)  [unwired: 5 in, 3 out]
                      n1319 = call "2ndOrderDerivate.vi"("t_capture"=w3234, "initial condition"=w3232, "x"=w3232) -> ("dx/dt"=w3237:dbl)  [unwired: 5 in, 3 out]
                      n1320 = call "2ndOrderDerivate.vi"("t_capture"=w3234, "initial condition"=w3231, "x"=w3231) -> ("dx/dt"=w3236:dbl)  [unwired: 5 in, 3 out]
                    }
                    frame 5 {
                      n1321 = call "2ndOrderDerivate.vi"("t_capture"=w3241, "initial condition"=w3240, "x"=w3240) -> ("dx/dt"=w3242:dbl)  [unwired: 5 in, 3 out]
                      n1322 = call "2ndOrderDerivate.vi"("t_capture"=w3241, "initial condition"=w3239, "x"=w3239) -> ("dx/dt"=w3244:dbl)  [unwired: 5 in, 3 out]
                      n1323 = call "2ndOrderDerivate.vi"("t_capture"=w3241, "initial condition"=w3238, "x"=w3238) -> ("dx/dt"=w3243:dbl)  [unwired: 5 in, 3 out]
                    }
                    frame 6 {
                      n1324 = call "2ndOrderDerivate.vi"("t_capture"=w3248, "initial condition"=w3247, "x"=w3247) -> ("dx/dt"=w3249:dbl)  [unwired: 5 in, 3 out]
                      n1325 = call "2ndOrderDerivate.vi"("t_capture"=w3248, "initial condition"=w3246, "x"=w3246) -> ("dx/dt"=w3251:dbl)  [unwired: 5 in, 3 out]
                      n1326 = call "2ndOrderDerivate.vi"("t_capture"=w3248, "initial condition"=w3245, "x"=w3245) -> ("dx/dt"=w3250:dbl)  [unwired: 5 in, 3 out]
                    }
                    frame 7 {
                      n1327 = call "2ndOrderDerivate.vi"("t_capture"=w3255, "initial condition"=w3254, "x"=w3254) -> ("dx/dt"=w3256:dbl)  [unwired: 5 in, 3 out]
                      n1328 = call "2ndOrderDerivate.vi"("t_capture"=w3255, "initial condition"=w3253, "x"=w3253) -> ("dx/dt"=w3258:dbl)  [unwired: 5 in, 3 out]
                      n1329 = call "2ndOrderDerivate.vi"("t_capture"=w3255, "initial condition"=w3252, "x"=w3252) -> ("dx/dt"=w3257:dbl)  [unwired: 5 in, 3 out]
                    }
                    frame 8 {
                      n1330 = call "2ndOrderDerivate.vi"("t_capture"=w3262, "initial condition"=w3261, "x"=w3261) -> ("dx/dt"=w3263:dbl)  [unwired: 5 in, 3 out]
                      n1331 = call "2ndOrderDerivate.vi"("t_capture"=w3262, "initial condition"=w3260, "x"=w3260) -> ("dx/dt"=w3265:dbl)  [unwired: 5 in, 3 out]
                      n1332 = call "2ndOrderDerivate.vi"("t_capture"=w3262, "initial condition"=w3259, "x"=w3259) -> ("dx/dt"=w3264:dbl)  [unwired: 5 in, 3 out]
                    }
                    frame 9 {
                      n1333 = call "2ndOrderDerivate.vi"("t_capture"=w3269, "initial condition"=w3268, "x"=w3268) -> ("dx/dt"=w3270:dbl)  [unwired: 5 in, 3 out]
                      n1334 = call "2ndOrderDerivate.vi"("t_capture"=w3269, "initial condition"=w3267, "x"=w3267) -> ("dx/dt"=w3272:dbl)  [unwired: 5 in, 3 out]
                      n1335 = call "2ndOrderDerivate.vi"("t_capture"=w3269, "initial condition"=w3266, "x"=w3266) -> ("dx/dt"=w3271:dbl)  [unwired: 5 in, 3 out]
                    }
                    frame 10 {
                      n1336 = call "2ndOrderDerivate.vi"("t_capture"=w3276, "initial condition"=w3275, "x"=w3275) -> ("dx/dt"=w3277:dbl)  [unwired: 5 in, 3 out]
                      n1337 = call "2ndOrderDerivate.vi"("t_capture"=w3276, "initial condition"=w3274, "x"=w3274) -> ("dx/dt"=w3279:dbl)  [unwired: 5 in, 3 out]
                      n1338 = call "2ndOrderDerivate.vi"("t_capture"=w3276, "initial condition"=w3273, "x"=w3273) -> ("dx/dt"=w3278:dbl)  [unwired: 5 in, 3 out]
                    }
                    frame 11 {
                      n1339 = call "2ndOrderDerivate.vi"("t_capture"=w3283, "initial condition"=w3282, "x"=w3282) -> ("dx/dt"=w3284:dbl)  [unwired: 5 in, 3 out]
                      n1340 = call "2ndOrderDerivate.vi"("t_capture"=w3283, "initial condition"=w3281, "x"=w3281) -> ("dx/dt"=w3286:dbl)  [unwired: 5 in, 3 out]
                      n1341 = call "2ndOrderDerivate.vi"("t_capture"=w3283, "initial condition"=w3280, "x"=w3280) -> ("dx/dt"=w3285:dbl)  [unwired: 5 in, 3 out]
                    }
                    frame 12 {
                      n1342 = call "2ndOrderDerivate.vi"("t_capture"=w3290, "initial condition"=w3289, "x"=w3289) -> ("dx/dt"=w3291:dbl)  [unwired: 5 in, 3 out]
                      n1343 = call "2ndOrderDerivate.vi"("t_capture"=w3290, "initial condition"=w3288, "x"=w3288) -> ("dx/dt"=w3293:dbl)  [unwired: 5 in, 3 out]
                      n1344 = call "2ndOrderDerivate.vi"("t_capture"=w3290, "initial condition"=w3287, "x"=w3287) -> ("dx/dt"=w3292:dbl)  [unwired: 5 in, 3 out]
                    }
                    frame 13 {
                      n1345 = call "2ndOrderDerivate.vi"("t_capture"=w3297, "initial condition"=w3296, "x"=w3296) -> ("dx/dt"=w3298:dbl)  [unwired: 5 in, 3 out]
                      n1346 = call "2ndOrderDerivate.vi"("t_capture"=w3297, "initial condition"=w3295, "x"=w3295) -> ("dx/dt"=w3300:dbl)  [unwired: 5 in, 3 out]
                      n1347 = call "2ndOrderDerivate.vi"("t_capture"=w3297, "initial condition"=w3294, "x"=w3294) -> ("dx/dt"=w3299:dbl)  [unwired: 5 in, 3 out]
                    }
                    frame 14 {
                      n1348 = call "2ndOrderDerivate.vi"("t_capture"=w3304, "initial condition"=w3303, "x"=w3303) -> ("dx/dt"=w3305:dbl)  [unwired: 5 in, 3 out]
                      n1349 = call "2ndOrderDerivate.vi"("t_capture"=w3304, "initial condition"=w3302, "x"=w3302) -> ("dx/dt"=w3307:dbl)  [unwired: 5 in, 3 out]
                      n1350 = call "2ndOrderDerivate.vi"("t_capture"=w3304, "initial condition"=w3301, "x"=w3301) -> ("dx/dt"=w3306:dbl)  [unwired: 5 in, 3 out]
                    }
                    frame 15 {
                      n1351 = call "2ndOrderDerivate.vi"("t_capture"=w3311, "initial condition"=w3310, "x"=w3310) -> ("dx/dt"=w3312:dbl)  [unwired: 5 in, 3 out]
                      n1352 = call "2ndOrderDerivate.vi"("t_capture"=w3311, "initial condition"=w3309, "x"=w3309) -> ("dx/dt"=w3314:dbl)  [unwired: 5 in, 3 out]
                      n1353 = call "2ndOrderDerivate.vi"("t_capture"=w3311, "initial condition"=w3308, "x"=w3308) -> ("dx/dt"=w3313:dbl)  [unwired: 5 in, 3 out]
                    }
                  }
                  n1354 = case shown="0, Default" w3082 {
                    tunnel: w3081 -> [w3093 w3100 w3107 w3114 w3121 w3128 w3135 w3142 w3149 w3156 w3163 w3170 w3177 w3184 w3191 w3198]
                    tunnel: [w3095 w3102 w3109 w3116 w3123 w3130 w3137 w3144 w3151 w3158 w3165 w3172 w3179 w3186 w3193 w3200] -> w3078
                    tunnel: [w3097 w3104 w3111 w3118 w3125 w3132 w3139 w3146 w3153 w3160 w3167 w3174 w3181 w3188 w3195 w3202] -> w3077
                    tunnel: [w3096 w3103 w3110 w3117 w3124 w3131 w3138 w3145 w3152 w3159 w3166 w3173 w3180 w3187 w3194 w3201] -> w3076
                    tunnel: w3080 -> [w3092 w3099 w3106 w3113 w3120 w3127 w3134 w3141 w3148 w3155 w3162 w3169 w3176 w3183 w3190 w3197]
                    tunnel: w3079 -> [w3091 w3098 w3105 w3112 w3119 w3126 w3133 w3140 w3147 w3154 w3161 w3168 w3175 w3182 w3189 w3196]
                    tunnel: w3083 -> [w3094 w3101 w3108 w3115 w3122 w3129 w3136 w3143 w3150 w3157 w3164 w3171 w3178 w3185 w3192 w3199]
                    frame 0, Default {
                      n1355 = call "2ndOrderDerivate.vi"("t_capture"=w3094, "initial condition"=w3093, "x"=w3093) -> ("dx/dt"=w3095:dbl)  [unwired: 5 in, 3 out]
                      n1356 = call "2ndOrderDerivate.vi"("t_capture"=w3094, "initial condition"=w3092, "x"=w3092) -> ("dx/dt"=w3097:dbl)  [unwired: 5 in, 3 out]
                      n1357 = call "2ndOrderDerivate.vi"("t_capture"=w3094, "initial condition"=w3091, "x"=w3091) -> ("dx/dt"=w3096:dbl)  [unwired: 5 in, 3 out]
                    }
                    frame 1 {
                      n1358 = call "2ndOrderDerivate.vi"("t_capture"=w3101, "initial condition"=w3100, "x"=w3100) -> ("dx/dt"=w3102:dbl)  [unwired: 5 in, 3 out]
                      n1359 = call "2ndOrderDerivate.vi"("t_capture"=w3101, "initial condition"=w3099, "x"=w3099) -> ("dx/dt"=w3104:dbl)  [unwired: 5 in, 3 out]
                      n1360 = call "2ndOrderDerivate.vi"("t_capture"=w3101, "initial condition"=w3098, "x"=w3098) -> ("dx/dt"=w3103:dbl)  [unwired: 5 in, 3 out]
                    }
                    frame 2 {
                      n1361 = call "2ndOrderDerivate.vi"("t_capture"=w3108, "initial condition"=w3107, "x"=w3107) -> ("dx/dt"=w3109:dbl)  [unwired: 5 in, 3 out]
                      n1362 = call "2ndOrderDerivate.vi"("t_capture"=w3108, "initial condition"=w3106, "x"=w3106) -> ("dx/dt"=w3111:dbl)  [unwired: 5 in, 3 out]
                      n1363 = call "2ndOrderDerivate.vi"("t_capture"=w3108, "initial condition"=w3105, "x"=w3105) -> ("dx/dt"=w3110:dbl)  [unwired: 5 in, 3 out]
                    }
                    frame 3 {
                      n1364 = call "2ndOrderDerivate.vi"("t_capture"=w3115, "initial condition"=w3114, "x"=w3114) -> ("dx/dt"=w3116:dbl)  [unwired: 5 in, 3 out]
                      n1365 = call "2ndOrderDerivate.vi"("t_capture"=w3115, "initial condition"=w3113, "x"=w3113) -> ("dx/dt"=w3118:dbl)  [unwired: 5 in, 3 out]
                      n1366 = call "2ndOrderDerivate.vi"("t_capture"=w3115, "initial condition"=w3112, "x"=w3112) -> ("dx/dt"=w3117:dbl)  [unwired: 5 in, 3 out]
                    }
                    frame 4 {
                      n1367 = call "2ndOrderDerivate.vi"("t_capture"=w3122, "initial condition"=w3121, "x"=w3121) -> ("dx/dt"=w3123:dbl)  [unwired: 5 in, 3 out]
                      n1368 = call "2ndOrderDerivate.vi"("t_capture"=w3122, "initial condition"=w3120, "x"=w3120) -> ("dx/dt"=w3125:dbl)  [unwired: 5 in, 3 out]
                      n1369 = call "2ndOrderDerivate.vi"("t_capture"=w3122, "initial condition"=w3119, "x"=w3119) -> ("dx/dt"=w3124:dbl)  [unwired: 5 in, 3 out]
                    }
                    frame 5 {
                      n1370 = call "2ndOrderDerivate.vi"("t_capture"=w3129, "initial condition"=w3128, "x"=w3128) -> ("dx/dt"=w3130:dbl)  [unwired: 5 in, 3 out]
                      n1371 = call "2ndOrderDerivate.vi"("t_capture"=w3129, "initial condition"=w3127, "x"=w3127) -> ("dx/dt"=w3132:dbl)  [unwired: 5 in, 3 out]
                      n1372 = call "2ndOrderDerivate.vi"("t_capture"=w3129, "initial condition"=w3126, "x"=w3126) -> ("dx/dt"=w3131:dbl)  [unwired: 5 in, 3 out]
                    }
                    frame 6 {
                      n1373 = call "2ndOrderDerivate.vi"("t_capture"=w3136, "initial condition"=w3135, "x"=w3135) -> ("dx/dt"=w3137:dbl)  [unwired: 5 in, 3 out]
                      n1374 = call "2ndOrderDerivate.vi"("t_capture"=w3136, "initial condition"=w3134, "x"=w3134) -> ("dx/dt"=w3139:dbl)  [unwired: 5 in, 3 out]
                      n1375 = call "2ndOrderDerivate.vi"("t_capture"=w3136, "initial condition"=w3133, "x"=w3133) -> ("dx/dt"=w3138:dbl)  [unwired: 5 in, 3 out]
                    }
                    frame 7 {
                      n1376 = call "2ndOrderDerivate.vi"("t_capture"=w3143, "initial condition"=w3142, "x"=w3142) -> ("dx/dt"=w3144:dbl)  [unwired: 5 in, 3 out]
                      n1377 = call "2ndOrderDerivate.vi"("t_capture"=w3143, "initial condition"=w3141, "x"=w3141) -> ("dx/dt"=w3146:dbl)  [unwired: 5 in, 3 out]
                      n1378 = call "2ndOrderDerivate.vi"("t_capture"=w3143, "initial condition"=w3140, "x"=w3140) -> ("dx/dt"=w3145:dbl)  [unwired: 5 in, 3 out]
                    }
                    frame 8 {
                      n1379 = call "2ndOrderDerivate.vi"("t_capture"=w3150, "initial condition"=w3149, "x"=w3149) -> ("dx/dt"=w3151:dbl)  [unwired: 5 in, 3 out]
                      n1380 = call "2ndOrderDerivate.vi"("t_capture"=w3150, "initial condition"=w3148, "x"=w3148) -> ("dx/dt"=w3153:dbl)  [unwired: 5 in, 3 out]
                      n1381 = call "2ndOrderDerivate.vi"("t_capture"=w3150, "initial condition"=w3147, "x"=w3147) -> ("dx/dt"=w3152:dbl)  [unwired: 5 in, 3 out]
                    }
                    frame 9 {
                      n1382 = call "2ndOrderDerivate.vi"("t_capture"=w3157, "initial condition"=w3156, "x"=w3156) -> ("dx/dt"=w3158:dbl)  [unwired: 5 in, 3 out]
                      n1383 = call "2ndOrderDerivate.vi"("t_capture"=w3157, "initial condition"=w3155, "x"=w3155) -> ("dx/dt"=w3160:dbl)  [unwired: 5 in, 3 out]
                      n1384 = call "2ndOrderDerivate.vi"("t_capture"=w3157, "initial condition"=w3154, "x"=w3154) -> ("dx/dt"=w3159:dbl)  [unwired: 5 in, 3 out]
                    }
                    frame 10 {
                      n1385 = call "2ndOrderDerivate.vi"("t_capture"=w3164, "initial condition"=w3163, "x"=w3163) -> ("dx/dt"=w3165:dbl)  [unwired: 5 in, 3 out]
                      n1386 = call "2ndOrderDerivate.vi"("t_capture"=w3164, "initial condition"=w3162, "x"=w3162) -> ("dx/dt"=w3167:dbl)  [unwired: 5 in, 3 out]
                      n1387 = call "2ndOrderDerivate.vi"("t_capture"=w3164, "initial condition"=w3161, "x"=w3161) -> ("dx/dt"=w3166:dbl)  [unwired: 5 in, 3 out]
                    }
                    frame 11 {
                      n1388 = call "2ndOrderDerivate.vi"("t_capture"=w3171, "initial condition"=w3170, "x"=w3170) -> ("dx/dt"=w3172:dbl)  [unwired: 5 in, 3 out]
                      n1389 = call "2ndOrderDerivate.vi"("t_capture"=w3171, "initial condition"=w3169, "x"=w3169) -> ("dx/dt"=w3174:dbl)  [unwired: 5 in, 3 out]
                      n1390 = call "2ndOrderDerivate.vi"("t_capture"=w3171, "initial condition"=w3168, "x"=w3168) -> ("dx/dt"=w3173:dbl)  [unwired: 5 in, 3 out]
                    }
                    frame 12 {
                      n1391 = call "2ndOrderDerivate.vi"("t_capture"=w3178, "initial condition"=w3177, "x"=w3177) -> ("dx/dt"=w3179:dbl)  [unwired: 5 in, 3 out]
                      n1392 = call "2ndOrderDerivate.vi"("t_capture"=w3178, "initial condition"=w3176, "x"=w3176) -> ("dx/dt"=w3181:dbl)  [unwired: 5 in, 3 out]
                      n1393 = call "2ndOrderDerivate.vi"("t_capture"=w3178, "initial condition"=w3175, "x"=w3175) -> ("dx/dt"=w3180:dbl)  [unwired: 5 in, 3 out]
                    }
                    frame 13 {
                      n1394 = call "2ndOrderDerivate.vi"("t_capture"=w3185, "initial condition"=w3184, "x"=w3184) -> ("dx/dt"=w3186:dbl)  [unwired: 5 in, 3 out]
                      n1395 = call "2ndOrderDerivate.vi"("t_capture"=w3185, "initial condition"=w3183, "x"=w3183) -> ("dx/dt"=w3188:dbl)  [unwired: 5 in, 3 out]
                      n1396 = call "2ndOrderDerivate.vi"("t_capture"=w3185, "initial condition"=w3182, "x"=w3182) -> ("dx/dt"=w3187:dbl)  [unwired: 5 in, 3 out]
                    }
                    frame 14 {
                      n1397 = call "2ndOrderDerivate.vi"("t_capture"=w3192, "initial condition"=w3191, "x"=w3191) -> ("dx/dt"=w3193:dbl)  [unwired: 5 in, 3 out]
                      n1398 = call "2ndOrderDerivate.vi"("t_capture"=w3192, "initial condition"=w3190, "x"=w3190) -> ("dx/dt"=w3195:dbl)  [unwired: 5 in, 3 out]
                      n1399 = call "2ndOrderDerivate.vi"("t_capture"=w3192, "initial condition"=w3189, "x"=w3189) -> ("dx/dt"=w3194:dbl)  [unwired: 5 in, 3 out]
                    }
                    frame 15 {
                      n1400 = call "2ndOrderDerivate.vi"("t_capture"=w3199, "initial condition"=w3198, "x"=w3198) -> ("dx/dt"=w3200:dbl)  [unwired: 5 in, 3 out]
                      n1401 = call "2ndOrderDerivate.vi"("t_capture"=w3199, "initial condition"=w3197, "x"=w3197) -> ("dx/dt"=w3202:dbl)  [unwired: 5 in, 3 out]
                      n1402 = call "2ndOrderDerivate.vi"("t_capture"=w3199, "initial condition"=w3196, "x"=w3196) -> ("dx/dt"=w3201:dbl)  [unwired: 5 in, 3 out]
                    }
                  }
                  n1403 = Build Array(w3085, w3081, w3088, w3080, w3087, w3079, w3078, w3077, w3076) -> (w3090:dbl[])
                  n1404 = call-poly <vilib>:"Array To Matrix.vi"("Real 1D Array"=w3090) -> ("Real Matrix (Column Vector)"=w3089:T3)
                  n1405 = Bundle By Name(cluster=w3084, "x_k|k"=w3089) -> (w3086:T2)
                }
              }
              frame True {
              }
            }
            n1406 = Bundle By Name(cluster=w2797, "robots_blue"=w2802, "robots_yellow"=w2801, "balls"=w2793) -> (w2800:T1)
            n1407 = Bundle By Name(cluster=w2797, "New"=FALSE) -> (w2798:T1)
          }
          frame 0, Default {
            n1408 = Empty Array?(array=w3319) -> (empty?=w3320:bool)
            n1409 = Empty Array?(array=w3327) -> (empty?=w3328:bool)
            n1410 = Reciprocal(x=w3329) -> (1/x=w3318:dbl)
            n1411 = Empty Array?(array=w3330) -> (empty?=w3331:bool)
            n1412 = case shown="False" w3320 {
              tunnel: w3319 -> [w3334 w3348]
              tunnel: w3318 -> [w3335 _]
              tunnel: [w3333 w3348] -> w3317
              tunnel: w3316 -> [w3332 _]
              frame False {
                n1413 = for {
                  tunnel: w3334 -> [w3347] mode=indexing
                  tunnel: w3335 -> [_]
                  tunnel: w3334 -> [w3346] mode=indexing
                  tunnel: [w3343] -> w3333 mode=indexing
                  tunnel: w3332 -> [w3341]
                  n1414 = Unbundle By Name(w3347) -> ("x"=w3342:sgl, "y"=w3340:sgl, "z"=w3336:sgl)
                  n1415 = call "2ndOrderDerivate.vi"("t_capture"=w3341, "initial condition"=w3340, "x"=w3340) -> ("dx/dt"=w3338:dbl)  [unwired: 5 in, 3 out]
                  n1416 = call "2ndOrderDerivate.vi"("t_capture"=w3341, "initial condition"=w3342, "x"=w3342) -> ("dx/dt"=w3339:dbl)  [unwired: 5 in, 3 out]
                  n1417 = call "2ndOrderDerivate.vi"("t_capture"=w3341, "initial condition"=w3336, "x"=w3336) -> ("dx/dt"=w3337:dbl)  [unwired: 5 in, 3 out]
                  n1418 = Build Array(w3342, w3339, w3340, w3338, w3336, w3337) -> (w3345:dbl[])
                  n1419 = call-poly <vilib>:"Array To Matrix.vi"("Real 1D Array"=w3345) -> ("Real Matrix (Column Vector)"=w3344:T3)
                  n1420 = Bundle By Name(cluster=w3346, "x_k|k"=w3344) -> (w3343:T4)
                }
              }
              frame True {
              }
            }
            n1421 = case shown="False" w3328 {
              tunnel: w3327 -> [w3350 w3591]
              tunnel: w3318 -> [_ _]
              tunnel: [w3351 w3591] -> w3325
              tunnel: w3316 -> [w3349 _]
              frame False {
                n1422 = for {
                  tunnel: w3350 -> [w3360] mode=indexing
                  tunnel: [w3362] -> w3351 mode=indexing
                  tunnel: w3349 -> [w3359]
                  n1423 = Unbundle By Name(w3360) -> ("x"=w3361:sgl, "y"=w3364:sgl, "orientation"=w3363:sgl, "robot_id"=w3358:u32)  [unwired: 1 out]
                  n1424 = case shown="0, Default" w3358 {
                    tunnel: w3361 -> [w3481 w3488 w3495 w3502 w3509 w3516 w3523 w3530 w3537 w3544 w3551 w3558 w3565 w3572 w3579 w3586]
                    tunnel: [w3483 w3490 w3497 w3504 w3511 w3518 w3525 w3532 w3539 w3546 w3553 w3560 w3567 w3574 w3581 w3588] -> w3357
                    tunnel: [w3485 w3492 w3499 w3506 w3513 w3520 w3527 w3534 w3541 w3548 w3555 w3562 w3569 w3576 w3583 w3590] -> w3356
                    tunnel: [w3484 w3491 w3498 w3505 w3512 w3519 w3526 w3533 w3540 w3547 w3554 w3561 w3568 w3575 w3582 w3589] -> w3355
                    tunnel: w3364 -> [w3480 w3487 w3494 w3501 w3508 w3515 w3522 w3529 w3536 w3543 w3550 w3557 w3564 w3571 w3578 w3585]
                    tunnel: w3363 -> [w3479 w3486 w3493 w3500 w3507 w3514 w3521 w3528 w3535 w3542 w3549 w3556 w3563 w3570 w3577 w3584]
                    tunnel: w3359 -> [w3482 w3489 w3496 w3503 w3510 w3517 w3524 w3531 w3538 w3545 w3552 w3559 w3566 w3573 w3580 w3587]
                    frame 0, Default {
                      n1425 = call "2ndOrderDerivate.vi"("t_capture"=w3482, "initial condition"=w3481, "x"=w3481) -> ("dx/dt"=w3483:dbl)  [unwired: 5 in, 3 out]
                      n1426 = call "2ndOrderDerivate.vi"("t_capture"=w3482, "initial condition"=w3480, "x"=w3480) -> ("dx/dt"=w3485:dbl)  [unwired: 5 in, 3 out]
                      n1427 = call "2ndOrderDerivate.vi"("t_capture"=w3482, "initial condition"=w3479, "x"=w3479) -> ("dx/dt"=w3484:dbl)  [unwired: 5 in, 3 out]
                    }
                    frame 1 {
                      n1428 = call "2ndOrderDerivate.vi"("t_capture"=w3489, "initial condition"=w3488, "x"=w3488) -> ("dx/dt"=w3490:dbl)  [unwired: 5 in, 3 out]
                      n1429 = call "2ndOrderDerivate.vi"("t_capture"=w3489, "initial condition"=w3487, "x"=w3487) -> ("dx/dt"=w3492:dbl)  [unwired: 5 in, 3 out]
                      n1430 = call "2ndOrderDerivate.vi"("t_capture"=w3489, "initial condition"=w3486, "x"=w3486) -> ("dx/dt"=w3491:dbl)  [unwired: 5 in, 3 out]
                    }
                    frame 2 {
                      n1431 = call "2ndOrderDerivate.vi"("t_capture"=w3496, "initial condition"=w3495, "x"=w3495) -> ("dx/dt"=w3497:dbl)  [unwired: 5 in, 3 out]
                      n1432 = call "2ndOrderDerivate.vi"("t_capture"=w3496, "initial condition"=w3494, "x"=w3494) -> ("dx/dt"=w3499:dbl)  [unwired: 5 in, 3 out]
                      n1433 = call "2ndOrderDerivate.vi"("t_capture"=w3496, "initial condition"=w3493, "x"=w3493) -> ("dx/dt"=w3498:dbl)  [unwired: 5 in, 3 out]
                    }
                    frame 3 {
                      n1434 = call "2ndOrderDerivate.vi"("t_capture"=w3503, "initial condition"=w3502, "x"=w3502) -> ("dx/dt"=w3504:dbl)  [unwired: 5 in, 3 out]
                      n1435 = call "2ndOrderDerivate.vi"("t_capture"=w3503, "initial condition"=w3501, "x"=w3501) -> ("dx/dt"=w3506:dbl)  [unwired: 5 in, 3 out]
                      n1436 = call "2ndOrderDerivate.vi"("t_capture"=w3503, "initial condition"=w3500, "x"=w3500) -> ("dx/dt"=w3505:dbl)  [unwired: 5 in, 3 out]
                    }
                    frame 4 {
                      n1437 = call "2ndOrderDerivate.vi"("t_capture"=w3510, "initial condition"=w3509, "x"=w3509) -> ("dx/dt"=w3511:dbl)  [unwired: 5 in, 3 out]
                      n1438 = call "2ndOrderDerivate.vi"("t_capture"=w3510, "initial condition"=w3508, "x"=w3508) -> ("dx/dt"=w3513:dbl)  [unwired: 5 in, 3 out]
                      n1439 = call "2ndOrderDerivate.vi"("t_capture"=w3510, "initial condition"=w3507, "x"=w3507) -> ("dx/dt"=w3512:dbl)  [unwired: 5 in, 3 out]
                    }
                    frame 5 {
                      n1440 = call "2ndOrderDerivate.vi"("t_capture"=w3517, "initial condition"=w3516, "x"=w3516) -> ("dx/dt"=w3518:dbl)  [unwired: 5 in, 3 out]
                      n1441 = call "2ndOrderDerivate.vi"("t_capture"=w3517, "initial condition"=w3515, "x"=w3515) -> ("dx/dt"=w3520:dbl)  [unwired: 5 in, 3 out]
                      n1442 = call "2ndOrderDerivate.vi"("t_capture"=w3517, "initial condition"=w3514, "x"=w3514) -> ("dx/dt"=w3519:dbl)  [unwired: 5 in, 3 out]
                    }
                    frame 6 {
                      n1443 = call "2ndOrderDerivate.vi"("t_capture"=w3524, "initial condition"=w3523, "x"=w3523) -> ("dx/dt"=w3525:dbl)  [unwired: 5 in, 3 out]
                      n1444 = call "2ndOrderDerivate.vi"("t_capture"=w3524, "initial condition"=w3522, "x"=w3522) -> ("dx/dt"=w3527:dbl)  [unwired: 5 in, 3 out]
                      n1445 = call "2ndOrderDerivate.vi"("t_capture"=w3524, "initial condition"=w3521, "x"=w3521) -> ("dx/dt"=w3526:dbl)  [unwired: 5 in, 3 out]
                    }
                    frame 7 {
                      n1446 = call "2ndOrderDerivate.vi"("t_capture"=w3531, "initial condition"=w3530, "x"=w3530) -> ("dx/dt"=w3532:dbl)  [unwired: 5 in, 3 out]
                      n1447 = call "2ndOrderDerivate.vi"("t_capture"=w3531, "initial condition"=w3529, "x"=w3529) -> ("dx/dt"=w3534:dbl)  [unwired: 5 in, 3 out]
                      n1448 = call "2ndOrderDerivate.vi"("t_capture"=w3531, "initial condition"=w3528, "x"=w3528) -> ("dx/dt"=w3533:dbl)  [unwired: 5 in, 3 out]
                    }
                    frame 8 {
                      n1449 = call "2ndOrderDerivate.vi"("t_capture"=w3538, "initial condition"=w3537, "x"=w3537) -> ("dx/dt"=w3539:dbl)  [unwired: 5 in, 3 out]
                      n1450 = call "2ndOrderDerivate.vi"("t_capture"=w3538, "initial condition"=w3536, "x"=w3536) -> ("dx/dt"=w3541:dbl)  [unwired: 5 in, 3 out]
                      n1451 = call "2ndOrderDerivate.vi"("t_capture"=w3538, "initial condition"=w3535, "x"=w3535) -> ("dx/dt"=w3540:dbl)  [unwired: 5 in, 3 out]
                    }
                    frame 9 {
                      n1452 = call "2ndOrderDerivate.vi"("t_capture"=w3545, "initial condition"=w3544, "x"=w3544) -> ("dx/dt"=w3546:dbl)  [unwired: 5 in, 3 out]
                      n1453 = call "2ndOrderDerivate.vi"("t_capture"=w3545, "initial condition"=w3543, "x"=w3543) -> ("dx/dt"=w3548:dbl)  [unwired: 5 in, 3 out]
                      n1454 = call "2ndOrderDerivate.vi"("t_capture"=w3545, "initial condition"=w3542, "x"=w3542) -> ("dx/dt"=w3547:dbl)  [unwired: 5 in, 3 out]
                    }
                    frame 10 {
                      n1455 = call "2ndOrderDerivate.vi"("t_capture"=w3552, "initial condition"=w3551, "x"=w3551) -> ("dx/dt"=w3553:dbl)  [unwired: 5 in, 3 out]
                      n1456 = call "2ndOrderDerivate.vi"("t_capture"=w3552, "initial condition"=w3550, "x"=w3550) -> ("dx/dt"=w3555:dbl)  [unwired: 5 in, 3 out]
                      n1457 = call "2ndOrderDerivate.vi"("t_capture"=w3552, "initial condition"=w3549, "x"=w3549) -> ("dx/dt"=w3554:dbl)  [unwired: 5 in, 3 out]
                    }
                    frame 11 {
                      n1458 = call "2ndOrderDerivate.vi"("t_capture"=w3559, "initial condition"=w3558, "x"=w3558) -> ("dx/dt"=w3560:dbl)  [unwired: 5 in, 3 out]
                      n1459 = call "2ndOrderDerivate.vi"("t_capture"=w3559, "initial condition"=w3557, "x"=w3557) -> ("dx/dt"=w3562:dbl)  [unwired: 5 in, 3 out]
                      n1460 = call "2ndOrderDerivate.vi"("t_capture"=w3559, "initial condition"=w3556, "x"=w3556) -> ("dx/dt"=w3561:dbl)  [unwired: 5 in, 3 out]
                    }
                    frame 12 {
                      n1461 = call "2ndOrderDerivate.vi"("t_capture"=w3566, "initial condition"=w3565, "x"=w3565) -> ("dx/dt"=w3567:dbl)  [unwired: 5 in, 3 out]
                      n1462 = call "2ndOrderDerivate.vi"("t_capture"=w3566, "initial condition"=w3564, "x"=w3564) -> ("dx/dt"=w3569:dbl)  [unwired: 5 in, 3 out]
                      n1463 = call "2ndOrderDerivate.vi"("t_capture"=w3566, "initial condition"=w3563, "x"=w3563) -> ("dx/dt"=w3568:dbl)  [unwired: 5 in, 3 out]
                    }
                    frame 13 {
                      n1464 = call "2ndOrderDerivate.vi"("t_capture"=w3573, "initial condition"=w3572, "x"=w3572) -> ("dx/dt"=w3574:dbl)  [unwired: 5 in, 3 out]
                      n1465 = call "2ndOrderDerivate.vi"("t_capture"=w3573, "initial condition"=w3571, "x"=w3571) -> ("dx/dt"=w3576:dbl)  [unwired: 5 in, 3 out]
                      n1466 = call "2ndOrderDerivate.vi"("t_capture"=w3573, "initial condition"=w3570, "x"=w3570) -> ("dx/dt"=w3575:dbl)  [unwired: 5 in, 3 out]
                    }
                    frame 14 {
                      n1467 = call "2ndOrderDerivate.vi"("t_capture"=w3580, "initial condition"=w3579, "x"=w3579) -> ("dx/dt"=w3581:dbl)  [unwired: 5 in, 3 out]
                      n1468 = call "2ndOrderDerivate.vi"("t_capture"=w3580, "initial condition"=w3578, "x"=w3578) -> ("dx/dt"=w3583:dbl)  [unwired: 5 in, 3 out]
                      n1469 = call "2ndOrderDerivate.vi"("t_capture"=w3580, "initial condition"=w3577, "x"=w3577) -> ("dx/dt"=w3582:dbl)  [unwired: 5 in, 3 out]
                    }
                    frame 15 {
                      n1470 = call "2ndOrderDerivate.vi"("t_capture"=w3587, "initial condition"=w3586, "x"=w3586) -> ("dx/dt"=w3588:dbl)  [unwired: 5 in, 3 out]
                      n1471 = call "2ndOrderDerivate.vi"("t_capture"=w3587, "initial condition"=w3585, "x"=w3585) -> ("dx/dt"=w3590:dbl)  [unwired: 5 in, 3 out]
                      n1472 = call "2ndOrderDerivate.vi"("t_capture"=w3587, "initial condition"=w3584, "x"=w3584) -> ("dx/dt"=w3589:dbl)  [unwired: 5 in, 3 out]
                    }
                  }
                  n1473 = case shown="0, Default" w3358 {
                    tunnel: w3357 -> [w3369 w3376 w3383 w3390 w3397 w3404 w3411 w3418 w3425 w3432 w3439 w3446 w3453 w3460 w3467 w3474]
                    tunnel: [w3371 w3378 w3385 w3392 w3399 w3406 w3413 w3420 w3427 w3434 w3441 w3448 w3455 w3462 w3469 w3476] -> w3354
                    tunnel: [w3373 w3380 w3387 w3394 w3401 w3408 w3415 w3422 w3429 w3436 w3443 w3450 w3457 w3464 w3471 w3478] -> w3353
                    tunnel: [w3372 w3379 w3386 w3393 w3400 w3407 w3414 w3421 w3428 w3435 w3442 w3449 w3456 w3463 w3470 w3477] -> w3352
                    tunnel: w3356 -> [w3368 w3375 w3382 w3389 w3396 w3403 w3410 w3417 w3424 w3431 w3438 w3445 w3452 w3459 w3466 w3473]
                    tunnel: w3355 -> [w3367 w3374 w3381 w3388 w3395 w3402 w3409 w3416 w3423 w3430 w3437 w3444 w3451 w3458 w3465 w3472]
                    tunnel: w3359 -> [w3370 w3377 w3384 w3391 w3398 w3405 w3412 w3419 w3426 w3433 w3440 w3447 w3454 w3461 w3468 w3475]
                    frame 0, Default {
                      n1474 = call "2ndOrderDerivate.vi"("t_capture"=w3370, "initial condition"=w3369, "x"=w3369) -> ("dx/dt"=w3371:dbl)  [unwired: 5 in, 3 out]
                      n1475 = call "2ndOrderDerivate.vi"("t_capture"=w3370, "initial condition"=w3368, "x"=w3368) -> ("dx/dt"=w3373:dbl)  [unwired: 5 in, 3 out]
                      n1476 = call "2ndOrderDerivate.vi"("t_capture"=w3370, "initial condition"=w3367, "x"=w3367) -> ("dx/dt"=w3372:dbl)  [unwired: 5 in, 3 out]
                    }
                    frame 1 {
                      n1477 = call "2ndOrderDerivate.vi"("t_capture"=w3377, "initial condition"=w3376, "x"=w3376) -> ("dx/dt"=w3378:dbl)  [unwired: 5 in, 3 out]
                      n1478 = call "2ndOrderDerivate.vi"("t_capture"=w3377, "initial condition"=w3375, "x"=w3375) -> ("dx/dt"=w3380:dbl)  [unwired: 5 in, 3 out]
                      n1479 = call "2ndOrderDerivate.vi"("t_capture"=w3377, "initial condition"=w3374, "x"=w3374) -> ("dx/dt"=w3379:dbl)  [unwired: 5 in, 3 out]
                    }
                    frame 2 {
                      n1480 = call "2ndOrderDerivate.vi"("t_capture"=w3384, "initial condition"=w3383, "x"=w3383) -> ("dx/dt"=w3385:dbl)  [unwired: 5 in, 3 out]
                      n1481 = call "2ndOrderDerivate.vi"("t_capture"=w3384, "initial condition"=w3382, "x"=w3382) -> ("dx/dt"=w3387:dbl)  [unwired: 5 in, 3 out]
                      n1482 = call "2ndOrderDerivate.vi"("t_capture"=w3384, "initial condition"=w3381, "x"=w3381) -> ("dx/dt"=w3386:dbl)  [unwired: 5 in, 3 out]
                    }
                    frame 3 {
                      n1483 = call "2ndOrderDerivate.vi"("t_capture"=w3391, "initial condition"=w3390, "x"=w3390) -> ("dx/dt"=w3392:dbl)  [unwired: 5 in, 3 out]
                      n1484 = call "2ndOrderDerivate.vi"("t_capture"=w3391, "initial condition"=w3389, "x"=w3389) -> ("dx/dt"=w3394:dbl)  [unwired: 5 in, 3 out]
                      n1485 = call "2ndOrderDerivate.vi"("t_capture"=w3391, "initial condition"=w3388, "x"=w3388) -> ("dx/dt"=w3393:dbl)  [unwired: 5 in, 3 out]
                    }
                    frame 4 {
                      n1486 = call "2ndOrderDerivate.vi"("t_capture"=w3398, "initial condition"=w3397, "x"=w3397) -> ("dx/dt"=w3399:dbl)  [unwired: 5 in, 3 out]
                      n1487 = call "2ndOrderDerivate.vi"("t_capture"=w3398, "initial condition"=w3396, "x"=w3396) -> ("dx/dt"=w3401:dbl)  [unwired: 5 in, 3 out]
                      n1488 = call "2ndOrderDerivate.vi"("t_capture"=w3398, "initial condition"=w3395, "x"=w3395) -> ("dx/dt"=w3400:dbl)  [unwired: 5 in, 3 out]
                    }
                    frame 5 {
                      n1489 = call "2ndOrderDerivate.vi"("t_capture"=w3405, "initial condition"=w3404, "x"=w3404) -> ("dx/dt"=w3406:dbl)  [unwired: 5 in, 3 out]
                      n1490 = call "2ndOrderDerivate.vi"("t_capture"=w3405, "initial condition"=w3403, "x"=w3403) -> ("dx/dt"=w3408:dbl)  [unwired: 5 in, 3 out]
                      n1491 = call "2ndOrderDerivate.vi"("t_capture"=w3405, "initial condition"=w3402, "x"=w3402) -> ("dx/dt"=w3407:dbl)  [unwired: 5 in, 3 out]
                    }
                    frame 6 {
                      n1492 = call "2ndOrderDerivate.vi"("t_capture"=w3412, "initial condition"=w3411, "x"=w3411) -> ("dx/dt"=w3413:dbl)  [unwired: 5 in, 3 out]
                      n1493 = call "2ndOrderDerivate.vi"("t_capture"=w3412, "initial condition"=w3410, "x"=w3410) -> ("dx/dt"=w3415:dbl)  [unwired: 5 in, 3 out]
                      n1494 = call "2ndOrderDerivate.vi"("t_capture"=w3412, "initial condition"=w3409, "x"=w3409) -> ("dx/dt"=w3414:dbl)  [unwired: 5 in, 3 out]
                    }
                    frame 7 {
                      n1495 = call "2ndOrderDerivate.vi"("t_capture"=w3419, "initial condition"=w3418, "x"=w3418) -> ("dx/dt"=w3420:dbl)  [unwired: 5 in, 3 out]
                      n1496 = call "2ndOrderDerivate.vi"("t_capture"=w3419, "initial condition"=w3417, "x"=w3417) -> ("dx/dt"=w3422:dbl)  [unwired: 5 in, 3 out]
                      n1497 = call "2ndOrderDerivate.vi"("t_capture"=w3419, "initial condition"=w3416, "x"=w3416) -> ("dx/dt"=w3421:dbl)  [unwired: 5 in, 3 out]
                    }
                    frame 8 {
                      n1498 = call "2ndOrderDerivate.vi"("t_capture"=w3426, "initial condition"=w3425, "x"=w3425) -> ("dx/dt"=w3427:dbl)  [unwired: 5 in, 3 out]
                      n1499 = call "2ndOrderDerivate.vi"("t_capture"=w3426, "initial condition"=w3424, "x"=w3424) -> ("dx/dt"=w3429:dbl)  [unwired: 5 in, 3 out]
                      n1500 = call "2ndOrderDerivate.vi"("t_capture"=w3426, "initial condition"=w3423, "x"=w3423) -> ("dx/dt"=w3428:dbl)  [unwired: 5 in, 3 out]
                    }
                    frame 9 {
                      n1501 = call "2ndOrderDerivate.vi"("t_capture"=w3433, "initial condition"=w3432, "x"=w3432) -> ("dx/dt"=w3434:dbl)  [unwired: 5 in, 3 out]
                      n1502 = call "2ndOrderDerivate.vi"("t_capture"=w3433, "initial condition"=w3431, "x"=w3431) -> ("dx/dt"=w3436:dbl)  [unwired: 5 in, 3 out]
                      n1503 = call "2ndOrderDerivate.vi"("t_capture"=w3433, "initial condition"=w3430, "x"=w3430) -> ("dx/dt"=w3435:dbl)  [unwired: 5 in, 3 out]
                    }
                    frame 10 {
                      n1504 = call "2ndOrderDerivate.vi"("t_capture"=w3440, "initial condition"=w3439, "x"=w3439) -> ("dx/dt"=w3441:dbl)  [unwired: 5 in, 3 out]
                      n1505 = call "2ndOrderDerivate.vi"("t_capture"=w3440, "initial condition"=w3438, "x"=w3438) -> ("dx/dt"=w3443:dbl)  [unwired: 5 in, 3 out]
                      n1506 = call "2ndOrderDerivate.vi"("t_capture"=w3440, "initial condition"=w3437, "x"=w3437) -> ("dx/dt"=w3442:dbl)  [unwired: 5 in, 3 out]
                    }
                    frame 11 {
                      n1507 = call "2ndOrderDerivate.vi"("t_capture"=w3447, "initial condition"=w3446, "x"=w3446) -> ("dx/dt"=w3448:dbl)  [unwired: 5 in, 3 out]
                      n1508 = call "2ndOrderDerivate.vi"("t_capture"=w3447, "initial condition"=w3445, "x"=w3445) -> ("dx/dt"=w3450:dbl)  [unwired: 5 in, 3 out]
                      n1509 = call "2ndOrderDerivate.vi"("t_capture"=w3447, "initial condition"=w3444, "x"=w3444) -> ("dx/dt"=w3449:dbl)  [unwired: 5 in, 3 out]
                    }
                    frame 12 {
                      n1510 = call "2ndOrderDerivate.vi"("t_capture"=w3454, "initial condition"=w3453, "x"=w3453) -> ("dx/dt"=w3455:dbl)  [unwired: 5 in, 3 out]
                      n1511 = call "2ndOrderDerivate.vi"("t_capture"=w3454, "initial condition"=w3452, "x"=w3452) -> ("dx/dt"=w3457:dbl)  [unwired: 5 in, 3 out]
                      n1512 = call "2ndOrderDerivate.vi"("t_capture"=w3454, "initial condition"=w3451, "x"=w3451) -> ("dx/dt"=w3456:dbl)  [unwired: 5 in, 3 out]
                    }
                    frame 13 {
                      n1513 = call "2ndOrderDerivate.vi"("t_capture"=w3461, "initial condition"=w3460, "x"=w3460) -> ("dx/dt"=w3462:dbl)  [unwired: 5 in, 3 out]
                      n1514 = call "2ndOrderDerivate.vi"("t_capture"=w3461, "initial condition"=w3459, "x"=w3459) -> ("dx/dt"=w3464:dbl)  [unwired: 5 in, 3 out]
                      n1515 = call "2ndOrderDerivate.vi"("t_capture"=w3461, "initial condition"=w3458, "x"=w3458) -> ("dx/dt"=w3463:dbl)  [unwired: 5 in, 3 out]
                    }
                    frame 14 {
                      n1516 = call "2ndOrderDerivate.vi"("t_capture"=w3468, "initial condition"=w3467, "x"=w3467) -> ("dx/dt"=w3469:dbl)  [unwired: 5 in, 3 out]
                      n1517 = call "2ndOrderDerivate.vi"("t_capture"=w3468, "initial condition"=w3466, "x"=w3466) -> ("dx/dt"=w3471:dbl)  [unwired: 5 in, 3 out]
                      n1518 = call "2ndOrderDerivate.vi"("t_capture"=w3468, "initial condition"=w3465, "x"=w3465) -> ("dx/dt"=w3470:dbl)  [unwired: 5 in, 3 out]
                    }
                    frame 15 {
                      n1519 = call "2ndOrderDerivate.vi"("t_capture"=w3475, "initial condition"=w3474, "x"=w3474) -> ("dx/dt"=w3476:dbl)  [unwired: 5 in, 3 out]
                      n1520 = call "2ndOrderDerivate.vi"("t_capture"=w3475, "initial condition"=w3473, "x"=w3473) -> ("dx/dt"=w3478:dbl)  [unwired: 5 in, 3 out]
                      n1521 = call "2ndOrderDerivate.vi"("t_capture"=w3475, "initial condition"=w3472, "x"=w3472) -> ("dx/dt"=w3477:dbl)  [unwired: 5 in, 3 out]
                    }
                  }
                  n1522 = Build Array(w3361, w3357, w3364, w3356, w3363, w3355, w3354, w3353, w3352) -> (w3366:dbl[])
                  n1523 = call-poly <vilib>:"Array To Matrix.vi"("Real 1D Array"=w3366) -> ("Real Matrix (Column Vector)"=w3365:T3)
                  n1524 = Bundle By Name(cluster=w3360, "x_k|k"=w3365) -> (w3362:T2)
                }
              }
              frame True {
              }
            }
            n1525 = case shown="False" w3331 {
              tunnel: w3330 -> [w3594 w3835]
              tunnel: w3318 -> [w3595 _]
              tunnel: [w3593 w3835] -> w3326
              tunnel: w3316 -> [w3592 _]
              frame False {
                n1526 = for {
                  tunnel: w3594 -> [w3604] mode=indexing
                  tunnel: w3595 -> [_]
                  tunnel: [w3606] -> w3593 mode=indexing
                  tunnel: w3592 -> [w3603]
                  n1527 = Unbundle By Name(w3604) -> ("x"=w3605:sgl, "y"=w3608:sgl, "orientation"=w3607:sgl, "robot_id"=w3602:u32)  [unwired: 1 out]
                  n1528 = case shown="0, Default" w3602 {
                    tunnel: w3605 -> [w3725 w3732 w3739 w3746 w3753 w3760 w3767 w3774 w3781 w3788 w3795 w3802 w3809 w3816 w3823 w3830]
                    tunnel: [w3727 w3734 w3741 w3748 w3755 w3762 w3769 w3776 w3783 w3790 w3797 w3804 w3811 w3818 w3825 w3832] -> w3601
                    tunnel: [w3729 w3736 w3743 w3750 w3757 w3764 w3771 w3778 w3785 w3792 w3799 w3806 w3813 w3820 w3827 w3834] -> w3600
                    tunnel: [w3728 w3735 w3742 w3749 w3756 w3763 w3770 w3777 w3784 w3791 w3798 w3805 w3812 w3819 w3826 w3833] -> w3599
                    tunnel: w3608 -> [w3724 w3731 w3738 w3745 w3752 w3759 w3766 w3773 w3780 w3787 w3794 w3801 w3808 w3815 w3822 w3829]
                    tunnel: w3607 -> [w3723 w3730 w3737 w3744 w3751 w3758 w3765 w3772 w3779 w3786 w3793 w3800 w3807 w3814 w3821 w3828]
                    tunnel: w3603 -> [w3726 w3733 w3740 w3747 w3754 w3761 w3768 w3775 w3782 w3789 w3796 w3803 w3810 w3817 w3824 w3831]
                    frame 0, Default {
                      n1529 = call "2ndOrderDerivate.vi"("t_capture"=w3726, "initial condition"=w3725, "x"=w3725) -> ("dx/dt"=w3727:dbl)  [unwired: 5 in, 3 out]
                      n1530 = call "2ndOrderDerivate.vi"("t_capture"=w3726, "initial condition"=w3724, "x"=w3724) -> ("dx/dt"=w3729:dbl)  [unwired: 5 in, 3 out]
                      n1531 = call "2ndOrderDerivate.vi"("t_capture"=w3726, "initial condition"=w3723, "x"=w3723) -> ("dx/dt"=w3728:dbl)  [unwired: 5 in, 3 out]
                    }
                    frame 1 {
                      n1532 = call "2ndOrderDerivate.vi"("t_capture"=w3733, "initial condition"=w3732, "x"=w3732) -> ("dx/dt"=w3734:dbl)  [unwired: 5 in, 3 out]
                      n1533 = call "2ndOrderDerivate.vi"("t_capture"=w3733, "initial condition"=w3731, "x"=w3731) -> ("dx/dt"=w3736:dbl)  [unwired: 5 in, 3 out]
                      n1534 = call "2ndOrderDerivate.vi"("t_capture"=w3733, "initial condition"=w3730, "x"=w3730) -> ("dx/dt"=w3735:dbl)  [unwired: 5 in, 3 out]
                    }
                    frame 2 {
                      n1535 = call "2ndOrderDerivate.vi"("t_capture"=w3740, "initial condition"=w3739, "x"=w3739) -> ("dx/dt"=w3741:dbl)  [unwired: 5 in, 3 out]
                      n1536 = call "2ndOrderDerivate.vi"("t_capture"=w3740, "initial condition"=w3738, "x"=w3738) -> ("dx/dt"=w3743:dbl)  [unwired: 5 in, 3 out]
                      n1537 = call "2ndOrderDerivate.vi"("t_capture"=w3740, "initial condition"=w3737, "x"=w3737) -> ("dx/dt"=w3742:dbl)  [unwired: 5 in, 3 out]
                    }
                    frame 3 {
                      n1538 = call "2ndOrderDerivate.vi"("t_capture"=w3747, "initial condition"=w3746, "x"=w3746) -> ("dx/dt"=w3748:dbl)  [unwired: 5 in, 3 out]
                      n1539 = call "2ndOrderDerivate.vi"("t_capture"=w3747, "initial condition"=w3745, "x"=w3745) -> ("dx/dt"=w3750:dbl)  [unwired: 5 in, 3 out]
                      n1540 = call "2ndOrderDerivate.vi"("t_capture"=w3747, "initial condition"=w3744, "x"=w3744) -> ("dx/dt"=w3749:dbl)  [unwired: 5 in, 3 out]
                    }
                    frame 4 {
                      n1541 = call "2ndOrderDerivate.vi"("t_capture"=w3754, "initial condition"=w3753, "x"=w3753) -> ("dx/dt"=w3755:dbl)  [unwired: 5 in, 3 out]
                      n1542 = call "2ndOrderDerivate.vi"("t_capture"=w3754, "initial condition"=w3752, "x"=w3752) -> ("dx/dt"=w3757:dbl)  [unwired: 5 in, 3 out]
                      n1543 = call "2ndOrderDerivate.vi"("t_capture"=w3754, "initial condition"=w3751, "x"=w3751) -> ("dx/dt"=w3756:dbl)  [unwired: 5 in, 3 out]
                    }
                    frame 5 {
                      n1544 = call "2ndOrderDerivate.vi"("t_capture"=w3761, "initial condition"=w3760, "x"=w3760) -> ("dx/dt"=w3762:dbl)  [unwired: 5 in, 3 out]
                      n1545 = call "2ndOrderDerivate.vi"("t_capture"=w3761, "initial condition"=w3759, "x"=w3759) -> ("dx/dt"=w3764:dbl)  [unwired: 5 in, 3 out]
                      n1546 = call "2ndOrderDerivate.vi"("t_capture"=w3761, "initial condition"=w3758, "x"=w3758) -> ("dx/dt"=w3763:dbl)  [unwired: 5 in, 3 out]
                    }
                    frame 6 {
                      n1547 = call "2ndOrderDerivate.vi"("t_capture"=w3768, "initial condition"=w3767, "x"=w3767) -> ("dx/dt"=w3769:dbl)  [unwired: 5 in, 3 out]
                      n1548 = call "2ndOrderDerivate.vi"("t_capture"=w3768, "initial condition"=w3766, "x"=w3766) -> ("dx/dt"=w3771:dbl)  [unwired: 5 in, 3 out]
                      n1549 = call "2ndOrderDerivate.vi"("t_capture"=w3768, "initial condition"=w3765, "x"=w3765) -> ("dx/dt"=w3770:dbl)  [unwired: 5 in, 3 out]
                    }
                    frame 7 {
                      n1550 = call "2ndOrderDerivate.vi"("t_capture"=w3775, "initial condition"=w3774, "x"=w3774) -> ("dx/dt"=w3776:dbl)  [unwired: 5 in, 3 out]
                      n1551 = call "2ndOrderDerivate.vi"("t_capture"=w3775, "initial condition"=w3773, "x"=w3773) -> ("dx/dt"=w3778:dbl)  [unwired: 5 in, 3 out]
                      n1552 = call "2ndOrderDerivate.vi"("t_capture"=w3775, "initial condition"=w3772, "x"=w3772) -> ("dx/dt"=w3777:dbl)  [unwired: 5 in, 3 out]
                    }
                    frame 8 {
                      n1553 = call "2ndOrderDerivate.vi"("t_capture"=w3782, "initial condition"=w3781, "x"=w3781) -> ("dx/dt"=w3783:dbl)  [unwired: 5 in, 3 out]
                      n1554 = call "2ndOrderDerivate.vi"("t_capture"=w3782, "initial condition"=w3780, "x"=w3780) -> ("dx/dt"=w3785:dbl)  [unwired: 5 in, 3 out]
                      n1555 = call "2ndOrderDerivate.vi"("t_capture"=w3782, "initial condition"=w3779, "x"=w3779) -> ("dx/dt"=w3784:dbl)  [unwired: 5 in, 3 out]
                    }
                    frame 9 {
                      n1556 = call "2ndOrderDerivate.vi"("t_capture"=w3789, "initial condition"=w3788, "x"=w3788) -> ("dx/dt"=w3790:dbl)  [unwired: 5 in, 3 out]
                      n1557 = call "2ndOrderDerivate.vi"("t_capture"=w3789, "initial condition"=w3787, "x"=w3787) -> ("dx/dt"=w3792:dbl)  [unwired: 5 in, 3 out]
                      n1558 = call "2ndOrderDerivate.vi"("t_capture"=w3789, "initial condition"=w3786, "x"=w3786) -> ("dx/dt"=w3791:dbl)  [unwired: 5 in, 3 out]
                    }
                    frame 10 {
                      n1559 = call "2ndOrderDerivate.vi"("t_capture"=w3796, "initial condition"=w3795, "x"=w3795) -> ("dx/dt"=w3797:dbl)  [unwired: 5 in, 3 out]
                      n1560 = call "2ndOrderDerivate.vi"("t_capture"=w3796, "initial condition"=w3794, "x"=w3794) -> ("dx/dt"=w3799:dbl)  [unwired: 5 in, 3 out]
                      n1561 = call "2ndOrderDerivate.vi"("t_capture"=w3796, "initial condition"=w3793, "x"=w3793) -> ("dx/dt"=w3798:dbl)  [unwired: 5 in, 3 out]
                    }
                    frame 11 {
                      n1562 = call "2ndOrderDerivate.vi"("t_capture"=w3803, "initial condition"=w3802, "x"=w3802) -> ("dx/dt"=w3804:dbl)  [unwired: 5 in, 3 out]
                      n1563 = call "2ndOrderDerivate.vi"("t_capture"=w3803, "initial condition"=w3801, "x"=w3801) -> ("dx/dt"=w3806:dbl)  [unwired: 5 in, 3 out]
                      n1564 = call "2ndOrderDerivate.vi"("t_capture"=w3803, "initial condition"=w3800, "x"=w3800) -> ("dx/dt"=w3805:dbl)  [unwired: 5 in, 3 out]
                    }
                    frame 12 {
                      n1565 = call "2ndOrderDerivate.vi"("t_capture"=w3810, "initial condition"=w3809, "x"=w3809) -> ("dx/dt"=w3811:dbl)  [unwired: 5 in, 3 out]
                      n1566 = call "2ndOrderDerivate.vi"("t_capture"=w3810, "initial condition"=w3808, "x"=w3808) -> ("dx/dt"=w3813:dbl)  [unwired: 5 in, 3 out]
                      n1567 = call "2ndOrderDerivate.vi"("t_capture"=w3810, "initial condition"=w3807, "x"=w3807) -> ("dx/dt"=w3812:dbl)  [unwired: 5 in, 3 out]
                    }
                    frame 13 {
                      n1568 = call "2ndOrderDerivate.vi"("t_capture"=w3817, "initial condition"=w3816, "x"=w3816) -> ("dx/dt"=w3818:dbl)  [unwired: 5 in, 3 out]
                      n1569 = call "2ndOrderDerivate.vi"("t_capture"=w3817, "initial condition"=w3815, "x"=w3815) -> ("dx/dt"=w3820:dbl)  [unwired: 5 in, 3 out]
                      n1570 = call "2ndOrderDerivate.vi"("t_capture"=w3817, "initial condition"=w3814, "x"=w3814) -> ("dx/dt"=w3819:dbl)  [unwired: 5 in, 3 out]
                    }
                    frame 14 {
                      n1571 = call "2ndOrderDerivate.vi"("t_capture"=w3824, "initial condition"=w3823, "x"=w3823) -> ("dx/dt"=w3825:dbl)  [unwired: 5 in, 3 out]
                      n1572 = call "2ndOrderDerivate.vi"("t_capture"=w3824, "initial condition"=w3822, "x"=w3822) -> ("dx/dt"=w3827:dbl)  [unwired: 5 in, 3 out]
                      n1573 = call "2ndOrderDerivate.vi"("t_capture"=w3824, "initial condition"=w3821, "x"=w3821) -> ("dx/dt"=w3826:dbl)  [unwired: 5 in, 3 out]
                    }
                    frame 15 {
                      n1574 = call "2ndOrderDerivate.vi"("t_capture"=w3831, "initial condition"=w3830, "x"=w3830) -> ("dx/dt"=w3832:dbl)  [unwired: 5 in, 3 out]
                      n1575 = call "2ndOrderDerivate.vi"("t_capture"=w3831, "initial condition"=w3829, "x"=w3829) -> ("dx/dt"=w3834:dbl)  [unwired: 5 in, 3 out]
                      n1576 = call "2ndOrderDerivate.vi"("t_capture"=w3831, "initial condition"=w3828, "x"=w3828) -> ("dx/dt"=w3833:dbl)  [unwired: 5 in, 3 out]
                    }
                  }
                  n1577 = case shown="0, Default" w3602 {
                    tunnel: w3601 -> [w3613 w3620 w3627 w3634 w3641 w3648 w3655 w3662 w3669 w3676 w3683 w3690 w3697 w3704 w3711 w3718]
                    tunnel: [w3615 w3622 w3629 w3636 w3643 w3650 w3657 w3664 w3671 w3678 w3685 w3692 w3699 w3706 w3713 w3720] -> w3598
                    tunnel: [w3617 w3624 w3631 w3638 w3645 w3652 w3659 w3666 w3673 w3680 w3687 w3694 w3701 w3708 w3715 w3722] -> w3597
                    tunnel: [w3616 w3623 w3630 w3637 w3644 w3651 w3658 w3665 w3672 w3679 w3686 w3693 w3700 w3707 w3714 w3721] -> w3596
                    tunnel: w3600 -> [w3612 w3619 w3626 w3633 w3640 w3647 w3654 w3661 w3668 w3675 w3682 w3689 w3696 w3703 w3710 w3717]
                    tunnel: w3599 -> [w3611 w3618 w3625 w3632 w3639 w3646 w3653 w3660 w3667 w3674 w3681 w3688 w3695 w3702 w3709 w3716]
                    tunnel: w3603 -> [w3614 w3621 w3628 w3635 w3642 w3649 w3656 w3663 w3670 w3677 w3684 w3691 w3698 w3705 w3712 w3719]
                    frame 0, Default {
                      n1578 = call "2ndOrderDerivate.vi"("t_capture"=w3614, "initial condition"=w3613, "x"=w3613) -> ("dx/dt"=w3615:dbl)  [unwired: 5 in, 3 out]
                      n1579 = call "2ndOrderDerivate.vi"("t_capture"=w3614, "initial condition"=w3612, "x"=w3612) -> ("dx/dt"=w3617:dbl)  [unwired: 5 in, 3 out]
                      n1580 = call "2ndOrderDerivate.vi"("t_capture"=w3614, "initial condition"=w3611, "x"=w3611) -> ("dx/dt"=w3616:dbl)  [unwired: 5 in, 3 out]
                    }
                    frame 1 {
                      n1581 = call "2ndOrderDerivate.vi"("t_capture"=w3621, "initial condition"=w3620, "x"=w3620) -> ("dx/dt"=w3622:dbl)  [unwired: 5 in, 3 out]
                      n1582 = call "2ndOrderDerivate.vi"("t_capture"=w3621, "initial condition"=w3619, "x"=w3619) -> ("dx/dt"=w3624:dbl)  [unwired: 5 in, 3 out]
                      n1583 = call "2ndOrderDerivate.vi"("t_capture"=w3621, "initial condition"=w3618, "x"=w3618) -> ("dx/dt"=w3623:dbl)  [unwired: 5 in, 3 out]
                    }
                    frame 2 {
                      n1584 = call "2ndOrderDerivate.vi"("t_capture"=w3628, "initial condition"=w3627, "x"=w3627) -> ("dx/dt"=w3629:dbl)  [unwired: 5 in, 3 out]
                      n1585 = call "2ndOrderDerivate.vi"("t_capture"=w3628, "initial condition"=w3626, "x"=w3626) -> ("dx/dt"=w3631:dbl)  [unwired: 5 in, 3 out]
                      n1586 = call "2ndOrderDerivate.vi"("t_capture"=w3628, "initial condition"=w3625, "x"=w3625) -> ("dx/dt"=w3630:dbl)  [unwired: 5 in, 3 out]
                    }
                    frame 3 {
                      n1587 = call "2ndOrderDerivate.vi"("t_capture"=w3635, "initial condition"=w3634, "x"=w3634) -> ("dx/dt"=w3636:dbl)  [unwired: 5 in, 3 out]
                      n1588 = call "2ndOrderDerivate.vi"("t_capture"=w3635, "initial condition"=w3633, "x"=w3633) -> ("dx/dt"=w3638:dbl)  [unwired: 5 in, 3 out]
                      n1589 = call "2ndOrderDerivate.vi"("t_capture"=w3635, "initial condition"=w3632, "x"=w3632) -> ("dx/dt"=w3637:dbl)  [unwired: 5 in, 3 out]
                    }
                    frame 4 {
                      n1590 = call "2ndOrderDerivate.vi"("t_capture"=w3642, "initial condition"=w3641, "x"=w3641) -> ("dx/dt"=w3643:dbl)  [unwired: 5 in, 3 out]
                      n1591 = call "2ndOrderDerivate.vi"("t_capture"=w3642, "initial condition"=w3640, "x"=w3640) -> ("dx/dt"=w3645:dbl)  [unwired: 5 in, 3 out]
                      n1592 = call "2ndOrderDerivate.vi"("t_capture"=w3642, "initial condition"=w3639, "x"=w3639) -> ("dx/dt"=w3644:dbl)  [unwired: 5 in, 3 out]
                    }
                    frame 5 {
                      n1593 = call "2ndOrderDerivate.vi"("t_capture"=w3649, "initial condition"=w3648, "x"=w3648) -> ("dx/dt"=w3650:dbl)  [unwired: 5 in, 3 out]
                      n1594 = call "2ndOrderDerivate.vi"("t_capture"=w3649, "initial condition"=w3647, "x"=w3647) -> ("dx/dt"=w3652:dbl)  [unwired: 5 in, 3 out]
                      n1595 = call "2ndOrderDerivate.vi"("t_capture"=w3649, "initial condition"=w3646, "x"=w3646) -> ("dx/dt"=w3651:dbl)  [unwired: 5 in, 3 out]
                    }
                    frame 6 {
                      n1596 = call "2ndOrderDerivate.vi"("t_capture"=w3656, "initial condition"=w3655, "x"=w3655) -> ("dx/dt"=w3657:dbl)  [unwired: 5 in, 3 out]
                      n1597 = call "2ndOrderDerivate.vi"("t_capture"=w3656, "initial condition"=w3654, "x"=w3654) -> ("dx/dt"=w3659:dbl)  [unwired: 5 in, 3 out]
                      n1598 = call "2ndOrderDerivate.vi"("t_capture"=w3656, "initial condition"=w3653, "x"=w3653) -> ("dx/dt"=w3658:dbl)  [unwired: 5 in, 3 out]
                    }
                    frame 7 {
                      n1599 = call "2ndOrderDerivate.vi"("t_capture"=w3663, "initial condition"=w3662, "x"=w3662) -> ("dx/dt"=w3664:dbl)  [unwired: 5 in, 3 out]
                      n1600 = call "2ndOrderDerivate.vi"("t_capture"=w3663, "initial condition"=w3661, "x"=w3661) -> ("dx/dt"=w3666:dbl)  [unwired: 5 in, 3 out]
                      n1601 = call "2ndOrderDerivate.vi"("t_capture"=w3663, "initial condition"=w3660, "x"=w3660) -> ("dx/dt"=w3665:dbl)  [unwired: 5 in, 3 out]
                    }
                    frame 8 {
                      n1602 = call "2ndOrderDerivate.vi"("t_capture"=w3670, "initial condition"=w3669, "x"=w3669) -> ("dx/dt"=w3671:dbl)  [unwired: 5 in, 3 out]
                      n1603 = call "2ndOrderDerivate.vi"("t_capture"=w3670, "initial condition"=w3668, "x"=w3668) -> ("dx/dt"=w3673:dbl)  [unwired: 5 in, 3 out]
                      n1604 = call "2ndOrderDerivate.vi"("t_capture"=w3670, "initial condition"=w3667, "x"=w3667) -> ("dx/dt"=w3672:dbl)  [unwired: 5 in, 3 out]
                    }
                    frame 9 {
                      n1605 = call "2ndOrderDerivate.vi"("t_capture"=w3677, "initial condition"=w3676, "x"=w3676) -> ("dx/dt"=w3678:dbl)  [unwired: 5 in, 3 out]
                      n1606 = call "2ndOrderDerivate.vi"("t_capture"=w3677, "initial condition"=w3675, "x"=w3675) -> ("dx/dt"=w3680:dbl)  [unwired: 5 in, 3 out]
                      n1607 = call "2ndOrderDerivate.vi"("t_capture"=w3677, "initial condition"=w3674, "x"=w3674) -> ("dx/dt"=w3679:dbl)  [unwired: 5 in, 3 out]
                    }
                    frame 10 {
                      n1608 = call "2ndOrderDerivate.vi"("t_capture"=w3684, "initial condition"=w3683, "x"=w3683) -> ("dx/dt"=w3685:dbl)  [unwired: 5 in, 3 out]
                      n1609 = call "2ndOrderDerivate.vi"("t_capture"=w3684, "initial condition"=w3682, "x"=w3682) -> ("dx/dt"=w3687:dbl)  [unwired: 5 in, 3 out]
                      n1610 = call "2ndOrderDerivate.vi"("t_capture"=w3684, "initial condition"=w3681, "x"=w3681) -> ("dx/dt"=w3686:dbl)  [unwired: 5 in, 3 out]
                    }
                    frame 11 {
                      n1611 = call "2ndOrderDerivate.vi"("t_capture"=w3691, "initial condition"=w3690, "x"=w3690) -> ("dx/dt"=w3692:dbl)  [unwired: 5 in, 3 out]
                      n1612 = call "2ndOrderDerivate.vi"("t_capture"=w3691, "initial condition"=w3689, "x"=w3689) -> ("dx/dt"=w3694:dbl)  [unwired: 5 in, 3 out]
                      n1613 = call "2ndOrderDerivate.vi"("t_capture"=w3691, "initial condition"=w3688, "x"=w3688) -> ("dx/dt"=w3693:dbl)  [unwired: 5 in, 3 out]
                    }
                    frame 12 {
                      n1614 = call "2ndOrderDerivate.vi"("t_capture"=w3698, "initial condition"=w3697, "x"=w3697) -> ("dx/dt"=w3699:dbl)  [unwired: 5 in, 3 out]
                      n1615 = call "2ndOrderDerivate.vi"("t_capture"=w3698, "initial condition"=w3696, "x"=w3696) -> ("dx/dt"=w3701:dbl)  [unwired: 5 in, 3 out]
                      n1616 = call "2ndOrderDerivate.vi"("t_capture"=w3698, "initial condition"=w3695, "x"=w3695) -> ("dx/dt"=w3700:dbl)  [unwired: 5 in, 3 out]
                    }
                    frame 13 {
                      n1617 = call "2ndOrderDerivate.vi"("t_capture"=w3705, "initial condition"=w3704, "x"=w3704) -> ("dx/dt"=w3706:dbl)  [unwired: 5 in, 3 out]
                      n1618 = call "2ndOrderDerivate.vi"("t_capture"=w3705, "initial condition"=w3703, "x"=w3703) -> ("dx/dt"=w3708:dbl)  [unwired: 5 in, 3 out]
                      n1619 = call "2ndOrderDerivate.vi"("t_capture"=w3705, "initial condition"=w3702, "x"=w3702) -> ("dx/dt"=w3707:dbl)  [unwired: 5 in, 3 out]
                    }
                    frame 14 {
                      n1620 = call "2ndOrderDerivate.vi"("t_capture"=w3712, "initial condition"=w3711, "x"=w3711) -> ("dx/dt"=w3713:dbl)  [unwired: 5 in, 3 out]
                      n1621 = call "2ndOrderDerivate.vi"("t_capture"=w3712, "initial condition"=w3710, "x"=w3710) -> ("dx/dt"=w3715:dbl)  [unwired: 5 in, 3 out]
                      n1622 = call "2ndOrderDerivate.vi"("t_capture"=w3712, "initial condition"=w3709, "x"=w3709) -> ("dx/dt"=w3714:dbl)  [unwired: 5 in, 3 out]
                    }
                    frame 15 {
                      n1623 = call "2ndOrderDerivate.vi"("t_capture"=w3719, "initial condition"=w3718, "x"=w3718) -> ("dx/dt"=w3720:dbl)  [unwired: 5 in, 3 out]
                      n1624 = call "2ndOrderDerivate.vi"("t_capture"=w3719, "initial condition"=w3717, "x"=w3717) -> ("dx/dt"=w3722:dbl)  [unwired: 5 in, 3 out]
                      n1625 = call "2ndOrderDerivate.vi"("t_capture"=w3719, "initial condition"=w3716, "x"=w3716) -> ("dx/dt"=w3721:dbl)  [unwired: 5 in, 3 out]
                    }
                  }
                  n1626 = Build Array(w3605, w3601, w3608, w3600, w3607, w3599, w3598, w3597, w3596) -> (w3610:dbl[])
                  n1627 = call-poly <vilib>:"Array To Matrix.vi"("Real 1D Array"=w3610) -> ("Real Matrix (Column Vector)"=w3609:T3)
                  n1628 = Bundle By Name(cluster=w3604, "x_k|k"=w3609) -> (w3606:T2)
                }
              }
              frame True {
              }
            }
            n1629 = Bundle By Name(cluster=w3321, "robots_blue"=w3326, "robots_yellow"=w3325, "balls"=w3317) -> (w3324:T1)
            n1630 = Bundle By Name(cluster=w3321, "New"=FALSE) -> (w3322:T1)
          }
          frame 1 {
            n1631 = Empty Array?(array=w3839) -> (empty?=w3840:bool)
            n1632 = Empty Array?(array=w3847) -> (empty?=w3848:bool)
            n1633 = Reciprocal(x=w3849) -> (1/x=w3838:dbl)
            n1634 = Empty Array?(array=w3850) -> (empty?=w3851:bool)
            n1635 = case shown="False" w3840 {
              tunnel: w3839 -> [w3854 w3868]
              tunnel: w3838 -> [w3855 _]
              tunnel: [w3853 w3868] -> w3837
              tunnel: w3836 -> [w3852 _]
              frame False {
                n1636 = for {
                  tunnel: w3854 -> [w3867] mode=indexing
                  tunnel: w3855 -> [_]
                  tunnel: w3854 -> [w3866] mode=indexing
                  tunnel: [w3863] -> w3853 mode=indexing
                  tunnel: w3852 -> [w3861]
                  n1637 = Unbundle By Name(w3867) -> ("x"=w3862:sgl, "y"=w3860:sgl, "z"=w3856:sgl)
                  n1638 = call "2ndOrderDerivate.vi"("t_capture"=w3861, "initial condition"=w3860, "x"=w3860) -> ("dx/dt"=w3858:dbl)  [unwired: 5 in, 3 out]
                  n1639 = call "2ndOrderDerivate.vi"("t_capture"=w3861, "initial condition"=w3862, "x"=w3862) -> ("dx/dt"=w3859:dbl)  [unwired: 5 in, 3 out]
                  n1640 = call "2ndOrderDerivate.vi"("t_capture"=w3861, "initial condition"=w3856, "x"=w3856) -> ("dx/dt"=w3857:dbl)  [unwired: 5 in, 3 out]
                  n1641 = Build Array(w3862, w3859, w3860, w3858, w3856, w3857) -> (w3865:dbl[])
                  n1642 = call-poly <vilib>:"Array To Matrix.vi"("Real 1D Array"=w3865) -> ("Real Matrix (Column Vector)"=w3864:T3)
                  n1643 = Bundle By Name(cluster=w3866, "x_k|k"=w3864) -> (w3863:T4)
                }
              }
              frame True {
              }
            }
            n1644 = case shown="False" w3848 {
              tunnel: w3847 -> [w3870 w4111]
              tunnel: w3838 -> [_ _]
              tunnel: [w3871 w4111] -> w3845
              tunnel: w3836 -> [w3869 _]
              frame False {
                n1645 = for {
                  tunnel: w3870 -> [w3880] mode=indexing
                  tunnel: [w3882] -> w3871 mode=indexing
                  tunnel: w3869 -> [w3879]
                  n1646 = Unbundle By Name(w3880) -> ("x"=w3881:sgl, "y"=w3884:sgl, "orientation"=w3883:sgl, "robot_id"=w3878:u32)  [unwired: 1 out]
                  n1647 = case shown="0, Default" w3878 {
                    tunnel: w3881 -> [w4001 w4008 w4015 w4022 w4029 w4036 w4043 w4050 w4057 w4064 w4071 w4078 w4085 w4092 w4099 w4106]
                    tunnel: [w4003 w4010 w4017 w4024 w4031 w4038 w4045 w4052 w4059 w4066 w4073 w4080 w4087 w4094 w4101 w4108] -> w3877
                    tunnel: [w4005 w4012 w4019 w4026 w4033 w4040 w4047 w4054 w4061 w4068 w4075 w4082 w4089 w4096 w4103 w4110] -> w3876
                    tunnel: [w4004 w4011 w4018 w4025 w4032 w4039 w4046 w4053 w4060 w4067 w4074 w4081 w4088 w4095 w4102 w4109] -> w3875
                    tunnel: w3884 -> [w4000 w4007 w4014 w4021 w4028 w4035 w4042 w4049 w4056 w4063 w4070 w4077 w4084 w4091 w4098 w4105]
                    tunnel: w3883 -> [w3999 w4006 w4013 w4020 w4027 w4034 w4041 w4048 w4055 w4062 w4069 w4076 w4083 w4090 w4097 w4104]
                    tunnel: w3879 -> [w4002 w4009 w4016 w4023 w4030 w4037 w4044 w4051 w4058 w4065 w4072 w4079 w4086 w4093 w4100 w4107]
                    frame 0, Default {
                      n1648 = call "2ndOrderDerivate.vi"("t_capture"=w4002, "initial condition"=w4001, "x"=w4001) -> ("dx/dt"=w4003:dbl)  [unwired: 5 in, 3 out]
                      n1649 = call "2ndOrderDerivate.vi"("t_capture"=w4002, "initial condition"=w4000, "x"=w4000) -> ("dx/dt"=w4005:dbl)  [unwired: 5 in, 3 out]
                      n1650 = call "2ndOrderDerivate.vi"("t_capture"=w4002, "initial condition"=w3999, "x"=w3999) -> ("dx/dt"=w4004:dbl)  [unwired: 5 in, 3 out]
                    }
                    frame 1 {
                      n1651 = call "2ndOrderDerivate.vi"("t_capture"=w4009, "initial condition"=w4008, "x"=w4008) -> ("dx/dt"=w4010:dbl)  [unwired: 5 in, 3 out]
                      n1652 = call "2ndOrderDerivate.vi"("t_capture"=w4009, "initial condition"=w4007, "x"=w4007) -> ("dx/dt"=w4012:dbl)  [unwired: 5 in, 3 out]
                      n1653 = call "2ndOrderDerivate.vi"("t_capture"=w4009, "initial condition"=w4006, "x"=w4006) -> ("dx/dt"=w4011:dbl)  [unwired: 5 in, 3 out]
                    }
                    frame 2 {
                      n1654 = call "2ndOrderDerivate.vi"("t_capture"=w4016, "initial condition"=w4015, "x"=w4015) -> ("dx/dt"=w4017:dbl)  [unwired: 5 in, 3 out]
                      n1655 = call "2ndOrderDerivate.vi"("t_capture"=w4016, "initial condition"=w4014, "x"=w4014) -> ("dx/dt"=w4019:dbl)  [unwired: 5 in, 3 out]
                      n1656 = call "2ndOrderDerivate.vi"("t_capture"=w4016, "initial condition"=w4013, "x"=w4013) -> ("dx/dt"=w4018:dbl)  [unwired: 5 in, 3 out]
                    }
                    frame 3 {
                      n1657 = call "2ndOrderDerivate.vi"("t_capture"=w4023, "initial condition"=w4022, "x"=w4022) -> ("dx/dt"=w4024:dbl)  [unwired: 5 in, 3 out]
                      n1658 = call "2ndOrderDerivate.vi"("t_capture"=w4023, "initial condition"=w4021, "x"=w4021) -> ("dx/dt"=w4026:dbl)  [unwired: 5 in, 3 out]
                      n1659 = call "2ndOrderDerivate.vi"("t_capture"=w4023, "initial condition"=w4020, "x"=w4020) -> ("dx/dt"=w4025:dbl)  [unwired: 5 in, 3 out]
                    }
                    frame 4 {
                      n1660 = call "2ndOrderDerivate.vi"("t_capture"=w4030, "initial condition"=w4029, "x"=w4029) -> ("dx/dt"=w4031:dbl)  [unwired: 5 in, 3 out]
                      n1661 = call "2ndOrderDerivate.vi"("t_capture"=w4030, "initial condition"=w4028, "x"=w4028) -> ("dx/dt"=w4033:dbl)  [unwired: 5 in, 3 out]
                      n1662 = call "2ndOrderDerivate.vi"("t_capture"=w4030, "initial condition"=w4027, "x"=w4027) -> ("dx/dt"=w4032:dbl)  [unwired: 5 in, 3 out]
                    }
                    frame 5 {
                      n1663 = call "2ndOrderDerivate.vi"("t_capture"=w4037, "initial condition"=w4036, "x"=w4036) -> ("dx/dt"=w4038:dbl)  [unwired: 5 in, 3 out]
                      n1664 = call "2ndOrderDerivate.vi"("t_capture"=w4037, "initial condition"=w4035, "x"=w4035) -> ("dx/dt"=w4040:dbl)  [unwired: 5 in, 3 out]
                      n1665 = call "2ndOrderDerivate.vi"("t_capture"=w4037, "initial condition"=w4034, "x"=w4034) -> ("dx/dt"=w4039:dbl)  [unwired: 5 in, 3 out]
                    }
                    frame 6 {
                      n1666 = call "2ndOrderDerivate.vi"("t_capture"=w4044, "initial condition"=w4043, "x"=w4043) -> ("dx/dt"=w4045:dbl)  [unwired: 5 in, 3 out]
                      n1667 = call "2ndOrderDerivate.vi"("t_capture"=w4044, "initial condition"=w4042, "x"=w4042) -> ("dx/dt"=w4047:dbl)  [unwired: 5 in, 3 out]
                      n1668 = call "2ndOrderDerivate.vi"("t_capture"=w4044, "initial condition"=w4041, "x"=w4041) -> ("dx/dt"=w4046:dbl)  [unwired: 5 in, 3 out]
                    }
                    frame 7 {
                      n1669 = call "2ndOrderDerivate.vi"("t_capture"=w4051, "initial condition"=w4050, "x"=w4050) -> ("dx/dt"=w4052:dbl)  [unwired: 5 in, 3 out]
                      n1670 = call "2ndOrderDerivate.vi"("t_capture"=w4051, "initial condition"=w4049, "x"=w4049) -> ("dx/dt"=w4054:dbl)  [unwired: 5 in, 3 out]
                      n1671 = call "2ndOrderDerivate.vi"("t_capture"=w4051, "initial condition"=w4048, "x"=w4048) -> ("dx/dt"=w4053:dbl)  [unwired: 5 in, 3 out]
                    }
                    frame 8 {
                      n1672 = call "2ndOrderDerivate.vi"("t_capture"=w4058, "initial condition"=w4057, "x"=w4057) -> ("dx/dt"=w4059:dbl)  [unwired: 5 in, 3 out]
                      n1673 = call "2ndOrderDerivate.vi"("t_capture"=w4058, "initial condition"=w4056, "x"=w4056) -> ("dx/dt"=w4061:dbl)  [unwired: 5 in, 3 out]
                      n1674 = call "2ndOrderDerivate.vi"("t_capture"=w4058, "initial condition"=w4055, "x"=w4055) -> ("dx/dt"=w4060:dbl)  [unwired: 5 in, 3 out]
                    }
                    frame 9 {
                      n1675 = call "2ndOrderDerivate.vi"("t_capture"=w4065, "initial condition"=w4064, "x"=w4064) -> ("dx/dt"=w4066:dbl)  [unwired: 5 in, 3 out]
                      n1676 = call "2ndOrderDerivate.vi"("t_capture"=w4065, "initial condition"=w4063, "x"=w4063) -> ("dx/dt"=w4068:dbl)  [unwired: 5 in, 3 out]
                      n1677 = call "2ndOrderDerivate.vi"("t_capture"=w4065, "initial condition"=w4062, "x"=w4062) -> ("dx/dt"=w4067:dbl)  [unwired: 5 in, 3 out]
                    }
                    frame 10 {
                      n1678 = call "2ndOrderDerivate.vi"("t_capture"=w4072, "initial condition"=w4071, "x"=w4071) -> ("dx/dt"=w4073:dbl)  [unwired: 5 in, 3 out]
                      n1679 = call "2ndOrderDerivate.vi"("t_capture"=w4072, "initial condition"=w4070, "x"=w4070) -> ("dx/dt"=w4075:dbl)  [unwired: 5 in, 3 out]
                      n1680 = call "2ndOrderDerivate.vi"("t_capture"=w4072, "initial condition"=w4069, "x"=w4069) -> ("dx/dt"=w4074:dbl)  [unwired: 5 in, 3 out]
                    }
                    frame 11 {
                      n1681 = call "2ndOrderDerivate.vi"("t_capture"=w4079, "initial condition"=w4078, "x"=w4078) -> ("dx/dt"=w4080:dbl)  [unwired: 5 in, 3 out]
                      n1682 = call "2ndOrderDerivate.vi"("t_capture"=w4079, "initial condition"=w4077, "x"=w4077) -> ("dx/dt"=w4082:dbl)  [unwired: 5 in, 3 out]
                      n1683 = call "2ndOrderDerivate.vi"("t_capture"=w4079, "initial condition"=w4076, "x"=w4076) -> ("dx/dt"=w4081:dbl)  [unwired: 5 in, 3 out]
                    }
                    frame 12 {
                      n1684 = call "2ndOrderDerivate.vi"("t_capture"=w4086, "initial condition"=w4085, "x"=w4085) -> ("dx/dt"=w4087:dbl)  [unwired: 5 in, 3 out]
                      n1685 = call "2ndOrderDerivate.vi"("t_capture"=w4086, "initial condition"=w4084, "x"=w4084) -> ("dx/dt"=w4089:dbl)  [unwired: 5 in, 3 out]
                      n1686 = call "2ndOrderDerivate.vi"("t_capture"=w4086, "initial condition"=w4083, "x"=w4083) -> ("dx/dt"=w4088:dbl)  [unwired: 5 in, 3 out]
                    }
                    frame 13 {
                      n1687 = call "2ndOrderDerivate.vi"("t_capture"=w4093, "initial condition"=w4092, "x"=w4092) -> ("dx/dt"=w4094:dbl)  [unwired: 5 in, 3 out]
                      n1688 = call "2ndOrderDerivate.vi"("t_capture"=w4093, "initial condition"=w4091, "x"=w4091) -> ("dx/dt"=w4096:dbl)  [unwired: 5 in, 3 out]
                      n1689 = call "2ndOrderDerivate.vi"("t_capture"=w4093, "initial condition"=w4090, "x"=w4090) -> ("dx/dt"=w4095:dbl)  [unwired: 5 in, 3 out]
                    }
                    frame 14 {
                      n1690 = call "2ndOrderDerivate.vi"("t_capture"=w4100, "initial condition"=w4099, "x"=w4099) -> ("dx/dt"=w4101:dbl)  [unwired: 5 in, 3 out]
                      n1691 = call "2ndOrderDerivate.vi"("t_capture"=w4100, "initial condition"=w4098, "x"=w4098) -> ("dx/dt"=w4103:dbl)  [unwired: 5 in, 3 out]
                      n1692 = call "2ndOrderDerivate.vi"("t_capture"=w4100, "initial condition"=w4097, "x"=w4097) -> ("dx/dt"=w4102:dbl)  [unwired: 5 in, 3 out]
                    }
                    frame 15 {
                      n1693 = call "2ndOrderDerivate.vi"("t_capture"=w4107, "initial condition"=w4106, "x"=w4106) -> ("dx/dt"=w4108:dbl)  [unwired: 5 in, 3 out]
                      n1694 = call "2ndOrderDerivate.vi"("t_capture"=w4107, "initial condition"=w4105, "x"=w4105) -> ("dx/dt"=w4110:dbl)  [unwired: 5 in, 3 out]
                      n1695 = call "2ndOrderDerivate.vi"("t_capture"=w4107, "initial condition"=w4104, "x"=w4104) -> ("dx/dt"=w4109:dbl)  [unwired: 5 in, 3 out]
                    }
                  }
                  n1696 = case shown="0, Default" w3878 {
                    tunnel: w3877 -> [w3889 w3896 w3903 w3910 w3917 w3924 w3931 w3938 w3945 w3952 w3959 w3966 w3973 w3980 w3987 w3994]
                    tunnel: [w3891 w3898 w3905 w3912 w3919 w3926 w3933 w3940 w3947 w3954 w3961 w3968 w3975 w3982 w3989 w3996] -> w3874
                    tunnel: [w3893 w3900 w3907 w3914 w3921 w3928 w3935 w3942 w3949 w3956 w3963 w3970 w3977 w3984 w3991 w3998] -> w3873
                    tunnel: [w3892 w3899 w3906 w3913 w3920 w3927 w3934 w3941 w3948 w3955 w3962 w3969 w3976 w3983 w3990 w3997] -> w3872
                    tunnel: w3876 -> [w3888 w3895 w3902 w3909 w3916 w3923 w3930 w3937 w3944 w3951 w3958 w3965 w3972 w3979 w3986 w3993]
                    tunnel: w3875 -> [w3887 w3894 w3901 w3908 w3915 w3922 w3929 w3936 w3943 w3950 w3957 w3964 w3971 w3978 w3985 w3992]
                    tunnel: w3879 -> [w3890 w3897 w3904 w3911 w3918 w3925 w3932 w3939 w3946 w3953 w3960 w3967 w3974 w3981 w3988 w3995]
                    frame 0, Default {
                      n1697 = call "2ndOrderDerivate.vi"("t_capture"=w3890, "initial condition"=w3889, "x"=w3889) -> ("dx/dt"=w3891:dbl)  [unwired: 5 in, 3 out]
                      n1698 = call "2ndOrderDerivate.vi"("t_capture"=w3890, "initial condition"=w3888, "x"=w3888) -> ("dx/dt"=w3893:dbl)  [unwired: 5 in, 3 out]
                      n1699 = call "2ndOrderDerivate.vi"("t_capture"=w3890, "initial condition"=w3887, "x"=w3887) -> ("dx/dt"=w3892:dbl)  [unwired: 5 in, 3 out]
                    }
                    frame 1 {
                      n1700 = call "2ndOrderDerivate.vi"("t_capture"=w3897, "initial condition"=w3896, "x"=w3896) -> ("dx/dt"=w3898:dbl)  [unwired: 5 in, 3 out]
                      n1701 = call "2ndOrderDerivate.vi"("t_capture"=w3897, "initial condition"=w3895, "x"=w3895) -> ("dx/dt"=w3900:dbl)  [unwired: 5 in, 3 out]
                      n1702 = call "2ndOrderDerivate.vi"("t_capture"=w3897, "initial condition"=w3894, "x"=w3894) -> ("dx/dt"=w3899:dbl)  [unwired: 5 in, 3 out]
                    }
                    frame 2 {
                      n1703 = call "2ndOrderDerivate.vi"("t_capture"=w3904, "initial condition"=w3903, "x"=w3903) -> ("dx/dt"=w3905:dbl)  [unwired: 5 in, 3 out]
                      n1704 = call "2ndOrderDerivate.vi"("t_capture"=w3904, "initial condition"=w3902, "x"=w3902) -> ("dx/dt"=w3907:dbl)  [unwired: 5 in, 3 out]
                      n1705 = call "2ndOrderDerivate.vi"("t_capture"=w3904, "initial condition"=w3901, "x"=w3901) -> ("dx/dt"=w3906:dbl)  [unwired: 5 in, 3 out]
                    }
                    frame 3 {
                      n1706 = call "2ndOrderDerivate.vi"("t_capture"=w3911, "initial condition"=w3910, "x"=w3910) -> ("dx/dt"=w3912:dbl)  [unwired: 5 in, 3 out]
                      n1707 = call "2ndOrderDerivate.vi"("t_capture"=w3911, "initial condition"=w3909, "x"=w3909) -> ("dx/dt"=w3914:dbl)  [unwired: 5 in, 3 out]
                      n1708 = call "2ndOrderDerivate.vi"("t_capture"=w3911, "initial condition"=w3908, "x"=w3908) -> ("dx/dt"=w3913:dbl)  [unwired: 5 in, 3 out]
                    }
                    frame 4 {
                      n1709 = call "2ndOrderDerivate.vi"("t_capture"=w3918, "initial condition"=w3917, "x"=w3917) -> ("dx/dt"=w3919:dbl)  [unwired: 5 in, 3 out]
                      n1710 = call "2ndOrderDerivate.vi"("t_capture"=w3918, "initial condition"=w3916, "x"=w3916) -> ("dx/dt"=w3921:dbl)  [unwired: 5 in, 3 out]
                      n1711 = call "2ndOrderDerivate.vi"("t_capture"=w3918, "initial condition"=w3915, "x"=w3915) -> ("dx/dt"=w3920:dbl)  [unwired: 5 in, 3 out]
                    }
                    frame 5 {
                      n1712 = call "2ndOrderDerivate.vi"("t_capture"=w3925, "initial condition"=w3924, "x"=w3924) -> ("dx/dt"=w3926:dbl)  [unwired: 5 in, 3 out]
                      n1713 = call "2ndOrderDerivate.vi"("t_capture"=w3925, "initial condition"=w3923, "x"=w3923) -> ("dx/dt"=w3928:dbl)  [unwired: 5 in, 3 out]
                      n1714 = call "2ndOrderDerivate.vi"("t_capture"=w3925, "initial condition"=w3922, "x"=w3922) -> ("dx/dt"=w3927:dbl)  [unwired: 5 in, 3 out]
                    }
                    frame 6 {
                      n1715 = call "2ndOrderDerivate.vi"("t_capture"=w3932, "initial condition"=w3931, "x"=w3931) -> ("dx/dt"=w3933:dbl)  [unwired: 5 in, 3 out]
                      n1716 = call "2ndOrderDerivate.vi"("t_capture"=w3932, "initial condition"=w3930, "x"=w3930) -> ("dx/dt"=w3935:dbl)  [unwired: 5 in, 3 out]
                      n1717 = call "2ndOrderDerivate.vi"("t_capture"=w3932, "initial condition"=w3929, "x"=w3929) -> ("dx/dt"=w3934:dbl)  [unwired: 5 in, 3 out]
                    }
                    frame 7 {
                      n1718 = call "2ndOrderDerivate.vi"("t_capture"=w3939, "initial condition"=w3938, "x"=w3938) -> ("dx/dt"=w3940:dbl)  [unwired: 5 in, 3 out]
                      n1719 = call "2ndOrderDerivate.vi"("t_capture"=w3939, "initial condition"=w3937, "x"=w3937) -> ("dx/dt"=w3942:dbl)  [unwired: 5 in, 3 out]
                      n1720 = call "2ndOrderDerivate.vi"("t_capture"=w3939, "initial condition"=w3936, "x"=w3936) -> ("dx/dt"=w3941:dbl)  [unwired: 5 in, 3 out]
                    }
                    frame 8 {
                      n1721 = call "2ndOrderDerivate.vi"("t_capture"=w3946, "initial condition"=w3945, "x"=w3945) -> ("dx/dt"=w3947:dbl)  [unwired: 5 in, 3 out]
                      n1722 = call "2ndOrderDerivate.vi"("t_capture"=w3946, "initial condition"=w3944, "x"=w3944) -> ("dx/dt"=w3949:dbl)  [unwired: 5 in, 3 out]
                      n1723 = call "2ndOrderDerivate.vi"("t_capture"=w3946, "initial condition"=w3943, "x"=w3943) -> ("dx/dt"=w3948:dbl)  [unwired: 5 in, 3 out]
                    }
                    frame 9 {
                      n1724 = call "2ndOrderDerivate.vi"("t_capture"=w3953, "initial condition"=w3952, "x"=w3952) -> ("dx/dt"=w3954:dbl)  [unwired: 5 in, 3 out]
                      n1725 = call "2ndOrderDerivate.vi"("t_capture"=w3953, "initial condition"=w3951, "x"=w3951) -> ("dx/dt"=w3956:dbl)  [unwired: 5 in, 3 out]
                      n1726 = call "2ndOrderDerivate.vi"("t_capture"=w3953, "initial condition"=w3950, "x"=w3950) -> ("dx/dt"=w3955:dbl)  [unwired: 5 in, 3 out]
                    }
                    frame 10 {
                      n1727 = call "2ndOrderDerivate.vi"("t_capture"=w3960, "initial condition"=w3959, "x"=w3959) -> ("dx/dt"=w3961:dbl)  [unwired: 5 in, 3 out]
                      n1728 = call "2ndOrderDerivate.vi"("t_capture"=w3960, "initial condition"=w3958, "x"=w3958) -> ("dx/dt"=w3963:dbl)  [unwired: 5 in, 3 out]
                      n1729 = call "2ndOrderDerivate.vi"("t_capture"=w3960, "initial condition"=w3957, "x"=w3957) -> ("dx/dt"=w3962:dbl)  [unwired: 5 in, 3 out]
                    }
                    frame 11 {
                      n1730 = call "2ndOrderDerivate.vi"("t_capture"=w3967, "initial condition"=w3966, "x"=w3966) -> ("dx/dt"=w3968:dbl)  [unwired: 5 in, 3 out]
                      n1731 = call "2ndOrderDerivate.vi"("t_capture"=w3967, "initial condition"=w3965, "x"=w3965) -> ("dx/dt"=w3970:dbl)  [unwired: 5 in, 3 out]
                      n1732 = call "2ndOrderDerivate.vi"("t_capture"=w3967, "initial condition"=w3964, "x"=w3964) -> ("dx/dt"=w3969:dbl)  [unwired: 5 in, 3 out]
                    }
                    frame 12 {
                      n1733 = call "2ndOrderDerivate.vi"("t_capture"=w3974, "initial condition"=w3973, "x"=w3973) -> ("dx/dt"=w3975:dbl)  [unwired: 5 in, 3 out]
                      n1734 = call "2ndOrderDerivate.vi"("t_capture"=w3974, "initial condition"=w3972, "x"=w3972) -> ("dx/dt"=w3977:dbl)  [unwired: 5 in, 3 out]
                      n1735 = call "2ndOrderDerivate.vi"("t_capture"=w3974, "initial condition"=w3971, "x"=w3971) -> ("dx/dt"=w3976:dbl)  [unwired: 5 in, 3 out]
                    }
                    frame 13 {
                      n1736 = call "2ndOrderDerivate.vi"("t_capture"=w3981, "initial condition"=w3980, "x"=w3980) -> ("dx/dt"=w3982:dbl)  [unwired: 5 in, 3 out]
                      n1737 = call "2ndOrderDerivate.vi"("t_capture"=w3981, "initial condition"=w3979, "x"=w3979) -> ("dx/dt"=w3984:dbl)  [unwired: 5 in, 3 out]
                      n1738 = call "2ndOrderDerivate.vi"("t_capture"=w3981, "initial condition"=w3978, "x"=w3978) -> ("dx/dt"=w3983:dbl)  [unwired: 5 in, 3 out]
                    }
                    frame 14 {
                      n1739 = call "2ndOrderDerivate.vi"("t_capture"=w3988, "initial condition"=w3987, "x"=w3987) -> ("dx/dt"=w3989:dbl)  [unwired: 5 in, 3 out]
                      n1740 = call "2ndOrderDerivate.vi"("t_capture"=w3988, "initial condition"=w3986, "x"=w3986) -> ("dx/dt"=w3991:dbl)  [unwired: 5 in, 3 out]
                      n1741 = call "2ndOrderDerivate.vi"("t_capture"=w3988, "initial condition"=w3985, "x"=w3985) -> ("dx/dt"=w3990:dbl)  [unwired: 5 in, 3 out]
                    }
                    frame 15 {
                      n1742 = call "2ndOrderDerivate.vi"("t_capture"=w3995, "initial condition"=w3994, "x"=w3994) -> ("dx/dt"=w3996:dbl)  [unwired: 5 in, 3 out]
                      n1743 = call "2ndOrderDerivate.vi"("t_capture"=w3995, "initial condition"=w3993, "x"=w3993) -> ("dx/dt"=w3998:dbl)  [unwired: 5 in, 3 out]
                      n1744 = call "2ndOrderDerivate.vi"("t_capture"=w3995, "initial condition"=w3992, "x"=w3992) -> ("dx/dt"=w3997:dbl)  [unwired: 5 in, 3 out]
                    }
                  }
                  n1745 = Build Array(w3881, w3877, w3884, w3876, w3883, w3875, w3874, w3873, w3872) -> (w3886:dbl[])
                  n1746 = call-poly <vilib>:"Array To Matrix.vi"("Real 1D Array"=w3886) -> ("Real Matrix (Column Vector)"=w3885:T3)
                  n1747 = Bundle By Name(cluster=w3880, "x_k|k"=w3885) -> (w3882:T2)
                }
              }
              frame True {
              }
            }
            n1748 = case shown="False" w3851 {
              tunnel: w3850 -> [w4114 w4355]
              tunnel: w3838 -> [w4115 _]
              tunnel: [w4113 w4355] -> w3846
              tunnel: w3836 -> [w4112 _]
              frame False {
                n1749 = for {
                  tunnel: w4114 -> [w4124] mode=indexing
                  tunnel: w4115 -> [_]
                  tunnel: [w4126] -> w4113 mode=indexing
                  tunnel: w4112 -> [w4123]
                  n1750 = Unbundle By Name(w4124) -> ("x"=w4125:sgl, "y"=w4128:sgl, "orientation"=w4127:sgl, "robot_id"=w4122:u32)  [unwired: 1 out]
                  n1751 = case shown="0, Default" w4122 {
                    tunnel: w4125 -> [w4245 w4252 w4259 w4266 w4273 w4280 w4287 w4294 w4301 w4308 w4315 w4322 w4329 w4336 w4343 w4350]
                    tunnel: [w4247 w4254 w4261 w4268 w4275 w4282 w4289 w4296 w4303 w4310 w4317 w4324 w4331 w4338 w4345 w4352] -> w4121
                    tunnel: [w4249 w4256 w4263 w4270 w4277 w4284 w4291 w4298 w4305 w4312 w4319 w4326 w4333 w4340 w4347 w4354] -> w4120
                    tunnel: [w4248 w4255 w4262 w4269 w4276 w4283 w4290 w4297 w4304 w4311 w4318 w4325 w4332 w4339 w4346 w4353] -> w4119
                    tunnel: w4128 -> [w4244 w4251 w4258 w4265 w4272 w4279 w4286 w4293 w4300 w4307 w4314 w4321 w4328 w4335 w4342 w4349]
                    tunnel: w4127 -> [w4243 w4250 w4257 w4264 w4271 w4278 w4285 w4292 w4299 w4306 w4313 w4320 w4327 w4334 w4341 w4348]
                    tunnel: w4123 -> [w4246 w4253 w4260 w4267 w4274 w4281 w4288 w4295 w4302 w4309 w4316 w4323 w4330 w4337 w4344 w4351]
                    frame 0, Default {
                      n1752 = call "2ndOrderDerivate.vi"("t_capture"=w4246, "initial condition"=w4245, "x"=w4245) -> ("dx/dt"=w4247:dbl)  [unwired: 5 in, 3 out]
                      n1753 = call "2ndOrderDerivate.vi"("t_capture"=w4246, "initial condition"=w4244, "x"=w4244) -> ("dx/dt"=w4249:dbl)  [unwired: 5 in, 3 out]
                      n1754 = call "2ndOrderDerivate.vi"("t_capture"=w4246, "initial condition"=w4243, "x"=w4243) -> ("dx/dt"=w4248:dbl)  [unwired: 5 in, 3 out]
                    }
                    frame 1 {
                      n1755 = call "2ndOrderDerivate.vi"("t_capture"=w4253, "initial condition"=w4252, "x"=w4252) -> ("dx/dt"=w4254:dbl)  [unwired: 5 in, 3 out]
                      n1756 = call "2ndOrderDerivate.vi"("t_capture"=w4253, "initial condition"=w4251, "x"=w4251) -> ("dx/dt"=w4256:dbl)  [unwired: 5 in, 3 out]
                      n1757 = call "2ndOrderDerivate.vi"("t_capture"=w4253, "initial condition"=w4250, "x"=w4250) -> ("dx/dt"=w4255:dbl)  [unwired: 5 in, 3 out]
                    }
                    frame 2 {
                      n1758 = call "2ndOrderDerivate.vi"("t_capture"=w4260, "initial condition"=w4259, "x"=w4259) -> ("dx/dt"=w4261:dbl)  [unwired: 5 in, 3 out]
                      n1759 = call "2ndOrderDerivate.vi"("t_capture"=w4260, "initial condition"=w4258, "x"=w4258) -> ("dx/dt"=w4263:dbl)  [unwired: 5 in, 3 out]
                      n1760 = call "2ndOrderDerivate.vi"("t_capture"=w4260, "initial condition"=w4257, "x"=w4257) -> ("dx/dt"=w4262:dbl)  [unwired: 5 in, 3 out]
                    }
                    frame 3 {
                      n1761 = call "2ndOrderDerivate.vi"("t_capture"=w4267, "initial condition"=w4266, "x"=w4266) -> ("dx/dt"=w4268:dbl)  [unwired: 5 in, 3 out]
                      n1762 = call "2ndOrderDerivate.vi"("t_capture"=w4267, "initial condition"=w4265, "x"=w4265) -> ("dx/dt"=w4270:dbl)  [unwired: 5 in, 3 out]
                      n1763 = call "2ndOrderDerivate.vi"("t_capture"=w4267, "initial condition"=w4264, "x"=w4264) -> ("dx/dt"=w4269:dbl)  [unwired: 5 in, 3 out]
                    }
                    frame 4 {
                      n1764 = call "2ndOrderDerivate.vi"("t_capture"=w4274, "initial condition"=w4273, "x"=w4273) -> ("dx/dt"=w4275:dbl)  [unwired: 5 in, 3 out]
                      n1765 = call "2ndOrderDerivate.vi"("t_capture"=w4274, "initial condition"=w4272, "x"=w4272) -> ("dx/dt"=w4277:dbl)  [unwired: 5 in, 3 out]
                      n1766 = call "2ndOrderDerivate.vi"("t_capture"=w4274, "initial condition"=w4271, "x"=w4271) -> ("dx/dt"=w4276:dbl)  [unwired: 5 in, 3 out]
                    }
                    frame 5 {
                      n1767 = call "2ndOrderDerivate.vi"("t_capture"=w4281, "initial condition"=w4280, "x"=w4280) -> ("dx/dt"=w4282:dbl)  [unwired: 5 in, 3 out]
                      n1768 = call "2ndOrderDerivate.vi"("t_capture"=w4281, "initial condition"=w4279, "x"=w4279) -> ("dx/dt"=w4284:dbl)  [unwired: 5 in, 3 out]
                      n1769 = call "2ndOrderDerivate.vi"("t_capture"=w4281, "initial condition"=w4278, "x"=w4278) -> ("dx/dt"=w4283:dbl)  [unwired: 5 in, 3 out]
                    }
                    frame 6 {
                      n1770 = call "2ndOrderDerivate.vi"("t_capture"=w4288, "initial condition"=w4287, "x"=w4287) -> ("dx/dt"=w4289:dbl)  [unwired: 5 in, 3 out]
                      n1771 = call "2ndOrderDerivate.vi"("t_capture"=w4288, "initial condition"=w4286, "x"=w4286) -> ("dx/dt"=w4291:dbl)  [unwired: 5 in, 3 out]
                      n1772 = call "2ndOrderDerivate.vi"("t_capture"=w4288, "initial condition"=w4285, "x"=w4285) -> ("dx/dt"=w4290:dbl)  [unwired: 5 in, 3 out]
                    }
                    frame 7 {
                      n1773 = call "2ndOrderDerivate.vi"("t_capture"=w4295, "initial condition"=w4294, "x"=w4294) -> ("dx/dt"=w4296:dbl)  [unwired: 5 in, 3 out]
                      n1774 = call "2ndOrderDerivate.vi"("t_capture"=w4295, "initial condition"=w4293, "x"=w4293) -> ("dx/dt"=w4298:dbl)  [unwired: 5 in, 3 out]
                      n1775 = call "2ndOrderDerivate.vi"("t_capture"=w4295, "initial condition"=w4292, "x"=w4292) -> ("dx/dt"=w4297:dbl)  [unwired: 5 in, 3 out]
                    }
                    frame 8 {
                      n1776 = call "2ndOrderDerivate.vi"("t_capture"=w4302, "initial condition"=w4301, "x"=w4301) -> ("dx/dt"=w4303:dbl)  [unwired: 5 in, 3 out]
                      n1777 = call "2ndOrderDerivate.vi"("t_capture"=w4302, "initial condition"=w4300, "x"=w4300) -> ("dx/dt"=w4305:dbl)  [unwired: 5 in, 3 out]
                      n1778 = call "2ndOrderDerivate.vi"("t_capture"=w4302, "initial condition"=w4299, "x"=w4299) -> ("dx/dt"=w4304:dbl)  [unwired: 5 in, 3 out]
                    }
                    frame 9 {
                      n1779 = call "2ndOrderDerivate.vi"("t_capture"=w4309, "initial condition"=w4308, "x"=w4308) -> ("dx/dt"=w4310:dbl)  [unwired: 5 in, 3 out]
                      n1780 = call "2ndOrderDerivate.vi"("t_capture"=w4309, "initial condition"=w4307, "x"=w4307) -> ("dx/dt"=w4312:dbl)  [unwired: 5 in, 3 out]
                      n1781 = call "2ndOrderDerivate.vi"("t_capture"=w4309, "initial condition"=w4306, "x"=w4306) -> ("dx/dt"=w4311:dbl)  [unwired: 5 in, 3 out]
                    }
                    frame 10 {
                      n1782 = call "2ndOrderDerivate.vi"("t_capture"=w4316, "initial condition"=w4315, "x"=w4315) -> ("dx/dt"=w4317:dbl)  [unwired: 5 in, 3 out]
                      n1783 = call "2ndOrderDerivate.vi"("t_capture"=w4316, "initial condition"=w4314, "x"=w4314) -> ("dx/dt"=w4319:dbl)  [unwired: 5 in, 3 out]
                      n1784 = call "2ndOrderDerivate.vi"("t_capture"=w4316, "initial condition"=w4313, "x"=w4313) -> ("dx/dt"=w4318:dbl)  [unwired: 5 in, 3 out]
                    }
                    frame 11 {
                      n1785 = call "2ndOrderDerivate.vi"("t_capture"=w4323, "initial condition"=w4322, "x"=w4322) -> ("dx/dt"=w4324:dbl)  [unwired: 5 in, 3 out]
                      n1786 = call "2ndOrderDerivate.vi"("t_capture"=w4323, "initial condition"=w4321, "x"=w4321) -> ("dx/dt"=w4326:dbl)  [unwired: 5 in, 3 out]
                      n1787 = call "2ndOrderDerivate.vi"("t_capture"=w4323, "initial condition"=w4320, "x"=w4320) -> ("dx/dt"=w4325:dbl)  [unwired: 5 in, 3 out]
                    }
                    frame 12 {
                      n1788 = call "2ndOrderDerivate.vi"("t_capture"=w4330, "initial condition"=w4329, "x"=w4329) -> ("dx/dt"=w4331:dbl)  [unwired: 5 in, 3 out]
                      n1789 = call "2ndOrderDerivate.vi"("t_capture"=w4330, "initial condition"=w4328, "x"=w4328) -> ("dx/dt"=w4333:dbl)  [unwired: 5 in, 3 out]
                      n1790 = call "2ndOrderDerivate.vi"("t_capture"=w4330, "initial condition"=w4327, "x"=w4327) -> ("dx/dt"=w4332:dbl)  [unwired: 5 in, 3 out]
                    }
                    frame 13 {
                      n1791 = call "2ndOrderDerivate.vi"("t_capture"=w4337, "initial condition"=w4336, "x"=w4336) -> ("dx/dt"=w4338:dbl)  [unwired: 5 in, 3 out]
                      n1792 = call "2ndOrderDerivate.vi"("t_capture"=w4337, "initial condition"=w4335, "x"=w4335) -> ("dx/dt"=w4340:dbl)  [unwired: 5 in, 3 out]
                      n1793 = call "2ndOrderDerivate.vi"("t_capture"=w4337, "initial condition"=w4334, "x"=w4334) -> ("dx/dt"=w4339:dbl)  [unwired: 5 in, 3 out]
                    }
                    frame 14 {
                      n1794 = call "2ndOrderDerivate.vi"("t_capture"=w4344, "initial condition"=w4343, "x"=w4343) -> ("dx/dt"=w4345:dbl)  [unwired: 5 in, 3 out]
                      n1795 = call "2ndOrderDerivate.vi"("t_capture"=w4344, "initial condition"=w4342, "x"=w4342) -> ("dx/dt"=w4347:dbl)  [unwired: 5 in, 3 out]
                      n1796 = call "2ndOrderDerivate.vi"("t_capture"=w4344, "initial condition"=w4341, "x"=w4341) -> ("dx/dt"=w4346:dbl)  [unwired: 5 in, 3 out]
                    }
                    frame 15 {
                      n1797 = call "2ndOrderDerivate.vi"("t_capture"=w4351, "initial condition"=w4350, "x"=w4350) -> ("dx/dt"=w4352:dbl)  [unwired: 5 in, 3 out]
                      n1798 = call "2ndOrderDerivate.vi"("t_capture"=w4351, "initial condition"=w4349, "x"=w4349) -> ("dx/dt"=w4354:dbl)  [unwired: 5 in, 3 out]
                      n1799 = call "2ndOrderDerivate.vi"("t_capture"=w4351, "initial condition"=w4348, "x"=w4348) -> ("dx/dt"=w4353:dbl)  [unwired: 5 in, 3 out]
                    }
                  }
                  n1800 = case shown="0, Default" w4122 {
                    tunnel: w4121 -> [w4133 w4140 w4147 w4154 w4161 w4168 w4175 w4182 w4189 w4196 w4203 w4210 w4217 w4224 w4231 w4238]
                    tunnel: [w4135 w4142 w4149 w4156 w4163 w4170 w4177 w4184 w4191 w4198 w4205 w4212 w4219 w4226 w4233 w4240] -> w4118
                    tunnel: [w4137 w4144 w4151 w4158 w4165 w4172 w4179 w4186 w4193 w4200 w4207 w4214 w4221 w4228 w4235 w4242] -> w4117
                    tunnel: [w4136 w4143 w4150 w4157 w4164 w4171 w4178 w4185 w4192 w4199 w4206 w4213 w4220 w4227 w4234 w4241] -> w4116
                    tunnel: w4120 -> [w4132 w4139 w4146 w4153 w4160 w4167 w4174 w4181 w4188 w4195 w4202 w4209 w4216 w4223 w4230 w4237]
                    tunnel: w4119 -> [w4131 w4138 w4145 w4152 w4159 w4166 w4173 w4180 w4187 w4194 w4201 w4208 w4215 w4222 w4229 w4236]
                    tunnel: w4123 -> [w4134 w4141 w4148 w4155 w4162 w4169 w4176 w4183 w4190 w4197 w4204 w4211 w4218 w4225 w4232 w4239]
                    frame 0, Default {
                      n1801 = call "2ndOrderDerivate.vi"("t_capture"=w4134, "initial condition"=w4133, "x"=w4133) -> ("dx/dt"=w4135:dbl)  [unwired: 5 in, 3 out]
                      n1802 = call "2ndOrderDerivate.vi"("t_capture"=w4134, "initial condition"=w4132, "x"=w4132) -> ("dx/dt"=w4137:dbl)  [unwired: 5 in, 3 out]
                      n1803 = call "2ndOrderDerivate.vi"("t_capture"=w4134, "initial condition"=w4131, "x"=w4131) -> ("dx/dt"=w4136:dbl)  [unwired: 5 in, 3 out]
                    }
                    frame 1 {
                      n1804 = call "2ndOrderDerivate.vi"("t_capture"=w4141, "initial condition"=w4140, "x"=w4140) -> ("dx/dt"=w4142:dbl)  [unwired: 5 in, 3 out]
                      n1805 = call "2ndOrderDerivate.vi"("t_capture"=w4141, "initial condition"=w4139, "x"=w4139) -> ("dx/dt"=w4144:dbl)  [unwired: 5 in, 3 out]
                      n1806 = call "2ndOrderDerivate.vi"("t_capture"=w4141, "initial condition"=w4138, "x"=w4138) -> ("dx/dt"=w4143:dbl)  [unwired: 5 in, 3 out]
                    }
                    frame 2 {
                      n1807 = call "2ndOrderDerivate.vi"("t_capture"=w4148, "initial condition"=w4147, "x"=w4147) -> ("dx/dt"=w4149:dbl)  [unwired: 5 in, 3 out]
                      n1808 = call "2ndOrderDerivate.vi"("t_capture"=w4148, "initial condition"=w4146, "x"=w4146) -> ("dx/dt"=w4151:dbl)  [unwired: 5 in, 3 out]
                      n1809 = call "2ndOrderDerivate.vi"("t_capture"=w4148, "initial condition"=w4145, "x"=w4145) -> ("dx/dt"=w4150:dbl)  [unwired: 5 in, 3 out]
                    }
                    frame 3 {
                      n1810 = call "2ndOrderDerivate.vi"("t_capture"=w4155, "initial condition"=w4154, "x"=w4154) -> ("dx/dt"=w4156:dbl)  [unwired: 5 in, 3 out]
                      n1811 = call "2ndOrderDerivate.vi"("t_capture"=w4155, "initial condition"=w4153, "x"=w4153) -> ("dx/dt"=w4158:dbl)  [unwired: 5 in, 3 out]
                      n1812 = call "2ndOrderDerivate.vi"("t_capture"=w4155, "initial condition"=w4152, "x"=w4152) -> ("dx/dt"=w4157:dbl)  [unwired: 5 in, 3 out]
                    }
                    frame 4 {
                      n1813 = call "2ndOrderDerivate.vi"("t_capture"=w4162, "initial condition"=w4161, "x"=w4161) -> ("dx/dt"=w4163:dbl)  [unwired: 5 in, 3 out]
                      n1814 = call "2ndOrderDerivate.vi"("t_capture"=w4162, "initial condition"=w4160, "x"=w4160) -> ("dx/dt"=w4165:dbl)  [unwired: 5 in, 3 out]
                      n1815 = call "2ndOrderDerivate.vi"("t_capture"=w4162, "initial condition"=w4159, "x"=w4159) -> ("dx/dt"=w4164:dbl)  [unwired: 5 in, 3 out]
                    }
                    frame 5 {
                      n1816 = call "2ndOrderDerivate.vi"("t_capture"=w4169, "initial condition"=w4168, "x"=w4168) -> ("dx/dt"=w4170:dbl)  [unwired: 5 in, 3 out]
                      n1817 = call "2ndOrderDerivate.vi"("t_capture"=w4169, "initial condition"=w4167, "x"=w4167) -> ("dx/dt"=w4172:dbl)  [unwired: 5 in, 3 out]
                      n1818 = call "2ndOrderDerivate.vi"("t_capture"=w4169, "initial condition"=w4166, "x"=w4166) -> ("dx/dt"=w4171:dbl)  [unwired: 5 in, 3 out]
                    }
                    frame 6 {
                      n1819 = call "2ndOrderDerivate.vi"("t_capture"=w4176, "initial condition"=w4175, "x"=w4175) -> ("dx/dt"=w4177:dbl)  [unwired: 5 in, 3 out]
                      n1820 = call "2ndOrderDerivate.vi"("t_capture"=w4176, "initial condition"=w4174, "x"=w4174) -> ("dx/dt"=w4179:dbl)  [unwired: 5 in, 3 out]
                      n1821 = call "2ndOrderDerivate.vi"("t_capture"=w4176, "initial condition"=w4173, "x"=w4173) -> ("dx/dt"=w4178:dbl)  [unwired: 5 in, 3 out]
                    }
                    frame 7 {
                      n1822 = call "2ndOrderDerivate.vi"("t_capture"=w4183, "initial condition"=w4182, "x"=w4182) -> ("dx/dt"=w4184:dbl)  [unwired: 5 in, 3 out]
                      n1823 = call "2ndOrderDerivate.vi"("t_capture"=w4183, "initial condition"=w4181, "x"=w4181) -> ("dx/dt"=w4186:dbl)  [unwired: 5 in, 3 out]
                      n1824 = call "2ndOrderDerivate.vi"("t_capture"=w4183, "initial condition"=w4180, "x"=w4180) -> ("dx/dt"=w4185:dbl)  [unwired: 5 in, 3 out]
                    }
                    frame 8 {
                      n1825 = call "2ndOrderDerivate.vi"("t_capture"=w4190, "initial condition"=w4189, "x"=w4189) -> ("dx/dt"=w4191:dbl)  [unwired: 5 in, 3 out]
                      n1826 = call "2ndOrderDerivate.vi"("t_capture"=w4190, "initial condition"=w4188, "x"=w4188) -> ("dx/dt"=w4193:dbl)  [unwired: 5 in, 3 out]
                      n1827 = call "2ndOrderDerivate.vi"("t_capture"=w4190, "initial condition"=w4187, "x"=w4187) -> ("dx/dt"=w4192:dbl)  [unwired: 5 in, 3 out]
                    }
                    frame 9 {
                      n1828 = call "2ndOrderDerivate.vi"("t_capture"=w4197, "initial condition"=w4196, "x"=w4196) -> ("dx/dt"=w4198:dbl)  [unwired: 5 in, 3 out]
                      n1829 = call "2ndOrderDerivate.vi"("t_capture"=w4197, "initial condition"=w4195, "x"=w4195) -> ("dx/dt"=w4200:dbl)  [unwired: 5 in, 3 out]
                      n1830 = call "2ndOrderDerivate.vi"("t_capture"=w4197, "initial condition"=w4194, "x"=w4194) -> ("dx/dt"=w4199:dbl)  [unwired: 5 in, 3 out]
                    }
                    frame 10 {
                      n1831 = call "2ndOrderDerivate.vi"("t_capture"=w4204, "initial condition"=w4203, "x"=w4203) -> ("dx/dt"=w4205:dbl)  [unwired: 5 in, 3 out]
                      n1832 = call "2ndOrderDerivate.vi"("t_capture"=w4204, "initial condition"=w4202, "x"=w4202) -> ("dx/dt"=w4207:dbl)  [unwired: 5 in, 3 out]
                      n1833 = call "2ndOrderDerivate.vi"("t_capture"=w4204, "initial condition"=w4201, "x"=w4201) -> ("dx/dt"=w4206:dbl)  [unwired: 5 in, 3 out]
                    }
                    frame 11 {
                      n1834 = call "2ndOrderDerivate.vi"("t_capture"=w4211, "initial condition"=w4210, "x"=w4210) -> ("dx/dt"=w4212:dbl)  [unwired: 5 in, 3 out]
                      n1835 = call "2ndOrderDerivate.vi"("t_capture"=w4211, "initial condition"=w4209, "x"=w4209) -> ("dx/dt"=w4214:dbl)  [unwired: 5 in, 3 out]
                      n1836 = call "2ndOrderDerivate.vi"("t_capture"=w4211, "initial condition"=w4208, "x"=w4208) -> ("dx/dt"=w4213:dbl)  [unwired: 5 in, 3 out]
                    }
                    frame 12 {
                      n1837 = call "2ndOrderDerivate.vi"("t_capture"=w4218, "initial condition"=w4217, "x"=w4217) -> ("dx/dt"=w4219:dbl)  [unwired: 5 in, 3 out]
                      n1838 = call "2ndOrderDerivate.vi"("t_capture"=w4218, "initial condition"=w4216, "x"=w4216) -> ("dx/dt"=w4221:dbl)  [unwired: 5 in, 3 out]
                      n1839 = call "2ndOrderDerivate.vi"("t_capture"=w4218, "initial condition"=w4215, "x"=w4215) -> ("dx/dt"=w4220:dbl)  [unwired: 5 in, 3 out]
                    }
                    frame 13 {
                      n1840 = call "2ndOrderDerivate.vi"("t_capture"=w4225, "initial condition"=w4224, "x"=w4224) -> ("dx/dt"=w4226:dbl)  [unwired: 5 in, 3 out]
                      n1841 = call "2ndOrderDerivate.vi"("t_capture"=w4225, "initial condition"=w4223, "x"=w4223) -> ("dx/dt"=w4228:dbl)  [unwired: 5 in, 3 out]
                      n1842 = call "2ndOrderDerivate.vi"("t_capture"=w4225, "initial condition"=w4222, "x"=w4222) -> ("dx/dt"=w4227:dbl)  [unwired: 5 in, 3 out]
                    }
                    frame 14 {
                      n1843 = call "2ndOrderDerivate.vi"("t_capture"=w4232, "initial condition"=w4231, "x"=w4231) -> ("dx/dt"=w4233:dbl)  [unwired: 5 in, 3 out]
                      n1844 = call "2ndOrderDerivate.vi"("t_capture"=w4232, "initial condition"=w4230, "x"=w4230) -> ("dx/dt"=w4235:dbl)  [unwired: 5 in, 3 out]
                      n1845 = call "2ndOrderDerivate.vi"("t_capture"=w4232, "initial condition"=w4229, "x"=w4229) -> ("dx/dt"=w4234:dbl)  [unwired: 5 in, 3 out]
                    }
                    frame 15 {
                      n1846 = call "2ndOrderDerivate.vi"("t_capture"=w4239, "initial condition"=w4238, "x"=w4238) -> ("dx/dt"=w4240:dbl)  [unwired: 5 in, 3 out]
                      n1847 = call "2ndOrderDerivate.vi"("t_capture"=w4239, "initial condition"=w4237, "x"=w4237) -> ("dx/dt"=w4242:dbl)  [unwired: 5 in, 3 out]
                      n1848 = call "2ndOrderDerivate.vi"("t_capture"=w4239, "initial condition"=w4236, "x"=w4236) -> ("dx/dt"=w4241:dbl)  [unwired: 5 in, 3 out]
                    }
                  }
                  n1849 = Build Array(w4125, w4121, w4128, w4120, w4127, w4119, w4118, w4117, w4116) -> (w4130:dbl[])
                  n1850 = call-poly <vilib>:"Array To Matrix.vi"("Real 1D Array"=w4130) -> ("Real Matrix (Column Vector)"=w4129:T3)
                  n1851 = Bundle By Name(cluster=w4124, "x_k|k"=w4129) -> (w4126:T2)
                }
              }
              frame True {
              }
            }
            n1852 = Bundle By Name(cluster=w3841, "robots_blue"=w3846, "robots_yellow"=w3845, "balls"=w3837) -> (w3844:T1)
            n1853 = Bundle By Name(cluster=w3841, "New"=FALSE) -> (w3842:T1)
          }
          frame 2 {
            n1854 = Empty Array?(array=w4359) -> (empty?=w4360:bool)
            n1855 = Empty Array?(array=w4367) -> (empty?=w4368:bool)
            n1856 = Reciprocal(x=w4369) -> (1/x=w4358:dbl)
            n1857 = Empty Array?(array=w4370) -> (empty?=w4371:bool)
            n1858 = case shown="False" w4360 {
              tunnel: w4359 -> [w4374 w4391]
              tunnel: w4358 -> [w4375 _]
              tunnel: [w4373 w4391] -> w4357
              tunnel: w4356 -> [w4372 _]
              frame False {
                n1859 = for {
                  tunnel: w4374 -> [w4390] mode=indexing
                  tunnel: w4375 -> [_]
                  tunnel: w4374 -> [w4389] mode=indexing
                  tunnel: [w4387] -> w4373 mode=indexing
                  tunnel: w4372 -> [w4380]
                  n1860 = Unbundle By Name(w4390) -> ("x"=w4385:sgl, "y"=w4383:sgl, "z"=w4381:sgl)
                  n1861 = call "2ndOrderDerivate.vi"("t_capture"=w4380, "initial condition"=w4385, "x"=w4385) -> ("dx/dt"=w4384:dbl)  [unwired: 5 in, 3 out]
                  n1862 = call "2ndOrderDerivate.vi"("t_capture"=w4380, "initial condition"=w4383, "x"=w4383) -> ("dx/dt"=w4382:dbl)  [unwired: 5 in, 3 out]
                  n1863 = call "2ndOrderDerivate.vi"("t_capture"=w4380, "initial condition"=w4381, "x"=w4381) -> ("dx/dt"=w4386:dbl)  [unwired: 5 in, 3 out]
                  n1864 = call "2ndOrderDerivate.vi"("t_capture"=w4380, "initial condition"=w4384, "x"=w4384) -> ("dx/dt"=w4379:dbl)  [unwired: 5 in, 3 out]
                  n1865 = call "2ndOrderDerivate.vi"("t_capture"=w4380, "initial condition"=w4382, "x"=w4382) -> ()  [unwired: 5 in, 4 out]
                  n1866 = call "2ndOrderDerivate.vi"("t_capture"=w4380, "initial condition"=w4386, "x"=w4386) -> ("dx/dt"=w4378:dbl)  [unwired: 5 in, 3 out]
                  n1867 = Build Array(w4385, w4384, w4383, w4382, w4381, w4380, w4379, 2.0 ("element"), w4378) -> (w4377:dbl[])
                  n1868 = call-poly <vilib>:"Array To Matrix.vi"("Real 1D Array"=w4377) -> ("Real Matrix (Column Vector)"=w4388:T3)
                  n1869 = Bundle By Name(cluster=w4389, "x_k|k"=w4388) -> (w4387:T4)
                }
              }
              frame True {
              }
            }
            n1870 = case shown="False" w4368 {
              tunnel: w4367 -> [w4393 w4634]
              tunnel: w4358 -> [_ _]
              tunnel: [w4394 w4634] -> w4365
              tunnel: w4356 -> [w4392 _]
              frame False {
                n1871 = for {
                  tunnel: w4393 -> [w4403] mode=indexing
                  tunnel: [w4405] -> w4394 mode=indexing
                  tunnel: w4392 -> [w4402]
                  n1872 = Unbundle By Name(w4403) -> ("x"=w4404:sgl, "y"=w4407:sgl, "orientation"=w4406:sgl, "robot_id"=w4401:u32)  [unwired: 1 out]
                  n1873 = case shown="0, Default" w4401 {
                    tunnel: w4404 -> [w4524 w4531 w4538 w4545 w4552 w4559 w4566 w4573 w4580 w4587 w4594 w4601 w4608 w4615 w4622 w4629]
                    tunnel: [w4526 w4533 w4540 w4547 w4554 w4561 w4568 w4575 w4582 w4589 w4596 w4603 w4610 w4617 w4624 w4631] -> w4400
                    tunnel: [w4528 w4535 w4542 w4549 w4556 w4563 w4570 w4577 w4584 w4591 w4598 w4605 w4612 w4619 w4626 w4633] -> w4399
                    tunnel: [w4527 w4534 w4541 w4548 w4555 w4562 w4569 w4576 w4583 w4590 w4597 w4604 w4611 w4618 w4625 w4632] -> w4398
                    tunnel: w4407 -> [w4523 w4530 w4537 w4544 w4551 w4558 w4565 w4572 w4579 w4586 w4593 w4600 w4607 w4614 w4621 w4628]
                    tunnel: w4406 -> [w4522 w4529 w4536 w4543 w4550 w4557 w4564 w4571 w4578 w4585 w4592 w4599 w4606 w4613 w4620 w4627]
                    tunnel: w4402 -> [w4525 w4532 w4539 w4546 w4553 w4560 w4567 w4574 w4581 w4588 w4595 w4602 w4609 w4616 w4623 w4630]
                    frame 0, Default {
                      n1874 = call "2ndOrderDerivate.vi"("t_capture"=w4525, "initial condition"=w4524, "x"=w4524) -> ("dx/dt"=w4526:dbl)  [unwired: 5 in, 3 out]
                      n1875 = call "2ndOrderDerivate.vi"("t_capture"=w4525, "initial condition"=w4523, "x"=w4523) -> ("dx/dt"=w4528:dbl)  [unwired: 5 in, 3 out]
                      n1876 = call "2ndOrderDerivate.vi"("t_capture"=w4525, "initial condition"=w4522, "x"=w4522) -> ("dx/dt"=w4527:dbl)  [unwired: 5 in, 3 out]
                    }
                    frame 1 {
                      n1877 = call "2ndOrderDerivate.vi"("t_capture"=w4532, "initial condition"=w4531, "x"=w4531) -> ("dx/dt"=w4533:dbl)  [unwired: 5 in, 3 out]
                      n1878 = call "2ndOrderDerivate.vi"("t_capture"=w4532, "initial condition"=w4530, "x"=w4530) -> ("dx/dt"=w4535:dbl)  [unwired: 5 in, 3 out]
                      n1879 = call "2ndOrderDerivate.vi"("t_capture"=w4532, "initial condition"=w4529, "x"=w4529) -> ("dx/dt"=w4534:dbl)  [unwired: 5 in, 3 out]
                    }
                    frame 2 {
                      n1880 = call "2ndOrderDerivate.vi"("t_capture"=w4539, "initial condition"=w4538, "x"=w4538) -> ("dx/dt"=w4540:dbl)  [unwired: 5 in, 3 out]
                      n1881 = call "2ndOrderDerivate.vi"("t_capture"=w4539, "initial condition"=w4537, "x"=w4537) -> ("dx/dt"=w4542:dbl)  [unwired: 5 in, 3 out]
                      n1882 = call "2ndOrderDerivate.vi"("t_capture"=w4539, "initial condition"=w4536, "x"=w4536) -> ("dx/dt"=w4541:dbl)  [unwired: 5 in, 3 out]
                    }
                    frame 3 {
                      n1883 = call "2ndOrderDerivate.vi"("t_capture"=w4546, "initial condition"=w4545, "x"=w4545) -> ("dx/dt"=w4547:dbl)  [unwired: 5 in, 3 out]
                      n1884 = call "2ndOrderDerivate.vi"("t_capture"=w4546, "initial condition"=w4544, "x"=w4544) -> ("dx/dt"=w4549:dbl)  [unwired: 5 in, 3 out]
                      n1885 = call "2ndOrderDerivate.vi"("t_capture"=w4546, "initial condition"=w4543, "x"=w4543) -> ("dx/dt"=w4548:dbl)  [unwired: 5 in, 3 out]
                    }
                    frame 4 {
                      n1886 = call "2ndOrderDerivate.vi"("t_capture"=w4553, "initial condition"=w4552, "x"=w4552) -> ("dx/dt"=w4554:dbl)  [unwired: 5 in, 3 out]
                      n1887 = call "2ndOrderDerivate.vi"("t_capture"=w4553, "initial condition"=w4551, "x"=w4551) -> ("dx/dt"=w4556:dbl)  [unwired: 5 in, 3 out]
                      n1888 = call "2ndOrderDerivate.vi"("t_capture"=w4553, "initial condition"=w4550, "x"=w4550) -> ("dx/dt"=w4555:dbl)  [unwired: 5 in, 3 out]
                    }
                    frame 5 {
                      n1889 = call "2ndOrderDerivate.vi"("t_capture"=w4560, "initial condition"=w4559, "x"=w4559) -> ("dx/dt"=w4561:dbl)  [unwired: 5 in, 3 out]
                      n1890 = call "2ndOrderDerivate.vi"("t_capture"=w4560, "initial condition"=w4558, "x"=w4558) -> ("dx/dt"=w4563:dbl)  [unwired: 5 in, 3 out]
                      n1891 = call "2ndOrderDerivate.vi"("t_capture"=w4560, "initial condition"=w4557, "x"=w4557) -> ("dx/dt"=w4562:dbl)  [unwired: 5 in, 3 out]
                    }
                    frame 6 {
                      n1892 = call "2ndOrderDerivate.vi"("t_capture"=w4567, "initial condition"=w4566, "x"=w4566) -> ("dx/dt"=w4568:dbl)  [unwired: 5 in, 3 out]
                      n1893 = call "2ndOrderDerivate.vi"("t_capture"=w4567, "initial condition"=w4565, "x"=w4565) -> ("dx/dt"=w4570:dbl)  [unwired: 5 in, 3 out]
                      n1894 = call "2ndOrderDerivate.vi"("t_capture"=w4567, "initial condition"=w4564, "x"=w4564) -> ("dx/dt"=w4569:dbl)  [unwired: 5 in, 3 out]
                    }
                    frame 7 {
                      n1895 = call "2ndOrderDerivate.vi"("t_capture"=w4574, "initial condition"=w4573, "x"=w4573) -> ("dx/dt"=w4575:dbl)  [unwired: 5 in, 3 out]
                      n1896 = call "2ndOrderDerivate.vi"("t_capture"=w4574, "initial condition"=w4572, "x"=w4572) -> ("dx/dt"=w4577:dbl)  [unwired: 5 in, 3 out]
                      n1897 = call "2ndOrderDerivate.vi"("t_capture"=w4574, "initial condition"=w4571, "x"=w4571) -> ("dx/dt"=w4576:dbl)  [unwired: 5 in, 3 out]
                    }
                    frame 8 {
                      n1898 = call "2ndOrderDerivate.vi"("t_capture"=w4581, "initial condition"=w4580, "x"=w4580) -> ("dx/dt"=w4582:dbl)  [unwired: 5 in, 3 out]
                      n1899 = call "2ndOrderDerivate.vi"("t_capture"=w4581, "initial condition"=w4579, "x"=w4579) -> ("dx/dt"=w4584:dbl)  [unwired: 5 in, 3 out]
                      n1900 = call "2ndOrderDerivate.vi"("t_capture"=w4581, "initial condition"=w4578, "x"=w4578) -> ("dx/dt"=w4583:dbl)  [unwired: 5 in, 3 out]
                    }
                    frame 9 {
                      n1901 = call "2ndOrderDerivate.vi"("t_capture"=w4588, "initial condition"=w4587, "x"=w4587) -> ("dx/dt"=w4589:dbl)  [unwired: 5 in, 3 out]
                      n1902 = call "2ndOrderDerivate.vi"("t_capture"=w4588, "initial condition"=w4586, "x"=w4586) -> ("dx/dt"=w4591:dbl)  [unwired: 5 in, 3 out]
                      n1903 = call "2ndOrderDerivate.vi"("t_capture"=w4588, "initial condition"=w4585, "x"=w4585) -> ("dx/dt"=w4590:dbl)  [unwired: 5 in, 3 out]
                    }
                    frame 10 {
                      n1904 = call "2ndOrderDerivate.vi"("t_capture"=w4595, "initial condition"=w4594, "x"=w4594) -> ("dx/dt"=w4596:dbl)  [unwired: 5 in, 3 out]
                      n1905 = call "2ndOrderDerivate.vi"("t_capture"=w4595, "initial condition"=w4593, "x"=w4593) -> ("dx/dt"=w4598:dbl)  [unwired: 5 in, 3 out]
                      n1906 = call "2ndOrderDerivate.vi"("t_capture"=w4595, "initial condition"=w4592, "x"=w4592) -> ("dx/dt"=w4597:dbl)  [unwired: 5 in, 3 out]
                    }
                    frame 11 {
                      n1907 = call "2ndOrderDerivate.vi"("t_capture"=w4602, "initial condition"=w4601, "x"=w4601) -> ("dx/dt"=w4603:dbl)  [unwired: 5 in, 3 out]
                      n1908 = call "2ndOrderDerivate.vi"("t_capture"=w4602, "initial condition"=w4600, "x"=w4600) -> ("dx/dt"=w4605:dbl)  [unwired: 5 in, 3 out]
                      n1909 = call "2ndOrderDerivate.vi"("t_capture"=w4602, "initial condition"=w4599, "x"=w4599) -> ("dx/dt"=w4604:dbl)  [unwired: 5 in, 3 out]
                    }
                    frame 12 {
                      n1910 = call "2ndOrderDerivate.vi"("t_capture"=w4609, "initial condition"=w4608, "x"=w4608) -> ("dx/dt"=w4610:dbl)  [unwired: 5 in, 3 out]
                      n1911 = call "2ndOrderDerivate.vi"("t_capture"=w4609, "initial condition"=w4607, "x"=w4607) -> ("dx/dt"=w4612:dbl)  [unwired: 5 in, 3 out]
                      n1912 = call "2ndOrderDerivate.vi"("t_capture"=w4609, "initial condition"=w4606, "x"=w4606) -> ("dx/dt"=w4611:dbl)  [unwired: 5 in, 3 out]
                    }
                    frame 13 {
                      n1913 = call "2ndOrderDerivate.vi"("t_capture"=w4616, "initial condition"=w4615, "x"=w4615) -> ("dx/dt"=w4617:dbl)  [unwired: 5 in, 3 out]
                      n1914 = call "2ndOrderDerivate.vi"("t_capture"=w4616, "initial condition"=w4614, "x"=w4614) -> ("dx/dt"=w4619:dbl)  [unwired: 5 in, 3 out]
                      n1915 = call "2ndOrderDerivate.vi"("t_capture"=w4616, "initial condition"=w4613, "x"=w4613) -> ("dx/dt"=w4618:dbl)  [unwired: 5 in, 3 out]
                    }
                    frame 14 {
                      n1916 = call "2ndOrderDerivate.vi"("t_capture"=w4623, "initial condition"=w4622, "x"=w4622) -> ("dx/dt"=w4624:dbl)  [unwired: 5 in, 3 out]
                      n1917 = call "2ndOrderDerivate.vi"("t_capture"=w4623, "initial condition"=w4621, "x"=w4621) -> ("dx/dt"=w4626:dbl)  [unwired: 5 in, 3 out]
                      n1918 = call "2ndOrderDerivate.vi"("t_capture"=w4623, "initial condition"=w4620, "x"=w4620) -> ("dx/dt"=w4625:dbl)  [unwired: 5 in, 3 out]
                    }
                    frame 15 {
                      n1919 = call "2ndOrderDerivate.vi"("t_capture"=w4630, "initial condition"=w4629, "x"=w4629) -> ("dx/dt"=w4631:dbl)  [unwired: 5 in, 3 out]
                      n1920 = call "2ndOrderDerivate.vi"("t_capture"=w4630, "initial condition"=w4628, "x"=w4628) -> ("dx/dt"=w4633:dbl)  [unwired: 5 in, 3 out]
                      n1921 = call "2ndOrderDerivate.vi"("t_capture"=w4630, "initial condition"=w4627, "x"=w4627) -> ("dx/dt"=w4632:dbl)  [unwired: 5 in, 3 out]
                    }
                  }
                  n1922 = case shown="0, Default" w4401 {
                    tunnel: w4400 -> [w4412 w4419 w4426 w4433 w4440 w4447 w4454 w4461 w4468 w4475 w4482 w4489 w4496 w4503 w4510 w4517]
                    tunnel: [w4414 w4421 w4428 w4435 w4442 w4449 w4456 w4463 w4470 w4477 w4484 w4491 w4498 w4505 w4512 w4519] -> w4397
                    tunnel: [w4416 w4423 w4430 w4437 w4444 w4451 w4458 w4465 w4472 w4479 w4486 w4493 w4500 w4507 w4514 w4521] -> w4396
                    tunnel: [w4415 w4422 w4429 w4436 w4443 w4450 w4457 w4464 w4471 w4478 w4485 w4492 w4499 w4506 w4513 w4520] -> w4395
                    tunnel: w4399 -> [w4411 w4418 w4425 w4432 w4439 w4446 w4453 w4460 w4467 w4474 w4481 w4488 w4495 w4502 w4509 w4516]
                    tunnel: w4398 -> [w4410 w4417 w4424 w4431 w4438 w4445 w4452 w4459 w4466 w4473 w4480 w4487 w4494 w4501 w4508 w4515]
                    tunnel: w4402 -> [w4413 w4420 w4427 w4434 w4441 w4448 w4455 w4462 w4469 w4476 w4483 w4490 w4497 w4504 w4511 w4518]
                    frame 0, Default {
                      n1923 = call "2ndOrderDerivate.vi"("t_capture"=w4413, "initial condition"=w4412, "x"=w4412) -> ("dx/dt"=w4414:dbl)  [unwired: 5 in, 3 out]
                      n1924 = call "2ndOrderDerivate.vi"("t_capture"=w4413, "initial condition"=w4411, "x"=w4411) -> ("dx/dt"=w4416:dbl)  [unwired: 5 in, 3 out]
                      n1925 = call "2ndOrderDerivate.vi"("t_capture"=w4413, "initial condition"=w4410, "x"=w4410) -> ("dx/dt"=w4415:dbl)  [unwired: 5 in, 3 out]
                    }
                    frame 1 {
                      n1926 = call "2ndOrderDerivate.vi"("t_capture"=w4420, "initial condition"=w4419, "x"=w4419) -> ("dx/dt"=w4421:dbl)  [unwired: 5 in, 3 out]
                      n1927 = call "2ndOrderDerivate.vi"("t_capture"=w4420, "initial condition"=w4418, "x"=w4418) -> ("dx/dt"=w4423:dbl)  [unwired: 5 in, 3 out]
                      n1928 = call "2ndOrderDerivate.vi"("t_capture"=w4420, "initial condition"=w4417, "x"=w4417) -> ("dx/dt"=w4422:dbl)  [unwired: 5 in, 3 out]
                    }
                    frame 2 {
                      n1929 = call "2ndOrderDerivate.vi"("t_capture"=w4427, "initial condition"=w4426, "x"=w4426) -> ("dx/dt"=w4428:dbl)  [unwired: 5 in, 3 out]
                      n1930 = call "2ndOrderDerivate.vi"("t_capture"=w4427, "initial condition"=w4425, "x"=w4425) -> ("dx/dt"=w4430:dbl)  [unwired: 5 in, 3 out]
                      n1931 = call "2ndOrderDerivate.vi"("t_capture"=w4427, "initial condition"=w4424, "x"=w4424) -> ("dx/dt"=w4429:dbl)  [unwired: 5 in, 3 out]
                    }
                    frame 3 {
                      n1932 = call "2ndOrderDerivate.vi"("t_capture"=w4434, "initial condition"=w4433, "x"=w4433) -> ("dx/dt"=w4435:dbl)  [unwired: 5 in, 3 out]
                      n1933 = call "2ndOrderDerivate.vi"("t_capture"=w4434, "initial condition"=w4432, "x"=w4432) -> ("dx/dt"=w4437:dbl)  [unwired: 5 in, 3 out]
                      n1934 = call "2ndOrderDerivate.vi"("t_capture"=w4434, "initial condition"=w4431, "x"=w4431) -> ("dx/dt"=w4436:dbl)  [unwired: 5 in, 3 out]
                    }
                    frame 4 {
                      n1935 = call "2ndOrderDerivate.vi"("t_capture"=w4441, "initial condition"=w4440, "x"=w4440) -> ("dx/dt"=w4442:dbl)  [unwired: 5 in, 3 out]
                      n1936 = call "2ndOrderDerivate.vi"("t_capture"=w4441, "initial condition"=w4439, "x"=w4439) -> ("dx/dt"=w4444:dbl)  [unwired: 5 in, 3 out]
                      n1937 = call "2ndOrderDerivate.vi"("t_capture"=w4441, "initial condition"=w4438, "x"=w4438) -> ("dx/dt"=w4443:dbl)  [unwired: 5 in, 3 out]
                    }
                    frame 5 {
                      n1938 = call "2ndOrderDerivate.vi"("t_capture"=w4448, "initial condition"=w4447, "x"=w4447) -> ("dx/dt"=w4449:dbl)  [unwired: 5 in, 3 out]
                      n1939 = call "2ndOrderDerivate.vi"("t_capture"=w4448, "initial condition"=w4446, "x"=w4446) -> ("dx/dt"=w4451:dbl)  [unwired: 5 in, 3 out]
                      n1940 = call "2ndOrderDerivate.vi"("t_capture"=w4448, "initial condition"=w4445, "x"=w4445) -> ("dx/dt"=w4450:dbl)  [unwired: 5 in, 3 out]
                    }
                    frame 6 {
                      n1941 = call "2ndOrderDerivate.vi"("t_capture"=w4455, "initial condition"=w4454, "x"=w4454) -> ("dx/dt"=w4456:dbl)  [unwired: 5 in, 3 out]
                      n1942 = call "2ndOrderDerivate.vi"("t_capture"=w4455, "initial condition"=w4453, "x"=w4453) -> ("dx/dt"=w4458:dbl)  [unwired: 5 in, 3 out]
                      n1943 = call "2ndOrderDerivate.vi"("t_capture"=w4455, "initial condition"=w4452, "x"=w4452) -> ("dx/dt"=w4457:dbl)  [unwired: 5 in, 3 out]
                    }
                    frame 7 {
                      n1944 = call "2ndOrderDerivate.vi"("t_capture"=w4462, "initial condition"=w4461, "x"=w4461) -> ("dx/dt"=w4463:dbl)  [unwired: 5 in, 3 out]
                      n1945 = call "2ndOrderDerivate.vi"("t_capture"=w4462, "initial condition"=w4460, "x"=w4460) -> ("dx/dt"=w4465:dbl)  [unwired: 5 in, 3 out]
                      n1946 = call "2ndOrderDerivate.vi"("t_capture"=w4462, "initial condition"=w4459, "x"=w4459) -> ("dx/dt"=w4464:dbl)  [unwired: 5 in, 3 out]
                    }
                    frame 8 {
                      n1947 = call "2ndOrderDerivate.vi"("t_capture"=w4469, "initial condition"=w4468, "x"=w4468) -> ("dx/dt"=w4470:dbl)  [unwired: 5 in, 3 out]
                      n1948 = call "2ndOrderDerivate.vi"("t_capture"=w4469, "initial condition"=w4467, "x"=w4467) -> ("dx/dt"=w4472:dbl)  [unwired: 5 in, 3 out]
                      n1949 = call "2ndOrderDerivate.vi"("t_capture"=w4469, "initial condition"=w4466, "x"=w4466) -> ("dx/dt"=w4471:dbl)  [unwired: 5 in, 3 out]
                    }
                    frame 9 {
                      n1950 = call "2ndOrderDerivate.vi"("t_capture"=w4476, "initial condition"=w4475, "x"=w4475) -> ("dx/dt"=w4477:dbl)  [unwired: 5 in, 3 out]
                      n1951 = call "2ndOrderDerivate.vi"("t_capture"=w4476, "initial condition"=w4474, "x"=w4474) -> ("dx/dt"=w4479:dbl)  [unwired: 5 in, 3 out]
                      n1952 = call "2ndOrderDerivate.vi"("t_capture"=w4476, "initial condition"=w4473, "x"=w4473) -> ("dx/dt"=w4478:dbl)  [unwired: 5 in, 3 out]
                    }
                    frame 10 {
                      n1953 = call "2ndOrderDerivate.vi"("t_capture"=w4483, "initial condition"=w4482, "x"=w4482) -> ("dx/dt"=w4484:dbl)  [unwired: 5 in, 3 out]
                      n1954 = call "2ndOrderDerivate.vi"("t_capture"=w4483, "initial condition"=w4481, "x"=w4481) -> ("dx/dt"=w4486:dbl)  [unwired: 5 in, 3 out]
                      n1955 = call "2ndOrderDerivate.vi"("t_capture"=w4483, "initial condition"=w4480, "x"=w4480) -> ("dx/dt"=w4485:dbl)  [unwired: 5 in, 3 out]
                    }
                    frame 11 {
                      n1956 = call "2ndOrderDerivate.vi"("t_capture"=w4490, "initial condition"=w4489, "x"=w4489) -> ("dx/dt"=w4491:dbl)  [unwired: 5 in, 3 out]
                      n1957 = call "2ndOrderDerivate.vi"("t_capture"=w4490, "initial condition"=w4488, "x"=w4488) -> ("dx/dt"=w4493:dbl)  [unwired: 5 in, 3 out]
                      n1958 = call "2ndOrderDerivate.vi"("t_capture"=w4490, "initial condition"=w4487, "x"=w4487) -> ("dx/dt"=w4492:dbl)  [unwired: 5 in, 3 out]
                    }
                    frame 12 {
                      n1959 = call "2ndOrderDerivate.vi"("t_capture"=w4497, "initial condition"=w4496, "x"=w4496) -> ("dx/dt"=w4498:dbl)  [unwired: 5 in, 3 out]
                      n1960 = call "2ndOrderDerivate.vi"("t_capture"=w4497, "initial condition"=w4495, "x"=w4495) -> ("dx/dt"=w4500:dbl)  [unwired: 5 in, 3 out]
                      n1961 = call "2ndOrderDerivate.vi"("t_capture"=w4497, "initial condition"=w4494, "x"=w4494) -> ("dx/dt"=w4499:dbl)  [unwired: 5 in, 3 out]
                    }
                    frame 13 {
                      n1962 = call "2ndOrderDerivate.vi"("t_capture"=w4504, "initial condition"=w4503, "x"=w4503) -> ("dx/dt"=w4505:dbl)  [unwired: 5 in, 3 out]
                      n1963 = call "2ndOrderDerivate.vi"("t_capture"=w4504, "initial condition"=w4502, "x"=w4502) -> ("dx/dt"=w4507:dbl)  [unwired: 5 in, 3 out]
                      n1964 = call "2ndOrderDerivate.vi"("t_capture"=w4504, "initial condition"=w4501, "x"=w4501) -> ("dx/dt"=w4506:dbl)  [unwired: 5 in, 3 out]
                    }
                    frame 14 {
                      n1965 = call "2ndOrderDerivate.vi"("t_capture"=w4511, "initial condition"=w4510, "x"=w4510) -> ("dx/dt"=w4512:dbl)  [unwired: 5 in, 3 out]
                      n1966 = call "2ndOrderDerivate.vi"("t_capture"=w4511, "initial condition"=w4509, "x"=w4509) -> ("dx/dt"=w4514:dbl)  [unwired: 5 in, 3 out]
                      n1967 = call "2ndOrderDerivate.vi"("t_capture"=w4511, "initial condition"=w4508, "x"=w4508) -> ("dx/dt"=w4513:dbl)  [unwired: 5 in, 3 out]
                    }
                    frame 15 {
                      n1968 = call "2ndOrderDerivate.vi"("t_capture"=w4518, "initial condition"=w4517, "x"=w4517) -> ("dx/dt"=w4519:dbl)  [unwired: 5 in, 3 out]
                      n1969 = call "2ndOrderDerivate.vi"("t_capture"=w4518, "initial condition"=w4516, "x"=w4516) -> ("dx/dt"=w4521:dbl)  [unwired: 5 in, 3 out]
                      n1970 = call "2ndOrderDerivate.vi"("t_capture"=w4518, "initial condition"=w4515, "x"=w4515) -> ("dx/dt"=w4520:dbl)  [unwired: 5 in, 3 out]
                    }
                  }
                  n1971 = Build Array(w4404, w4400, w4407, w4399, w4406, w4398, w4397, w4396, w4395) -> (w4409:dbl[])
                  n1972 = call-poly <vilib>:"Array To Matrix.vi"("Real 1D Array"=w4409) -> ("Real Matrix (Column Vector)"=w4408:T3)
                  n1973 = Bundle By Name(cluster=w4403, "x_k|k"=w4408) -> (w4405:T2)
                }
              }
              frame True {
              }
            }
            n1974 = case shown="False" w4371 {
              tunnel: w4370 -> [w4637 w4878]
              tunnel: w4358 -> [w4638 _]
              tunnel: [w4636 w4878] -> w4366
              tunnel: w4356 -> [w4635 _]
              frame False {
                n1975 = for {
                  tunnel: w4637 -> [w4647] mode=indexing
                  tunnel: w4638 -> [_]
                  tunnel: [w4649] -> w4636 mode=indexing
                  tunnel: w4635 -> [w4646]
                  n1976 = Unbundle By Name(w4647) -> ("x"=w4648:sgl, "y"=w4651:sgl, "orientation"=w4650:sgl, "robot_id"=w4645:u32)  [unwired: 1 out]
                  n1977 = case shown="0, Default" w4645 {
                    tunnel: w4648 -> [w4768 w4775 w4782 w4789 w4796 w4803 w4810 w4817 w4824 w4831 w4838 w4845 w4852 w4859 w4866 w4873]
                    tunnel: [w4770 w4777 w4784 w4791 w4798 w4805 w4812 w4819 w4826 w4833 w4840 w4847 w4854 w4861 w4868 w4875] -> w4644
                    tunnel: [w4772 w4779 w4786 w4793 w4800 w4807 w4814 w4821 w4828 w4835 w4842 w4849 w4856 w4863 w4870 w4877] -> w4643
                    tunnel: [w4771 w4778 w4785 w4792 w4799 w4806 w4813 w4820 w4827 w4834 w4841 w4848 w4855 w4862 w4869 w4876] -> w4642
                    tunnel: w4651 -> [w4767 w4774 w4781 w4788 w4795 w4802 w4809 w4816 w4823 w4830 w4837 w4844 w4851 w4858 w4865 w4872]
                    tunnel: w4650 -> [w4766 w4773 w4780 w4787 w4794 w4801 w4808 w4815 w4822 w4829 w4836 w4843 w4850 w4857 w4864 w4871]
                    tunnel: w4646 -> [w4769 w4776 w4783 w4790 w4797 w4804 w4811 w4818 w4825 w4832 w4839 w4846 w4853 w4860 w4867 w4874]
                    frame 0, Default {
                      n1978 = call "2ndOrderDerivate.vi"("t_capture"=w4769, "initial condition"=w4768, "x"=w4768) -> ("dx/dt"=w4770:dbl)  [unwired: 5 in, 3 out]
                      n1979 = call "2ndOrderDerivate.vi"("t_capture"=w4769, "initial condition"=w4767, "x"=w4767) -> ("dx/dt"=w4772:dbl)  [unwired: 5 in, 3 out]
                      n1980 = call "2ndOrderDerivate.vi"("t_capture"=w4769, "initial condition"=w4766, "x"=w4766) -> ("dx/dt"=w4771:dbl)  [unwired: 5 in, 3 out]
                    }
                    frame 1 {
                      n1981 = call "2ndOrderDerivate.vi"("t_capture"=w4776, "initial condition"=w4775, "x"=w4775) -> ("dx/dt"=w4777:dbl)  [unwired: 5 in, 3 out]
                      n1982 = call "2ndOrderDerivate.vi"("t_capture"=w4776, "initial condition"=w4774, "x"=w4774) -> ("dx/dt"=w4779:dbl)  [unwired: 5 in, 3 out]
                      n1983 = call "2ndOrderDerivate.vi"("t_capture"=w4776, "initial condition"=w4773, "x"=w4773) -> ("dx/dt"=w4778:dbl)  [unwired: 5 in, 3 out]
                    }
                    frame 2 {
                      n1984 = call "2ndOrderDerivate.vi"("t_capture"=w4783, "initial condition"=w4782, "x"=w4782) -> ("dx/dt"=w4784:dbl)  [unwired: 5 in, 3 out]
                      n1985 = call "2ndOrderDerivate.vi"("t_capture"=w4783, "initial condition"=w4781, "x"=w4781) -> ("dx/dt"=w4786:dbl)  [unwired: 5 in, 3 out]
                      n1986 = call "2ndOrderDerivate.vi"("t_capture"=w4783, "initial condition"=w4780, "x"=w4780) -> ("dx/dt"=w4785:dbl)  [unwired: 5 in, 3 out]
                    }
                    frame 3 {
                      n1987 = call "2ndOrderDerivate.vi"("t_capture"=w4790, "initial condition"=w4789, "x"=w4789) -> ("dx/dt"=w4791:dbl)  [unwired: 5 in, 3 out]
                      n1988 = call "2ndOrderDerivate.vi"("t_capture"=w4790, "initial condition"=w4788, "x"=w4788) -> ("dx/dt"=w4793:dbl)  [unwired: 5 in, 3 out]
                      n1989 = call "2ndOrderDerivate.vi"("t_capture"=w4790, "initial condition"=w4787, "x"=w4787) -> ("dx/dt"=w4792:dbl)  [unwired: 5 in, 3 out]
                    }
                    frame 4 {
                      n1990 = call "2ndOrderDerivate.vi"("t_capture"=w4797, "initial condition"=w4796, "x"=w4796) -> ("dx/dt"=w4798:dbl)  [unwired: 5 in, 3 out]
                      n1991 = call "2ndOrderDerivate.vi"("t_capture"=w4797, "initial condition"=w4795, "x"=w4795) -> ("dx/dt"=w4800:dbl)  [unwired: 5 in, 3 out]
                      n1992 = call "2ndOrderDerivate.vi"("t_capture"=w4797, "initial condition"=w4794, "x"=w4794) -> ("dx/dt"=w4799:dbl)  [unwired: 5 in, 3 out]
                    }
                    frame 5 {
                      n1993 = call "2ndOrderDerivate.vi"("t_capture"=w4804, "initial condition"=w4803, "x"=w4803) -> ("dx/dt"=w4805:dbl)  [unwired: 5 in, 3 out]
                      n1994 = call "2ndOrderDerivate.vi"("t_capture"=w4804, "initial condition"=w4802, "x"=w4802) -> ("dx/dt"=w4807:dbl)  [unwired: 5 in, 3 out]
                      n1995 = call "2ndOrderDerivate.vi"("t_capture"=w4804, "initial condition"=w4801, "x"=w4801) -> ("dx/dt"=w4806:dbl)  [unwired: 5 in, 3 out]
                    }
                    frame 6 {
                      n1996 = call "2ndOrderDerivate.vi"("t_capture"=w4811, "initial condition"=w4810, "x"=w4810) -> ("dx/dt"=w4812:dbl)  [unwired: 5 in, 3 out]
                      n1997 = call "2ndOrderDerivate.vi"("t_capture"=w4811, "initial condition"=w4809, "x"=w4809) -> ("dx/dt"=w4814:dbl)  [unwired: 5 in, 3 out]
                      n1998 = call "2ndOrderDerivate.vi"("t_capture"=w4811, "initial condition"=w4808, "x"=w4808) -> ("dx/dt"=w4813:dbl)  [unwired: 5 in, 3 out]
                    }
                    frame 7 {
                      n1999 = call "2ndOrderDerivate.vi"("t_capture"=w4818, "initial condition"=w4817, "x"=w4817) -> ("dx/dt"=w4819:dbl)  [unwired: 5 in, 3 out]
                      n2000 = call "2ndOrderDerivate.vi"("t_capture"=w4818, "initial condition"=w4816, "x"=w4816) -> ("dx/dt"=w4821:dbl)  [unwired: 5 in, 3 out]
                      n2001 = call "2ndOrderDerivate.vi"("t_capture"=w4818, "initial condition"=w4815, "x"=w4815) -> ("dx/dt"=w4820:dbl)  [unwired: 5 in, 3 out]
                    }
                    frame 8 {
                      n2002 = call "2ndOrderDerivate.vi"("t_capture"=w4825, "initial condition"=w4824, "x"=w4824) -> ("dx/dt"=w4826:dbl)  [unwired: 5 in, 3 out]
                      n2003 = call "2ndOrderDerivate.vi"("t_capture"=w4825, "initial condition"=w4823, "x"=w4823) -> ("dx/dt"=w4828:dbl)  [unwired: 5 in, 3 out]
                      n2004 = call "2ndOrderDerivate.vi"("t_capture"=w4825, "initial condition"=w4822, "x"=w4822) -> ("dx/dt"=w4827:dbl)  [unwired: 5 in, 3 out]
                    }
                    frame 9 {
                      n2005 = call "2ndOrderDerivate.vi"("t_capture"=w4832, "initial condition"=w4831, "x"=w4831) -> ("dx/dt"=w4833:dbl)  [unwired: 5 in, 3 out]
                      n2006 = call "2ndOrderDerivate.vi"("t_capture"=w4832, "initial condition"=w4830, "x"=w4830) -> ("dx/dt"=w4835:dbl)  [unwired: 5 in, 3 out]
                      n2007 = call "2ndOrderDerivate.vi"("t_capture"=w4832, "initial condition"=w4829, "x"=w4829) -> ("dx/dt"=w4834:dbl)  [unwired: 5 in, 3 out]
                    }
                    frame 10 {
                      n2008 = call "2ndOrderDerivate.vi"("t_capture"=w4839, "initial condition"=w4838, "x"=w4838) -> ("dx/dt"=w4840:dbl)  [unwired: 5 in, 3 out]
                      n2009 = call "2ndOrderDerivate.vi"("t_capture"=w4839, "initial condition"=w4837, "x"=w4837) -> ("dx/dt"=w4842:dbl)  [unwired: 5 in, 3 out]
                      n2010 = call "2ndOrderDerivate.vi"("t_capture"=w4839, "initial condition"=w4836, "x"=w4836) -> ("dx/dt"=w4841:dbl)  [unwired: 5 in, 3 out]
                    }
                    frame 11 {
                      n2011 = call "2ndOrderDerivate.vi"("t_capture"=w4846, "initial condition"=w4845, "x"=w4845) -> ("dx/dt"=w4847:dbl)  [unwired: 5 in, 3 out]
                      n2012 = call "2ndOrderDerivate.vi"("t_capture"=w4846, "initial condition"=w4844, "x"=w4844) -> ("dx/dt"=w4849:dbl)  [unwired: 5 in, 3 out]
                      n2013 = call "2ndOrderDerivate.vi"("t_capture"=w4846, "initial condition"=w4843, "x"=w4843) -> ("dx/dt"=w4848:dbl)  [unwired: 5 in, 3 out]
                    }
                    frame 12 {
                      n2014 = call "2ndOrderDerivate.vi"("t_capture"=w4853, "initial condition"=w4852, "x"=w4852) -> ("dx/dt"=w4854:dbl)  [unwired: 5 in, 3 out]
                      n2015 = call "2ndOrderDerivate.vi"("t_capture"=w4853, "initial condition"=w4851, "x"=w4851) -> ("dx/dt"=w4856:dbl)  [unwired: 5 in, 3 out]
                      n2016 = call "2ndOrderDerivate.vi"("t_capture"=w4853, "initial condition"=w4850, "x"=w4850) -> ("dx/dt"=w4855:dbl)  [unwired: 5 in, 3 out]
                    }
                    frame 13 {
                      n2017 = call "2ndOrderDerivate.vi"("t_capture"=w4860, "initial condition"=w4859, "x"=w4859) -> ("dx/dt"=w4861:dbl)  [unwired: 5 in, 3 out]
                      n2018 = call "2ndOrderDerivate.vi"("t_capture"=w4860, "initial condition"=w4858, "x"=w4858) -> ("dx/dt"=w4863:dbl)  [unwired: 5 in, 3 out]
                      n2019 = call "2ndOrderDerivate.vi"("t_capture"=w4860, "initial condition"=w4857, "x"=w4857) -> ("dx/dt"=w4862:dbl)  [unwired: 5 in, 3 out]
                    }
                    frame 14 {
                      n2020 = call "2ndOrderDerivate.vi"("t_capture"=w4867, "initial condition"=w4866, "x"=w4866) -> ("dx/dt"=w4868:dbl)  [unwired: 5 in, 3 out]
                      n2021 = call "2ndOrderDerivate.vi"("t_capture"=w4867, "initial condition"=w4865, "x"=w4865) -> ("dx/dt"=w4870:dbl)  [unwired: 5 in, 3 out]
                      n2022 = call "2ndOrderDerivate.vi"("t_capture"=w4867, "initial condition"=w4864, "x"=w4864) -> ("dx/dt"=w4869:dbl)  [unwired: 5 in, 3 out]
                    }
                    frame 15 {
                      n2023 = call "2ndOrderDerivate.vi"("t_capture"=w4874, "initial condition"=w4873, "x"=w4873) -> ("dx/dt"=w4875:dbl)  [unwired: 5 in, 3 out]
                      n2024 = call "2ndOrderDerivate.vi"("t_capture"=w4874, "initial condition"=w4872, "x"=w4872) -> ("dx/dt"=w4877:dbl)  [unwired: 5 in, 3 out]
                      n2025 = call "2ndOrderDerivate.vi"("t_capture"=w4874, "initial condition"=w4871, "x"=w4871) -> ("dx/dt"=w4876:dbl)  [unwired: 5 in, 3 out]
                    }
                  }
                  n2026 = case shown="0, Default" w4645 {
                    tunnel: w4644 -> [w4656 w4663 w4670 w4677 w4684 w4691 w4698 w4705 w4712 w4719 w4726 w4733 w4740 w4747 w4754 w4761]
                    tunnel: [w4658 w4665 w4672 w4679 w4686 w4693 w4700 w4707 w4714 w4721 w4728 w4735 w4742 w4749 w4756 w4763] -> w4641
                    tunnel: [w4660 w4667 w4674 w4681 w4688 w4695 w4702 w4709 w4716 w4723 w4730 w4737 w4744 w4751 w4758 w4765] -> w4640
                    tunnel: [w4659 w4666 w4673 w4680 w4687 w4694 w4701 w4708 w4715 w4722 w4729 w4736 w4743 w4750 w4757 w4764] -> w4639
                    tunnel: w4643 -> [w4655 w4662 w4669 w4676 w4683 w4690 w4697 w4704 w4711 w4718 w4725 w4732 w4739 w4746 w4753 w4760]
                    tunnel: w4642 -> [w4654 w4661 w4668 w4675 w4682 w4689 w4696 w4703 w4710 w4717 w4724 w4731 w4738 w4745 w4752 w4759]
                    tunnel: w4646 -> [w4657 w4664 w4671 w4678 w4685 w4692 w4699 w4706 w4713 w4720 w4727 w4734 w4741 w4748 w4755 w4762]
                    frame 0, Default {
                      n2027 = call "2ndOrderDerivate.vi"("t_capture"=w4657, "initial condition"=w4656, "x"=w4656) -> ("dx/dt"=w4658:dbl)  [unwired: 5 in, 3 out]
                      n2028 = call "2ndOrderDerivate.vi"("t_capture"=w4657, "initial condition"=w4655, "x"=w4655) -> ("dx/dt"=w4660:dbl)  [unwired: 5 in, 3 out]
                      n2029 = call "2ndOrderDerivate.vi"("t_capture"=w4657, "initial condition"=w4654, "x"=w4654) -> ("dx/dt"=w4659:dbl)  [unwired: 5 in, 3 out]
                    }
                    frame 1 {
                      n2030 = call "2ndOrderDerivate.vi"("t_capture"=w4664, "initial condition"=w4663, "x"=w4663) -> ("dx/dt"=w4665:dbl)  [unwired: 5 in, 3 out]
                      n2031 = call "2ndOrderDerivate.vi"("t_capture"=w4664, "initial condition"=w4662, "x"=w4662) -> ("dx/dt"=w4667:dbl)  [unwired: 5 in, 3 out]
                      n2032 = call "2ndOrderDerivate.vi"("t_capture"=w4664, "initial condition"=w4661, "x"=w4661) -> ("dx/dt"=w4666:dbl)  [unwired: 5 in, 3 out]
                    }
                    frame 2 {
                      n2033 = call "2ndOrderDerivate.vi"("t_capture"=w4671, "initial condition"=w4670, "x"=w4670) -> ("dx/dt"=w4672:dbl)  [unwired: 5 in, 3 out]
                      n2034 = call "2ndOrderDerivate.vi"("t_capture"=w4671, "initial condition"=w4669, "x"=w4669) -> ("dx/dt"=w4674:dbl)  [unwired: 5 in, 3 out]
                      n2035 = call "2ndOrderDerivate.vi"("t_capture"=w4671, "initial condition"=w4668, "x"=w4668) -> ("dx/dt"=w4673:dbl)  [unwired: 5 in, 3 out]
                    }
                    frame 3 {
                      n2036 = call "2ndOrderDerivate.vi"("t_capture"=w4678, "initial condition"=w4677, "x"=w4677) -> ("dx/dt"=w4679:dbl)  [unwired: 5 in, 3 out]
                      n2037 = call "2ndOrderDerivate.vi"("t_capture"=w4678, "initial condition"=w4676, "x"=w4676) -> ("dx/dt"=w4681:dbl)  [unwired: 5 in, 3 out]
                      n2038 = call "2ndOrderDerivate.vi"("t_capture"=w4678, "initial condition"=w4675, "x"=w4675) -> ("dx/dt"=w4680:dbl)  [unwired: 5 in, 3 out]
                    }
                    frame 4 {
                      n2039 = call "2ndOrderDerivate.vi"("t_capture"=w4685, "initial condition"=w4684, "x"=w4684) -> ("dx/dt"=w4686:dbl)  [unwired: 5 in, 3 out]
                      n2040 = call "2ndOrderDerivate.vi"("t_capture"=w4685, "initial condition"=w4683, "x"=w4683) -> ("dx/dt"=w4688:dbl)  [unwired: 5 in, 3 out]
                      n2041 = call "2ndOrderDerivate.vi"("t_capture"=w4685, "initial condition"=w4682, "x"=w4682) -> ("dx/dt"=w4687:dbl)  [unwired: 5 in, 3 out]
                    }
                    frame 5 {
                      n2042 = call "2ndOrderDerivate.vi"("t_capture"=w4692, "initial condition"=w4691, "x"=w4691) -> ("dx/dt"=w4693:dbl)  [unwired: 5 in, 3 out]
                      n2043 = call "2ndOrderDerivate.vi"("t_capture"=w4692, "initial condition"=w4690, "x"=w4690) -> ("dx/dt"=w4695:dbl)  [unwired: 5 in, 3 out]
                      n2044 = call "2ndOrderDerivate.vi"("t_capture"=w4692, "initial condition"=w4689, "x"=w4689) -> ("dx/dt"=w4694:dbl)  [unwired: 5 in, 3 out]
                    }
                    frame 6 {
                      n2045 = call "2ndOrderDerivate.vi"("t_capture"=w4699, "initial condition"=w4698, "x"=w4698) -> ("dx/dt"=w4700:dbl)  [unwired: 5 in, 3 out]
                      n2046 = call "2ndOrderDerivate.vi"("t_capture"=w4699, "initial condition"=w4697, "x"=w4697) -> ("dx/dt"=w4702:dbl)  [unwired: 5 in, 3 out]
                      n2047 = call "2ndOrderDerivate.vi"("t_capture"=w4699, "initial condition"=w4696, "x"=w4696) -> ("dx/dt"=w4701:dbl)  [unwired: 5 in, 3 out]
                    }
                    frame 7 {
                      n2048 = call "2ndOrderDerivate.vi"("t_capture"=w4706, "initial condition"=w4705, "x"=w4705) -> ("dx/dt"=w4707:dbl)  [unwired: 5 in, 3 out]
                      n2049 = call "2ndOrderDerivate.vi"("t_capture"=w4706, "initial condition"=w4704, "x"=w4704) -> ("dx/dt"=w4709:dbl)  [unwired: 5 in, 3 out]
                      n2050 = call "2ndOrderDerivate.vi"("t_capture"=w4706, "initial condition"=w4703, "x"=w4703) -> ("dx/dt"=w4708:dbl)  [unwired: 5 in, 3 out]
                    }
                    frame 8 {
                      n2051 = call "2ndOrderDerivate.vi"("t_capture"=w4713, "initial condition"=w4712, "x"=w4712) -> ("dx/dt"=w4714:dbl)  [unwired: 5 in, 3 out]
                      n2052 = call "2ndOrderDerivate.vi"("t_capture"=w4713, "initial condition"=w4711, "x"=w4711) -> ("dx/dt"=w4716:dbl)  [unwired: 5 in, 3 out]
                      n2053 = call "2ndOrderDerivate.vi"("t_capture"=w4713, "initial condition"=w4710, "x"=w4710) -> ("dx/dt"=w4715:dbl)  [unwired: 5 in, 3 out]
                    }
                    frame 9 {
                      n2054 = call "2ndOrderDerivate.vi"("t_capture"=w4720, "initial condition"=w4719, "x"=w4719) -> ("dx/dt"=w4721:dbl)  [unwired: 5 in, 3 out]
                      n2055 = call "2ndOrderDerivate.vi"("t_capture"=w4720, "initial condition"=w4718, "x"=w4718) -> ("dx/dt"=w4723:dbl)  [unwired: 5 in, 3 out]
                      n2056 = call "2ndOrderDerivate.vi"("t_capture"=w4720, "initial condition"=w4717, "x"=w4717) -> ("dx/dt"=w4722:dbl)  [unwired: 5 in, 3 out]
                    }
                    frame 10 {
                      n2057 = call "2ndOrderDerivate.vi"("t_capture"=w4727, "initial condition"=w4726, "x"=w4726) -> ("dx/dt"=w4728:dbl)  [unwired: 5 in, 3 out]
                      n2058 = call "2ndOrderDerivate.vi"("t_capture"=w4727, "initial condition"=w4725, "x"=w4725) -> ("dx/dt"=w4730:dbl)  [unwired: 5 in, 3 out]
                      n2059 = call "2ndOrderDerivate.vi"("t_capture"=w4727, "initial condition"=w4724, "x"=w4724) -> ("dx/dt"=w4729:dbl)  [unwired: 5 in, 3 out]
                    }
                    frame 11 {
                      n2060 = call "2ndOrderDerivate.vi"("t_capture"=w4734, "initial condition"=w4733, "x"=w4733) -> ("dx/dt"=w4735:dbl)  [unwired: 5 in, 3 out]
                      n2061 = call "2ndOrderDerivate.vi"("t_capture"=w4734, "initial condition"=w4732, "x"=w4732) -> ("dx/dt"=w4737:dbl)  [unwired: 5 in, 3 out]
                      n2062 = call "2ndOrderDerivate.vi"("t_capture"=w4734, "initial condition"=w4731, "x"=w4731) -> ("dx/dt"=w4736:dbl)  [unwired: 5 in, 3 out]
                    }
                    frame 12 {
                      n2063 = call "2ndOrderDerivate.vi"("t_capture"=w4741, "initial condition"=w4740, "x"=w4740) -> ("dx/dt"=w4742:dbl)  [unwired: 5 in, 3 out]
                      n2064 = call "2ndOrderDerivate.vi"("t_capture"=w4741, "initial condition"=w4739, "x"=w4739) -> ("dx/dt"=w4744:dbl)  [unwired: 5 in, 3 out]
                      n2065 = call "2ndOrderDerivate.vi"("t_capture"=w4741, "initial condition"=w4738, "x"=w4738) -> ("dx/dt"=w4743:dbl)  [unwired: 5 in, 3 out]
                    }
                    frame 13 {
                      n2066 = call "2ndOrderDerivate.vi"("t_capture"=w4748, "initial condition"=w4747, "x"=w4747) -> ("dx/dt"=w4749:dbl)  [unwired: 5 in, 3 out]
                      n2067 = call "2ndOrderDerivate.vi"("t_capture"=w4748, "initial condition"=w4746, "x"=w4746) -> ("dx/dt"=w4751:dbl)  [unwired: 5 in, 3 out]
                      n2068 = call "2ndOrderDerivate.vi"("t_capture"=w4748, "initial condition"=w4745, "x"=w4745) -> ("dx/dt"=w4750:dbl)  [unwired: 5 in, 3 out]
                    }
                    frame 14 {
                      n2069 = call "2ndOrderDerivate.vi"("t_capture"=w4755, "initial condition"=w4754, "x"=w4754) -> ("dx/dt"=w4756:dbl)  [unwired: 5 in, 3 out]
                      n2070 = call "2ndOrderDerivate.vi"("t_capture"=w4755, "initial condition"=w4753, "x"=w4753) -> ("dx/dt"=w4758:dbl)  [unwired: 5 in, 3 out]
                      n2071 = call "2ndOrderDerivate.vi"("t_capture"=w4755, "initial condition"=w4752, "x"=w4752) -> ("dx/dt"=w4757:dbl)  [unwired: 5 in, 3 out]
                    }
                    frame 15 {
                      n2072 = call "2ndOrderDerivate.vi"("t_capture"=w4762, "initial condition"=w4761, "x"=w4761) -> ("dx/dt"=w4763:dbl)  [unwired: 5 in, 3 out]
                      n2073 = call "2ndOrderDerivate.vi"("t_capture"=w4762, "initial condition"=w4760, "x"=w4760) -> ("dx/dt"=w4765:dbl)  [unwired: 5 in, 3 out]
                      n2074 = call "2ndOrderDerivate.vi"("t_capture"=w4762, "initial condition"=w4759, "x"=w4759) -> ("dx/dt"=w4764:dbl)  [unwired: 5 in, 3 out]
                    }
                  }
                  n2075 = Build Array(w4648, w4644, w4651, w4643, w4650, w4642, w4641, w4640, w4639) -> (w4653:dbl[])
                  n2076 = call-poly <vilib>:"Array To Matrix.vi"("Real 1D Array"=w4653) -> ("Real Matrix (Column Vector)"=w4652:T3)
                  n2077 = Bundle By Name(cluster=w4647, "x_k|k"=w4652) -> (w4649:T2)
                }
              }
              frame True {
              }
            }
            n2078 = Bundle By Name(cluster=w4361, "robots_blue"=w4366, "robots_yellow"=w4365, "balls"=w4357) -> (w4364:T1)
            n2079 = Bundle By Name(cluster=w4361, "New"=FALSE) -> (w4362:T1)
          }
        }
      }
      frame "Nenhum" {
      }
    }
  }
  n2080 = feedback-in #1(w26) -> ()
  n2081 = feedback-in #3(w16) -> ()
  n2082 = disable-structure shown="Enabled" {
    disable-tunnel: _ -> [w4893 _]
    disable-tunnel: _ -> [w4892 _]
    disable-tunnel: _ -> [w4891 _]
    disable-tunnel: _ -> [w4886 _]
    disable-tunnel: w16 -> [w4883 w4898]
    disable-tunnel: [_ w4897] -> w6
    disable-tunnel: "cameras array" -> [_ w4896]
    disable-tunnel: "grSim?" -> [_ w4895]
    disable-tunnel: "Field Size" -> [_ w4894]
    frame Disabled {
      n2083 = Bundle By Name(cluster=w4893, "robots_yellow"=w4892, "robots_blue"=w4891, "balls"=w4886) -> (w4882:cluster{})
      n2084 = Unbundle By Name(w4882) -> ("balls"=w4885, "robots_yellow"=w4888, "robots_blue"=w4890)
      n2085 = call "Select Robots By Confidence.vi"("robots_blue"=w4888) -> ("Array"=w4887:T2[])  [unwired: 10 in]
      n2086 = call "Select Ball By Confidence.vi"("Array"=w4883, "balls"=w4885) -> ("balls out"=w4884:T4[])  [unwired: 9 in]
      n2087 = call "Select Robots By Confidence.vi"("robots_blue"=w4890) -> ("Array"=w4889:T2[])  [unwired: 10 in]
      n2088 = Bundle By Name(cluster=w4882, "balls"=w4884, "robots_yellow"=w4887, "robots_blue"=w4889) -> (w4881:cluster{})
    }
    frame Enabled {
      n2089 = call "mediaIntesecaoCameras_v2.vi"("grsim?"=w4895, "cameras array"=w4896, "Field Geometry In"=w4894, "Cameras Array"=w4898) -> ("frame out"=w4897:T1)  [unwired: 7 in]
    }
  }
  n2090 = Unbundle By Name(w6) -> ("balls"=w11:T4[])
  n2091 = Index Array(array=w11) -> (element=w10:T4)  [unwired: 1 in]
  n2092 = Unbundle By Name(w10) -> ("Valid"=w9:bool)
  n2093 = case shown="False" w9 {
    tunnel: [w4900 w4920] -> w12
    tunnel: w11 -> [_ w4904]
    tunnel: w11 -> [w4902 _]
    tunnel: w13 -> [w4901 _]
    tunnel: "Life Time" -> [w4899 _]
    frame False {
      n2094 = call "NewBallLifetime.vi"("Life Time"=w4899, "last balls"=w4901, "current balls array"=w4902) -> ("balls out"=w4900:T4[])  [unwired: 8 in]
    }
    frame True {
      n2095 = Index Array(array=w4904) -> (element=w4903:T4)  [unwired: 1 in]
      n2096 = Unbundle By Name(w4903) -> ("x_k|k"=w4912:T3)
      n2097 = feedback #4() -> (w4919:T4[])  [unwired: 1 in]
      n2098 = Build Array (concatenate)(w4903, w4919) -> (w4918:T4[])
      n2099 = Delete From Array(array=w4918, index=12) -> (array with subset deleted=w4916:T4[])  [unwired: 1 in, 1 out]
      n2100 = feedback-in #4(w4916) -> ()
      n2101 = for {
        tunnel: w4916 -> [w4926] mode=indexing
        tunnel: [w4922] -> w4915 mode=indexing
        tunnel: [w4921] -> w4914 mode=indexing
        n2102 = Unbundle By Name(w4926) -> ("x_k|k"=w4925:T3)
        n2103 = Index Array(array=w4925) -> (element #2=w4924:dbl[], element #4=w4923:dbl[])  [unwired: 8 in, 2 out]
        n2104 = Index Array(array=w4924) -> (element=w4922:dbl)  [unwired: 1 in]
        n2105 = Index Array(array=w4923) -> (element=w4921:dbl)  [unwired: 1 in]
      }
      n2106 = call <vilib>:"Median.vi"("X"=w4915) -> ("median"=w4909:dbl)  [unwired: 1 out]
      n2107 = call <vilib>:"Median.vi"("X"=w4914) -> ("median"=w4906:dbl)  [unwired: 1 out]
      n2108 = Replace Array Subset(array=w4912, new element #1=w4909, index (row) #1=1 ("index (row)"), index (col) #1=0 ("index (row)"), new element #2=w4906, index (row) #2=3 ("index (row)"), index (col) #2=0 ("index (row)")) -> (w4905:T3)
      n2109 = Bundle By Name(cluster=w4903, "x_k|k"=w4905) -> (w4913:T4)
      n2110 = Build Array(w4913) -> (w4920:T4[])
    }
  }
  n2111 = feedback-in #2(w12) -> ()
  n2112 = Unbundle By Name(w6) -> ("robots_blue"=w5:T2[], "robots_yellow"=w4:T2[])
  n2113 = disable-structure shown="Enabled" {
    disable-tunnel: w5 -> [w4933 w4935]
    disable-tunnel: w4 -> [w4932 w4934]
    disable-tunnel: "Life Time" -> [w4931 _]
    disable-tunnel: [w4930 w4935] -> w2
    disable-tunnel: [w4928 w4934] -> w1
    frame Enabled {
      n2114 = feedback #5() -> (w4927:T2[])  [unwired: 1 in]
      n2115 = call "newRobotsLifeTime.vi"("Life Time"=w4931, "old robots"=w4927, "robots"=w4932) -> ("robots"=w4928:T2[])  [unwired: 6 in, 2 out]
      n2116 = feedback-in #5(w4928) -> ()
      n2117 = feedback #6() -> (w4929:T2[])  [unwired: 1 in]
      n2118 = call "newRobotsLifeTime.vi"("Life Time"=w4931, "old robots"=w4929, "robots"=w4933) -> ("robots"=w4930:T2[])  [unwired: 6 in, 2 out]
      n2119 = feedback-in #6(w4930) -> ()
    }
    frame Disabled {
    }
  }
  n2120 = Get Date/Time In Seconds() -> (seconds since 1Jan1904=w15:timestamp)
  n2121 = Bundle By Name(cluster=w6, "robots_blue"=w2, "robots_yellow"=w1, "balls"=w12, "Time Stamp"=w15) -> (→"Detection Frame Out":T1)
  "Field Size Out" <- "Field Size"
